vi "transconductance.vi"(6 "Vsg step":dbl=0.002, 8 "B max":dbl=67.0, 9 "B min":dbl=87.0, 10 "load data from file?":bool=TRUE) -> (0 "N Array":T1(array[cluster])=[{"N1"=157.003, "N2"=266.981, "N3"=0.00010058761141376306, "N4"=-1.0315790407323053e-05}, {"N1"=157.003, "N2"=265.999, "N3"=0.00010059098292336149, "N4"=-1.0332480129997402e-05}, {"N1"=157.003, "N2"=265.085, "N3"=0.00010060944077843739, "N4"=-1.0322427910341245e-05}, {"N1"=157.003, "N2"=263.997, "N3"=0.000100657113380779, "N4"=-1.0393866015746848e-05}, {"N1"=157.003, "N2"=263.075, "N3"=0.00010069386977626447, "N4"=-1.0407685152644096e-05}, {"N1"=157.003, "N2"=262.077, "N3"=0.00010056895998220536, "N4"=-1.0343510988281777e-05}, {"N1"=157.003, "N2"=261.132, "N3"=0.00010053448024520868, "N4"=-1.0349016712876126e-05}, {"N1"=157.003, "N2"=260.059, "N3"=0.00010062294424790826, "N4"=-1.0277597394971399e-05}, {"N1"=157.003, "N2"=259.002, "N3"=0.00010065465463674774, "N4"=-1.030766592338683e-05}, {"N1"=157.003, "N2"=257.994, "N3"=0.00010053039567669925, "N4"=-1.0503582041961604e-05}, {"N1"=157.003, "N2"=257.002, "N3"=0.00010061057686438726, "N4"=-1.0271984325309709e-05}, {"N1"=157.003, "N2"=256.047, "N3"=0.00010067349246760751, "N4"=-1.0251899805257316e-05}, {"N1"=157.003, "N2"=255.009, "N3"=0.0001005746979150816, "N4"=-1.0374581059943446e-05}, {"N1"=157.003, "N2"=254.01, "N3"=0.00010064525623886029, "N4"=-1.0267776606434536e-05}, {"N1"=157.003, "N2"=252.961, "N3"=0.0001005733669086136, "N4"=-1.0318808655600757e-05}, {"N1"=157.003, "N2"=252.138, "N3"=0.00010065566340283842, "N4"=-1.0302895488637936e-05}, {"N1"=157.003, "N2"=251.239, "N3"=0.0001006794958238487, "N4"=-1.030436110773387e-05}, {"N1"=157.003, "N2"=250.058, "N3"=0.0001006606457173001, "N4"=-1.033162509347294e-05}, {"N1"=157.003, "N2"=249.134, "N3"=0.00010070695284612299, "N4"=-1.0349127157664972e-05}, {"N1"=157.003, "N2"=248.057, "N3"=0.00010063480571495228, "N4"=-1.0343952424043254e-05}, {"N1"=157.003, "N2"=247.046, "N3"=0.0001005939449441208, "N4"=-1.0301691972698925e-05}, {"N1"=157.003, "N2"=246.001, "N3"=0.00010061079760290319, "N4"=-1.0341399561683132e-05}, {"N1"=157.003, "N2"=245.127, "N3"=0.00010063836300299804, "N4"=-1.038263241630273e-05}, {"N1"=157.003, "N2"=244.19, "N3"=0.00010052888786407929, "N4"=-1.0366000769957849e-05}, {"N1"=157.003, "N2"=243.056, "N3"=0.00010055609422862572, "N4"=-1.032480110310128e-05}, {"N1"=157.003, "N2"=241.985, "N3"=0.00010060349631456675, "N4"=-1.0352572333486109e-05}, {"N1"=157.003, "N2"=240.968, "N3"=0.0001005730466397368, "N4"=-1.0406162088350849e-05}, {"N1"=157.003, "N2"=239.997, "N3"=0.00010055796837859916, "N4"=-1.0447874922582124e-05}, {"N1"=157.003, "N2"=239.348, "N3"=0.00010064935879623944, "N4"=-1.0319947524395836e-05}, {"N1"=157.003, "N2"=238.084, "N3"=0.00010057773089892466, "N4"=-1.0479841722046195e-05}, {"N1"=157.003, "N2"=237.112, "N3"=0.00010064891429557363, "N4"=-1.049047519616346e-05}, {"N1"=157.003, "N2"=236.004, "N3"=0.00010065709472725735, "N4"=-1.0324150119014948e-05}, {"N1"=157.003, "N2"=234.996, "N3"=0.00010057723777641319, "N4"=-1.0336422363141234e-05}, {"N1"=157.003, "N2"=234.019, "N3"=0.00010045398973880146, "N4"=-1.0377301904232947e-05}, {"N1"=157.003, "N2"=233.096, "N3"=0.00010057181495580477, "N4"=-1.0313588970498165e-05}, {"N1"=157.003, "N2"=232.123, "N3"=0.00010054998403538271, "N4"=-1.0403263055311217e-05}, {"N1"=157.003, "N2"=231.112, "N3"=0.00010069630908042105, "N4"=-1.0328850635915879e-05}, {"N1"=157.003, "N2"=230.005, "N3"=0.0001005825699420265, "N4"=-1.013345847934897e-05}, {"N1"=157.003, "N2"=229.052, "N3"=0.00010066775145077032, "N4"=-1.0360530914703863e-05}, {"N1"=157.003, "N2"=228.029, "N3"=0.0001006005911344668, "N4"=-1.0262365451060467e-05}, {"N1"=157.003, "N2"=227.081, "N3"=0.0001006880496209156, "N4"=-1.0331153141935446e-05}, {"N1"=157.003, "N2"=226.184, "N3"=0.00010063762766846488, "N4"=-1.0365370825229791e-05}, {"N1"=157.003, "N2"=225.156, "N3"=0.00010060840425208388, "N4"=-1.0325694682226826e-05}, {"N1"=157.003, "N2"=223.981, "N3"=0.00010060008180158568, "N4"=-1.030788393467471e-05}, {"N1"=157.003, "N2"=223.117, "N3"=0.00010064362809307492, "N4"=-1.0410394990300755e-05}, {"N1"=157.003, "N2"=222.006, "N3"=0.00010052956894532667, "N4"=-1.0312456867656895e-05}, {"N1"=157.003, "N2"=221.15, "N3"=0.00010073993925105531, "N4"=-1.0520923879015318e-05}, {"N1"=157.003, "N2"=220.132, "N3"=0.0001005467107798333, "N4"=-1.0451840001316155e-05}, {"N1"=157.003, "N2"=219.14, "N3"=0.00010056576858730084, "N4"=-1.0520553001153154e-05}, {"N1"=157.003, "N2"=218.151, "N3"=0.00010058549543700654, "N4"=-1.0330365594944888e-05}, {"N1"=157.003, "N2"=217.144, "N3"=0.00010051145692162056, "N4"=-1.03377330611703e-05}, {"N1"=157.003, "N2"=216.153, "N3"=0.00010073501846407267, "N4"=-1.0489693235349407e-05}, {"N1"=157.003, "N2"=214.997, "N3"=0.00010066401252774728, "N4"=-1.0430688948597772e-05}, {"N1"=157.003, "N2"=214.148, "N3"=0.00010062308186580819, "N4"=-1.0280249425931093e-05}, {"N1"=157.003, "N2"=213.226, "N3"=0.00010062562347473316, "N4"=-1.0297033249151475e-05}, {"N1"=157.003, "N2"=212.267, "N3"=0.0001004056393064652, "N4"=-1.0354527978745687e-05}, {"N1"=157.003, "N2"=211.106, "N3"=0.00010053371092077836, "N4"=-1.0258061653605368e-05}, {"N1"=157.003, "N2"=210.034, "N3"=0.0001005206561452233, "N4"=-1.0277392375838352e-05}, {"N1"=157.003, "N2"=209.16, "N3"=0.00010062151524095544, "N4"=-1.0318539021491905e-05}, {"N1"=157.003, "N2"=208.248, "N3"=0.00010059710791627925, "N4"=-1.0633465001550955e-05}, {"N1"=157.003, "N2"=207.003, "N3"=0.00010062673174994523, "N4"=-1.0321171852761056e-05}, {"N1"=157.003, "N2"=206.388, "N3"=0.00010061513331833293, "N4"=-1.0324705100902347e-05}, {"N1"=157.003, "N2"=204.991, "N3"=0.0001005439011236034, "N4"=-1.0309493090621932e-05}, {"N1"=157.003, "N2"=204.132, "N3"=0.00010070060888909204, "N4"=-1.0291219627570718e-05}, {"N1"=157.003, "N2"=203.139, "N3"=0.00010064572292852508, "N4"=-1.0464495626958931e-05}, {"N1"=157.003, "N2"=202.208, "N3"=0.00010064163036004339, "N4"=-1.0527705497905832e-05}, {"N1"=157.003, "N2"=200.997, "N3"=0.00010060444212186648, "N4"=-1.0239666475444635e-05}, {"N1"=157.003, "N2"=199.979, "N3"=0.00010045464357967768, "N4"=-1.0332757739473804e-05}, {"N1"=157.003, "N2"=199.145, "N3"=0.00010052319470245587, "N4"=-1.0408078825076916e-05}, {"N1"=157.003, "N2"=198.151, "N3"=0.00010054670987583925, "N4"=-1.0224118002428333e-05}, {"N1"=157.003, "N2"=197.167, "N3"=0.00010064778537782342, "N4"=-1.0323540832018964e-05}, {"N1"=157.003, "N2"=196.024, "N3"=0.00010059750202844955, "N4"=-1.031116849358743e-05}, {"N1"=157.003, "N2"=195.158, "N3"=0.00010058423886157823, "N4"=-1.0255054779838974e-05}, {"N1"=157.003, "N2"=194.255, "N3"=0.00010071404209700317, "N4"=-1.0181418387683495e-05}, {"N1"=157.003, "N2"=193.167, "N3"=0.00010057340590266535, "N4"=-1.0242330877904251e-05}, {"N1"=157.003, "N2"=192.004, "N3"=0.00010068713388045283, "N4"=-1.0249310430158046e-05}, {"N1"=157.003, "N2"=191.222, "N3"=0.00010060502412989036, "N4"=-1.0132381864656099e-05}, {"N1"=157.003, "N2"=190.0, "N3"=0.00010060744320199426, "N4"=-1.0398792500202499e-05}, {"N1"=157.003, "N2"=189.161, "N3"=0.00010058313711640197, "N4"=-1.0335999046260006e-05}, {"N1"=157.003, "N2"=188.182, "N3"=0.0001005729482088783, "N4"=-1.0175494539414885e-05}, {"N1"=157.003, "N2"=187.187, "N3"=0.00010062532065791654, "N4"=-1.0311661990340356e-05}, {"N1"=157.003, "N2"=186.127, "N3"=0.00010070821910793247, "N4"=-1.027480676439334e-05}, {"N1"=157.003, "N2"=185.003, "N3"=0.00010055156194819312, "N4"=-1.028064538575304e-05}, {"N1"=157.003, "N2"=183.995, "N3"=0.00010067671472910203, "N4"=-1.0455212193898765e-05}, {"N1"=157.003, "N2"=183.205, "N3"=0.00010050604172122397, "N4"=-1.0365017753701822e-05}, {"N1"=157.003, "N2"=182.153, "N3"=0.00010057840866780894, "N4"=-1.0315396628303899e-05}, {"N1"=157.003, "N2"=181.15, "N3"=0.00010058546375450866, "N4"=-1.0361578284644076e-05}, {"N1"=157.003, "N2"=179.996, "N3"=0.0001006240086180247, "N4"=-1.0119129316713388e-05}, {"N1"=157.003, "N2"=179.042, "N3"=0.00010064273438767862, "N4"=-1.0255802631395027e-05}, {"N1"=157.003, "N2"=177.974, "N3"=0.00010063106842247951, "N4"=-1.0299974893794054e-05}, {"N1"=157.003, "N2"=177.161, "N3"=0.00010065009914739528, "N4"=-1.0296372901106247e-05}, {"N1"=157.003, "N2"=175.982, "N3"=0.00010067126680486314, "N4"=-1.0306700692332765e-05}, {"N1"=157.003, "N2"=174.995, "N3"=0.00010053475509784773, "N4"=-1.0433320095914615e-05}, {"N1"=157.003, "N2"=174.139, "N3"=0.00010049406853859304, "N4"=-1.0270604949039266e-05}, {"N1"=157.003, "N2"=173.118, "N3"=0.00010053736854866473, "N4"=-1.016880594814786e-05}, {"N1"=157.003, "N2"=172.219, "N3"=0.00010058931714745791, "N4"=-1.0410165714531099e-05}, {"N1"=157.003, "N2"=171.156, "N3"=0.00010056082364767814, "N4"=-1.0322038747437007e-05}, {"N1"=157.003, "N2"=170.109, "N3"=0.00010056010719994381, "N4"=-1.0287668368179046e-05}, {"N1"=157.003, "N2"=169.204, "N3"=0.00010064886941818687, "N4"=-1.029160673901251e-05}, {"N1"=157.003, "N2"=168.15, "N3"=0.00010060742217090351, "N4"=-1.0262911647489893e-05}, {"N1"=157.003, "N2"=167.112, "N3"=0.00010047282448029428, "N4"=-1.0358833399498402e-05}, {"N1"=157.003, "N2"=166.21, "N3"=0.00010060401190277079, "N4"=-1.0350385128996471e-05}, {"N1"=157.003, "N2"=165.011, "N3"=0.00010060416035284246, "N4"=-1.0377472785141268e-05}, {"N1"=157.003, "N2"=164.167, "N3"=0.0001004397217463161, "N4"=-1.0450134705351127e-05}, {"N1"=157.003, "N2"=163.001, "N3"=0.00010051036584794823, "N4"=-1.0382389231895817e-05}, {"N1"=157.003, "N2"=162.034, "N3"=0.00010047904100883916, "N4"=-1.0341186675967576e-05}, {"N1"=157.003, "N2"=160.997, "N3"=0.00010053000872693343, "N4"=-1.0484345783511955e-05}, {"N1"=157.003, "N2"=160.209, "N3"=0.00010062652830459546, "N4"=-1.0297537290876405e-05}, {"N1"=157.003, "N2"=159.149, "N3"=0.00010056339474194626, "N4"=-1.0346385416074202e-05}, {"N1"=157.003, "N2"=157.992, "N3"=0.00010054027429101758, "N4"=-1.0402084267772915e-05}, {"N1"=157.003, "N2"=157.001, "N3"=0.00010072664661678648, "N4"=-1.0389584614637704e-05}, {"N1"=157.003, "N2"=156.136, "N3"=0.00010057574533189637, "N4"=-1.0286379321831545e-05}, {"N1"=157.003, "N2"=155.184, "N3"=0.00010061297401308573, "N4"=-1.0356101436450663e-05}, {"N1"=157.003, "N2"=154.14, "N3"=0.00010065486717861918, "N4"=-1.027695564379398e-05}, {"N1"=157.003, "N2"=153.001, "N3"=0.00010066710265738706, "N4"=-1.0289877618531446e-05}, {"N1"=157.003, "N2"=152.094, "N3"=0.00010069298668309146, "N4"=-1.0373605458303733e-05}, {"N1"=157.003, "N2"=151.229, "N3"=0.00010075373194915584, "N4"=-1.0343078388110773e-05}, {"N1"=147.01, "N2"=267.017, "N3"=9.799983736018753e-05, "N4"=-1.0019951532324723e-05}, {"N1"=147.01, "N2"=262.383, "N3"=9.763241950106681e-05, "N4"=-9.728183012788925e-06}, {"N1"=147.01, "N2"=257.562, "N3"=9.857415477184657e-05, "N4"=-9.961675445649451e-06}, {"N1"=147.01, "N2"=252.008, "N3"=9.812568640591443e-05, "N4"=-9.853612153506874e-06}, {"N1"=147.01, "N2"=247.006, "N3"=9.984319825339365e-05, "N4"=-1.0146544647968204e-05}, {"N1"=147.01, "N2"=241.997, "N3"=9.947477892699824e-05, "N4"=-1.0131401570354352e-05}, {"N1"=147.01, "N2"=238.533, "N3"=0.00010005415475521616, "N4"=-1.0167893750971189e-05}, {"N1"=147.01, "N2"=232.001, "N3"=9.882236061778423e-05, "N4"=-1.011184445981214e-05}, {"N1"=147.01, "N2"=228.619, "N3"=9.9581272321477e-05, "N4"=-1.0201481180871728e-05}, {"N1"=147.01, "N2"=221.992, "N3"=9.96719889398003e-05, "N4"=-1.0088519208290693e-05}, {"N1"=147.01, "N2"=217.038, "N3"=9.844041955679962e-05, "N4"=-9.941300701952415e-06}, {"N1"=147.01, "N2"=212.037, "N3"=9.969254017177194e-05, "N4"=-1.0181600609931255e-05}, {"N1"=147.01, "N2"=207.001, "N3"=9.949616020991875e-05, "N4"=-1.0131625256668759e-05}, {"N1"=147.01, "N2"=202.009, "N3"=9.972322051345787e-05, "N4"=-1.030119353660157e-05}, {"N1"=147.01, "N2"=197.009, "N3"=9.972222689830247e-05, "N4"=-1.0129755820315606e-05}, {"N1"=147.01, "N2"=192.052, "N3"=9.927072186296552e-05, "N4"=-1.0101700894209476e-05}, {"N1"=147.01, "N2"=187.035, "N3"=9.971985526642769e-05, "N4"=-1.0163071908619776e-05}, {"N1"=147.01, "N2"=182.038, "N3"=9.938768123188747e-05, "N4"=-1.0116333084138861e-05}, {"N1"=147.01, "N2"=177.024, "N3"=9.895565966028784e-05, "N4"=-1.0184916134362883e-05}, {"N1"=147.01, "N2"=172.002, "N3"=9.903423254443763e-05, "N4"=-9.977232855655323e-06}, {"N1"=147.01, "N2"=167.528, "N3"=9.938030934401597e-05, "N4"=-1.013542865258268e-05}, {"N1"=147.01, "N2"=162.609, "N3"=9.898463034406892e-05, "N4"=-1.0045094991441177e-05}, {"N1"=147.01, "N2"=157.833, "N3"=9.946683387231336e-05, "N4"=-1.0208638458775468e-05}, {"N1"=137.106, "N2"=157.019, "N3"=0.00010037737790660152, "N4"=-1.030680610999361e-05}, {"N1"=137.106, "N2"=161.993, "N3"=0.00010051095901282851, "N4"=-1.015609388550053e-05}, {"N1"=137.106, "N2"=166.478, "N3"=0.00010061415096599144, "N4"=-1.0361761811054065e-05}, {"N1"=137.106, "N2"=171.321, "N3"=0.00010066129576563336, "N4"=-1.0484617945251967e-05}, {"N1"=137.106, "N2"=177.002, "N3"=0.00010061617278473286, "N4"=-1.0472267311277374e-05}, {"N1"=137.106, "N2"=181.274, "N3"=0.00010061494851260961, "N4"=-1.0526404210905806e-05}, {"N1"=137.106, "N2"=185.979, "N3"=0.00010059337699446351, "N4"=-1.040515740405918e-05}, {"N1"=137.106, "N2"=190.957, "N3"=0.0001006229368267242, "N4"=-1.0316576837476962e-05}, {"N1"=137.106, "N2"=196.956, "N3"=0.00010052691716632796, "N4"=-1.0426565141411268e-05}, {"N1"=137.106, "N2"=200.797, "N3"=0.00010048017416406656, "N4"=-1.0205543027371177e-05}, {"N1"=137.106, "N2"=206.992, "N3"=0.00010051573531694569, "N4"=-1.0500465961498208e-05}, {"N1"=137.106, "N2"=211.99, "N3"=0.00010047604987372997, "N4"=-1.0186688450911605e-05}, {"N1"=137.106, "N2"=216.974, "N3"=0.00010041066876877247, "N4"=-1.0483017642678282e-05}, {"N1"=137.106, "N2"=221.18, "N3"=0.00010052645014313375, "N4"=-1.0365935977453018e-05}, {"N1"=137.106, "N2"=225.381, "N3"=0.00010058558925443369, "N4"=-1.0254871445882739e-05}, {"N1"=137.106, "N2"=232.004, "N3"=9.913954515490299e-05, "N4"=-1.005309209916423e-05}, {"N1"=137.106, "N2"=236.99, "N3"=0.0001003799328902402, "N4"=-1.0139936029757658e-05}, {"N1"=137.106, "N2"=242.016, "N3"=0.00010005730438840346, "N4"=-1.0090877786993333e-05}, {"N1"=137.106, "N2"=245.974, "N3"=0.00010048425816903801, "N4"=-1.0483823131656468e-05}, {"N1"=137.106, "N2"=250.925, "N3"=0.00010040732666965968, "N4"=-1.0299776631743095e-05}, {"N1"=137.106, "N2"=257.02, "N3"=0.00010045673123155542, "N4"=-1.014502752268486e-05}, {"N1"=137.106, "N2"=261.97, "N3"=0.00010053750806744122, "N4"=-1.0170204737819931e-05}, {"N1"=137.106, "N2"=266.974, "N3"=0.00010046811899562129, "N4"=-1.0258157731175788e-05}, {"N1"=127.009, "N2"=157.022, "N3"=0.00010057347860141696, "N4"=-1.0228102959349011e-05}, {"N1"=127.009, "N2"=161.996, "N3"=0.00010062562883782826, "N4"=-1.0170220838565306e-05}, {"N1"=127.009, "N2"=167.013, "N3"=0.00010066593581146635, "N4"=-1.0124193285242448e-05}, {"N1"=127.009, "N2"=171.248, "N3"=0.00010070721275823473, "N4"=-1.0260385180386528e-05}, {"N1"=127.009, "N2"=176.996, "N3"=0.00010064297358361281, "N4"=-1.0308355187961158e-05}, {"N1"=127.009, "N2"=181.986, "N3"=0.00010061342489787007, "N4"=-1.0129603180411648e-05}, {"N1"=127.009, "N2"=186.989, "N3"=0.00010061225714944682, "N4"=-1.026327093758386e-05}, {"N1"=127.009, "N2"=192.002, "N3"=0.00010060286819188852, "N4"=-1.0222596869690172e-05}, {"N1"=127.009, "N2"=197.03, "N3"=0.00010067499622887365, "N4"=-1.042309998693685e-05}, {"N1"=127.009, "N2"=202.004, "N3"=0.00010059110286327089, "N4"=-1.0321036547786183e-05}, {"N1"=127.009, "N2"=206.995, "N3"=0.00010059948277673225, "N4"=-1.0384420982036602e-05}, {"N1"=127.009, "N2"=211.966, "N3"=0.00010058300170100732, "N4"=-1.0321869852951667e-05}, {"N1"=127.009, "N2"=216.996, "N3"=0.00010057100746133218, "N4"=-1.0479270764700121e-05}, {"N1"=127.009, "N2"=222.012, "N3"=0.00010050186248972992, "N4"=-1.0279112143261431e-05}, {"N1"=127.009, "N2"=227.008, "N3"=0.00010067472374815698, "N4"=-1.024778604350329e-05}, {"N1"=127.009, "N2"=231.971, "N3"=0.00010065735991437597, "N4"=-1.027124744107791e-05}, {"N1"=127.009, "N2"=237.004, "N3"=0.00010057124546163262, "N4"=-1.0340391607088675e-05}, {"N1"=127.009, "N2"=242.0, "N3"=0.00010054458432600382, "N4"=-1.0398708177970036e-05}, {"N1"=127.009, "N2"=246.996, "N3"=0.00010062032362546629, "N4"=-1.029301084170431e-05}, {"N1"=127.009, "N2"=251.943, "N3"=0.0001005705365053531, "N4"=-1.0188324652684972e-05}, {"N1"=127.009, "N2"=256.96, "N3"=0.00010061231844925602, "N4"=-1.0222616593874322e-05}, {"N1"=127.009, "N2"=261.944, "N3"=0.0001005374732511164, "N4"=-1.0238804050129587e-05}, {"N1"=127.009, "N2"=267.002, "N3"=0.00010061482989823944, "N4"=-1.0260599454521908e-05}, {"N1"=117.007, "N2"=32.056, "N3"=0.00010064978817090146, "N4"=-1.025610764423456e-05}, {"N1"=117.007, "N2"=34.532, "N3"=0.00010045388961118922, "N4"=-1.0281623718938048e-05}, {"N1"=117.007, "N2"=36.991, "N3"=0.00010051501976709822, "N4"=-1.0346988455857735e-05}, {"N1"=117.007, "N2"=39.496, "N3"=0.00010051493139529077, "N4"=-1.0087270665342305e-05}, {"N1"=117.007, "N2"=42.014, "N3"=0.00010069551813105615, "N4"=-1.0293552346164798e-05}, {"N1"=117.007, "N2"=44.076, "N3"=0.00010061513649741965, "N4"=-1.0166358665250762e-05}, {"N1"=117.007, "N2"=47.003, "N3"=0.00010062687846722984, "N4"=-1.0327337858815028e-05}, {"N1"=117.007, "N2"=49.497, "N3"=0.00010056452732695654, "N4"=-1.0173349314359884e-05}, {"N1"=117.007, "N2"=52.015, "N3"=0.00010052841627670957, "N4"=-1.0154426622830124e-05}, {"N1"=117.007, "N2"=54.143, "N3"=0.00010067512909890701, "N4"=-1.0297943395729118e-05}, {"N1"=117.007, "N2"=56.469, "N3"=0.00010058850823882672, "N4"=-1.0229671611179695e-05}, {"N1"=117.007, "N2"=59.109, "N3"=0.00010052479798279025, "N4"=-1.0343373479061018e-05}, {"N1"=117.007, "N2"=61.392, "N3"=0.00010058686320873386, "N4"=-1.022378755210072e-05}, {"N1"=117.007, "N2"=64.504, "N3"=0.0001005412527806689, "N4"=-1.0139418557798202e-05}, {"N1"=117.007, "N2"=66.556, "N3"=0.00010059966338797697, "N4"=-1.0310327223639804e-05}, {"N1"=117.007, "N2"=69.51, "N3"=0.00010057652888712345, "N4"=-1.0212157986809609e-05}, {"N1"=117.007, "N2"=71.992, "N3"=0.00010050180247112291, "N4"=-1.028268878318887e-05}, {"N1"=117.007, "N2"=74.522, "N3"=0.00010060272680910092, "N4"=-1.0302907303716237e-05}, {"N1"=117.007, "N2"=76.511, "N3"=0.00010063436117013613, "N4"=-1.0284977160718541e-05}, {"N1"=117.007, "N2"=79.507, "N3"=0.00010053382792202885, "N4"=-1.0146593941792322e-05}, {"N1"=117.007, "N2"=81.621, "N3"=0.0001005751528212949, "N4"=-1.0354807579206691e-05}, {"N1"=117.007, "N2"=84.502, "N3"=0.00010054348640316594, "N4"=-9.990825055029414e-06}, {"N1"=117.007, "N2"=86.673, "N3"=0.00010050030986939123, "N4"=-1.0332786827163976e-05}, {"N1"=117.007, "N2"=89.151, "N3"=0.0001006654029019091, "N4"=-1.0344630164623589e-05}, {"N1"=117.007, "N2"=91.994, "N3"=0.00010054329129975139, "N4"=-1.0416490377942942e-05}, {"N1"=117.007, "N2"=93.872, "N3"=0.00010074985037679878, "N4"=-1.0168075579477274e-05}, {"N1"=117.007, "N2"=97.001, "N3"=0.00010066712568587043, "N4"=-1.0282065430206825e-05}, {"N1"=117.007, "N2"=99.508, "N3"=0.00010058539368521102, "N4"=-1.0226362854395622e-05}, {"N1"=117.007, "N2"=102.003, "N3"=0.00010072773688354306, "N4"=-1.0239518541904778e-05}, {"N1"=117.007, "N2"=104.027, "N3"=0.0001006236337285617, "N4"=-9.92643871278832e-06}, {"N1"=117.007, "N2"=107.002, "N3"=0.00010052762532773571, "N4"=-1.0217345822124191e-05}, {"N1"=117.007, "N2"=109.51, "N3"=0.0001006008322570536, "N4"=-1.0213249312954479e-05}, {"N1"=117.007, "N2"=111.64, "N3"=0.00010065064240265076, "N4"=-1.043949739151913e-05}, {"N1"=117.007, "N2"=114.086, "N3"=0.00010065977101688157, "N4"=-1.0347667960354994e-05}, {"N1"=117.007, "N2"=116.974, "N3"=0.00010064577563892032, "N4"=-1.0261940880614038e-05}, {"N1"=117.007, "N2"=119.164, "N3"=0.00010055241551826978, "N4"=-1.0013106313453286e-05}, {"N1"=117.007, "N2"=121.617, "N3"=0.000100561207477888, "N4"=-1.0369167295744242e-05}, {"N1"=117.007, "N2"=123.953, "N3"=0.00010059801647650067, "N4"=-1.0273027796032252e-05}, {"N1"=117.007, "N2"=126.551, "N3"=0.0001006127598601274, "N4"=-1.0125299677061743e-05}, {"N1"=117.007, "N2"=129.224, "N3"=0.00010055833799216406, "N4"=-1.0282054349485067e-05}, {"N1"=117.007, "N2"=131.348, "N3"=0.0001006318839714987, "N4"=-1.0193376447352927e-05}, {"N1"=117.007, "N2"=134.11, "N3"=0.00010063185541431723, "N4"=-1.0205829882631764e-05}, {"N1"=117.007, "N2"=137.003, "N3"=0.00010060564044060756, "N4"=-1.0244636687470948e-05}, {"N1"=117.007, "N2"=139.499, "N3"=0.00010062058894582516, "N4"=-1.0205560464282248e-05}, {"N1"=117.007, "N2"=141.377, "N3"=0.00010055921223965429, "N4"=-1.0317277689164375e-05}, {"N1"=117.007, "N2"=143.853, "N3"=0.00010063046467230716, "N4"=-1.0424464439912497e-05}, {"N1"=117.007, "N2"=146.475, "N3"=0.00010074839880717587, "N4"=-9.968827456523466e-06}, {"N1"=117.007, "N2"=149.043, "N3"=0.00010060702485041066, "N4"=-1.0324898769603983e-05}, {"N1"=117.007, "N2"=151.32, "N3"=0.00010061979522812291, "N4"=-1.010611168298942e-05}, {"N1"=117.007, "N2"=153.929, "N3"=0.00010073737621468872, "N4"=-1.017623849860103e-05}, {"N1"=117.007, "N2"=156.997, "N3"=0.00010052357273829458, "N4"=-1.030104354858853e-05}, {"N1"=117.007, "N2"=159.155, "N3"=0.00010064384474727063, "N4"=-1.0154250298751187e-05}, {"N1"=117.007, "N2"=161.993, "N3"=0.00010049835467157835, "N4"=-1.0126613367881921e-05}, {"N1"=117.007, "N2"=163.92, "N3"=0.00010061017247784827, "N4"=-1.0129053480100996e-05}, {"N1"=117.007, "N2"=166.542, "N3"=0.00010066112540598374, "N4"=-1.0323598162374622e-05}, {"N1"=117.007, "N2"=169.032, "N3"=0.00010056464247038716, "N4"=-1.015117251415302e-05}, {"N1"=117.007, "N2"=171.999, "N3"=0.00010055273787852328, "N4"=-1.0222883358440501e-05}, {"N1"=117.007, "N2"=174.087, "N3"=0.0001005535662134572, "N4"=-1.0233743737108524e-05}, {"N1"=117.007, "N2"=177.013, "N3"=0.00010065204487612477, "N4"=-1.0278690981467345e-05}, {"N1"=117.007, "N2"=179.486, "N3"=0.00010062663690154288, "N4"=-1.0210955481467252e-05}, {"N1"=117.007, "N2"=181.566, "N3"=0.00010065643695650927, "N4"=-1.0305260660087358e-05}, {"N1"=117.007, "N2"=184.05, "N3"=0.00010053947571011885, "N4"=-1.0281875916189764e-05}, {"N1"=117.007, "N2"=186.314, "N3"=0.00010051599223005814, "N4"=-1.0336881480449907e-05}, {"N1"=117.007, "N2"=188.866, "N3"=0.00010068051349858722, "N4"=-1.026762456597061e-05}, {"N1"=117.007, "N2"=191.473, "N3"=0.00010059622764588772, "N4"=-1.0246628233644514e-05}, {"N1"=117.007, "N2"=194.499, "N3"=0.0001004420622289131, "N4"=-1.0237429165590822e-05}, {"N1"=117.007, "N2"=197.005, "N3"=0.00010060970619697381, "N4"=-1.0205860357975657e-05}, {"N1"=117.007, "N2"=199.518, "N3"=0.00010062216506165582, "N4"=-1.0228015285178902e-05}, {"N1"=117.007, "N2"=201.451, "N3"=0.00010078348793378344, "N4"=-1.0117377988074068e-05}, {"N1"=117.007, "N2"=204.498, "N3"=0.00010059087649278548, "N4"=-1.0238717664490123e-05}, {"N1"=117.007, "N2"=207.002, "N3"=0.00010057185074610495, "N4"=-1.0255278722166194e-05}, {"N1"=117.007, "N2"=209.501, "N3"=0.00010050592898327873, "N4"=-1.0391027260226272e-05}, {"N1"=117.007, "N2"=211.266, "N3"=0.0001005823105087564, "N4"=-1.0250973507029187e-05}, {"N1"=117.007, "N2"=214.506, "N3"=0.00010063260661714465, "N4"=-1.0292247886556636e-05}, {"N1"=117.007, "N2"=216.342, "N3"=0.00010063951530946773, "N4"=-1.0279616841338573e-05}, {"N1"=117.007, "N2"=219.492, "N3"=0.00010048115826019133, "N4"=-1.0267554131539686e-05}, {"N1"=117.007, "N2"=221.307, "N3"=0.0001006316815669094, "N4"=-1.0207880772305242e-05}, {"N1"=117.007, "N2"=224.494, "N3"=0.00010054522858521489, "N4"=-1.0184516241235662e-05}, {"N1"=117.007, "N2"=226.535, "N3"=0.00010070519724589977, "N4"=-1.0178226851388292e-05}, {"N1"=117.007, "N2"=228.773, "N3"=0.00010055385580668074, "N4"=-1.0249496333864772e-05}, {"N1"=117.007, "N2"=231.998, "N3"=0.00010064839405973074, "N4"=-1.0482356762634406e-05}, {"N1"=117.007, "N2"=234.493, "N3"=0.0001005447595299115, "N4"=-1.014946667913593e-05}, {"N1"=117.007, "N2"=236.999, "N3"=0.00010054486355912897, "N4"=-1.0488706413938635e-05}, {"N1"=117.007, "N2"=239.48, "N3"=0.00010053899503907004, "N4"=-1.0335221946167345e-05}, {"N1"=117.007, "N2"=241.988, "N3"=0.0001005781719500306, "N4"=-1.0175093856633557e-05}, {"N1"=117.007, "N2"=244.468, "N3"=0.0001004815279861057, "N4"=-1.022807286858223e-05}, {"N1"=117.007, "N2"=246.5, "N3"=0.00010075441800463656, "N4"=-1.0055129608757884e-05}, {"N1"=117.007, "N2"=248.959, "N3"=0.0001006404674253252, "N4"=-1.032902146641543e-05}, {"N1"=117.007, "N2"=252.031, "N3"=0.0001006261384085402, "N4"=-1.0265942683216317e-05}, {"N1"=117.007, "N2"=253.846, "N3"=0.00010070306362349486, "N4"=-1.0240516717808242e-05}, {"N1"=117.007, "N2"=257.004, "N3"=0.0001006801603898491, "N4"=-1.0325659054015416e-05}, {"N1"=117.007, "N2"=259.503, "N3"=0.00010055575183981358, "N4"=-1.0294112971374265e-05}, {"N1"=117.007, "N2"=262.01, "N3"=0.00010062552009819317, "N4"=-1.0188597483007576e-05}, {"N1"=117.007, "N2"=263.976, "N3"=0.00010063652055599028, "N4"=-1.0204669545558723e-05}, {"N1"=117.007, "N2"=266.952, "N3"=0.000100514825665194, "N4"=-1.040146174902912e-05}, {"N1"=117.007, "N2"=269.469, "N3"=0.0001006420158488929, "N4"=-1.0331409244148652e-05}, {"N1"=117.007, "N2"=271.982, "N3"=0.00010057113432047844, "N4"=-1.0220097216685064e-05}, {"N1"=117.007, "N2"=274.503, "N3"=0.00010058024667950214, "N4"=-1.031877234810934e-05}, {"N1"=117.007, "N2"=276.997, "N3"=0.0001005561952905316, "N4"=-1.0286103088404645e-05}, {"N1"=117.007, "N2"=279.503, "N3"=0.00010051021491299667, "N4"=-1.0437540985715723e-05}, {"N1"=117.007, "N2"=282.002, "N3"=0.00010064439847725866, "N4"=-1.0075036301704775e-05}, {"N1"=117.007, "N2"=284.503, "N3"=0.0001006200552994746, "N4"=-1.0263733076995429e-05}, {"N1"=117.007, "N2"=286.96, "N3"=0.00010058228864646168, "N4"=-1.0217664392238925e-05}, {"N1"=117.007, "N2"=289.5, "N3"=0.00010063080321728486, "N4"=-1.0261720319263618e-05}, {"N1"=117.007, "N2"=291.996, "N3"=0.00010042548197148666, "N4"=-1.0116467509768251e-05}, {"N1"=117.007, "N2"=294.44, "N3"=0.00010058818357799011, "N4"=-1.0369759866378409e-05}, {"N1"=117.007, "N2"=297.002, "N3"=0.00010061449943261898, "N4"=-1.0198178104675134e-05}, {"N1"=117.007, "N2"=299.447, "N3"=0.00010053105057471438, "N4"=-1.0346528082889999e-05}, {"N1"=117.007, "N2"=301.999, "N3"=0.00010069113752078103, "N4"=-1.0211268869372451e-05}, {"N1"=187.027, "N2"=89.503, "N3"=0.0001005538097501194, "N4"=-1.0068716487720403e-05}, {"N1"=187.027, "N2"=87.241, "N3"=0.00010063437472482058, "N4"=-1.0504361485493965e-05}, {"N1"=187.027, "N2"=84.714, "N3"=0.0001005805723632631, "N4"=-1.0371142364249591e-05}, {"N1"=187.027, "N2"=82.378, "N3"=0.00010058564168627688, "N4"=-1.0616441632202452e-05}, {"N1"=187.027, "N2"=79.768, "N3"=0.00010055343585591008, "N4"=-1.0293175645836954e-05}, {"N1"=187.027, "N2"=77.006, "N3"=0.0001006022924498344, "N4"=-1.025812933866109e-05}, {"N1"=187.027, "N2"=74.747, "N3"=0.00010053039429056371, "N4"=-1.0480715790045093e-05}, {"N1"=187.027, "N2"=72.204, "N3"=0.00010073948663635986, "N4"=-1.0397569090337858e-05}, {"N1"=187.027, "N2"=69.687, "N3"=0.00010047861358984462, "N4"=-1.0406363855228905e-05}, {"N1"=187.027, "N2"=67.001, "N3"=0.00010059018869806295, "N4"=-1.0362119487654798e-05}, {"N1"=187.027, "N2"=64.514, "N3"=0.00010067770468751678, "N4"=-1.0264446735673443e-05}, {"N1"=184.504, "N2"=64.511, "N3"=0.00010067979628336618, "N4"=-1.0123006665973067e-05}, {"N1"=184.504, "N2"=66.865, "N3"=0.00010058980563947531, "N4"=-1.034051355402341e-05}, {"N1"=184.504, "N2"=69.309, "N3"=0.00010058242185159121, "N4"=-1.0332746370657409e-05}, {"N1"=184.504, "N2"=72.02, "N3"=0.0001006185988594614, "N4"=-1.0322913240994248e-05}, {"N1"=184.504, "N2"=74.346, "N3"=0.00010053861643353745, "N4"=-1.0189404728299887e-05}, {"N1"=184.504, "N2"=76.763, "N3"=0.00010051830927292453, "N4"=-1.0304975486645362e-05}, {"N1"=184.504, "N2"=79.202, "N3"=0.00010063132765245739, "N4"=-1.0497288171111559e-05}, {"N1"=184.504, "N2"=82.007, "N3"=0.0001006238777087195, "N4"=-1.0342532146106403e-05}, {"N1"=184.504, "N2"=84.288, "N3"=0.00010059607081892192, "N4"=-1.0391061751967603e-05}, {"N1"=184.504, "N2"=86.989, "N3"=0.0001005416740301612, "N4"=-1.0390375441065005e-05}, {"N1"=184.504, "N2"=89.512, "N3"=0.00010048184727127543, "N4"=-1.0500678517682486e-05}, {"N1"=182.02, "N2"=89.482, "N3"=0.00010050855414624652, "N4"=-1.0331298091019059e-05}, {"N1"=182.02, "N2"=87.008, "N3"=0.00010059725246730611, "N4"=-1.0021974070113783e-05}, {"N1"=182.02, "N2"=84.5, "N3"=0.00010064138388942822, "N4"=-1.0330565331350644e-05}, {"N1"=182.02, "N2"=82.251, "N3"=0.00010059626324907907, "N4"=-1.0363153720005846e-05}, {"N1"=182.02, "N2"=79.689, "N3"=0.00010070038682013327, "N4"=-1.0152433515939979e-05}, {"N1"=182.02, "N2"=76.996, "N3"=0.0001006624795222232, "N4"=-1.036483953997913e-05}, {"N1"=182.02, "N2"=74.714, "N3"=0.00010055589215289286, "N4"=-1.0413660572035531e-05}, {"N1"=182.02, "N2"=71.997, "N3"=0.00010060580719745948, "N4"=-1.0382949390742456e-05}, {"N1"=182.02, "N2"=69.897, "N3"=0.0001005916548237922, "N4"=-1.035092915466362e-05}, {"N1"=182.02, "N2"=67.236, "N3"=0.00010059841289240594, "N4"=-1.0442950057046927e-05}, {"N1"=182.02, "N2"=64.532, "N3"=0.00010059224341172395, "N4"=-1.062260387394076e-05}, {"N1"=179.503, "N2"=64.479, "N3"=0.00010057055625034519, "N4"=-1.0517867007309303e-05}, {"N1"=179.503, "N2"=66.781, "N3"=0.000100421153562096, "N4"=-1.0331116778665024e-05}, {"N1"=179.503, "N2"=69.326, "N3"=0.00010054916476736131, "N4"=-1.0331989543478477e-05}, {"N1"=179.503, "N2"=71.763, "N3"=0.00010047434048428019, "N4"=-1.0263828286308527e-05}, {"N1"=179.503, "N2"=74.235, "N3"=0.00010057455741087348, "N4"=-1.0380831519662786e-05}, {"N1"=179.503, "N2"=76.705, "N3"=0.00010066717519552144, "N4"=-1.0380978544815065e-05}, {"N1"=179.503, "N2"=79.32, "N3"=0.00010060522661631534, "N4"=-1.0461271615126765e-05}, {"N1"=179.503, "N2"=81.658, "N3"=0.00010057766342038517, "N4"=-1.0413113813839867e-05}, {"N1"=179.503, "N2"=84.508, "N3"=0.00010069252694269775, "N4"=-1.0398580251867144e-05}, {"N1"=179.503, "N2"=86.68, "N3"=0.00010059231391507116, "N4"=-1.044539416751534e-05}, {"N1"=179.503, "N2"=89.35, "N3"=0.00010048971129646124, "N4"=-1.0268819117500044e-05}, {"N1"=177.025, "N2"=89.498, "N3"=0.00010060618454866035, "N4"=-1.0371231194086334e-05}, {"N1"=177.025, "N2"=87.264, "N3"=0.00010057510843963045, "N4"=-1.0225328126104061e-05}, {"N1"=177.025, "N2"=84.856, "N3"=0.0001005685693757888, "N4"=-1.018497459984881e-05}, {"N1"=177.025, "N2"=81.991, "N3"=0.0001006204574554324, "N4"=-1.031876629735078e-05}, {"N1"=177.025, "N2"=79.714, "N3"=0.0001005650653539355, "N4"=-1.0300677403340528e-05}, {"N1"=177.025, "N2"=77.318, "N3"=0.00010043209269920212, "N4"=-1.029537108597193e-05}, {"N1"=177.025, "N2"=74.497, "N3"=0.00010049008523085714, "N4"=-1.0465378307644795e-05}, {"N1"=177.025, "N2"=71.997, "N3"=0.00010054503295847881, "N4"=-1.0422497997885621e-05}, {"N1"=177.025, "N2"=69.505, "N3"=0.00010049241157570501, "N4"=-1.0506515638655537e-05}, {"N1"=177.025, "N2"=67.036, "N3"=0.00010049802689116723, "N4"=-1.0254992435638624e-05}, {"N1"=177.025, "N2"=64.524, "N3"=0.00010055511045977823, "N4"=-1.0471541695994191e-05}, {"N1"=174.508, "N2"=64.524, "N3"=0.00010058442377447452, "N4"=-1.0265602103734435e-05}, {"N1"=174.508, "N2"=66.824, "N3"=0.00010060549659099618, "N4"=-1.0335393232345529e-05}, {"N1"=174.508, "N2"=69.52, "N3"=0.00010056961567867355, "N4"=-1.03139183475667e-05}, {"N1"=174.508, "N2"=72.009, "N3"=0.00010050525424298924, "N4"=-1.0471776431016364e-05}, {"N1"=174.508, "N2"=74.5, "N3"=0.00010055674082340847, "N4"=-1.0297914935022879e-05}, {"N1"=174.508, "N2"=76.802, "N3"=0.00010057488934929836, "N4"=-1.0349374017560867e-05}, {"N1"=174.508, "N2"=79.236, "N3"=0.00010045680590912412, "N4"=-1.0322793862780694e-05}, {"N1"=174.508, "N2"=81.867, "N3"=0.00010043564909997728, "N4"=-1.0303026661889269e-05}, {"N1"=174.508, "N2"=84.493, "N3"=0.00010053298385350193, "N4"=-1.0386051365001408e-05}, {"N1"=174.508, "N2"=86.994, "N3"=0.00010053200300050581, "N4"=-1.0328246222436942e-05}, {"N1"=174.508, "N2"=89.508, "N3"=0.00010055825595324877, "N4"=-1.0359151928951748e-05}, {"N1"=172.007, "N2"=89.492, "N3"=0.00010063203033637178, "N4"=-1.0327706829098011e-05}, {"N1"=172.007, "N2"=87.298, "N3"=0.00010048876122707189, "N4"=-1.0389142662693645e-05}, {"N1"=172.007, "N2"=84.787, "N3"=0.00010047819419267379, "N4"=-1.0360910545361936e-05}, {"N1"=172.007, "N2"=82.322, "N3"=0.00010054374530748202, "N4"=-1.0332833010349498e-05}, {"N1"=172.007, "N2"=79.933, "N3"=0.00010059860927256583, "N4"=-1.0495770678229992e-05}, {"N1"=172.007, "N2"=77.048, "N3"=0.00010050973067817493, "N4"=-1.0373769938330423e-05}, {"N1"=172.007, "N2"=74.5, "N3"=0.00010052776184992925, "N4"=-1.0329652120112693e-05}, {"N1"=172.007, "N2"=72.003, "N3"=0.00010051195382604792, "N4"=-1.030155450789321e-05}, {"N1"=172.007, "N2"=69.502, "N3"=0.00010057737153872506, "N4"=-1.0406750813701743e-05}, {"N1"=172.007, "N2"=67.281, "N3"=0.00010053398890493448, "N4"=-1.0261150031855245e-05}, {"N1"=172.007, "N2"=64.498, "N3"=0.00010060849661348991, "N4"=-1.031575763252827e-05}, {"N1"=169.502, "N2"=64.525, "N3"=0.00010054683702601303, "N4"=-1.0370137456722481e-05}, {"N1"=169.502, "N2"=66.705, "N3"=0.00010058528937249951, "N4"=-1.0293815086596263e-05}, {"N1"=169.502, "N2"=69.48, "N3"=0.00010057189043098801, "N4"=-1.0309919001522938e-05}, {"N1"=169.502, "N2"=72.019, "N3"=0.00010059753324136094, "N4"=-1.0271135721251809e-05}, {"N1"=169.502, "N2"=74.4, "N3"=0.0001005185725337175, "N4"=-1.0524089497531527e-05}, {"N1"=169.502, "N2"=76.985, "N3"=0.00010050824590943186, "N4"=-1.0323707397510927e-05}, {"N1"=169.502, "N2"=79.494, "N3"=0.00010061569883517271, "N4"=-1.0430429858222473e-05}, {"N1"=169.502, "N2"=81.711, "N3"=0.00010068521739159446, "N4"=-1.0375009521526162e-05}, {"N1"=169.502, "N2"=84.526, "N3"=0.00010057546661980447, "N4"=-1.048782298781082e-05}, {"N1"=169.502, "N2"=87.001, "N3"=0.00010062622101785718, "N4"=-1.0388108016666844e-05}, {"N1"=169.502, "N2"=89.271, "N3"=0.00010055616555887019, "N4"=-1.033895491044533e-05}, {"N1"=167.005, "N2"=89.508, "N3"=0.00010055746015128895, "N4"=-1.0238378697299005e-05}, {"N1"=167.005, "N2"=87.002, "N3"=0.00010070615682900987, "N4"=-1.0358853090244672e-05}, {"N1"=167.005, "N2"=84.501, "N3"=0.00010048217565123469, "N4"=-1.0392975117995525e-05}, {"N1"=167.005, "N2"=82.374, "N3"=0.00010061420096214566, "N4"=-1.051369939236666e-05}, {"N1"=167.005, "N2"=79.7, "N3"=0.00010058672720208782, "N4"=-1.03232323866168e-05}, {"N1"=167.005, "N2"=77.011, "N3"=0.00010050169575191754, "N4"=-1.032033897095732e-05}, {"N1"=167.005, "N2"=74.756, "N3"=0.0001007119468191676, "N4"=-1.0343831292146167e-05}, {"N1"=167.005, "N2"=72.038, "N3"=0.00010040373607560784, "N4"=-1.058028106504143e-05}, {"N1"=167.005, "N2"=69.847, "N3"=0.00010054577185633803, "N4"=-1.037811124380008e-05}, {"N1"=167.005, "N2"=67.414, "N3"=0.00010056868380268909, "N4"=-1.0272744913655757e-05}, {"N1"=167.005, "N2"=64.501, "N3"=0.00010057363754714859, "N4"=-1.0397242170889903e-05}, {"N1"=164.505, "N2"=64.518, "N3"=0.00010044004683687069, "N4"=-1.028603303927345e-05}, {"N1"=164.505, "N2"=66.758, "N3"=0.00010058509910058875, "N4"=-1.0374163484188778e-05}, {"N1"=164.505, "N2"=69.112, "N3"=0.00010050825134333576, "N4"=-1.0333402406292994e-05}, {"N1"=164.505, "N2"=71.993, "N3"=0.00010054040915011839, "N4"=-1.0497567414438182e-05}, {"N1"=164.505, "N2"=74.397, "N3"=0.00010054122780018578, "N4"=-1.0339260857338038e-05}, {"N1"=164.505, "N2"=76.994, "N3"=0.00010060326598119498, "N4"=-1.0527681852640668e-05}, {"N1"=164.505, "N2"=79.503, "N3"=0.00010046474291687741, "N4"=-1.0260425970497155e-05}, {"N1"=164.505, "N2"=81.873, "N3"=0.00010056650989864249, "N4"=-1.0367701953412877e-05}, {"N1"=164.505, "N2"=84.278, "N3"=0.00010069327471749918, "N4"=-1.0299978353635183e-05}, {"N1"=164.505, "N2"=87.002, "N3"=0.00010055633707278133, "N4"=-1.04525051468583e-05}, {"N1"=164.505, "N2"=89.246, "N3"=0.00010059900386763756, "N4"=-1.0222708643708766e-05}, {"N1"=162.021, "N2"=89.501, "N3"=0.00010055905888410154, "N4"=-1.0383167945725405e-05}, {"N1"=162.021, "N2"=86.999, "N3"=0.00010049836016716291, "N4"=-1.0344028905420932e-05}, {"N1"=162.021, "N2"=84.479, "N3"=0.00010065865893854313, "N4"=-1.029031910432269e-05}, {"N1"=162.021, "N2"=82.334, "N3"=0.00010060171073522291, "N4"=-1.031179676129115e-05}, {"N1"=162.021, "N2"=79.722, "N3"=0.00010055161232195931, "N4"=-1.0410237870902512e-05}, {"N1"=162.021, "N2"=77.33, "N3"=0.00010056329704811053, "N4"=-1.0424688690105853e-05}, {"N1"=162.021, "N2"=74.499, "N3"=0.00010064834110723014, "N4"=-1.0253179379907153e-05}, {"N1"=162.021, "N2"=72.164, "N3"=0.00010050968622089045, "N4"=-1.0304515033076581e-05}, {"N1"=162.021, "N2"=69.517, "N3"=0.0001006460174419785, "N4"=-1.0319282055668342e-05}, {"N1"=162.021, "N2"=67.273, "N3"=0.00010059532093116402, "N4"=-1.0359489066628755e-05}, {"N1"=162.021, "N2"=64.491, "N3"=0.00010055335726968501, "N4"=-1.0375397216295825e-05}, {"N1"=159.508, "N2"=64.529, "N3"=0.00010058220947958114, "N4"=-1.0409654073027485e-05}, {"N1"=159.508, "N2"=66.608, "N3"=0.00010051924034481212, "N4"=-1.0559200871671656e-05}, {"N1"=159.508, "N2"=69.256, "N3"=0.000100615955350755, "N4"=-1.0411918977297675e-05}, {"N1"=159.508, "N2"=71.794, "N3"=0.0001005186441244473, "N4"=-1.0305323618103925e-05}, {"N1"=159.508, "N2"=74.288, "N3"=0.00010038751051594126, "N4"=-1.0460520801557472e-05}, {"N1"=159.508, "N2"=76.997, "N3"=0.00010058454495070586, "N4"=-1.0434871716286152e-05}, {"N1"=159.508, "N2"=79.495, "N3"=0.00010058453901491224, "N4"=-1.0393787876144356e-05}, {"N1"=159.508, "N2"=81.774, "N3"=0.00010046879993332481, "N4"=-1.0258755801039191e-05}, {"N1"=159.508, "N2"=84.345, "N3"=0.00010062366311837281, "N4"=-1.0232208681591546e-05}, {"N1"=159.508, "N2"=86.676, "N3"=0.00010063829099980864, "N4"=-1.0368738311184274e-05}, {"N1"=159.508, "N2"=89.366, "N3"=0.00010062332445066576, "N4"=-1.0288054360646662e-05}, {"N1"=157.01, "N2"=89.366, "N3"=0.00010063216609520602, "N4"=-1.0366590924044708e-05}, {"N1"=157.01, "N2"=87.038, "N3"=0.00010062377070477484, "N4"=-1.0259742326928577e-05}, {"N1"=157.01, "N2"=84.503, "N3"=0.00010055391234922045, "N4"=-1.0326654697798581e-05}, {"N1"=157.01, "N2"=82.261, "N3"=0.0001005896288054743, "N4"=-1.0170121633197498e-05}, {"N1"=157.01, "N2"=79.5, "N3"=0.0001005675395538572, "N4"=-1.0355383724985741e-05}, {"N1"=157.01, "N2"=77.011, "N3"=0.00010044278409493319, "N4"=-1.034540281846942e-05}, {"N1"=157.01, "N2"=74.522, "N3"=0.0001006017918027428, "N4"=-1.0410648176801857e-05}, {"N1"=157.01, "N2"=71.989, "N3"=0.0001006871321519983, "N4"=-1.0447830822041254e-05}, {"N1"=157.01, "N2"=69.44, "N3"=0.00010047733555323425, "N4"=-1.0352021411602509e-05}, {"N1"=157.01, "N2"=67.021, "N3"=0.00010063259498380248, "N4"=-1.0369864678277793e-05}, {"N1"=157.01, "N2"=64.47, "N3"=0.00010054128894894425, "N4"=-1.0349513973693469e-05}, {"N1"=154.508, "N2"=64.497, "N3"=0.00010058742278479965, "N4"=-1.043268893895931e-05}, {"N1"=154.508, "N2"=66.632, "N3"=0.00010057605131771914, "N4"=-1.0472163804897722e-05}, {"N1"=154.508, "N2"=69.157, "N3"=0.0001005754932818997, "N4"=-1.052486689613068e-05}, {"N1"=154.508, "N2"=72.002, "N3"=0.00010051158349612883, "N4"=-1.043815035637486e-05}, {"N1"=154.508, "N2"=74.507, "N3"=0.0001006876921083139, "N4"=-1.039748449678052e-05}, {"N1"=154.508, "N2"=76.982, "N3"=0.00010058681115521638, "N4"=-1.0472693776308262e-05}, {"N1"=154.508, "N2"=79.392, "N3"=0.0001005541671659117, "N4"=-1.0504080827325662e-05}, {"N1"=154.508, "N2"=81.991, "N3"=0.00010054442882218008, "N4"=-1.0354346083750894e-05}, {"N1"=154.508, "N2"=84.377, "N3"=0.00010050536334402543, "N4"=-1.040163233595326e-05}, {"N1"=154.508, "N2"=86.78, "N3"=0.00010045068223784615, "N4"=-1.037975022275213e-05}, {"N1"=154.508, "N2"=89.297, "N3"=0.00010059722699638339, "N4"=-1.0364877935260277e-05}, {"N1"=152.008, "N2"=89.496, "N3"=0.00010052916265034106, "N4"=-1.0356259089907488e-05}, {"N1"=152.008, "N2"=87.027, "N3"=0.00010055355037465621, "N4"=-1.0394689698756681e-05}, {"N1"=152.008, "N2"=84.502, "N3"=0.00010051462109257033, "N4"=-1.0391057887481473e-05}, {"N1"=152.008, "N2"=82.342, "N3"=0.00010057255034859199, "N4"=-1.0443052617878978e-05}, {"N1"=152.008, "N2"=79.498, "N3"=0.00010049361733670868, "N4"=-1.0075862343825072e-05}, {"N1"=152.008, "N2"=76.991, "N3"=0.00010048952736481864, "N4"=-1.0429041716639411e-05}, {"N1"=152.008, "N2"=74.53, "N3"=0.00010054597131692924, "N4"=-1.038281981980344e-05}, {"N1"=152.008, "N2"=72.287, "N3"=0.00010051822579456211, "N4"=-1.0300216981003882e-05}, {"N1"=152.008, "N2"=69.513, "N3"=0.00010055985014127507, "N4"=-1.0377012189536592e-05}, {"N1"=152.008, "N2"=67.004, "N3"=0.00010056119554619893, "N4"=-1.04417746693229e-05}, {"N1"=152.008, "N2"=64.534, "N3"=0.00010053739074560734, "N4"=-1.023587720430397e-05}, {"N1"=149.619, "N2"=64.504, "N3"=0.00010061252828025033, "N4"=-1.0559659891738197e-05}, {"N1"=149.619, "N2"=66.605, "N3"=0.00010060023951287196, "N4"=-1.0309522827413073e-05}, {"N1"=149.619, "N2"=69.495, "N3"=0.0001005216016225172, "N4"=-1.0172256394895664e-05}, {"N1"=149.619, "N2"=72.003, "N3"=0.00010038723155643375, "N4"=-1.0335554165351732e-05}, {"N1"=149.619, "N2"=74.404, "N3"=0.00010062409473556875, "N4"=-1.059015536094174e-05}, {"N1"=149.619, "N2"=76.728, "N3"=0.00010059828984453887, "N4"=-1.047656158213085e-05}, {"N1"=149.619, "N2"=79.496, "N3"=0.0001005060711540597, "N4"=-1.0329403959264902e-05}, {"N1"=149.619, "N2"=81.871, "N3"=0.00010053106990657012, "N4"=-1.0441724821028686e-05}, {"N1"=149.619, "N2"=84.308, "N3"=0.00010043043735246, "N4"=-1.0466751074281351e-05}, {"N1"=149.619, "N2"=86.692, "N3"=0.00010056624561014778, "N4"=-1.0605117016603453e-05}, {"N1"=149.619, "N2"=89.261, "N3"=0.0001007245704509603, "N4"=-1.0358427367549496e-05}, {"N1"=147.005, "N2"=89.514, "N3"=0.00010054788293493557, "N4"=-1.0465707937829983e-05}, {"N1"=147.005, "N2"=87.318, "N3"=0.00010067747498786916, "N4"=-1.0449256220258553e-05}, {"N1"=147.005, "N2"=84.97, "N3"=0.0001005471351982552, "N4"=-1.0325399204829004e-05}, {"N1"=147.005, "N2"=82.459, "N3"=0.0001006336050149554, "N4"=-1.0312722372735097e-05}, {"N1"=147.005, "N2"=79.496, "N3"=0.00010057255386028244, "N4"=-1.0344660957195826e-05}, {"N1"=147.005, "N2"=76.982, "N3"=0.00010057759239115202, "N4"=-1.0370210061721761e-05}, {"N1"=147.005, "N2"=74.702, "N3"=0.00010054433615195099, "N4"=-1.031799270277536e-05}, {"N1"=147.005, "N2"=72.278, "N3"=0.00010056781136823783, "N4"=-1.03095900815865e-05}, {"N1"=147.005, "N2"=70.089, "N3"=0.00010070615191175957, "N4"=-1.033377084890516e-05}, {"N1"=147.005, "N2"=67.307, "N3"=0.00010058128746386446, "N4"=-1.0444745911001558e-05}, {"N1"=147.118, "N2"=64.488, "N3"=0.000100576975520853, "N4"=-1.037696059266248e-05}, {"N1"=182.012, "N2"=152.611, "N3"=0.00010055273278373869, "N4"=-1.0408310537738696e-05}, {"N1"=182.012, "N2"=154.521, "N3"=0.00010056655571956805, "N4"=-1.0216076711249071e-05}, {"N1"=182.012, "N2"=157.019, "N3"=0.0001004627190886361, "N4"=-1.0528661328930298e-05}, {"N1"=182.012, "N2"=159.159, "N3"=0.00010054194119197448, "N4"=-1.0482959038998612e-05}, {"N1"=182.012, "N2"=161.982, "N3"=0.00010058221076553393, "N4"=-1.0317470544947592e-05}, {"N1"=182.012, "N2"=164.502, "N3"=0.00010056800492814469, "N4"=-1.0377751714809693e-05}, {"N1"=182.012, "N2"=166.904, "N3"=0.00010059709329404294, "N4"=-1.0364691330812088e-05}, {"N1"=182.012, "N2"=169.371, "N3"=0.0001005974575843628, "N4"=-1.0259290343015878e-05}, {"N1"=182.012, "N2"=171.997, "N3"=0.00010065865520086382, "N4"=-1.0410635835058914e-05}, {"N1"=182.012, "N2"=174.501, "N3"=0.0001005689954811829, "N4"=-1.0524764759634564e-05}, {"N1"=182.012, "N2"=176.701, "N3"=0.00010058564900218558, "N4"=-1.0358045979302124e-05}, {"N1"=182.012, "N2"=179.487, "N3"=0.0001005761639196866, "N4"=-1.0515876781309377e-05}, {"N1"=182.012, "N2"=181.998, "N3"=0.00010049371861045066, "N4"=-1.0261366670332017e-05}, {"N1"=179.504, "N2"=182.007, "N3"=0.00010053614047661596, "N4"=-1.044014033571524e-05}, {"N1"=179.504, "N2"=179.827, "N3"=0.00010051391831655712, "N4"=-1.0424197597054344e-05}, {"N1"=179.504, "N2"=176.956, "N3"=0.00010068079984430216, "N4"=-1.0227667218636083e-05}, {"N1"=179.504, "N2"=174.514, "N3"=0.00010049733005875758, "N4"=-1.035523428389971e-05}, {"N1"=179.504, "N2"=172.174, "N3"=0.00010058032892290357, "N4"=-1.0399169546890665e-05}, {"N1"=179.504, "N2"=169.502, "N3"=0.00010057418913917706, "N4"=-1.013360662580444e-05}, {"N1"=179.504, "N2"=167.252, "N3"=0.00010056731585418782, "N4"=-1.0448611950470434e-05}, {"N1"=179.504, "N2"=164.512, "N3"=0.00010059025588361039, "N4"=-1.0303488174053339e-05}, {"N1"=179.504, "N2"=162.068, "N3"=0.00010058875689560746, "N4"=-9.99043304684887e-06}, {"N1"=179.504, "N2"=159.491, "N3"=0.00010061354137906023, "N4"=-1.043460790607774e-05}, {"N1"=179.504, "N2"=157.22, "N3"=0.0001005621931456755, "N4"=-1.0360835824388902e-05}, {"N1"=179.504, "N2"=154.749, "N3"=0.0001006188684023702, "N4"=-1.0401023715949517e-05}, {"N1"=179.504, "N2"=152.204, "N3"=0.00010062366835214202, "N4"=-1.0421884559596913e-05}, {"N1"=177.006, "N2"=151.995, "N3"=0.00010058465638431029, "N4"=-1.0335842559258598e-05}, {"N1"=177.006, "N2"=154.396, "N3"=0.00010064048986834815, "N4"=-1.0419054431910744e-05}, {"N1"=177.006, "N2"=156.992, "N3"=0.00010070759447510396, "N4"=-1.049131453854165e-05}, {"N1"=177.006, "N2"=159.309, "N3"=0.00010058808962722079, "N4"=-1.039657704163045e-05}, {"N1"=177.006, "N2"=161.993, "N3"=0.00010069386264902427, "N4"=-1.0142245152433344e-05}, {"N1"=177.006, "N2"=164.281, "N3"=0.00010064613814311726, "N4"=-1.0347712971643544e-05}, {"N1"=177.006, "N2"=166.816, "N3"=0.00010053383469759641, "N4"=-1.0379028976706458e-05}, {"N1"=177.006, "N2"=169.292, "N3"=0.00010065689384258168, "N4"=-1.0345278335648412e-05}, {"N1"=177.006, "N2"=172.022, "N3"=0.00010059339792922846, "N4"=-1.0414143332488914e-05}, {"N1"=177.006, "N2"=174.29, "N3"=0.00010061108002761034, "N4"=-1.0514609177634065e-05}, {"N1"=177.006, "N2"=176.983, "N3"=0.00010067030682426444, "N4"=-1.0374197988561465e-05}, {"N1"=177.006, "N2"=178.925, "N3"=0.00010066950640410923, "N4"=-1.0392269856550798e-05}, {"N1"=177.006, "N2"=181.965, "N3"=0.00010051154842300859, "N4"=-1.035363274010177e-05}, {"N1"=174.535, "N2"=181.998, "N3"=0.00010052762174271708, "N4"=-1.0315700662767116e-05}, {"N1"=174.535, "N2"=179.507, "N3"=0.00010049881209647428, "N4"=-1.0464915893973651e-05}, {"N1"=174.535, "N2"=177.004, "N3"=0.00010065558772756656, "N4"=-1.0404842677178236e-05}, {"N1"=174.535, "N2"=174.498, "N3"=0.00010061016798809082, "N4"=-1.033869071584736e-05}, {"N1"=174.535, "N2"=172.23, "N3"=0.00010055953109317131, "N4"=-1.0294735150771711e-05}, {"N1"=174.535, "N2"=169.474, "N3"=0.00010053638717837301, "N4"=-1.0426220828840348e-05}, {"N1"=174.535, "N2"=167.212, "N3"=0.00010054711611366855, "N4"=-1.0288179033399426e-05}, {"N1"=174.535, "N2"=164.881, "N3"=0.0001005637441230306, "N4"=-1.0376406182987105e-05}, {"N1"=174.535, "N2"=162.178, "N3"=0.00010057630041995113, "N4"=-1.0333188832120185e-05}, {"N1"=174.535, "N2"=159.922, "N3"=0.00010051390612366023, "N4"=-1.03732462107962e-05}, {"N1"=174.535, "N2"=157.024, "N3"=0.00010052151661060848, "N4"=-1.0178899892628567e-05}, {"N1"=174.535, "N2"=154.742, "N3"=0.00010052568212633925, "N4"=-1.0336577309168365e-05}, {"N1"=174.535, "N2"=152.001, "N3"=0.00010043833567543106, "N4"=-1.0345716020400479e-05}, {"N1"=172.007, "N2"=151.993, "N3"=0.00010052091622244408, "N4"=-1.037796586495544e-05}, {"N1"=172.007, "N2"=154.261, "N3"=0.00010056042046810158, "N4"=-1.0331026431309562e-05}, {"N1"=172.007, "N2"=156.807, "N3"=0.00010052078834673039, "N4"=-1.0236069899038438e-05}, {"N1"=172.007, "N2"=159.134, "N3"=0.00010055899324905961, "N4"=-1.030433807189516e-05}, {"N1"=172.007, "N2"=161.987, "N3"=0.00010053597918022388, "N4"=-1.02501173014592e-05}, {"N1"=172.007, "N2"=164.278, "N3"=0.000100582114547373, "N4"=-1.0395954634842206e-05}, {"N1"=172.007, "N2"=167.0, "N3"=0.00010048467907552117, "N4"=-1.0313757712231493e-05}, {"N1"=172.007, "N2"=169.414, "N3"=0.00010057912792042218, "N4"=-1.0401981611189082e-05}, {"N1"=172.007, "N2"=171.78, "N3"=0.00010058536722138234, "N4"=-1.022592089962056e-05}, {"N1"=172.007, "N2"=174.418, "N3"=0.00010056524818285286, "N4"=-1.0555883638983451e-05}, {"N1"=172.007, "N2"=176.847, "N3"=0.00010048009637215594, "N4"=-1.0264985239173327e-05}, {"N1"=172.007, "N2"=179.499, "N3"=0.0001006041996268558, "N4"=-1.0386931447997637e-05}, {"N1"=172.007, "N2"=181.743, "N3"=0.00010058483003502757, "N4"=-1.033539560252702e-05}, {"N1"=169.511, "N2"=182.003, "N3"=0.0001006095386880882, "N4"=-1.0397496007975827e-05}, {"N1"=169.511, "N2"=179.724, "N3"=0.00010040829034856045, "N4"=-1.0402310925533099e-05}, {"N1"=169.511, "N2"=177.288, "N3"=0.0001005602775023726, "N4"=-1.0344480264179504e-05}, {"N1"=169.511, "N2"=174.502, "N3"=0.00010048213937989927, "N4"=-1.026176079311075e-05}, {"N1"=169.511, "N2"=172.408, "N3"=0.00010052120688560638, "N4"=-1.0409633619178077e-05}, {"N1"=169.511, "N2"=169.784, "N3"=0.00010056851888490843, "N4"=-1.0377628999671905e-05}, {"N1"=169.511, "N2"=167.224, "N3"=0.00010050211359977716, "N4"=-1.0512748060521344e-05}, {"N1"=169.511, "N2"=164.787, "N3"=0.00010057181541433262, "N4"=-1.042288722994474e-05}, {"N1"=169.511, "N2"=162.208, "N3"=0.00010057285277288677, "N4"=-1.0240506833313383e-05}, {"N1"=169.511, "N2"=159.929, "N3"=0.00010063847822573006, "N4"=-1.0286818897050851e-05}, {"N1"=169.511, "N2"=157.013, "N3"=0.00010043988380991298, "N4"=-1.038852685845044e-05}, {"N1"=169.511, "N2"=154.684, "N3"=0.00010054150477038508, "N4"=-1.0394937302553588e-05}, {"N1"=169.511, "N2"=152.303, "N3"=0.00010050107854436061, "N4"=-1.0356554570408694e-05}, {"N1"=167.008, "N2"=151.975, "N3"=0.00010065804591532068, "N4"=-1.0473499284903614e-05}, {"N1"=167.008, "N2"=154.281, "N3"=0.00010043280079178797, "N4"=-1.0388035735919689e-05}, {"N1"=167.008, "N2"=156.97, "N3"=0.0001005049187407278, "N4"=-1.0151105398959336e-05}, {"N1"=167.008, "N2"=159.168, "N3"=0.00010053391016644253, "N4"=-9.92503840144809e-06}, {"N1"=167.008, "N2"=161.748, "N3"=0.00010054044702236584, "N4"=-1.0377863950430322e-05}, {"N1"=167.008, "N2"=164.403, "N3"=0.00010056653769692994, "N4"=-1.0419094789339587e-05}, {"N1"=167.008, "N2"=166.864, "N3"=0.00010052741000594614, "N4"=-1.0124455762147418e-05}, {"N1"=167.008, "N2"=169.32, "N3"=0.0001005865975931813, "N4"=-1.0305890954236986e-05}, {"N1"=167.008, "N2"=171.787, "N3"=0.00010061330642759622, "N4"=-1.0257225208519041e-05}, {"N1"=167.008, "N2"=174.225, "N3"=0.00010048411635875578, "N4"=-1.0217662381425612e-05}, {"N1"=167.008, "N2"=176.792, "N3"=0.0001005693070561886, "N4"=-1.0213021913462708e-05}, {"N1"=167.008, "N2"=179.243, "N3"=0.00010053451649290888, "N4"=-1.0329012823308996e-05}, {"N1"=167.008, "N2"=181.729, "N3"=0.00010066065081120688, "N4"=-1.0493101769788713e-05}, {"N1"=164.51, "N2"=182.003, "N3"=0.00010058644189508781, "N4"=-1.0534583371748753e-05}, {"N1"=164.51, "N2"=179.494, "N3"=0.00010047532875861697, "N4"=-1.0320441834768146e-05}, {"N1"=164.51, "N2"=177.325, "N3"=0.00010059320676960861, "N4"=-1.0358395076057365e-05}, {"N1"=164.51, "N2"=174.834, "N3"=0.00010054372731298209, "N4"=-1.040873096506112e-05}, {"N1"=164.51, "N2"=172.15, "N3"=0.00010058291433696635, "N4"=-1.0184313976353813e-05}, {"N1"=164.51, "N2"=169.73, "N3"=0.00010064845886809261, "N4"=-1.0218453728016236e-05}, {"N1"=164.51, "N2"=167.039, "N3"=0.00010051874866106351, "N4"=-1.036866155552973e-05}, {"N1"=164.51, "N2"=164.719, "N3"=0.0001005647780331879, "N4"=-1.0228367487269825e-05}, {"N1"=164.51, "N2"=161.997, "N3"=0.00010070305115664577, "N4"=-1.0296255264737138e-05}, {"N1"=164.51, "N2"=159.871, "N3"=0.00010049964669458673, "N4"=-1.0616605005878712e-05}, {"N1"=164.51, "N2"=157.373, "N3"=0.00010050972698554164, "N4"=-1.030774489819331e-05}, {"N1"=164.51, "N2"=154.751, "N3"=0.00010058390297280664, "N4"=-1.0262379242022347e-05}, {"N1"=164.51, "N2"=152.344, "N3"=0.00010054924905839477, "N4"=-1.0563518384471683e-05}, {"N1"=162.009, "N2"=152.344, "N3"=0.0001005838648785531, "N4"=-1.0140418680852941e-05}, {"N1"=162.009, "N2"=154.493, "N3"=0.00010045565144201422, "N4"=-1.0345202237889113e-05}, {"N1"=162.009, "N2"=156.98, "N3"=0.0001005573067128509, "N4"=-1.029998197998634e-05}, {"N1"=162.009, "N2"=159.478, "N3"=0.00010036673714426203, "N4"=-1.0156282973690785e-05}, {"N1"=162.009, "N2"=161.958, "N3"=0.00010048540042336985, "N4"=-1.0399506130201608e-05}, {"N1"=162.009, "N2"=164.262, "N3"=0.00010061991373559685, "N4"=-1.0444457665240834e-05}, {"N1"=162.009, "N2"=166.85, "N3"=0.00010049639860075027, "N4"=-1.045305862910067e-05}, {"N1"=162.009, "N2"=169.347, "N3"=0.00010052351561037964, "N4"=-1.0184274437547899e-05}, {"N1"=162.009, "N2"=172.005, "N3"=0.00010056116542875544, "N4"=-1.0400976153311835e-05}, {"N1"=162.009, "N2"=174.21, "N3"=0.00010068390788027873, "N4"=-1.0255326298505552e-05}, {"N1"=162.009, "N2"=177.009, "N3"=0.0001005654883920819, "N4"=-1.0388144268547188e-05}, {"N1"=162.009, "N2"=179.386, "N3"=0.00010061309434455823, "N4"=-1.0531154999894492e-05}, {"N1"=162.009, "N2"=181.876, "N3"=0.00010059807898114881, "N4"=-1.0333029210150257e-05}, {"N1"=159.505, "N2"=182.002, "N3"=0.00010055723891507587, "N4"=-1.0318546030714028e-05}, {"N1"=159.505, "N2"=179.505, "N3"=0.00010046027729769476, "N4"=-1.0382956727671214e-05}, {"N1"=159.505, "N2"=177.231, "N3"=0.00010058221955045654, "N4"=-1.0434351774140535e-05}, {"N1"=159.505, "N2"=174.768, "N3"=0.00010063209262666011, "N4"=-1.0350089425412385e-05}, {"N1"=159.505, "N2"=172.352, "N3"=0.00010046025084146832, "N4"=-1.0329755908837778e-05}, {"N1"=159.505, "N2"=169.744, "N3"=0.00010059654554971513, "N4"=-1.0241273093192002e-05}, {"N1"=159.505, "N2"=167.018, "N3"=0.000100479958707661, "N4"=-1.0337587297327188e-05}, {"N1"=159.505, "N2"=164.748, "N3"=0.00010064692875075217, "N4"=-1.0245102370866817e-05}, {"N1"=159.505, "N2"=162.011, "N3"=0.00010050869279020892, "N4"=-1.0474623494397008e-05}, {"N1"=159.505, "N2"=159.877, "N3"=0.00010070627481461012, "N4"=-1.032540641702993e-05}, {"N1"=159.505, "N2"=157.405, "N3"=0.00010071054762358575, "N4"=-1.027765798450718e-05}, {"N1"=159.505, "N2"=154.737, "N3"=0.00010053402519125851, "N4"=-1.0509891274614203e-05}, {"N1"=159.505, "N2"=152.281, "N3"=0.00010062812666296488, "N4"=-1.044019968337579e-05}, {"N1"=157.011, "N2"=152.002, "N3"=0.0001005194015027839, "N4"=-1.0430277023516214e-05}, {"N1"=157.011, "N2"=154.502, "N3"=0.00010052981987561536, "N4"=-1.025224719428463e-05}, {"N1"=157.011, "N2"=156.649, "N3"=0.000100664982423806, "N4"=-1.0376498361488301e-05}, {"N1"=157.011, "N2"=159.501, "N3"=0.00010062713095967057, "N4"=-1.0509484487856454e-05}, {"N1"=157.011, "N2"=161.992, "N3"=0.00010052307864800399, "N4"=-1.0395547561060376e-05}, {"N1"=157.011, "N2"=164.318, "N3"=0.00010066038653681619, "N4"=-1.029675659740362e-05}, {"N1"=157.011, "N2"=166.897, "N3"=0.00010053632356016271, "N4"=-1.0374164340022899e-05}, {"N1"=157.011, "N2"=169.419, "N3"=0.00010049859835869724, "N4"=-1.0371437785845049e-05}, {"N1"=157.011, "N2"=171.88, "N3"=0.00010050306876779167, "N4"=-1.022335142529632e-05}, {"N1"=157.011, "N2"=174.293, "N3"=0.00010049440467144726, "N4"=-1.0223900522649466e-05}, {"N1"=157.011, "N2"=176.902, "N3"=0.00010062190913278209, "N4"=-1.045145236080008e-05}, {"N1"=157.011, "N2"=179.179, "N3"=0.00010041970507105444, "N4"=-1.0257525708310082e-05}, {"N1"=157.011, "N2"=182.022, "N3"=0.00010055201620996002, "N4"=-1.025273201986802e-05}, {"N1"=127.007, "N2"=181.98, "N3"=0.00010066967452682336, "N4"=-1.0220175988694377e-05}, {"N1"=127.007, "N2"=179.71, "N3"=0.00010055538270612703, "N4"=-1.025609312780955e-05}, {"N1"=127.007, "N2"=177.003, "N3"=0.00010064307003744251, "N4"=-1.0394766220874339e-05}, {"N1"=127.007, "N2"=174.758, "N3"=0.00010065691572176585, "N4"=-1.0569369307369789e-05}, {"N1"=127.007, "N2"=171.989, "N3"=0.00010054302114903295, "N4"=-1.0278496859463441e-05}, {"N1"=127.007, "N2"=169.507, "N3"=0.00010052219109080995, "N4"=-1.0374154825409664e-05}, {"N1"=127.007, "N2"=167.296, "N3"=0.00010055625572461704, "N4"=-1.0338406912258674e-05}, {"N1"=127.007, "N2"=164.506, "N3"=0.00010061744105887757, "N4"=-1.0400707561427745e-05}, {"N1"=127.007, "N2"=162.004, "N3"=0.00010071314175082436, "N4"=-1.0132054198391493e-05}, {"N1"=127.007, "N2"=159.5, "N3"=0.00010055527946356487, "N4"=-1.0221145777137548e-05}, {"N1"=127.007, "N2"=157.002, "N3"=0.00010053989180110475, "N4"=-1.0238627656812452e-05}, {"N1"=127.007, "N2"=154.494, "N3"=0.00010046380864192742, "N4"=-1.0323179668306778e-05}, {"N1"=127.007, "N2"=152.004, "N3"=0.00010076251037812463, "N4"=-1.0397209083439456e-05}, {"N1"=124.509, "N2"=152.005, "N3"=0.00010055289537303127, "N4"=-1.0318149507704667e-05}, {"N1"=124.509, "N2"=154.278, "N3"=0.00010056906675676558, "N4"=-1.0241755929751154e-05}, {"N1"=124.509, "N2"=156.995, "N3"=0.00010057283915850164, "N4"=-1.0387271353474952e-05}, {"N1"=124.509, "N2"=159.329, "N3"=0.00010067012052758113, "N4"=-1.0098373201757675e-05}, {"N1"=124.509, "N2"=161.909, "N3"=0.00010059404518212576, "N4"=-1.0230107464653003e-05}, {"N1"=124.509, "N2"=164.353, "N3"=0.0001005730917827833, "N4"=-1.0265841012528947e-05}, {"N1"=124.509, "N2"=166.772, "N3"=0.00010060365168644365, "N4"=-1.0305625088300388e-05}, {"N1"=124.509, "N2"=169.285, "N3"=0.00010055978134938268, "N4"=-1.0440092767503536e-05}, {"N1"=124.509, "N2"=172.011, "N3"=0.00010051420045093946, "N4"=-1.0269949430347485e-05}, {"N1"=124.509, "N2"=174.395, "N3"=0.00010049360501534616, "N4"=-1.033682927176177e-05}, {"N1"=124.509, "N2"=177.001, "N3"=0.00010055855735030683, "N4"=-1.026728226442454e-05}, {"N1"=124.509, "N2"=179.217, "N3"=0.00010052691301909924, "N4"=-1.0123229513416078e-05}, {"N1"=124.509, "N2"=181.794, "N3"=0.00010053161204254887, "N4"=-1.0274482366371959e-05}, {"N1"=122.004, "N2"=182.006, "N3"=0.00010057713663278465, "N4"=-1.0377027274661478e-05}, {"N1"=122.004, "N2"=179.506, "N3"=0.00010056565797614752, "N4"=-1.0372199940521955e-05}, {"N1"=122.004, "N2"=177.01, "N3"=0.00010060151746974734, "N4"=-1.0388607239209304e-05}, {"N1"=122.004, "N2"=174.496, "N3"=0.00010054169938917225, "N4"=-1.0311827976359371e-05}, {"N1"=122.004, "N2"=172.001, "N3"=0.0001006434418902588, "N4"=-1.0355170897474064e-05}, {"N1"=122.004, "N2"=169.77, "N3"=0.000100558145454887, "N4"=-1.046164214171523e-05}, {"N1"=122.004, "N2"=167.31, "N3"=0.00010052510545142468, "N4"=-1.0331957985024297e-05}, {"N1"=122.004, "N2"=164.834, "N3"=0.00010061047949711061, "N4"=-1.032545212338667e-05}, {"N1"=122.004, "N2"=162.299, "N3"=0.00010057413186928892, "N4"=-1.0490653301006056e-05}, {"N1"=122.004, "N2"=159.809, "N3"=0.00010057262055880731, "N4"=-1.0360581022065193e-05}, {"N1"=122.004, "N2"=157.452, "N3"=0.00010057479045979356, "N4"=-1.0369045444105874e-05}, {"N1"=122.004, "N2"=154.845, "N3"=0.00010065951323108781, "N4"=-1.0228662645117242e-05}, {"N1"=122.004, "N2"=152.25, "N3"=0.00010067579688774562, "N4"=-1.0296467220094232e-05}, {"N1"=119.507, "N2"=152.001, "N3"=0.00010052817383513941, "N4"=-1.0389724821440452e-05}, {"N1"=119.507, "N2"=154.494, "N3"=0.00010058017163122574, "N4"=-1.0152733108088067e-05}, {"N1"=119.507, "N2"=156.785, "N3"=0.00010056519103290949, "N4"=-1.0288040660934445e-05}, {"N1"=119.507, "N2"=159.23, "N3"=0.00010059444682129899, "N4"=-1.0298177774956188e-05}, {"N1"=119.507, "N2"=161.993, "N3"=0.0001005203463430634, "N4"=-1.0185615245692898e-05}, {"N1"=119.507, "N2"=164.253, "N3"=0.00010066571589598315, "N4"=-1.0207348610608702e-05}, {"N1"=119.507, "N2"=166.823, "N3"=0.00010056864418895355, "N4"=-1.033267345830009e-05}, {"N1"=119.507, "N2"=169.278, "N3"=0.00010057864360744154, "N4"=-1.0277086614245395e-05}, {"N1"=119.507, "N2"=171.993, "N3"=0.00010066265875918596, "N4"=-1.029751357328337e-05}, {"N1"=119.507, "N2"=174.278, "N3"=0.00010060703030850649, "N4"=-1.0103391482026253e-05}, {"N1"=119.507, "N2"=176.998, "N3"=0.00010060025344344439, "N4"=-1.0323915711634079e-05}, {"N1"=119.507, "N2"=179.514, "N3"=0.00010057981625729959, "N4"=-1.0295503743191012e-05}, {"N1"=119.507, "N2"=181.675, "N3"=0.00010059327261484356, "N4"=-1.0428834837094947e-05}, {"N1"=117.007, "N2"=182.002, "N3"=0.00010061818343626208, "N4"=-1.0319901056366384e-05}, {"N1"=117.007, "N2"=179.851, "N3"=0.00010054985650052086, "N4"=-1.0139151259362754e-05}, {"N1"=117.007, "N2"=177.36, "N3"=0.00010062351150607574, "N4"=-1.0334951983724557e-05}, {"N1"=117.007, "N2"=174.534, "N3"=0.00010057227752130818, "N4"=-1.0292515733334306e-05}, {"N1"=117.007, "N2"=172.391, "N3"=0.00010066808612838374, "N4"=-1.0435468135302864e-05}, {"N1"=117.007, "N2"=169.503, "N3"=0.00010056843347508542, "N4"=-1.0489739905106059e-05}, {"N1"=117.007, "N2"=167.294, "N3"=0.00010059541206115747, "N4"=-1.037897687149665e-05}, {"N1"=117.007, "N2"=164.774, "N3"=0.00010050409926807748, "N4"=-1.0341059880821408e-05}, {"N1"=117.007, "N2"=162.008, "N3"=0.00010058359392534071, "N4"=-1.0478415008222957e-05}, {"N1"=117.007, "N2"=159.94, "N3"=0.00010053978570627231, "N4"=-1.0195104142266479e-05}, {"N1"=117.007, "N2"=157.468, "N3"=0.00010051485676268084, "N4"=-1.034759566346305e-05}, {"N1"=117.007, "N2"=154.711, "N3"=0.00010058288379158468, "N4"=-1.0244664241709425e-05}, {"N1"=117.007, "N2"=152.27, "N3"=0.00010065008790879852, "N4"=-1.0369873700764411e-05}, {"N1"=114.503, "N2"=152.018, "N3"=0.00010068431467890425, "N4"=-1.0254021790212383e-05}, {"N1"=114.503, "N2"=154.528, "N3"=0.00010063648586061624, "N4"=-1.0401640504030923e-05}, {"N1"=114.503, "N2"=156.994, "N3"=0.00010057438667298901, "N4"=-1.0286239676061815e-05}, {"N1"=114.503, "N2"=159.257, "N3"=0.00010056396828368788, "N4"=-1.0307452724514088e-05}, {"N1"=114.503, "N2"=161.72, "N3"=0.00010064475418264949, "N4"=-1.0304295957939977e-05}, {"N1"=114.503, "N2"=164.258, "N3"=0.00010056313134032531, "N4"=-1.0265622238591132e-05}, {"N1"=114.503, "N2"=166.668, "N3"=0.00010054206554045979, "N4"=-1.03577829325654e-05}, {"N1"=114.503, "N2"=168.921, "N3"=0.00010055263722193717, "N4"=-1.0240166845763056e-05}, {"N1"=114.503, "N2"=172.006, "N3"=0.00010059201181876049, "N4"=-1.0224358903848528e-05}, {"N1"=114.503, "N2"=174.205, "N3"=0.0001005777722337138, "N4"=-1.0295983590500779e-05}, {"N1"=114.503, "N2"=177.0, "N3"=0.00010063818422803006, "N4"=-1.0268253185394315e-05}, {"N1"=114.503, "N2"=179.336, "N3"=0.00010059059953981527, "N4"=-1.039412205429316e-05}, {"N1"=114.503, "N2"=181.793, "N3"=0.00010050182424797325, "N4"=-1.0293494403914489e-05}, {"N1"=112.001, "N2"=182.001, "N3"=0.00010058772052700467, "N4"=-1.0116996145843834e-05}, {"N1"=112.001, "N2"=179.736, "N3"=0.00010062770027443537, "N4"=-1.0394589470427061e-05}, {"N1"=112.001, "N2"=177.038, "N3"=0.00010049241913289186, "N4"=-1.0154728674995575e-05}, {"N1"=112.001, "N2"=174.505, "N3"=0.00010063028981436415, "N4"=-1.020454856739115e-05}, {"N1"=112.001, "N2"=172.268, "N3"=0.00010061659246320014, "N4"=-1.0266370303128043e-05}, {"N1"=112.001, "N2"=169.794, "N3"=0.00010064160852633623, "N4"=-1.0394536898233264e-05}, {"N1"=112.001, "N2"=167.006, "N3"=0.00010053190296396764, "N4"=-1.0298528321225881e-05}, {"N1"=112.001, "N2"=164.496, "N3"=0.00010056563349771668, "N4"=-1.0207391044562614e-05}, {"N1"=112.001, "N2"=162.414, "N3"=0.00010060633719081935, "N4"=-1.0240845650269418e-05}, {"N1"=112.001, "N2"=159.847, "N3"=0.00010056750058437907, "N4"=-1.022347948799072e-05}, {"N1"=112.001, "N2"=157.042, "N3"=0.00010063169467172565, "N4"=-1.0014326106408688e-05}, {"N1"=112.001, "N2"=154.72, "N3"=0.00010070283509249232, "N4"=-1.0219994933391487e-05}, {"N1"=112.001, "N2"=152.235, "N3"=0.00010051617793078027, "N4"=-9.985715127407607e-06}, {"N1"=109.503, "N2"=151.998, "N3"=0.00010064479545558171, "N4"=-1.019823804320326e-05}, {"N1"=109.503, "N2"=154.553, "N3"=0.00010047279421271291, "N4"=-1.0214967537903954e-05}, {"N1"=109.503, "N2"=157.015, "N3"=0.00010064125710251541, "N4"=-1.033262893440704e-05}, {"N1"=109.503, "N2"=159.501, "N3"=0.00010056605207760532, "N4"=-1.0050326295282882e-05}, {"N1"=109.503, "N2"=161.768, "N3"=0.00010060794445267047, "N4"=-1.0391545930470155e-05}, {"N1"=109.503, "N2"=164.311, "N3"=0.00010059434852723423, "N4"=-1.0154338884270507e-05}, {"N1"=109.503, "N2"=166.728, "N3"=0.00010051166299766488, "N4"=-1.0277169883596048e-05}, {"N1"=109.503, "N2"=169.341, "N3"=0.00010057169316557466, "N4"=-1.0213253273715291e-05}, {"N1"=109.503, "N2"=171.739, "N3"=0.00010058779134890114, "N4"=-1.0385291622614835e-05}, {"N1"=109.503, "N2"=174.183, "N3"=0.00010067913942708822, "N4"=-1.0270797434936313e-05}, {"N1"=109.503, "N2"=176.659, "N3"=0.00010058024764650308, "N4"=-1.0190941665468636e-05}, {"N1"=109.503, "N2"=179.505, "N3"=0.00010056550367754658, "N4"=-1.0351926966026093e-05}, {"N1"=109.503, "N2"=181.848, "N3"=0.00010060054708789, "N4"=-1.0382526391134081e-05}, {"N1"=107.007, "N2"=182.004, "N3"=0.0001006000455667911, "N4"=-1.015378722873713e-05}, {"N1"=107.007, "N2"=179.895, "N3"=0.00010052561134913114, "N4"=-1.0148921681179518e-05}, {"N1"=107.007, "N2"=177.287, "N3"=0.00010065412648543197, "N4"=-1.0258985312638265e-05}, {"N1"=107.007, "N2"=174.779, "N3"=0.00010066791920310797, "N4"=-1.0353637086780785e-05}, {"N1"=107.007, "N2"=172.252, "N3"=0.00010058023682484012, "N4"=-1.0318279193977408e-05}, {"N1"=107.007, "N2"=169.481, "N3"=0.00010063706509352364, "N4"=-1.0197247737394732e-05}, {"N1"=107.007, "N2"=167.481, "N3"=0.00010072604919962668, "N4"=-1.0372199018389237e-05}, {"N1"=107.007, "N2"=164.504, "N3"=0.00010060272558520007, "N4"=-1.0283276967420611e-05}, {"N1"=107.007, "N2"=162.41, "N3"=0.00010066468650682885, "N4"=-1.0281510362058396e-05}, {"N1"=107.007, "N2"=159.862, "N3"=0.00010055360467534195, "N4"=-1.0179858122773344e-05}, {"N1"=107.007, "N2"=156.988, "N3"=0.00010054736426164819, "N4"=-1.0153865620150245e-05}, {"N1"=107.007, "N2"=154.766, "N3"=0.0001006424414233881, "N4"=-1.014273009512474e-05}, {"N1"=107.007, "N2"=152.003, "N3"=0.00010064326729363789, "N4"=-1.034598843938665e-05}, {"N1"=146.999, "N2"=114.503, "N3"=0.00010060499770106316, "N4"=-1.0317076173852246e-05}, {"N1"=146.999, "N2"=111.989, "N3"=0.00010047583572364766, "N4"=-1.03994928026879e-05}, {"N1"=146.999, "N2"=109.53, "N3"=0.00010056748890579797, "N4"=-1.0362628901071797e-05}, {"N1"=146.999, "N2"=106.998, "N3"=0.0001005299083186239, "N4"=-1.0319567343808175e-05}, {"N1"=146.999, "N2"=104.693, "N3"=0.00010053513575496426, "N4"=-1.0312374890310944e-05}, {"N1"=146.999, "N2"=102.002, "N3"=0.00010055637248268927, "N4"=-1.0328987151737936e-05}, {"N1"=146.999, "N2"=99.466, "N3"=0.00010056296547858146, "N4"=-1.036130313154264e-05}, {"N1"=146.999, "N2"=97.303, "N3"=0.00010052119951464826, "N4"=-1.0275481300931123e-05}, {"N1"=146.999, "N2"=94.731, "N3"=0.00010068244026671613, "N4"=-1.06117423064434e-05}, {"N1"=146.999, "N2"=92.018, "N3"=0.0001004552952991342, "N4"=-1.0654054944551996e-05}, {"N1"=146.999, "N2"=89.5, "N3"=0.00010052150063502006, "N4"=-1.031630545163132e-05}, {"N1"=149.496, "N2"=89.5, "N3"=0.00010060504796829301, "N4"=-1.0299318883327083e-05}, {"N1"=149.496, "N2"=92.008, "N3"=0.00010051072029635824, "N4"=-1.0403256147104009e-05}, {"N1"=149.496, "N2"=94.283, "N3"=0.00010055444696055002, "N4"=-1.0518940524357734e-05}, {"N1"=149.496, "N2"=96.644, "N3"=0.00010064332893876944, "N4"=-1.0001216674626905e-05}, {"N1"=149.496, "N2"=99.17, "N3"=0.00010060793657365403, "N4"=-1.0275067239957101e-05}, {"N1"=149.496, "N2"=102.005, "N3"=0.0001005318022941122, "N4"=-1.0382527589088096e-05}, {"N1"=149.496, "N2"=104.497, "N3"=0.00010054079000820997, "N4"=-1.0544537688756178e-05}, {"N1"=149.496, "N2"=106.846, "N3"=0.00010043415997742106, "N4"=-1.0486591910841888e-05}, {"N1"=149.496, "N2"=109.257, "N3"=0.00010047973222052626, "N4"=-1.041296831386093e-05}, {"N1"=149.496, "N2"=111.86, "N3"=0.0001007007111001422, "N4"=-1.0281231289777976e-05}, {"N1"=149.496, "N2"=114.476, "N3"=0.00010050480021978257, "N4"=-1.0329033218604983e-05}, {"N1"=151.908, "N2"=114.506, "N3"=0.00010055656515645495, "N4"=-1.0020266230478073e-05}, {"N1"=151.908, "N2"=111.991, "N3"=0.00010056495506648089, "N4"=-1.0327543095226283e-05}, {"N1"=151.908, "N2"=109.497, "N3"=0.00010058706905136275, "N4"=-1.0365900866113115e-05}, {"N1"=151.908, "N2"=107.024, "N3"=0.00010051509340318225, "N4"=-1.0376536524763746e-05}, {"N1"=151.908, "N2"=104.891, "N3"=0.00010041706046621053, "N4"=-1.0316740908889466e-05}, {"N1"=151.908, "N2"=102.341, "N3"=0.00010050920824774616, "N4"=-1.0065406545552593e-05}, {"N1"=151.908, "N2"=99.956, "N3"=0.00010068041493594367, "N4"=-1.0389397204993474e-05}, {"N1"=151.908, "N2"=97.378, "N3"=0.0001006900423365571, "N4"=-1.0662835478619497e-05}, {"N1"=151.908, "N2"=94.523, "N3"=0.00010060966842381001, "N4"=-1.0410285085022189e-05}, {"N1"=151.908, "N2"=91.984, "N3"=0.00010068792556598615, "N4"=-1.0274635261056571e-05}, {"N1"=151.908, "N2"=89.699, "N3"=0.00010066185923758861, "N4"=-9.907377051691505e-06}, {"N1"=154.495, "N2"=89.503, "N3"=0.00010068253868042378, "N4"=-1.0495030963229954e-05}, {"N1"=154.495, "N2"=91.829, "N3"=0.00010078882479117923, "N4"=-1.0699169460155344e-05}, {"N1"=154.495, "N2"=94.117, "N3"=0.00010059461735619844, "N4"=-1.026890771828903e-05}, {"N1"=154.495, "N2"=97.011, "N3"=0.00010053202746382141, "N4"=-1.0344645710348867e-05}, {"N1"=154.495, "N2"=99.519, "N3"=0.00010053142546206444, "N4"=-1.0369638826065193e-05}, {"N1"=154.495, "N2"=101.998, "N3"=0.00010067871661700116, "N4"=-1.0374874269089218e-05}, {"N1"=154.495, "N2"=104.218, "N3"=0.00010072553753268753, "N4"=-1.0573427401765086e-05}, {"N1"=154.495, "N2"=107.001, "N3"=0.0001005573049878312, "N4"=-1.0221720030120929e-05}, {"N1"=154.495, "N2"=109.477, "N3"=0.0001007143346600422, "N4"=-1.0315424468920982e-05}, {"N1"=154.495, "N2"=111.798, "N3"=0.00010060679547104105, "N4"=-1.0492485481270145e-05}, {"N1"=154.495, "N2"=114.412, "N3"=0.00010046906821566981, "N4"=-1.023083318528866e-05}, {"N1"=156.996, "N2"=114.502, "N3"=0.00010055007321851584, "N4"=-1.052274942483182e-05}, {"N1"=156.996, "N2"=112.25, "N3"=0.00010057418626935975, "N4"=-1.0405543610434793e-05}, {"N1"=156.996, "N2"=109.676, "N3"=0.00010069179485446984, "N4"=-1.0379151706304188e-05}, {"N1"=156.996, "N2"=107.411, "N3"=0.00010058209465276414, "N4"=-1.0256652904447258e-05}, {"N1"=156.996, "N2"=104.812, "N3"=0.00010051735728992372, "N4"=-1.0376534442795295e-05}, {"N1"=156.996, "N2"=102.473, "N3"=0.00010059071085739439, "N4"=-1.02479410442246e-05}, {"N1"=156.996, "N2"=99.888, "N3"=0.00010052469801744513, "N4"=-1.0382065100851749e-05}, {"N1"=156.996, "N2"=96.999, "N3"=0.0001005415183791208, "N4"=-1.013971629911719e-05}, {"N1"=156.996, "N2"=94.456, "N3"=0.00010054257194928158, "N4"=-1.0226317752047225e-05}, {"N1"=156.996, "N2"=91.999, "N3"=0.00010062668881057213, "N4"=-1.0382610226950327e-05}, {"N1"=156.996, "N2"=89.497, "N3"=0.00010068589824330873, "N4"=-1.041429745330267e-05}, {"N1"=159.49, "N2"=89.514, "N3"=0.00010054182451209732, "N4"=-1.0395374993859549e-05}, {"N1"=159.49, "N2"=91.996, "N3"=0.00010054486127716693, "N4"=-1.0307167894579886e-05}, {"N1"=159.49, "N2"=94.25, "N3"=0.00010066637434498448, "N4"=-1.0136340878502978e-05}, {"N1"=159.49, "N2"=96.785, "N3"=0.00010056763970426168, "N4"=-1.0337906859028654e-05}, {"N1"=159.49, "N2"=98.566, "N3"=0.00010048567701356749, "N4"=-1.0346873370842697e-05}, {"N1"=159.49, "N2"=101.997, "N3"=0.00010065826315028559, "N4"=-1.0174631971257145e-05}, {"N1"=159.49, "N2"=104.506, "N3"=0.00010050570275674231, "N4"=-1.0379874853053304e-05}, {"N1"=159.49, "N2"=106.852, "N3"=0.0001005877573224815, "N4"=-1.026776664524608e-05}, {"N1"=159.49, "N2"=109.471, "N3"=0.00010058612875963466, "N4"=-1.0430394597249182e-05}, {"N1"=159.49, "N2"=111.868, "N3"=0.0001006541226677135, "N4"=-1.0230268960334434e-05}, {"N1"=159.49, "N2"=114.342, "N3"=0.0001005775105304762, "N4"=-1.0437108678183315e-05}, {"N1"=161.983, "N2"=114.507, "N3"=0.00010068371665082046, "N4"=-1.0445701995914409e-05}, {"N1"=161.983, "N2"=112.004, "N3"=0.00010052410901230568, "N4"=-1.0481194334898093e-05}, {"N1"=161.983, "N2"=109.489, "N3"=0.00010053260717008978, "N4"=-1.0642110397844789e-05}, {"N1"=161.983, "N2"=107.301, "N3"=0.000100640325155521, "N4"=-1.0374144854144585e-05}, {"N1"=161.983, "N2"=104.505, "N3"=0.00010047611407593544, "N4"=-1.0380815109538789e-05}, {"N1"=161.983, "N2"=102.017, "N3"=0.00010057110679466989, "N4"=-1.0420174110328346e-05}, {"N1"=161.983, "N2"=99.513, "N3"=0.00010055845295575355, "N4"=-1.03154613520224e-05}, {"N1"=161.983, "N2"=97.001, "N3"=0.00010057308979834507, "N4"=-1.0349930881454738e-05}, {"N1"=161.983, "N2"=94.499, "N3"=0.00010059409055654802, "N4"=-1.0029465881604357e-05}, {"N1"=161.983, "N2"=92.01, "N3"=0.00010056956364370521, "N4"=-1.0602775271067255e-05}, {"N1"=161.983, "N2"=89.898, "N3"=0.00010060244056346333, "N4"=-1.0638698777958477e-05}, {"N1"=164.496, "N2"=89.898, "N3"=0.00010048814396409382, "N4"=-1.0260437340010916e-05}, {"N1"=164.496, "N2"=92.007, "N3"=0.00010057011320489959, "N4"=-1.0642901694107624e-05}, {"N1"=164.496, "N2"=94.303, "N3"=0.00010058277958213819, "N4"=-1.0059975250910372e-05}, {"N1"=164.496, "N2"=96.719, "N3"=0.00010063913013417645, "N4"=-1.0637514624567747e-05}, {"N1"=164.496, "N2"=99.229, "N3"=0.00010052994145816619, "N4"=-1.0324964588086446e-05}, {"N1"=164.496, "N2"=101.835, "N3"=0.00010054225919419489, "N4"=-1.022470931712745e-05}, {"N1"=164.496, "N2"=104.366, "N3"=0.00010050480199991469, "N4"=-1.011263863189184e-05}, {"N1"=164.496, "N2"=106.998, "N3"=0.0001005543191480403, "N4"=-1.0414655531885156e-05}, {"N1"=164.496, "N2"=109.173, "N3"=0.00010053051225409979, "N4"=-1.0500326021179052e-05}, {"N1"=164.496, "N2"=111.739, "N3"=0.00010062423849062954, "N4"=-1.0613135323965765e-05}, {"N1"=164.496, "N2"=114.42, "N3"=0.00010063062561204481, "N4"=-1.058885887449276e-05}, {"N1"=166.994, "N2"=114.519, "N3"=0.00010051709293576832, "N4"=-1.0443402691016554e-05}, {"N1"=166.994, "N2"=112.33, "N3"=0.00010049375406009971, "N4"=-1.0740933275983281e-05}, {"N1"=166.994, "N2"=109.852, "N3"=0.00010052042976109586, "N4"=-1.0571157365927451e-05}, {"N1"=166.994, "N2"=107.002, "N3"=0.0001005949653323901, "N4"=-1.0415577576495951e-05}, {"N1"=166.994, "N2"=104.759, "N3"=0.00010055088701353558, "N4"=-1.0421181788351225e-05}, {"N1"=166.994, "N2"=102.327, "N3"=0.00010075376943781988, "N4"=-1.0417052859371254e-05}, {"N1"=166.994, "N2"=99.502, "N3"=0.0001006670723644356, "N4"=-1.0199569011228347e-05}, {"N1"=166.994, "N2"=97.268, "N3"=0.00010070266596724642, "N4"=-1.0393130558592505e-05}, {"N1"=166.994, "N2"=94.497, "N3"=0.00010051464624161111, "N4"=-1.0434830073153744e-05}, {"N1"=166.994, "N2"=92.044, "N3"=0.00010050716248067688, "N4"=-1.0349337942348713e-05}, {"N1"=166.994, "N2"=89.817, "N3"=0.00010066563636718391, "N4"=-1.0045009227877071e-05}, {"N1"=169.495, "N2"=89.486, "N3"=0.00010057320179739244, "N4"=-1.0227325730443702e-05}, {"N1"=169.495, "N2"=91.671, "N3"=0.00010069826294117365, "N4"=-1.063886211215806e-05}, {"N1"=169.495, "N2"=94.283, "N3"=0.00010058349482054724, "N4"=-1.0645406429609959e-05}, {"N1"=169.495, "N2"=96.819, "N3"=0.00010054384086763938, "N4"=-1.055977207209704e-05}, {"N1"=169.495, "N2"=99.226, "N3"=0.00010053929190141979, "N4"=-1.046351796738137e-05}, {"N1"=169.495, "N2"=102.002, "N3"=0.00010050597692589498, "N4"=-1.0037749856519407e-05}, {"N1"=169.495, "N2"=104.246, "N3"=0.00010060301951595907, "N4"=-1.0376405720979674e-05}, {"N1"=169.495, "N2"=106.804, "N3"=0.00010057429264822356, "N4"=-1.0167419264455338e-05}, {"N1"=169.495, "N2"=109.27, "N3"=0.00010050538878497119, "N4"=-1.0088713846005043e-05}, {"N1"=169.495, "N2"=112.026, "N3"=0.00010053910145648137, "N4"=-1.0394493351801651e-05}, {"N1"=169.495, "N2"=114.22, "N3"=0.00010052851417023094, "N4"=-1.0682873460167943e-05}, {"N1"=171.883, "N2"=114.507, "N3"=0.00010053712116719145, "N4"=-1.0266044088642181e-05}, {"N1"=171.883, "N2"=111.996, "N3"=0.0001005017439561145, "N4"=-1.0324547629284264e-05}, {"N1"=171.883, "N2"=109.848, "N3"=0.00010049948944593192, "N4"=-1.0206767308618884e-05}, {"N1"=171.883, "N2"=107.463, "N3"=0.00010052904871629471, "N4"=-1.038533145363368e-05}, {"N1"=171.883, "N2"=104.871, "N3"=0.0001005738260646754, "N4"=-1.0376004348811694e-05}, {"N1"=171.883, "N2"=101.991, "N3"=0.00010055372310088669, "N4"=-1.0250260450221826e-05}, {"N1"=171.883, "N2"=99.94, "N3"=0.00010059384998808005, "N4"=-1.0377346727853323e-05}, {"N1"=171.883, "N2"=97.323, "N3"=0.00010045260127290205, "N4"=-1.0142135108610598e-05}, {"N1"=171.883, "N2"=94.547, "N3"=0.00010056545431402706, "N4"=-1.0329684145398186e-05}, {"N1"=171.883, "N2"=92.259, "N3"=0.00010045935630986664, "N4"=-1.0476569179953833e-05}, {"N1"=171.883, "N2"=89.71, "N3"=0.00010053456463580633, "N4"=-1.0482807818304463e-05}, {"N1"=174.494, "N2"=89.504, "N3"=0.00010059148056849578, "N4"=-1.014857690287672e-05}, {"N1"=174.494, "N2"=91.742, "N3"=0.00010060176173810656, "N4"=-1.0322886507205224e-05}, {"N1"=174.494, "N2"=94.098, "N3"=0.0001005640572937127, "N4"=-1.0406357664570412e-05}, {"N1"=174.494, "N2"=97.009, "N3"=0.00010059732841583133, "N4"=-1.009206877841672e-05}, {"N1"=174.494, "N2"=99.498, "N3"=0.0001004866464273728, "N4"=-1.0385158848437636e-05}, {"N1"=174.494, "N2"=101.844, "N3"=0.0001004846690086862, "N4"=-1.0508972621384048e-05}, {"N1"=174.494, "N2"=104.48, "N3"=0.0001004879994441, "N4"=-1.0551649159602135e-05}, {"N1"=174.494, "N2"=106.817, "N3"=0.00010063513433150371, "N4"=-1.0415313534897814e-05}, {"N1"=174.494, "N2"=109.502, "N3"=0.00010052069776793929, "N4"=-1.0429211626997979e-05}, {"N1"=174.494, "N2"=111.991, "N3"=0.00010067569666507484, "N4"=-1.0419642235438489e-05}, {"N1"=174.494, "N2"=114.536, "N3"=0.00010081180105069445, "N4"=-1.0404705205815954e-05}, {"N1"=176.998, "N2"=114.513, "N3"=0.00010056115436641966, "N4"=-1.0292414962786945e-05}, {"N1"=176.998, "N2"=112.3, "N3"=0.00010055971217769431, "N4"=-1.0269561378937349e-05}, {"N1"=176.998, "N2"=109.691, "N3"=0.00010046435749747637, "N4"=-1.0388972064867833e-05}, {"N1"=176.998, "N2"=107.0, "N3"=0.00010054050728334219, "N4"=-1.0447588731418671e-05}, {"N1"=176.998, "N2"=104.801, "N3"=0.00010062624247864694, "N4"=-1.0425638948989608e-05}, {"N1"=176.998, "N2"=102.327, "N3"=0.00010055222900913126, "N4"=-1.0269352290753455e-05}, {"N1"=176.998, "N2"=99.501, "N3"=0.00010047325837555974, "N4"=-1.0143078887491751e-05}, {"N1"=176.998, "N2"=97.002, "N3"=0.00010062184796938916, "N4"=-1.0280035050657638e-05}, {"N1"=176.998, "N2"=94.439, "N3"=0.00010052864374345616, "N4"=-1.0484935932147626e-05}, {"N1"=176.998, "N2"=92.22, "N3"=0.00010054150201171854, "N4"=-1.0384158887893506e-05}, {"N1"=176.998, "N2"=89.894, "N3"=0.00010055443147564314, "N4"=-1.0381384344484938e-05}, {"N1"=179.496, "N2"=89.502, "N3"=0.00010065394787749831, "N4"=-1.0378615602595834e-05}, {"N1"=179.496, "N2"=91.852, "N3"=0.00010053848144487536, "N4"=-1.0296378167571764e-05}, {"N1"=179.496, "N2"=94.183, "N3"=0.00010049253126070856, "N4"=-1.0312313955952983e-05}, {"N1"=179.496, "N2"=96.792, "N3"=0.00010063655479762752, "N4"=-1.0087788581921771e-05}, {"N1"=179.496, "N2"=99.24, "N3"=0.00010048665002495486, "N4"=-1.0368882352837475e-05}, {"N1"=179.496, "N2"=101.709, "N3"=0.00010054720723223964, "N4"=-1.035151219891597e-05}, {"N1"=179.496, "N2"=104.504, "N3"=0.00010066468144814112, "N4"=-1.036751880342346e-05}, {"N1"=179.496, "N2"=106.617, "N3"=0.00010059194868342962, "N4"=-1.0624696758329911e-05}, {"N1"=179.496, "N2"=109.409, "N3"=0.00010058293048354515, "N4"=-1.013910783805464e-05}, {"N1"=179.496, "N2"=111.842, "N3"=0.00010063206794802302, "N4"=-1.0478987984529087e-05}, {"N1"=179.496, "N2"=114.279, "N3"=0.00010053290884922094, "N4"=-1.0748863794305894e-05}, {"N1"=181.991, "N2"=114.502, "N3"=0.00010060364155975004, "N4"=-1.0539738081964645e-05}, {"N1"=181.991, "N2"=112.198, "N3"=0.00010044157230260417, "N4"=-1.0392808573650057e-05}, {"N1"=181.991, "N2"=109.502, "N3"=0.00010048616274984088, "N4"=-1.022687623825104e-05}, {"N1"=181.991, "N2"=107.002, "N3"=0.00010055591333181053, "N4"=-1.0306410932815041e-05}, {"N1"=181.991, "N2"=104.82, "N3"=0.00010058368991156377, "N4"=-9.91636860521745e-06}, {"N1"=181.991, "N2"=101.992, "N3"=0.00010072475510736278, "N4"=-1.0830380233122652e-05}, {"N1"=181.991, "N2"=99.508, "N3"=0.00010069465835530913, "N4"=-1.044534956683265e-05}, {"N1"=181.991, "N2"=97.389, "N3"=0.00010057978082684279, "N4"=-1.0447508845920227e-05}, {"N1"=181.991, "N2"=94.528, "N3"=0.00010059037235251282, "N4"=-1.0624977651036895e-05}, {"N1"=181.991, "N2"=91.998, "N3"=0.00010057858186474582, "N4"=-1.0278923749840406e-05}, {"N1"=181.991, "N2"=89.84, "N3"=0.00010057553350288104, "N4"=-1.0378586094888816e-05}, {"N1"=184.416, "N2"=89.516, "N3"=0.00010056546088225978, "N4"=-1.0362901620447478e-05}, {"N1"=184.416, "N2"=91.572, "N3"=0.00010048195684120855, "N4"=-1.0260403305451498e-05}, {"N1"=184.416, "N2"=94.219, "N3"=0.00010067708016955082, "N4"=-1.0356189811758044e-05}, {"N1"=184.416, "N2"=96.978, "N3"=0.00010063069950031687, "N4"=-1.034572437768273e-05}, {"N1"=184.416, "N2"=99.511, "N3"=0.00010054426793166629, "N4"=-1.0578225410191917e-05}, {"N1"=184.416, "N2"=102.003, "N3"=0.00010053162118628789, "N4"=-1.031899599693824e-05}, {"N1"=184.416, "N2"=104.499, "N3"=0.0001005533942606881, "N4"=-1.0375560970319743e-05}, {"N1"=184.416, "N2"=106.852, "N3"=0.00010055278397039816, "N4"=-1.0064715694811877e-05}, {"N1"=184.416, "N2"=109.287, "N3"=0.00010065834392520048, "N4"=-1.0316757363626799e-05}, {"N1"=184.416, "N2"=112.001, "N3"=0.00010051492337315109, "N4"=-1.0520721690183389e-05}, {"N1"=184.416, "N2"=114.225, "N3"=0.00010057827621791868, "N4"=-1.0219484032027895e-05}, {"N1"=186.996, "N2"=114.503, "N3"=0.00010063677766509167, "N4"=-1.0181154686397127e-05}, {"N1"=186.996, "N2"=112.186, "N3"=0.00010058314272196287, "N4"=-1.0270785852024913e-05}, {"N1"=186.996, "N2"=109.69, "N3"=0.00010048588062443048, "N4"=-1.029598028684236e-05}, {"N1"=186.996, "N2"=107.408, "N3"=0.00010057368837517393, "N4"=-1.018049608359016e-05}, {"N1"=186.996, "N2"=104.885, "N3"=0.00010060216520685674, "N4"=-1.0312257789517935e-05}, {"N1"=186.996, "N2"=102.042, "N3"=0.00010058432475508994, "N4"=-1.0263384987111241e-05}, {"N1"=186.996, "N2"=99.781, "N3"=0.00010058699630838505, "N4"=-1.0352929066332636e-05}, {"N1"=186.996, "N2"=97.245, "N3"=0.00010046126662878602, "N4"=-1.0626292071846878e-05}, {"N1"=186.996, "N2"=94.498, "N3"=0.00010049120333482968, "N4"=-1.0074309920725545e-05}, {"N1"=186.996, "N2"=92.037, "N3"=0.0001004500649868954, "N4"=-1.0147416916329142e-05}, {"N1"=186.996, "N2"=89.777, "N3"=0.00010069084257118586, "N4"=-1.0339645045259801e-05}, {"N1"=186.996, "N2"=114.498, "N3"=0.00010062692650713552, "N4"=-1.0379146262324162e-05}, {"N1"=186.996, "N2"=116.841, "N3"=0.00010053712096639657, "N4"=-1.0690314902457516e-05}, {"N1"=186.996, "N2"=119.513, "N3"=0.00010065001964136715, "N4"=-1.0242509050843946e-05}, {"N1"=186.996, "N2"=121.875, "N3"=0.00010056583126694079, "N4"=-1.0488769368813804e-05}, {"N1"=186.996, "N2"=124.491, "N3"=0.00010056467831802905, "N4"=-1.0566488413214566e-05}, {"N1"=186.996, "N2"=126.597, "N3"=0.00010049702603825771, "N4"=-1.0686143271586093e-05}, {"N1"=186.996, "N2"=129.501, "N3"=0.00010050459932822164, "N4"=-1.0112848519342277e-05}, {"N1"=186.996, "N2"=131.758, "N3"=0.00010061165238247087, "N4"=-1.0257148823475635e-05}, {"N1"=186.996, "N2"=134.503, "N3"=0.00010059379878020946, "N4"=-1.0292138802663583e-05}, {"N1"=186.996, "N2"=136.697, "N3"=0.0001005177884080994, "N4"=-1.0301529666777696e-05}, {"N1"=186.996, "N2"=139.5, "N3"=0.00010061551648413663, "N4"=-1.0285601009784287e-05}, {"N1"=189.493, "N2"=139.521, "N3"=0.00010065811968121243, "N4"=-1.0474173429681113e-05}, {"N1"=189.493, "N2"=137.255, "N3"=0.00010043239961442407, "N4"=-1.0284677089965968e-05}, {"N1"=189.493, "N2"=134.677, "N3"=0.0001006364092371449, "N4"=-1.0350646107511002e-05}, {"N1"=189.493, "N2"=132.193, "N3"=0.00010047751229100592, "N4"=-1.0246513417188419e-05}, {"N1"=189.493, "N2"=129.515, "N3"=0.00010058039498042905, "N4"=-1.0345678555264667e-05}, {"N1"=189.493, "N2"=126.972, "N3"=0.00010041425246450131, "N4"=-1.0511496380684028e-05}, {"N1"=189.493, "N2"=124.542, "N3"=0.00010045810385222098, "N4"=-1.0313667849160737e-05}, {"N1"=189.493, "N2"=122.316, "N3"=0.00010053537625529291, "N4"=-1.008468362982841e-05}, {"N1"=189.493, "N2"=119.535, "N3"=0.00010052620281201316, "N4"=-1.0293990137032178e-05}, {"N1"=189.493, "N2"=117.021, "N3"=0.00010064299442268789, "N4"=-1.0139610194727024e-05}, {"N1"=189.493, "N2"=114.489, "N3"=0.00010051170749224173, "N4"=-1.0180389026308908e-05}, {"N1"=191.982, "N2"=114.5, "N3"=0.00010059548086192432, "N4"=-1.0344277489752226e-05}, {"N1"=191.982, "N2"=117.013, "N3"=0.00010063536335575964, "N4"=-1.0231229821765076e-05}, {"N1"=191.982, "N2"=119.493, "N3"=0.00010055503695570355, "N4"=-1.0439974054199725e-05}, {"N1"=191.982, "N2"=121.985, "N3"=0.00010055660843981584, "N4"=-1.0345288170957576e-05}, {"N1"=191.982, "N2"=124.318, "N3"=0.0001006575870044503, "N4"=-1.0464226191733627e-05}, {"N1"=191.982, "N2"=126.785, "N3"=0.00010065042167491977, "N4"=-1.0569824372843455e-05}, {"N1"=191.982, "N2"=129.309, "N3"=0.0001005756119552502, "N4"=-1.0615747704357023e-05}, {"N1"=191.982, "N2"=131.72, "N3"=0.00010055452017268634, "N4"=-1.0528711529329893e-05}, {"N1"=191.982, "N2"=134.192, "N3"=0.000100497370641192, "N4"=-1.0270525359081904e-05}, {"N1"=191.982, "N2"=136.758, "N3"=0.00010058151015600906, "N4"=-1.0522709848811357e-05}, {"N1"=191.982, "N2"=139.483, "N3"=0.00010054923431037895, "N4"=-1.0292347101408578e-05}, {"N1"=194.498, "N2"=139.494, "N3"=0.00010055597188211656, "N4"=-1.0243413970924894e-05}, {"N1"=194.498, "N2"=137.198, "N3"=0.00010052169517802965, "N4"=-1.0269947005969802e-05}, {"N1"=194.498, "N2"=134.727, "N3"=0.00010038533466469408, "N4"=-1.0461920879690848e-05}, {"N1"=194.498, "N2"=132.021, "N3"=0.00010047264491826939, "N4"=-1.0402079004565774e-05}, {"N1"=194.498, "N2"=129.847, "N3"=0.00010051765809288875, "N4"=-1.0272964612445752e-05}, {"N1"=194.498, "N2"=127.001, "N3"=0.00010052524486754333, "N4"=-1.0410412930987889e-05}, {"N1"=194.498, "N2"=124.48, "N3"=0.00010055237701232716, "N4"=-1.03785400943151e-05}, {"N1"=194.498, "N2"=122.319, "N3"=0.00010057035390823348, "N4"=-1.0244872409892844e-05}, {"N1"=194.498, "N2"=119.71, "N3"=0.00010052452518299726, "N4"=-1.030883393829317e-05}, {"N1"=194.498, "N2"=117.002, "N3"=0.00010051364548228354, "N4"=-1.0235349706588265e-05}, {"N1"=194.498, "N2"=114.499, "N3"=0.00010062744144064514, "N4"=-1.0497505877162535e-05}, {"N1"=196.972, "N2"=114.499, "N3"=0.00010053100385870424, "N4"=-1.0353452037182097e-05}, {"N1"=196.972, "N2"=116.976, "N3"=0.00010059972183768522, "N4"=-1.0329883461385281e-05}, {"N1"=196.972, "N2"=119.511, "N3"=0.00010062749897995651, "N4"=-1.0250311766008719e-05}, {"N1"=196.972, "N2"=121.995, "N3"=0.00010051258287875067, "N4"=-1.0365730668014968e-05}, {"N1"=196.972, "N2"=124.267, "N3"=0.00010061815081609635, "N4"=-1.055952597950726e-05}, {"N1"=196.972, "N2"=127.008, "N3"=0.00010050307177341909, "N4"=-1.0385253618167535e-05}, {"N1"=196.972, "N2"=129.196, "N3"=0.00010060421668027115, "N4"=-1.0246003522387107e-05}, {"N1"=196.972, "N2"=131.786, "N3"=0.00010056402361198962, "N4"=-1.026584685311642e-05}, {"N1"=196.972, "N2"=134.265, "N3"=0.00010055649605186719, "N4"=-1.0644970161274753e-05}, {"N1"=196.972, "N2"=136.783, "N3"=0.00010067317190733693, "N4"=-1.0308515848458662e-05}, {"N1"=196.972, "N2"=139.497, "N3"=0.00010057618112399889, "N4"=-1.0321839416161683e-05}, {"N1"=199.497, "N2"=139.497, "N3"=0.00010057970726160341, "N4"=-1.0276047033908628e-05}, {"N1"=199.497, "N2"=137.222, "N3"=0.00010052114538489574, "N4"=-1.0074293156140917e-05}, {"N1"=199.497, "N2"=134.505, "N3"=0.00010056195180444358, "N4"=-1.0203826844149927e-05}, {"N1"=199.497, "N2"=131.995, "N3"=0.0001004698654033356, "N4"=-1.0460938590601448e-05}, {"N1"=199.497, "N2"=129.504, "N3"=0.00010068153412573708, "N4"=-1.0386375922436362e-05}, {"N1"=199.497, "N2"=127.001, "N3"=0.000100638010359207, "N4"=-1.0149357679075847e-05}, {"N1"=199.497, "N2"=124.525, "N3"=0.00010048296688320728, "N4"=-1.0485141286157863e-05}, {"N1"=199.497, "N2"=122.009, "N3"=0.00010061013700768544, "N4"=-1.034047782158585e-05}, {"N1"=199.497, "N2"=119.537, "N3"=0.00010062095956746089, "N4"=-1.0325512630045374e-05}, {"N1"=199.497, "N2"=117.278, "N3"=0.00010055229223195379, "N4"=-1.0548318170120856e-05}, {"N1"=199.497, "N2"=114.92, "N3"=0.00010064119661885946, "N4"=-1.0263359827917113e-05}, {"N1"=201.998, "N2"=114.462, "N3"=0.00010058947269887276, "N4"=-1.0470855048853185e-05}, {"N1"=201.998, "N2"=117.003, "N3"=0.00010053842263906008, "N4"=-1.0236722353628386e-05}, {"N1"=201.998, "N2"=119.484, "N3"=0.0001004786998986167, "N4"=-1.0329111902704082e-05}, {"N1"=201.998, "N2"=122.007, "N3"=0.00010059294967026013, "N4"=-1.02258355878065e-05}, {"N1"=201.998, "N2"=124.341, "N3"=0.00010061442402067531, "N4"=-1.0561438191604866e-05}, {"N1"=201.998, "N2"=126.988, "N3"=0.00010050513672655457, "N4"=-1.0114485220686001e-05}, {"N1"=201.998, "N2"=129.507, "N3"=0.00010055592705312273, "N4"=-1.0277288944171451e-05}, {"N1"=201.998, "N2"=131.991, "N3"=0.00010056857022127168, "N4"=-1.0202969391123564e-05}, {"N1"=201.998, "N2"=134.312, "N3"=0.00010053872113150245, "N4"=-1.034326513817242e-05}, {"N1"=201.998, "N2"=136.88, "N3"=0.00010062408148693691, "N4"=-1.0371370902083716e-05}, {"N1"=201.998, "N2"=139.523, "N3"=0.00010044237347185545, "N4"=-1.0382451453732467e-05}, {"N1"=204.491, "N2"=139.485, "N3"=0.00010064217847606471, "N4"=-1.0317244840799119e-05}, {"N1"=204.491, "N2"=137.326, "N3"=0.00010059083950815067, "N4"=-1.0538437754500795e-05}, {"N1"=204.491, "N2"=134.802, "N3"=0.00010077099122968396, "N4"=-1.039643515868239e-05}, {"N1"=204.491, "N2"=131.986, "N3"=0.00010053964731166844, "N4"=-1.0417755879865712e-05}, {"N1"=204.491, "N2"=129.498, "N3"=0.00010064595595277834, "N4"=-1.0059266314419994e-05}, {"N1"=204.491, "N2"=127.246, "N3"=0.0001005963881787339, "N4"=-1.0250428810743107e-05}, {"N1"=204.491, "N2"=124.456, "N3"=0.00010055352125306458, "N4"=-1.0340710812284911e-05}, {"N1"=204.491, "N2"=122.404, "N3"=0.00010060627753549074, "N4"=-1.0201480476549741e-05}, {"N1"=204.491, "N2"=119.502, "N3"=0.00010066574681733725, "N4"=-1.0301008211128834e-05}, {"N1"=204.491, "N2"=117.407, "N3"=0.00010053663381298301, "N4"=-1.0321813295060909e-05}, {"N1"=204.491, "N2"=114.489, "N3"=0.00010064591593863201, "N4"=-1.0272372399629984e-05}, {"N1"=206.86, "N2"=114.496, "N3"=0.00010058435615490992, "N4"=-1.0295169837878176e-05}, {"N1"=206.86, "N2"=116.672, "N3"=0.00010055700024056959, "N4"=-1.0257508350212743e-05}, {"N1"=206.86, "N2"=119.325, "N3"=0.00010053623092425434, "N4"=-1.0535705992731928e-05}, {"N1"=206.86, "N2"=121.643, "N3"=0.00010050002674266096, "N4"=-1.0240308826067224e-05}, {"N1"=206.86, "N2"=124.34, "N3"=0.00010065258252810722, "N4"=-1.0327423105270024e-05}, {"N1"=206.86, "N2"=127.011, "N3"=0.00010064941354573508, "N4"=-1.0396762846880845e-05}, {"N1"=206.86, "N2"=129.275, "N3"=0.0001005796768498394, "N4"=-1.0309694829175047e-05}, {"N1"=206.86, "N2"=131.861, "N3"=0.00010059449510014535, "N4"=-1.0438765224260397e-05}, {"N1"=206.86, "N2"=134.247, "N3"=0.00010059602091789288, "N4"=-1.0359653731078761e-05}, {"N1"=206.86, "N2"=136.823, "N3"=0.0001005199930932152, "N4"=-1.0431533670976243e-05}, {"N1"=206.86, "N2"=139.516, "N3"=0.00010064209274399593, "N4"=-1.052018532491652e-05}, {"N1"=209.497, "N2"=139.473, "N3"=0.0001005538093763474, "N4"=-1.0295763128215634e-05}, {"N1"=209.497, "N2"=137.177, "N3"=0.00010057333324274813, "N4"=-1.0207872963207442e-05}, {"N1"=209.497, "N2"=134.719, "N3"=0.00010066852161287753, "N4"=-1.0274507527038644e-05}, {"N1"=209.497, "N2"=131.993, "N3"=0.00010065610151539386, "N4"=-1.0262678209653979e-05}, {"N1"=209.497, "N2"=129.74, "N3"=0.0001005826845490767, "N4"=-1.0199190442510633e-05}, {"N1"=209.497, "N2"=127.478, "N3"=0.00010054831590596191, "N4"=-1.0283302383927606e-05}, {"N1"=209.497, "N2"=124.548, "N3"=0.00010050160476610038, "N4"=-1.0408404089576085e-05}, {"N1"=209.497, "N2"=122.002, "N3"=0.0001005577994635799, "N4"=-1.0407159510576975e-05}, {"N1"=209.497, "N2"=119.497, "N3"=0.00010049043998568819, "N4"=-1.0311944321728337e-05}, {"N1"=209.497, "N2"=116.996, "N3"=0.0001004551202772475, "N4"=-1.0343993975385424e-05}, {"N1"=209.497, "N2"=114.778, "N3"=0.00010058194584294698, "N4"=-1.053403408371471e-05}, {"N1"=184.553, "N2"=117.007, "N3"=0.00010059146452851106, "N4"=-1.0388544013871929e-05}, {"N1"=184.553, "N2"=119.47, "N3"=0.00010055861458914452, "N4"=-1.029646377974472e-05}, {"N1"=184.553, "N2"=121.688, "N3"=0.00010043189787173947, "N4"=-1.0360464399976454e-05}, {"N1"=184.553, "N2"=124.478, "N3"=0.0001004842791550175, "N4"=-1.0263709190436084e-05}, {"N1"=184.553, "N2"=126.892, "N3"=0.00010053956250465372, "N4"=-1.0370719125443691e-05}, {"N1"=184.553, "N2"=129.337, "N3"=0.00010060897420313449, "N4"=-1.0371594223795042e-05}, {"N1"=184.553, "N2"=131.669, "N3"=0.00010063462681676376, "N4"=-1.0461991302463605e-05}, {"N1"=184.553, "N2"=134.257, "N3"=0.00010048519949538947, "N4"=-1.0342100747403899e-05}, {"N1"=184.553, "N2"=136.878, "N3"=0.0001004410150242101, "N4"=-1.0296165803859934e-05}, {"N1"=184.553, "N2"=139.352, "N3"=0.00010072726757482467, "N4"=-1.0329247248312456e-05}, {"N1"=184.553, "N2"=141.73, "N3"=0.00010044220308956644, "N4"=-1.0490860557901031e-05}, {"N1"=182.005, "N2"=142.009, "N3"=0.00010050500072723025, "N4"=-1.0378923076589328e-05}, {"N1"=182.005, "N2"=139.695, "N3"=0.00010057745486141954, "N4"=-1.0345208963865304e-05}, {"N1"=182.005, "N2"=137.284, "N3"=0.00010063889987340568, "N4"=-1.0452821250099016e-05}, {"N1"=182.005, "N2"=134.521, "N3"=0.00010051918406337945, "N4"=-1.0381885875497187e-05}, {"N1"=182.005, "N2"=132.002, "N3"=0.00010062459358247482, "N4"=-1.0395798732907756e-05}, {"N1"=182.005, "N2"=129.504, "N3"=0.00010066039329513683, "N4"=-1.034003729566559e-05}, {"N1"=182.005, "N2"=127.403, "N3"=0.00010054988421753654, "N4"=-1.0296580649309803e-05}, {"N1"=182.005, "N2"=124.554, "N3"=0.00010056130788994546, "N4"=-1.0479756925140636e-05}, {"N1"=182.005, "N2"=122.333, "N3"=0.00010064438573455727, "N4"=-1.0379667631936802e-05}, {"N1"=182.005, "N2"=119.501, "N3"=0.00010057612504747955, "N4"=-1.0352778076138057e-05}, {"N1"=182.005, "N2"=117.309, "N3"=0.00010061535899683524, "N4"=-1.0487547295164834e-05}, {"N1"=179.507, "N2"=117.309, "N3"=0.0001005761068839688, "N4"=-1.0272221502613761e-05}, {"N1"=179.507, "N2"=119.508, "N3"=0.00010056912493296026, "N4"=-1.042045441849985e-05}, {"N1"=179.507, "N2"=122.003, "N3"=0.00010060642696422925, "N4"=-1.0279204891848489e-05}, {"N1"=179.507, "N2"=124.317, "N3"=0.00010048238786654824, "N4"=-1.0346177423041005e-05}, {"N1"=179.507, "N2"=126.981, "N3"=0.00010054213841186517, "N4"=-1.0389014733202514e-05}, {"N1"=179.507, "N2"=129.298, "N3"=0.00010054557882903328, "N4"=-1.037299416906731e-05}, {"N1"=179.507, "N2"=131.778, "N3"=0.0001006549625792609, "N4"=-1.0435875991270398e-05}, {"N1"=179.507, "N2"=134.504, "N3"=0.00010057585420062247, "N4"=-1.0355421914546735e-05}, {"N1"=179.507, "N2"=136.846, "N3"=0.00010049615915529446, "N4"=-1.0514025118121538e-05}, {"N1"=179.507, "N2"=139.398, "N3"=0.00010056063905756571, "N4"=-1.0319168874166382e-05}, {"N1"=179.507, "N2"=141.755, "N3"=0.00010039573925551357, "N4"=-1.0524674139036438e-05}, {"N1"=177.003, "N2"=142.038, "N3"=0.00010054669038812751, "N4"=-1.0297527520687461e-05}, {"N1"=177.003, "N2"=139.87, "N3"=0.00010056811682685965, "N4"=-1.0295586509111913e-05}, {"N1"=177.003, "N2"=136.998, "N3"=0.00010057392273408035, "N4"=-1.0423048935353686e-05}, {"N1"=177.003, "N2"=134.817, "N3"=0.00010062002221420951, "N4"=-1.0320428410655464e-05}, {"N1"=177.003, "N2"=132.058, "N3"=0.00010059690147045393, "N4"=-1.0462448490692068e-05}, {"N1"=177.003, "N2"=129.5, "N3"=0.00010054937145393229, "N4"=-1.0477489139447477e-05}, {"N1"=177.003, "N2"=127.394, "N3"=0.00010062797985192404, "N4"=-1.0226482257500002e-05}, {"N1"=177.003, "N2"=124.471, "N3"=0.00010055012646937922, "N4"=-1.0274417456608019e-05}, {"N1"=177.003, "N2"=121.948, "N3"=0.00010065343711328856, "N4"=-1.0393282014272288e-05}, {"N1"=177.003, "N2"=119.501, "N3"=0.00010061922156220026, "N4"=-1.0433497176401722e-05}, {"N1"=177.003, "N2"=117.001, "N3"=0.00010059092541057091, "N4"=-1.0341842791110043e-05}, {"N1"=174.504, "N2"=117.036, "N3"=0.00010052648773553534, "N4"=-1.0274308803411861e-05}, {"N1"=174.504, "N2"=119.495, "N3"=0.00010060080739597907, "N4"=-1.004476358369826e-05}, {"N1"=174.504, "N2"=122.003, "N3"=0.00010053621340103111, "N4"=-1.0288554566044123e-05}, {"N1"=174.504, "N2"=124.273, "N3"=0.00010050928980549325, "N4"=-1.042302041259302e-05}, {"N1"=174.504, "N2"=127.001, "N3"=0.00010057425999680214, "N4"=-9.974371701551962e-06}, {"N1"=174.504, "N2"=129.501, "N3"=0.00010061672470143939, "N4"=-1.0328659908826785e-05}, {"N1"=174.504, "N2"=132.001, "N3"=0.00010054119176128216, "N4"=-1.0359274896880002e-05}, {"N1"=174.504, "N2"=134.232, "N3"=0.00010057445359787256, "N4"=-1.0104543978999419e-05}, {"N1"=174.504, "N2"=136.748, "N3"=0.00010059589049026271, "N4"=-1.0251558252398136e-05}, {"N1"=174.504, "N2"=139.528, "N3"=0.00010052773895841159, "N4"=-1.0541482878885507e-05}, {"N1"=174.504, "N2"=141.812, "N3"=0.00010061440418712718, "N4"=-1.0336290301436648e-05}, {"N1"=172.009, "N2"=141.984, "N3"=0.00010065201552302352, "N4"=-1.0558237704119496e-05}, {"N1"=172.009, "N2"=139.493, "N3"=0.00010056159099212083, "N4"=-1.0342304145441498e-05}, {"N1"=172.009, "N2"=137.23, "N3"=0.00010056426046591867, "N4"=-1.036678018499724e-05}, {"N1"=172.009, "N2"=134.498, "N3"=0.00010054660093263579, "N4"=-1.0298519284589796e-05}, {"N1"=172.009, "N2"=132.35, "N3"=0.00010055376462966115, "N4"=-1.0324016195050238e-05}, {"N1"=172.009, "N2"=129.501, "N3"=0.00010052148919223511, "N4"=-1.0367851727278967e-05}, {"N1"=172.009, "N2"=127.304, "N3"=0.00010058874875637376, "N4"=-1.050973793832626e-05}, {"N1"=172.009, "N2"=124.471, "N3"=0.00010062062036049002, "N4"=-1.0457672994235088e-05}, {"N1"=172.009, "N2"=122.002, "N3"=0.00010060071027730201, "N4"=-1.0312777300722334e-05}, {"N1"=172.009, "N2"=119.495, "N3"=0.00010054298827558248, "N4"=-1.035459533675667e-05}, {"N1"=172.009, "N2"=116.97, "N3"=0.00010065863829078428, "N4"=-1.0309129248540426e-05}, {"N1"=169.505, "N2"=117.016, "N3"=0.00010046786274321069, "N4"=-1.0456601365642704e-05}, {"N1"=169.505, "N2"=119.469, "N3"=0.00010059761364771047, "N4"=-1.0561117146104116e-05}, {"N1"=169.505, "N2"=121.795, "N3"=0.00010049341433007379, "N4"=-1.0413905917185706e-05}, {"N1"=169.505, "N2"=124.517, "N3"=0.00010066636235475952, "N4"=-1.0353637411980454e-05}, {"N1"=169.505, "N2"=126.796, "N3"=0.00010063261802844523, "N4"=-1.0334558463862006e-05}, {"N1"=169.505, "N2"=129.357, "N3"=0.00010065423291790545, "N4"=-1.037834212491725e-05}, {"N1"=169.505, "N2"=132.029, "N3"=0.00010067855270641082, "N4"=-1.0426042694351648e-05}, {"N1"=169.505, "N2"=134.331, "N3"=0.00010065724773310943, "N4"=-1.038623372708994e-05}, {"N1"=169.505, "N2"=136.739, "N3"=0.00010051110533248984, "N4"=-1.0284339923302253e-05}, {"N1"=169.505, "N2"=139.397, "N3"=0.00010047939506040595, "N4"=-1.0414307248424401e-05}, {"N1"=169.505, "N2"=141.802, "N3"=0.00010065899947397095, "N4"=-1.0393187540705996e-05}, {"N1"=167.007, "N2"=141.99, "N3"=0.0001005695242329897, "N4"=-1.0177853494214666e-05}, {"N1"=167.007, "N2"=139.501, "N3"=0.00010057099206360553, "N4"=-1.0436733617320278e-05}, {"N1"=167.007, "N2"=137.004, "N3"=0.00010055185673082942, "N4"=-1.0291492047554177e-05}, {"N1"=167.007, "N2"=134.499, "N3"=0.00010058146722498193, "N4"=-1.0378272869030202e-05}, {"N1"=167.007, "N2"=132.364, "N3"=0.00010064054212182182, "N4"=-1.0403412975477178e-05}, {"N1"=167.007, "N2"=129.507, "N3"=0.00010055472748843877, "N4"=-1.0385498149809915e-05}, {"N1"=167.007, "N2"=127.495, "N3"=0.00010062915483101089, "N4"=-1.042384852936843e-05}, {"N1"=167.007, "N2"=124.543, "N3"=0.00010046154332406246, "N4"=-1.0301958710256067e-05}, {"N1"=167.007, "N2"=121.992, "N3"=0.00010056415387770768, "N4"=-1.0261909708538007e-05}, {"N1"=167.007, "N2"=119.805, "N3"=0.00010073189424383664, "N4"=-1.0527798543412124e-05}, {"N1"=167.007, "N2"=117.251, "N3"=0.00010044392362746821, "N4"=-1.0199591460805141e-05}, {"N1"=164.503, "N2"=116.969, "N3"=0.0001005662404775267, "N4"=-1.0522124124447618e-05}, {"N1"=164.503, "N2"=119.497, "N3"=0.00010055112325902262, "N4"=-1.0073237802308957e-05}, {"N1"=164.503, "N2"=121.766, "N3"=0.00010050117544255604, "N4"=-1.0497485658056827e-05}, {"N1"=164.504, "N2"=117.016, "N3"=0.00010049269743051667, "N4"=-1.027483733153481e-05}, {"N1"=164.504, "N2"=119.367, "N3"=0.0001005494031865731, "N4"=-1.0447866343600998e-05}, {"N1"=164.504, "N2"=121.889, "N3"=0.00010064802033732407, "N4"=-1.0308063755329468e-05}, {"N1"=164.504, "N2"=124.267, "N3"=0.00010046883424490334, "N4"=-1.0350521661484808e-05}, {"N1"=164.504, "N2"=126.886, "N3"=0.00010046276650051809, "N4"=-1.0481892568155837e-05}, {"N1"=164.504, "N2"=129.289, "N3"=0.00010055448424209784, "N4"=-1.0442580692069773e-05}, {"N1"=164.504, "N2"=131.731, "N3"=0.0001006115049858572, "N4"=-1.0392922399654882e-05}, {"N1"=164.504, "N2"=134.366, "N3"=0.0001006793384461246, "N4"=-1.033310104194545e-05}, {"N1"=164.504, "N2"=136.998, "N3"=0.00010052813978749797, "N4"=-1.0430491024404317e-05}, {"N1"=164.504, "N2"=139.246, "N3"=0.00010056181587766742, "N4"=-1.0534594612818997e-05}, {"N1"=164.504, "N2"=141.982, "N3"=0.0001006401968849996, "N4"=-1.0373517835298896e-05}, {"N1"=164.504, "N2"=144.215, "N3"=0.00010057635521052555, "N4"=-1.0292313151340409e-05}, {"N1"=164.504, "N2"=146.977, "N3"=0.00010056580743087376, "N4"=-1.04566991718854e-05}, {"N1"=164.504, "N2"=149.356, "N3"=0.00010053373307857589, "N4"=-1.0473120979234718e-05}, {"N1"=162.003, "N2"=149.502, "N3"=0.00010062833487448124, "N4"=-1.0508614851963253e-05}, {"N1"=162.003, "N2"=147.042, "N3"=0.00010058351795946075, "N4"=-1.0348234094961914e-05}, {"N1"=162.003, "N2"=144.709, "N3"=0.00010056895190275648, "N4"=-1.0035774931746906e-05}, {"N1"=162.003, "N2"=142.296, "N3"=0.00010051733628145831, "N4"=-1.0388688555696195e-05}, {"N1"=162.003, "N2"=139.835, "N3"=0.00010056969524132631, "N4"=-1.0370244545291619e-05}, {"N1"=162.003, "N2"=137.008, "N3"=0.00010063945488903496, "N4"=-1.0486306542250182e-05}, {"N1"=162.003, "N2"=134.498, "N3"=0.00010064349784457727, "N4"=-1.037733840445335e-05}, {"N1"=162.003, "N2"=132.004, "N3"=0.00010055458506125796, "N4"=-1.0284724588700372e-05}, {"N1"=162.003, "N2"=129.477, "N3"=0.00010054150805728426, "N4"=-1.017120948535454e-05}, {"N1"=162.003, "N2"=126.995, "N3"=0.00010047982834951657, "N4"=-1.0333472742136943e-05}, {"N1"=162.003, "N2"=124.495, "N3"=0.0001005415230748842, "N4"=-1.0124737897377322e-05}, {"N1"=162.003, "N2"=122.384, "N3"=0.00010054688084870989, "N4"=-1.0322868076468943e-05}, {"N1"=162.003, "N2"=119.935, "N3"=0.00010057868733831236, "N4"=-1.047529098877101e-05}, {"N1"=162.003, "N2"=116.998, "N3"=0.00010065071902185159, "N4"=-1.0441210210756248e-05}, {"N1"=159.505, "N2"=117.023, "N3"=0.00010062140426381693, "N4"=-1.034592009907794e-05}, {"N1"=159.505, "N2"=119.55, "N3"=0.00010060155731901412, "N4"=-1.0267163950348662e-05}, {"N1"=159.505, "N2"=121.786, "N3"=0.00010053619129403293, "N4"=-1.02912944372415e-05}, {"N1"=159.505, "N2"=124.336, "N3"=0.00010059512806725215, "N4"=-1.0325923429429126e-05}, {"N1"=159.505, "N2"=127.001, "N3"=0.00010059490134238402, "N4"=-1.0234806928315857e-05}, {"N1"=159.505, "N2"=129.508, "N3"=0.0001005043131485438, "N4"=-1.0399015546300578e-05}, {"N1"=159.505, "N2"=131.903, "N3"=0.0001005843560390402, "N4"=-1.0272099266852468e-05}, {"N1"=159.505, "N2"=134.24, "N3"=0.00010052350589281774, "N4"=-1.0457459019346997e-05}, {"N1"=159.505, "N2"=137.018, "N3"=0.00010065178511222863, "N4"=-1.0395917854740611e-05}, {"N1"=159.505, "N2"=139.138, "N3"=0.00010049346146368262, "N4"=-1.0388102971892434e-05}, {"N1"=159.505, "N2"=141.995, "N3"=0.00010056839258668768, "N4"=-1.0468358529202424e-05}, {"N1"=159.505, "N2"=144.496, "N3"=0.00010057206895810795, "N4"=-1.0297865401393399e-05}, {"N1"=159.505, "N2"=147.0, "N3"=0.00010059814995048672, "N4"=-1.0449303729327082e-05}, {"N1"=159.505, "N2"=149.477, "N3"=0.00010057296034411018, "N4"=-1.0169088841860752e-05}, {"N1"=157.002, "N2"=149.507, "N3"=0.00010055599748203207, "N4"=-1.0293578939030758e-05}, {"N1"=157.002, "N2"=147.277, "N3"=0.00010061897360933323, "N4"=-1.00413229943577e-05}, {"N1"=157.002, "N2"=144.921, "N3"=0.00010057222441126179, "N4"=-1.045298666327595e-05}, {"N1"=157.002, "N2"=142.012, "N3"=0.00010046539741328427, "N4"=-1.027049515612258e-05}, {"N1"=157.002, "N2"=139.751, "N3"=0.00010050684974882449, "N4"=-1.0192608431104588e-05}, {"N1"=157.002, "N2"=137.33, "N3"=0.00010060248451382324, "N4"=-1.0523615020027692e-05}, {"N1"=157.002, "N2"=134.742, "N3"=0.00010057979882366348, "N4"=-1.0276825120798206e-05}, {"N1"=157.002, "N2"=132.036, "N3"=0.00010055957486331446, "N4"=-1.034696883419761e-05}, {"N1"=157.002, "N2"=129.848, "N3"=0.00010058843258311114, "N4"=-1.0449932810669681e-05}, {"N1"=157.002, "N2"=127.01, "N3"=0.00010072069934267054, "N4"=-1.0283362453969017e-05}, {"N1"=157.002, "N2"=124.485, "N3"=0.00010068285389602451, "N4"=-1.057751169934909e-05}, {"N1"=157.002, "N2"=122.267, "N3"=0.00010055765650813793, "N4"=-1.0330501604414478e-05}, {"N1"=157.002, "N2"=119.559, "N3"=0.00010053075352598335, "N4"=-1.0446149515084873e-05}, {"N1"=157.002, "N2"=117.343, "N3"=0.0001007009117533854, "N4"=-1.0355529489366831e-05}, {"N1"=154.503, "N2"=116.955, "N3"=0.00010062063347388942, "N4"=-1.0230402572366444e-05}, {"N1"=154.503, "N2"=119.496, "N3"=0.00010055701816655911, "N4"=-1.0243881079226215e-05}, {"N1"=154.503, "N2"=121.985, "N3"=0.00010051149630278998, "N4"=-1.0342396714054824e-05}, {"N1"=154.503, "N2"=124.278, "N3"=0.00010059523927698657, "N4"=-1.0230929167116033e-05}, {"N1"=154.503, "N2"=126.827, "N3"=0.0001005979251339054, "N4"=-1.0482774858090947e-05}, {"N1"=154.503, "N2"=129.277, "N3"=0.0001005841640628933, "N4"=-1.042178730802122e-05}, {"N1"=154.503, "N2"=131.988, "N3"=0.00010066558399537575, "N4"=-1.040799094449207e-05}, {"N1"=154.503, "N2"=134.333, "N3"=0.0001006598578427202, "N4"=-1.0277371831773167e-05}, {"N1"=154.503, "N2"=136.791, "N3"=0.00010058251372801229, "N4"=-1.0247128664653888e-05}, {"N1"=154.503, "N2"=139.418, "N3"=0.00010041102609172348, "N4"=-1.0322094232625279e-05}, {"N1"=154.503, "N2"=141.779, "N3"=0.00010049850085466028, "N4"=-1.0336339792011367e-05}, {"N1"=154.503, "N2"=144.193, "N3"=0.00010055072828574676, "N4"=-1.0325562302236852e-05}, {"N1"=154.503, "N2"=146.675, "N3"=0.00010058312031848977, "N4"=-1.0349921683832133e-05}, {"N1"=154.503, "N2"=149.496, "N3"=0.00010051919914208212, "N4"=-1.0377976511425714e-05}, {"N1"=152.004, "N2"=149.504, "N3"=0.00010053872617908566, "N4"=-1.037244996437282e-05}, {"N1"=152.004, "N2"=146.998, "N3"=0.00010069476305827682, "N4"=-1.0348155211665467e-05}, {"N1"=152.004, "N2"=144.502, "N3"=0.00010054030045809894, "N4"=-1.0228116513984353e-05}, {"N1"=152.004, "N2"=141.994, "N3"=0.00010043087783237099, "N4"=-1.0304580722653196e-05}, {"N1"=152.004, "N2"=139.505, "N3"=0.00010062939891080778, "N4"=-1.0297233834860054e-05}, {"N1"=152.004, "N2"=136.993, "N3"=0.00010056510264300851, "N4"=-1.0492336501999903e-05}, {"N1"=152.004, "N2"=134.86, "N3"=0.00010059083649006086, "N4"=-1.0390959996788271e-05}, {"N1"=152.004, "N2"=132.032, "N3"=0.00010060163235038002, "N4"=-1.0313066217501323e-05}, {"N1"=152.004, "N2"=129.917, "N3"=0.00010062365410820106, "N4"=-1.0301136021552274e-05}, {"N1"=152.004, "N2"=126.987, "N3"=0.00010046923588716854, "N4"=-1.0430627670585603e-05}, {"N1"=152.004, "N2"=124.507, "N3"=0.00010061948940027883, "N4"=-1.0443531328239596e-05}, {"N1"=152.004, "N2"=122.0, "N3"=0.0001006315748242027, "N4"=-1.0216262680802176e-05}, {"N1"=152.004, "N2"=119.723, "N3"=0.00010057047397371159, "N4"=-1.030836636326719e-05}, {"N1"=152.004, "N2"=117.269, "N3"=0.0001006412606619715, "N4"=-1.0402070343421836e-05}, {"N1"=149.504, "N2"=117.269, "N3"=0.00010071971682391206, "N4"=-1.032964995042858e-05}, {"N1"=149.504, "N2"=119.5, "N3"=0.00010060647358717563, "N4"=-1.0363472297927608e-05}, {"N1"=149.504, "N2"=122.022, "N3"=0.00010065573416933438, "N4"=-1.0378418406286614e-05}, {"N1"=149.504, "N2"=124.324, "N3"=0.00010050845863892421, "N4"=-1.0239097726091218e-05}, {"N1"=149.504, "N2"=126.829, "N3"=0.000100666022023567, "N4"=-1.0278249193180104e-05}, {"N1"=149.504, "N2"=129.512, "N3"=0.00010057161008923896, "N4"=-1.0195806740961933e-05}, {"N1"=149.504, "N2"=131.713, "N3"=0.00010059135508919501, "N4"=-1.0415387066107528e-05}, {"N1"=149.504, "N2"=134.376, "N3"=0.00010052759374161593, "N4"=-1.0593649276601493e-05}, {"N1"=149.504, "N2"=136.866, "N3"=0.00010068945385428807, "N4"=-1.031282962259783e-05}, {"N1"=149.504, "N2"=139.382, "N3"=0.00010065552702871607, "N4"=-1.0404840070232321e-05}, {"N1"=149.504, "N2"=141.991, "N3"=0.00010052397105623015, "N4"=-1.0348581102478636e-05}, {"N1"=149.504, "N2"=144.488, "N3"=0.00010063895072433827, "N4"=-1.0303289972633314e-05}, {"N1"=149.504, "N2"=147.016, "N3"=0.00010049471126759772, "N4"=-1.0294953776593344e-05}, {"N1"=149.504, "N2"=149.345, "N3"=0.00010056050725249474, "N4"=-1.0292767409900594e-05}, {"N1"=147.008, "N2"=149.495, "N3"=0.00010060819213176628, "N4"=-1.0301275023816109e-05}, {"N1"=147.008, "N2"=147.263, "N3"=0.00010061750449992732, "N4"=-1.0224208561623774e-05}, {"N1"=147.008, "N2"=144.754, "N3"=0.00010059529064690775, "N4"=-1.0423492606312144e-05}, {"N1"=147.008, "N2"=141.979, "N3"=0.00010053056929662445, "N4"=-1.0332587928845142e-05}, {"N1"=147.008, "N2"=139.558, "N3"=0.00010070357522428476, "N4"=-1.0228629523470624e-05}, {"N1"=147.008, "N2"=137.4, "N3"=0.00010045900680224087, "N4"=-1.0232107246527014e-05}, {"N1"=147.008, "N2"=134.508, "N3"=0.00010061414760207699, "N4"=-1.0068050881017596e-05}, {"N1"=147.008, "N2"=132.006, "N3"=0.00010059335460784064, "N4"=-1.026844486475866e-05}, {"N1"=147.008, "N2"=129.802, "N3"=0.00010050994037513152, "N4"=-1.0260426956511741e-05}, {"N1"=147.008, "N2"=126.998, "N3"=0.00010050072050497287, "N4"=-1.0403086083888002e-05}, {"N1"=147.008, "N2"=124.522, "N3"=0.00010059993307454964, "N4"=-1.0232223757630371e-05}, {"N1"=147.008, "N2"=121.93, "N3"=0.00010068030603337025, "N4"=-1.0307410632941375e-05}, {"N1"=147.008, "N2"=119.471, "N3"=0.00010061625922177942, "N4"=-1.0293525457093817e-05}, {"N1"=147.008, "N2"=117.016, "N3"=0.0001005019227000808, "N4"=-1.0401879402249025e-05}, {"N1"=144.504, "N2"=117.003, "N3"=0.00010049787147710703, "N4"=-1.0425079943250253e-05}, {"N1"=144.504, "N2"=119.501, "N3"=0.00010054804787299352, "N4"=-1.0252634002677028e-05}, {"N1"=144.504, "N2"=122.011, "N3"=0.00010053416621200439, "N4"=-1.0322782559442437e-05}, {"N1"=144.504, "N2"=124.118, "N3"=0.00010058345125384192, "N4"=-1.0321329000219688e-05}, {"N1"=144.504, "N2"=126.616, "N3"=0.00010039034644257998, "N4"=-1.0284757628914072e-05}, {"N1"=144.504, "N2"=129.507, "N3"=0.00010058733940772762, "N4"=-1.0420289465942938e-05}, {"N1"=144.504, "N2"=132.003, "N3"=0.00010050170010654708, "N4"=-1.0390696761684604e-05}, {"N1"=144.504, "N2"=134.358, "N3"=0.00010066427544073963, "N4"=-1.0108124806403855e-05}, {"N1"=144.504, "N2"=137.006, "N3"=0.00010053446248024114, "N4"=-1.0266222017370464e-05}, {"N1"=144.504, "N2"=139.39, "N3"=0.00010057716453669314, "N4"=-1.0279331405274479e-05}, {"N1"=144.504, "N2"=141.993, "N3"=0.0001005184963360002, "N4"=-1.0267612729027159e-05}, {"N1"=144.504, "N2"=144.35, "N3"=0.00010056769340112286, "N4"=-1.0322318585012174e-05}, {"N1"=144.504, "N2"=146.899, "N3"=0.0001005777386354461, "N4"=-1.0289315989756152e-05}, {"N1"=144.504, "N2"=149.495, "N3"=0.00010058602866922187, "N4"=-1.0356066131030543e-05}, {"N1"=166.994, "N2"=144.92, "N3"=0.00010063132489488085, "N4"=-1.0393145199522023e-05}, {"N1"=166.994, "N2"=147.006, "N3"=0.00010051194333166727, "N4"=-1.0250463266315734e-05}, {"N1"=166.994, "N2"=149.514, "N3"=0.0001005771438343386, "N4"=-1.0362734110826016e-05}, {"N1"=169.497, "N2"=149.5, "N3"=0.00010049483742907352, "N4"=-1.0311511979643547e-05}, {"N1"=169.497, "N2"=147.434, "N3"=0.00010047759243822706, "N4"=-1.0315267637816948e-05}, {"N1"=169.497, "N2"=144.724, "N3"=0.0001004964544789488, "N4"=-1.028986751682054e-05}, {"N1"=172.011, "N2"=144.489, "N3"=0.00010049460915218653, "N4"=-1.0231060331594025e-05}, {"N1"=172.011, "N2"=146.993, "N3"=0.0001005835280386187, "N4"=-1.044002113577621e-05}, {"N1"=172.011, "N2"=149.482, "N3"=0.00010065528758565956, "N4"=-1.045002103134663e-05}, {"N1"=174.496, "N2"=149.539, "N3"=0.0001004252902922398, "N4"=-1.020324583339702e-05}, {"N1"=174.496, "N2"=147.244, "N3"=0.00010053865660222454, "N4"=-1.0650778643545045e-05}, {"N1"=174.496, "N2"=144.824, "N3"=0.00010070969444101262, "N4"=-1.024451573464899e-05}, {"N1"=176.995, "N2"=144.504, "N3"=0.00010049948356024197, "N4"=-1.034940024297289e-05}, {"N1"=176.995, "N2"=146.978, "N3"=0.00010055264892997143, "N4"=-1.0356491313978087e-05}, {"N1"=176.995, "N2"=149.5, "N3"=0.00010057760683022456, "N4"=-1.0343439488403287e-05}, {"N1"=179.484, "N2"=149.499, "N3"=0.00010053634824722144, "N4"=-1.0272097288995867e-05}, {"N1"=179.484, "N2"=147.222, "N3"=0.00010050028712718304, "N4"=-1.0490296942003244e-05}, {"N1"=179.484, "N2"=144.895, "N3"=0.00010048059150285485, "N4"=-1.047428348899092e-05}, {"N1"=181.998, "N2"=144.49, "N3"=0.00010051575158333539, "N4"=-1.0504628107330734e-05}, {"N1"=181.998, "N2"=147.011, "N3"=0.00010052303872423142, "N4"=-1.011001761152717e-05}, {"N1"=181.998, "N2"=149.479, "N3"=0.00010055176613925775, "N4"=-1.031223064909187e-05}, {"N1"=184.49, "N2"=149.492, "N3"=0.00010051176723114332, "N4"=-1.0350523756774964e-05}, {"N1"=184.49, "N2"=147.234, "N3"=0.0001004816200286196, "N4"=-1.0280022324874274e-05}, {"N1"=184.49, "N2"=144.852, "N3"=0.00010054409790484611, "N4"=-1.0289696224564238e-05}, {"N1"=186.998, "N2"=144.499, "N3"=0.00010053397621725331, "N4"=-1.0262259270116831e-05}, {"N1"=186.998, "N2"=147.012, "N3"=0.00010046894356162366, "N4"=-1.0428316306154973e-05}, {"N1"=186.998, "N2"=149.48, "N3"=0.0001005994588730581, "N4"=-1.033140550864559e-05}, {"N1"=191.996, "N2"=144.795, "N3"=0.00010057503022848991, "N4"=-1.0338940453395174e-05}, {"N1"=191.996, "N2"=147.003, "N3"=0.00010066534958225373, "N4"=-1.0380780420219314e-05}, {"N1"=191.996, "N2"=149.362, "N3"=0.00010045742974572892, "N4"=-1.0407899416737152e-05}, {"N1"=191.996, "N2"=151.724, "N3"=0.0001005426468584359, "N4"=-1.041982763249689e-05}, {"N1"=191.996, "N2"=154.337, "N3"=0.00010054163078601866, "N4"=-1.0324258520933678e-05}, {"N1"=191.996, "N2"=156.886, "N3"=0.00010056662242594223, "N4"=-1.038386753752895e-05}, {"N1"=191.996, "N2"=159.496, "N3"=0.0001006132221954114, "N4"=-1.0237620457409125e-05}, {"N1"=191.996, "N2"=161.991, "N3"=0.00010051966642671815, "N4"=-1.0219524315805733e-05}, {"N1"=191.996, "N2"=164.35, "N3"=0.00010054011068586918, "N4"=-1.0306705331260904e-05}, {"N1"=191.996, "N2"=166.841, "N3"=0.00010064457917184225, "N4"=-1.0165964089479782e-05}, {"N1"=191.996, "N2"=169.349, "N3"=0.00010053072958605225, "N4"=-1.0410678322353806e-05}, {"N1"=191.996, "N2"=172.005, "N3"=0.0001004938480593684, "N4"=-1.0388414744068434e-05}, {"N1"=191.996, "N2"=174.505, "N3"=0.00010066827534930882, "N4"=-1.0395636867591871e-05}, {"N1"=191.996, "N2"=177.006, "N3"=0.0001005048646735938, "N4"=-1.0223947706368497e-05}, {"N1"=191.996, "N2"=179.504, "N3"=0.00010058085140214634, "N4"=-1.0431970547534671e-05}, {"N1"=191.996, "N2"=181.84, "N3"=0.00010052922489490765, "N4"=-1.0355084186355676e-05}, {"N1"=191.996, "N2"=184.374, "N3"=0.00010058119857393249, "N4"=-1.0414147914325042e-05}, {"N1"=191.996, "N2"=187.017, "N3"=0.00010055623762781604, "N4"=-1.0471997511387608e-05}, {"N1"=191.996, "N2"=189.493, "N3"=0.00010061746471290358, "N4"=-1.0469366265831165e-05}, {"N1"=191.996, "N2"=192.044, "N3"=0.00010054215797227613, "N4"=-1.035195576109068e-05}, {"N1"=191.996, "N2"=194.506, "N3"=0.00010070522372706563, "N4"=-1.0337727806851342e-05}, {"N1"=191.996, "N2"=196.968, "N3"=0.00010065305882857154, "N4"=-1.0272321635940252e-05}, {"N1"=191.996, "N2"=199.515, "N3"=0.00010065777271444059, "N4"=-1.0350588285323707e-05}, {"N1"=191.996, "N2"=201.997, "N3"=0.00010058385854993672, "N4"=-1.0306678170450834e-05}, {"N1"=191.996, "N2"=204.265, "N3"=0.00010061221693842934, "N4"=-1.0065603355709244e-05}, {"N1"=191.996, "N2"=206.999, "N3"=0.0001005875811108127, "N4"=-1.0206305681344109e-05}, {"N1"=191.996, "N2"=209.539, "N3"=0.00010058820923197684, "N4"=-1.0493263333126373e-05}, {"N1"=191.996, "N2"=212.028, "N3"=0.00010061805295099033, "N4"=-1.0298862286088797e-05}, {"N1"=191.996, "N2"=214.443, "N3"=0.00010055810354804531, "N4"=-1.0563400445389847e-05}, {"N1"=191.996, "N2"=216.725, "N3"=0.00010053926676591393, "N4"=-1.038753898763444e-05}, {"N1"=191.996, "N2"=219.47, "N3"=0.00010058066546024038, "N4"=-1.03096656971029e-05}, {"N1"=191.996, "N2"=221.797, "N3"=0.000100521698263223, "N4"=-1.033180469731966e-05}, {"N1"=191.996, "N2"=224.497, "N3"=0.0001004795934350268, "N4"=-1.0405173181004657e-05}, {"N1"=191.996, "N2"=226.998, "N3"=0.00010059015791575789, "N4"=-1.033766826105032e-05}, {"N1"=191.996, "N2"=229.436, "N3"=0.00010060923714347418, "N4"=-1.0267885998498252e-05}, {"N1"=191.996, "N2"=231.634, "N3"=0.00010049651116289272, "N4"=-1.0430449385843277e-05}, {"N1"=191.996, "N2"=234.5, "N3"=0.00010055712089386373, "N4"=-1.0358131509413556e-05}, {"N1"=191.996, "N2"=236.999, "N3"=0.00010068379827598355, "N4"=-1.0302561579314388e-05}, {"N1"=191.996, "N2"=239.477, "N3"=0.00010047866336560874, "N4"=-1.0411909259862328e-05}, {"N1"=191.996, "N2"=241.853, "N3"=0.00010055343454259429, "N4"=-1.0243657310468301e-05}, {"N1"=191.996, "N2"=244.405, "N3"=0.00010058417717772568, "N4"=-1.0269493681777803e-05}, {"N1"=191.996, "N2"=246.91, "N3"=0.00010062819456533582, "N4"=-1.0272141148598907e-05}, {"N1"=191.996, "N2"=249.488, "N3"=0.00010056821029236928, "N4"=-1.0340020021854818e-05}, {"N1"=191.996, "N2"=251.704, "N3"=0.00010065759557074449, "N4"=-1.0329641383071122e-05}, {"N1"=191.996, "N2"=254.492, "N3"=0.00010057796952190451, "N4"=-1.0284612827778078e-05}, {"N1"=191.996, "N2"=256.799, "N3"=0.00010063577042569525, "N4"=-1.0329227866710886e-05}, {"N1"=189.506, "N2"=256.99, "N3"=0.00010053195853199196, "N4"=-1.0445442874501309e-05}, {"N1"=189.506, "N2"=254.642, "N3"=0.00010062373739047002, "N4"=-1.038267676413735e-05}, {"N1"=189.506, "N2"=252.252, "N3"=0.00010060901043629462, "N4"=-1.0423317753346132e-05}, {"N1"=189.506, "N2"=249.855, "N3"=0.00010050094587740504, "N4"=-1.0431223967160507e-05}, {"N1"=189.506, "N2"=246.999, "N3"=0.00010058974428219982, "N4"=-1.0340299277280957e-05}, {"N1"=189.506, "N2"=244.524, "N3"=0.00010055656468780623, "N4"=-1.053351676682195e-05}, {"N1"=189.506, "N2"=242.248, "N3"=0.00010055388255591169, "N4"=-1.0216325327280904e-05}, {"N1"=189.506, "N2"=240.113, "N3"=0.00010057451174382039, "N4"=-1.041060384291682e-05}, {"N1"=189.506, "N2"=236.998, "N3"=0.00010054319017101952, "N4"=-1.0348870506195839e-05}, {"N1"=189.506, "N2"=234.866, "N3"=0.00010050860466242158, "N4"=-1.0475965819222953e-05}, {"N1"=189.506, "N2"=231.979, "N3"=0.00010060735713010531, "N4"=-1.0374517256243438e-05}, {"N1"=189.506, "N2"=229.88, "N3"=0.00010049947613491992, "N4"=-1.0491154630192516e-05}, {"N1"=189.506, "N2"=227.267, "N3"=0.00010062560576095063, "N4"=-1.0555557528305423e-05}, {"N1"=189.506, "N2"=224.473, "N3"=0.00010054870210895435, "N4"=-1.0387256544361327e-05}, {"N1"=189.506, "N2"=222.338, "N3"=0.0001005705880949266, "N4"=-1.0359666369953541e-05}, {"N1"=189.506, "N2"=219.943, "N3"=0.00010052399645025834, "N4"=-1.0310144901537403e-05}, {"N1"=189.506, "N2"=217.359, "N3"=0.00010060901318214533, "N4"=-1.0430222257765288e-05}, {"N1"=189.506, "N2"=214.968, "N3"=0.0001005359008706473, "N4"=-1.0310194088582675e-05}, {"N1"=189.506, "N2"=212.385, "N3"=0.00010054874079276358, "N4"=-1.0350840870693861e-05}, {"N1"=189.506, "N2"=209.538, "N3"=0.00010052877064697572, "N4"=-1.0448750460944099e-05}, {"N1"=189.506, "N2"=207.267, "N3"=0.00010053680956204742, "N4"=-1.0355852855433731e-05}, {"N1"=189.506, "N2"=204.668, "N3"=0.00010057308714312922, "N4"=-1.0381850165958104e-05}, {"N1"=189.506, "N2"=201.992, "N3"=0.00010051465119619463, "N4"=-1.0253710037528991e-05}, {"N1"=189.506, "N2"=199.708, "N3"=0.00010054552600488515, "N4"=-1.0111514624342852e-05}, {"N1"=189.506, "N2"=197.028, "N3"=0.00010056463679786198, "N4"=-1.0131100186631911e-05}, {"N1"=189.506, "N2"=194.795, "N3"=0.00010052779216466223, "N4"=-1.0611826314801406e-05}, {"N1"=189.506, "N2"=192.336, "N3"=0.00010061170953168135, "N4"=-1.0313720182691726e-05}, {"N1"=189.506, "N2"=189.856, "N3"=0.00010049183044402859, "N4"=-1.0574827403736794e-05}, {"N1"=189.506, "N2"=187.38, "N3"=0.00010057831497383143, "N4"=-1.0526665896714861e-05}, {"N1"=189.506, "N2"=184.506, "N3"=0.0001005504195817918, "N4"=-1.0419727243247705e-05}, {"N1"=189.506, "N2"=182.041, "N3"=0.00010053309735838938, "N4"=-1.027504174089921e-05}, {"N1"=189.506, "N2"=179.521, "N3"=0.00010063619607854753, "N4"=-1.0259288158518756e-05}, {"N1"=189.506, "N2"=177.348, "N3"=0.00010056552179621183, "N4"=-1.0306944055227605e-05}, {"N1"=189.506, "N2"=174.768, "N3"=0.00010050767014227269, "N4"=-1.0363158516396958e-05}, {"N1"=189.506, "N2"=171.99, "N3"=0.00010049993887402406, "N4"=-1.0288583567424436e-05}, {"N1"=189.506, "N2"=169.508, "N3"=0.00010061187175001803, "N4"=-1.0557478049771404e-05}, {"N1"=189.506, "N2"=167.368, "N3"=0.00010048423542880793, "N4"=-1.0045680054673883e-05}, {"N1"=189.506, "N2"=164.762, "N3"=0.00010065330365149442, "N4"=-1.0141054465717669e-05}, {"N1"=189.506, "N2"=162.018, "N3"=0.00010066083398297246, "N4"=-1.0542179742891947e-05}, {"N1"=189.506, "N2"=159.944, "N3"=0.00010052369352912782, "N4"=-1.032647282448874e-05}, {"N1"=189.506, "N2"=157.276, "N3"=0.00010056916416645032, "N4"=-1.0215027812823863e-05}, {"N1"=189.506, "N2"=154.743, "N3"=0.00010047947141481361, "N4"=-1.0419662663205136e-05}, {"N1"=189.506, "N2"=151.994, "N3"=0.00010057001878316886, "N4"=-9.826004172101797e-06}, {"N1"=189.506, "N2"=149.739, "N3"=0.00010054929559028402, "N4"=-1.0679183701845848e-05}, {"N1"=189.506, "N2"=147.013, "N3"=0.00010075367648667777, "N4"=-1.0348473745328102e-05}, {"N1"=189.506, "N2"=144.553, "N3"=0.00010056636743875816, "N4"=-1.0022593896020288e-05}, {"N1"=187.13, "N2"=144.493, "N3"=0.00010053838933053025, "N4"=-1.06298346600296e-05}, {"N1"=187.13, "N2"=146.75, "N3"=0.0001005970449939864, "N4"=-1.0435689480923566e-05}, {"N1"=187.13, "N2"=149.507, "N3"=0.0001004670463215843, "N4"=-1.0411558691606884e-05}, {"N1"=187.13, "N2"=151.762, "N3"=0.00010049367432338714, "N4"=-1.0307083770674997e-05}, {"N1"=187.13, "N2"=154.498, "N3"=0.00010064459157133176, "N4"=-1.0031696878103363e-05}, {"N1"=187.13, "N2"=156.888, "N3"=0.00010059117290115231, "N4"=-1.0476521312755448e-05}, {"N1"=187.13, "N2"=159.499, "N3"=0.0001005079689039197, "N4"=-1.0521172221912126e-05}, {"N1"=187.13, "N2"=162.01, "N3"=0.00010048336649203051, "N4"=-9.95963564899579e-06}, {"N1"=187.13, "N2"=164.287, "N3"=0.00010058054596888425, "N4"=-1.067950241070496e-05}, {"N1"=187.13, "N2"=166.865, "N3"=0.00010050096505067525, "N4"=-1.045661472837391e-05}, {"N1"=187.13, "N2"=169.51, "N3"=0.00010064722990245543, "N4"=-1.0385550376919822e-05}, {"N1"=187.13, "N2"=171.93, "N3"=0.00010054066693114364, "N4"=-1.0358528804819501e-05}, {"N1"=187.13, "N2"=174.498, "N3"=0.0001006758249585693, "N4"=-1.0626358761555797e-05}, {"N1"=187.13, "N2"=177.007, "N3"=0.00010054981271242698, "N4"=-1.0393582564080786e-05}, {"N1"=187.13, "N2"=179.51, "N3"=0.00010063106678017868, "N4"=-1.0350383828251821e-05}, {"N1"=187.13, "N2"=181.88, "N3"=0.00010052458297340836, "N4"=-1.0536264182501381e-05}, {"N1"=187.13, "N2"=184.399, "N3"=0.00010060053032234755, "N4"=-1.0290728734102487e-05}, {"N1"=187.13, "N2"=187.007, "N3"=0.00010058178533841776, "N4"=-1.053579462825528e-05}, {"N1"=187.13, "N2"=189.503, "N3"=0.00010056000137835346, "N4"=-1.033274667374382e-05}, {"N1"=187.13, "N2"=191.985, "N3"=0.00010053399619088432, "N4"=-1.0663283285985974e-05}, {"N1"=187.13, "N2"=194.498, "N3"=0.00010057416046866958, "N4"=-1.0483080191442944e-05}, {"N1"=187.13, "N2"=196.976, "N3"=0.00010062100307365897, "N4"=-1.0670093567442412e-05}, {"N1"=187.13, "N2"=199.335, "N3"=0.00010063980686717409, "N4"=-1.0280074269162914e-05}, {"N1"=187.13, "N2"=202.036, "N3"=0.00010053629939556323, "N4"=-1.0455161452210727e-05}, {"N1"=187.13, "N2"=204.283, "N3"=0.00010045055700881544, "N4"=-1.0636975882671941e-05}, {"N1"=187.13, "N2"=206.87, "N3"=0.00010055760691081898, "N4"=-1.0567788857664322e-05}, {"N1"=187.13, "N2"=209.492, "N3"=0.00010049319937417005, "N4"=-9.910018236603157e-06}, {"N1"=187.13, "N2"=211.978, "N3"=0.00010053316117246027, "N4"=-1.0556809365678003e-05}, {"N1"=187.13, "N2"=214.492, "N3"=0.00010055957782332536, "N4"=-1.0616242470082422e-05}, {"N1"=187.13, "N2"=216.915, "N3"=0.00010062990865654056, "N4"=-1.0457187594364205e-05}, {"N1"=187.13, "N2"=219.518, "N3"=0.00010066021960718487, "N4"=-1.0272684496675975e-05}, {"N1"=187.13, "N2"=222.0, "N3"=0.00010064441367586943, "N4"=-1.0475701685312074e-05}, {"N1"=187.13, "N2"=224.502, "N3"=0.00010049878162934754, "N4"=-1.0344766905520962e-05}, {"N1"=187.13, "N2"=226.994, "N3"=0.00010051449094228862, "N4"=-1.0401970655682825e-05}, {"N1"=187.13, "N2"=229.413, "N3"=0.00010055933438376278, "N4"=-1.0533913920877074e-05}, {"N1"=187.13, "N2"=231.753, "N3"=0.00010072714981528499, "N4"=-1.0420251189267061e-05}, {"N1"=187.13, "N2"=234.378, "N3"=0.00010053684965334715, "N4"=-1.039539290241415e-05}, {"N1"=187.13, "N2"=237.008, "N3"=0.00010058967589759505, "N4"=-1.0608434997809762e-05}, {"N1"=187.13, "N2"=239.637, "N3"=0.00010048395874628148, "N4"=-1.055213645387239e-05}, {"N1"=187.13, "N2"=241.759, "N3"=0.00010056319796045057, "N4"=-1.0623324474982988e-05}, {"N1"=187.13, "N2"=244.503, "N3"=0.00010061295369376409, "N4"=-1.0529273654315344e-05}, {"N1"=187.13, "N2"=246.729, "N3"=0.00010050408284990959, "N4"=-9.912348997140046e-06}, {"N1"=187.13, "N2"=249.445, "N3"=0.00010049962265092163, "N4"=-1.0437248961338241e-05}, {"N1"=187.13, "N2"=251.744, "N3"=0.00010058042213900567, "N4"=-1.026354125131022e-05}, {"N1"=187.13, "N2"=254.339, "N3"=0.00010055287538140131, "N4"=-1.0345509885470194e-05}, {"N1"=187.13, "N2"=256.915, "N3"=0.00010066126264276298, "N4"=-1.0276367626954048e-05}, {"N1"=184.504, "N2"=257.002, "N3"=0.00010058865292160406, "N4"=-1.0413560771788407e-05}, {"N1"=184.504, "N2"=254.662, "N3"=0.00010059037275160661, "N4"=-1.0167167002920129e-05}, {"N1"=184.504, "N2"=252.015, "N3"=0.00010054666334783864, "N4"=-1.0509023833849896e-05}, {"N1"=184.504, "N2"=249.66, "N3"=0.00010049472511201633, "N4"=-1.0301718262494856e-05}, {"N1"=184.504, "N2"=247.351, "N3"=0.00010054614750886326, "N4"=-1.0347062752666793e-05}, {"N1"=184.504, "N2"=244.504, "N3"=0.00010064938286882759, "N4"=-1.0238012787382043e-05}, {"N1"=184.504, "N2"=242.002, "N3"=0.00010059504820740615, "N4"=-1.0449901619130157e-05}, {"N1"=184.504, "N2"=239.727, "N3"=0.00010062185568411652, "N4"=-1.0393539408979357e-05}, {"N1"=184.504, "N2"=237.299, "N3"=0.00010045063384983075, "N4"=-1.0268859103872335e-05}, {"N1"=184.504, "N2"=234.664, "N3"=0.00010053501606030399, "N4"=-1.0205976976529773e-05}, {"N1"=184.504, "N2"=231.991, "N3"=0.0001006286827361225, "N4"=-1.0257915445336476e-05}, {"N1"=184.504, "N2"=229.502, "N3"=0.00010050282065797416, "N4"=-1.008298843883937e-05}, {"N1"=184.504, "N2"=227.346, "N3"=0.000100611779365592, "N4"=-1.02938184637026e-05}, {"N1"=184.504, "N2"=224.866, "N3"=0.00010054791499493552, "N4"=-1.0141562516733599e-05}, {"N1"=184.504, "N2"=222.014, "N3"=0.00010062181181911447, "N4"=-1.0306009627423539e-05}, {"N1"=184.504, "N2"=219.867, "N3"=0.00010063023197977295, "N4"=-1.0374782923846605e-05}, {"N1"=184.676, "N2"=216.999, "N3"=0.0001005277051479229, "N4"=-1.0266818753325784e-05}, {"N1"=184.662, "N2"=214.498, "N3"=0.00010053693001922061, "N4"=-1.0330329797231284e-05}, {"N1"=184.677, "N2"=212.007, "N3"=0.00010058282265285195, "N4"=-1.035627437734821e-05}, {"N1"=184.676, "N2"=209.503, "N3"=0.00010060823300190782, "N4"=-1.0337046188399921e-05}, {"N1"=184.675, "N2"=206.998, "N3"=0.0001006829091124832, "N4"=-1.0373077841842383e-05}, {"N1"=184.668, "N2"=204.502, "N3"=0.00010061749675097556, "N4"=-1.0337837948793004e-05}, {"N1"=184.682, "N2"=202.007, "N3"=0.00010063459815530022, "N4"=-1.036227538375986e-05}, {"N1"=184.677, "N2"=199.504, "N3"=0.00010057544314753224, "N4"=-1.0399934309518636e-05}, {"N1"=184.673, "N2"=197.005, "N3"=0.00010070265673481819, "N4"=-1.0396287285154003e-05}, {"N1"=184.652, "N2"=194.496, "N3"=0.00010053547922922743, "N4"=-1.0418086156486104e-05}, {"N1"=184.67, "N2"=192.006, "N3"=0.00010059579658227902, "N4"=-1.0402015105569576e-05}, {"N1"=184.672, "N2"=189.5, "N3"=0.00010061569682931151, "N4"=-1.0134319438222533e-05}, {"N1"=184.67, "N2"=187.0, "N3"=0.00010057380903570334, "N4"=-1.0405290683878323e-05}, {"N1"=184.669, "N2"=184.5, "N3"=0.00010047722217336012, "N4"=-1.0367230872522774e-05}, {"N1"=184.665, "N2"=181.999, "N3"=0.00010060880092000912, "N4"=-1.0361291416871499e-05}, {"N1"=184.676, "N2"=179.499, "N3"=0.00010061482456302944, "N4"=-1.0522538377029939e-05}, {"N1"=184.678, "N2"=176.999, "N3"=0.00010062195859281164, "N4"=-1.035164978013157e-05}, {"N1"=184.67, "N2"=174.501, "N3"=0.00010062438396040221, "N4"=-1.0298221450096029e-05}, {"N1"=184.636, "N2"=171.999, "N3"=0.00010055345546514398, "N4"=-1.0358131838181341e-05}, {"N1"=184.674, "N2"=169.501, "N3"=0.00010050390446363961, "N4"=-1.042263095618173e-05}, {"N1"=184.662, "N2"=166.996, "N3"=0.0001006825990264115, "N4"=-1.0504232168865763e-05}, {"N1"=184.682, "N2"=164.52, "N3"=0.00010055466511977611, "N4"=-1.0403147541392191e-05}, {"N1"=184.674, "N2"=161.996, "N3"=0.00010058478715753651, "N4"=-1.0334858738086899e-05}, {"N1"=184.677, "N2"=159.505, "N3"=0.00010056067939185176, "N4"=-1.0309319124362399e-05}, {"N1"=184.672, "N2"=156.999, "N3"=0.00010059857095461566, "N4"=-1.0282080851684711e-05}, {"N1"=184.674, "N2"=154.5, "N3"=0.00010061526532846634, "N4"=-1.0418456017324834e-05}, {"N1"=184.682, "N2"=152.003, "N3"=0.00010051693196295312, "N4"=-1.0337491205647466e-05}, {"N1"=184.682, "N2"=149.509, "N3"=0.00010053890079761343, "N4"=-1.0403517270499351e-05}, {"N1"=184.666, "N2"=146.998, "N3"=0.00010075643050487386, "N4"=-1.0581079529169731e-05}, {"N1"=184.664, "N2"=144.496, "N3"=0.00010057788325799562, "N4"=-1.0248508032282926e-05}, {"N1"=182.154, "N2"=254.484, "N3"=0.0001005228266862595, "N4"=-1.0320640276482976e-05}, {"N1"=182.154, "N2"=251.999, "N3"=0.00010041612643578808, "N4"=-1.029034591187582e-05}, {"N1"=182.19, "N2"=249.503, "N3"=0.0001005418702379083, "N4"=-1.0107274266541032e-05}, {"N1"=182.192, "N2"=246.998, "N3"=0.00010069596661045965, "N4"=-1.044467352502349e-05}, {"N1"=182.196, "N2"=244.502, "N3"=0.00010062223338736789, "N4"=-1.0404214155486233e-05}, {"N1"=182.192, "N2"=242.0, "N3"=0.00010054296809495869, "N4"=-1.0357706743338664e-05}, {"N1"=182.194, "N2"=239.501, "N3"=0.00010059629840531535, "N4"=-1.0313954303766615e-05}, {"N1"=182.191, "N2"=236.994, "N3"=0.00010059864566966612, "N4"=-1.0447773037011574e-05}, {"N1"=182.199, "N2"=234.505, "N3"=0.00010050530681521679, "N4"=-1.0427765970498422e-05}, {"N1"=182.187, "N2"=231.994, "N3"=0.00010067607062458273, "N4"=-1.0548774757051225e-05}, {"N1"=182.197, "N2"=229.503, "N3"=0.00010063282891798748, "N4"=-1.0437269325049078e-05}, {"N1"=182.187, "N2"=227.0, "N3"=0.00010063996932031998, "N4"=-1.0370417567571988e-05}, {"N1"=182.19, "N2"=224.498, "N3"=0.00010056726878312552, "N4"=-1.03599009828373e-05}, {"N1"=182.2, "N2"=222.001, "N3"=0.00010064804362076197, "N4"=-1.0311621371166104e-05}, {"N1"=182.202, "N2"=219.504, "N3"=0.00010063665671695525, "N4"=-1.0513499784442607e-05}, {"N1"=182.189, "N2"=217.008, "N3"=0.00010054850449051165, "N4"=-1.0399421359489461e-05}, {"N1"=182.191, "N2"=214.502, "N3"=0.00010054825225798077, "N4"=-1.0389796810447088e-05}, {"N1"=182.195, "N2"=211.998, "N3"=0.0001006371102507405, "N4"=-1.035884378338865e-05}, {"N1"=182.177, "N2"=209.494, "N3"=0.0001005418293118631, "N4"=-1.0606910342392814e-05}, {"N1"=182.193, "N2"=207.0, "N3"=0.00010048796834559383, "N4"=-1.046365618180543e-05}, {"N1"=182.205, "N2"=204.506, "N3"=0.00010053784773541875, "N4"=-1.0356783177716566e-05}, {"N1"=182.21, "N2"=202.0, "N3"=0.00010058145737585234, "N4"=-1.0313437763917822e-05}, {"N1"=182.209, "N2"=199.502, "N3"=0.00010060472034277179, "N4"=-1.0397894862159398e-05}, {"N1"=182.208, "N2"=197.002, "N3"=0.00010058214212044629, "N4"=-1.0397273362676702e-05}, {"N1"=182.193, "N2"=194.497, "N3"=0.00010057097663167662, "N4"=-1.0342855635282052e-05}, {"N1"=182.191, "N2"=191.999, "N3"=0.000100542400573095, "N4"=-1.031201011769828e-05}, {"N1"=182.197, "N2"=189.501, "N3"=0.00010059086249518053, "N4"=-1.0386476734764882e-05}, {"N1"=182.197, "N2"=187.0, "N3"=0.00010058561495084324, "N4"=-1.0316108211477523e-05}, {"N1"=182.201, "N2"=184.503, "N3"=0.00010060505409270737, "N4"=-1.0406098887001503e-05}, {"N1"=179.588, "N2"=184.501, "N3"=0.00010063616940509914, "N4"=-1.0346617565174347e-05}, {"N1"=179.656, "N2"=187.006, "N3"=0.00010065555893805825, "N4"=-1.0480888221949916e-05}, {"N1"=179.673, "N2"=189.499, "N3"=0.00010054564226578889, "N4"=-1.043977356501652e-05}, {"N1"=179.665, "N2"=192.02, "N3"=0.00010052428072671487, "N4"=-1.0320044432249768e-05}, {"N1"=179.642, "N2"=194.499, "N3"=0.00010055027974563369, "N4"=-1.0284036331376105e-05}, {"N1"=179.69, "N2"=197.0, "N3"=0.00010067895646756075, "N4"=-1.037442130107441e-05}, {"N1"=179.684, "N2"=199.497, "N3"=0.00010054489452526912, "N4"=-1.038634563507568e-05}, {"N1"=179.695, "N2"=202.007, "N3"=0.00010052154530700064, "N4"=-1.0328663797121323e-05}, {"N1"=179.69, "N2"=204.509, "N3"=0.0001005926642830983, "N4"=-1.041093978537501e-05}, {"N1"=179.689, "N2"=206.998, "N3"=0.0001006624751248665, "N4"=-1.0310725218335403e-05}, {"N1"=179.653, "N2"=209.492, "N3"=0.00010060292275900545, "N4"=-1.0302538350643192e-05}, {"N1"=179.69, "N2"=212.006, "N3"=0.00010050545946527583, "N4"=-1.0482385922550538e-05}, {"N1"=179.689, "N2"=214.502, "N3"=0.0001005631085927493, "N4"=-1.0165697947928522e-05}, {"N1"=179.696, "N2"=217.002, "N3"=0.0001005842810374032, "N4"=-1.0176336430683493e-05}, {"N1"=179.615, "N2"=219.494, "N3"=0.00010060545610708717, "N4"=-1.0323182651774049e-05}, {"N1"=179.69, "N2"=221.998, "N3"=0.00010062674013239683, "N4"=-1.0234555101538814e-05}, {"N1"=179.697, "N2"=224.501, "N3"=0.00010060019569530594, "N4"=-1.0472314513525755e-05}, {"N1"=179.688, "N2"=226.999, "N3"=0.00010066126588863499, "N4"=-1.0319298576540959e-05}, {"N1"=179.687, "N2"=229.498, "N3"=0.00010066164580328467, "N4"=-1.025975396082442e-05}, {"N1"=179.7, "N2"=232.002, "N3"=0.00010059939512870188, "N4"=-1.0557285793716774e-05}, {"N1"=179.701, "N2"=234.509, "N3"=0.00010053158585883804, "N4"=-1.0228406572700483e-05}, {"N1"=179.708, "N2"=236.999, "N3"=0.00010061959633397193, "N4"=-1.0297830329735278e-05}, {"N1"=179.549, "N2"=239.506, "N3"=0.00010064967011407564, "N4"=-1.05889259617004e-05}, {"N1"=179.684, "N2"=242.0, "N3"=0.00010037627995397305, "N4"=-1.040295003289471e-05}, {"N1"=179.627, "N2"=244.499, "N3"=0.00010061424989600551, "N4"=-1.0299384469636194e-05}, {"N1"=179.698, "N2"=247.002, "N3"=0.00010058365592809027, "N4"=-1.0496451474700274e-05}, {"N1"=179.697, "N2"=249.502, "N3"=0.00010061583530648307, "N4"=-1.0431406585168696e-05}, {"N1"=179.698, "N2"=252.0, "N3"=0.00010066307370658188, "N4"=-1.0395753885085858e-05}, {"N1"=179.7, "N2"=254.503, "N3"=0.00010052555325657566, "N4"=-1.0581098634928242e-05}, {"N1"=177.102, "N2"=254.497, "N3"=0.00010048555745751602, "N4"=-1.0386816651810863e-05}, {"N1"=177.137, "N2"=251.998, "N3"=0.00010059759389104031, "N4"=-1.0153478822088376e-05}, {"N1"=177.183, "N2"=249.501, "N3"=0.000100537857748161, "N4"=-1.0329557925633957e-05}, {"N1"=177.185, "N2"=246.999, "N3"=0.00010055447323204678, "N4"=-1.0368566550224198e-05}, {"N1"=177.189, "N2"=244.5, "N3"=0.00010056221783611028, "N4"=-1.0382946243989625e-05}, {"N1"=177.192, "N2"=242.001, "N3"=0.00010069481721494526, "N4"=-1.0383898894730616e-05}, {"N1"=177.187, "N2"=239.506, "N3"=0.00010058983231924863, "N4"=-1.0366846787549775e-05}, {"N1"=177.177, "N2"=236.999, "N3"=0.00010050101429309329, "N4"=-1.0363531734940847e-05}, {"N1"=177.192, "N2"=234.497, "N3"=0.00010062033004765729, "N4"=-1.0323968376937155e-05}, {"N1"=177.186, "N2"=231.995, "N3"=0.00010058413040989756, "N4"=-1.0383102834931026e-05}, {"N1"=177.2, "N2"=229.506, "N3"=0.00010045518994180424, "N4"=-1.042239591152223e-05}, {"N1"=177.179, "N2"=226.999, "N3"=0.00010048041293317921, "N4"=-1.0263383880804631e-05}, {"N1"=177.183, "N2"=224.499, "N3"=0.00010071286959190333, "N4"=-1.0339318502571861e-05}, {"N1"=177.186, "N2"=221.995, "N3"=0.00010059400792826088, "N4"=-1.0449054784554912e-05}, {"N1"=177.158, "N2"=219.495, "N3"=0.00010053505722966405, "N4"=-1.0472546356348127e-05}, {"N1"=177.197, "N2"=217.0, "N3"=0.0001005921550973305, "N4"=-1.0373497084032953e-05}, {"N1"=177.203, "N2"=214.503, "N3"=0.00010054778122167157, "N4"=-1.0269459682578653e-05}, {"N1"=177.194, "N2"=211.993, "N3"=0.00010055533647499167, "N4"=-1.0280953807681494e-05}, {"N1"=177.168, "N2"=209.498, "N3"=0.00010057971757330195, "N4"=-1.0502428665994152e-05}, {"N1"=177.207, "N2"=207.002, "N3"=0.00010063009929595163, "N4"=-1.0451516427657889e-05}, {"N1"=177.203, "N2"=204.504, "N3"=0.00010060522268642766, "N4"=-1.0381643154015022e-05}, {"N1"=177.202, "N2"=202.001, "N3"=0.0001004996141450169, "N4"=-1.0429244923116366e-05}, {"N1"=177.198, "N2"=199.511, "N3"=0.00010062412150139144, "N4"=-1.0304515823025727e-05}, {"N1"=177.202, "N2"=197.003, "N3"=0.00010057485897462646, "N4"=-1.041353011796818e-05}, {"N1"=177.194, "N2"=194.503, "N3"=0.00010044384844484558, "N4"=-1.0106364077812626e-05}, {"N1"=177.201, "N2"=192.001, "N3"=0.00010060196900009477, "N4"=-1.041383927467444e-05}, {"N1"=177.207, "N2"=189.497, "N3"=0.00010054079156093745, "N4"=-1.0350166348202287e-05}, {"N1"=177.206, "N2"=187.002, "N3"=0.00010056306483115067, "N4"=-1.0374352214990319e-05}, {"N1"=177.218, "N2"=184.509, "N3"=0.0001005764672463416, "N4"=-1.0345034109409499e-05}, {"N1"=174.571, "N2"=184.493, "N3"=0.00010072866807588699, "N4"=-1.029687447840569e-05}, {"N1"=174.65, "N2"=187.003, "N3"=0.000100485986306007, "N4"=-1.0459243065894773e-05}, {"N1"=174.658, "N2"=189.505, "N3"=0.00010063758223053145, "N4"=-1.0364681770711236e-05}, {"N1"=174.653, "N2"=191.998, "N3"=0.00010052738678345106, "N4"=-1.0432268863797004e-05}, {"N1"=174.646, "N2"=194.5, "N3"=0.0001005670859205579, "N4"=-1.0340561490660886e-05}, {"N1"=174.684, "N2"=197.015, "N3"=0.00010047454940461702, "N4"=-1.0411449152606119e-05}, {"N1"=174.673, "N2"=199.499, "N3"=0.00010063638529204644, "N4"=-1.0419233542543256e-05}, {"N1"=174.682, "N2"=202.011, "N3"=0.00010061527337342576, "N4"=-1.0392112452181738e-05}, {"N1"=174.676, "N2"=204.493, "N3"=0.00010063932969324114, "N4"=-1.0205101205046129e-05}, {"N1"=174.687, "N2"=207.01, "N3"=0.00010050634990863304, "N4"=-1.037532209054735e-05}, {"N1"=174.674, "N2"=209.5, "N3"=0.00010063847531389078, "N4"=-1.0300039421451099e-05}, {"N1"=174.671, "N2"=212.001, "N3"=0.00010060084805033301, "N4"=-1.0497005381869963e-05}, {"N1"=174.67, "N2"=214.503, "N3"=0.00010061356385345521, "N4"=-1.0196774324362367e-05}, {"N1"=174.668, "N2"=216.997, "N3"=0.00010061524473087806, "N4"=-1.0334329796891949e-05}, {"N1"=174.662, "N2"=219.501, "N3"=0.00010057410210229362, "N4"=-1.0331382769647341e-05}, {"N1"=174.669, "N2"=222.004, "N3"=0.00010051124469771391, "N4"=-1.0297241823616087e-05}, {"N1"=174.672, "N2"=224.497, "N3"=0.00010072919871038887, "N4"=-1.0422662026231325e-05}, {"N1"=174.672, "N2"=226.997, "N3"=0.00010063774158155976, "N4"=-1.0255244115338244e-05}, {"N1"=174.62, "N2"=229.501, "N3"=0.00010064995527971172, "N4"=-1.0224462296017921e-05}, {"N1"=174.674, "N2"=232.011, "N3"=0.00010062112250728264, "N4"=-1.0397636295264744e-05}, {"N1"=174.677, "N2"=234.499, "N3"=0.00010055436207432691, "N4"=-1.0281127842375146e-05}, {"N1"=174.67, "N2"=237.001, "N3"=0.00010050617276623229, "N4"=-1.027258178442683e-05}, {"N1"=174.549, "N2"=239.504, "N3"=0.00010050484095148279, "N4"=-1.031200458815883e-05}, {"N1"=174.675, "N2"=242.002, "N3"=0.00010061105085279847, "N4"=-1.054470283941695e-05}, {"N1"=174.66, "N2"=244.499, "N3"=0.0001006543242287764, "N4"=-1.0573445930777054e-05}, {"N1"=174.675, "N2"=246.999, "N3"=0.00010061747366050946, "N4"=-1.0339165989216521e-05}, {"N1"=174.687, "N2"=249.5, "N3"=0.00010062444313943346, "N4"=-1.039956754348585e-05}, {"N1"=174.667, "N2"=251.997, "N3"=0.00010051804426435225, "N4"=-1.0342258611695435e-05}, {"N1"=174.662, "N2"=254.498, "N3"=0.00010055232259890577, "N4"=-1.045142564050838e-05}, {"N1"=172.115, "N2"=254.491, "N3"=0.00010051686117666405, "N4"=-1.0388854735803942e-05}, {"N1"=172.164, "N2"=251.996, "N3"=0.0001006414820498013, "N4"=-1.0054974529688774e-05}, {"N1"=172.19, "N2"=249.505, "N3"=0.00010056147694537137, "N4"=-1.0284964750875155e-05}, {"N1"=172.191, "N2"=246.997, "N3"=0.00010060688637063793, "N4"=-1.0270710291712582e-05}, {"N1"=172.186, "N2"=244.501, "N3"=0.00010056424994078149, "N4"=-1.0298647667606897e-05}, {"N1"=172.177, "N2"=241.999, "N3"=0.00010051479907519292, "N4"=-1.0142310174587072e-05}, {"N1"=172.172, "N2"=239.499, "N3"=0.00010056352317475037, "N4"=-1.0253836497988945e-05}, {"N1"=172.189, "N2"=237.006, "N3"=0.00010064045328109252, "N4"=-1.0410486615616051e-05}, {"N1"=172.174, "N2"=234.489, "N3"=0.00010064704779005822, "N4"=-1.0423936208343195e-05}, {"N1"=172.184, "N2"=231.999, "N3"=0.0001005800423486196, "N4"=-1.0586593352628624e-05}, {"N1"=172.188, "N2"=229.502, "N3"=0.00010059027590518583, "N4"=-1.0331123081686343e-05}, {"N1"=172.189, "N2"=227.005, "N3"=0.00010068451897971222, "N4"=-1.0168074987990413e-05}, {"N1"=172.184, "N2"=224.497, "N3"=0.00010053358872492644, "N4"=-1.0289763013672919e-05}, {"N1"=172.184, "N2"=221.997, "N3"=0.0001006372130003581, "N4"=-1.0481774014161902e-05}, {"N1"=172.195, "N2"=219.501, "N3"=0.0001005904343064764, "N4"=-1.0389478667070903e-05}, {"N1"=172.201, "N2"=217.003, "N3"=0.00010053807792962248, "N4"=-1.0329489634346316e-05}, {"N1"=172.191, "N2"=214.494, "N3"=0.00010045730072107484, "N4"=-1.0417370122834706e-05}, {"N1"=172.192, "N2"=211.999, "N3"=0.00010048814039782801, "N4"=-1.0409257057633277e-05}, {"N1"=172.19, "N2"=209.498, "N3"=0.00010057360657568786, "N4"=-1.0254523689738158e-05}, {"N1"=172.189, "N2"=206.998, "N3"=0.00010045587934314887, "N4"=-1.0288711787228305e-05}, {"N1"=172.198, "N2"=204.505, "N3"=0.00010056220129472909, "N4"=-1.0070555701615801e-05}, {"N1"=172.176, "N2"=202.002, "N3"=0.00010064757794587837, "N4"=-1.0294114382088938e-05}, {"N1"=172.195, "N2"=199.498, "N3"=0.00010062406927801754, "N4"=-1.0492634029975401e-05}, {"N1"=172.192, "N2"=197.007, "N3"=0.00010061760060688045, "N4"=-1.0319016762631358e-05}, {"N1"=172.19, "N2"=194.498, "N3"=0.0001006768879635731, "N4"=-1.0495769795981891e-05}, {"N1"=172.184, "N2"=191.993, "N3"=0.00010064513924344042, "N4"=-1.0260890454632586e-05}, {"N1"=172.187, "N2"=189.502, "N3"=0.00010062987674075304, "N4"=-1.0247210788922372e-05}, {"N1"=172.194, "N2"=187.016, "N3"=0.00010055542473272687, "N4"=-1.0399342866811968e-05}, {"N1"=172.185, "N2"=184.501, "N3"=0.00010051081253480909, "N4"=-1.038332393606816e-05}, {"N1"=169.563, "N2"=184.497, "N3"=0.00010057564127638256, "N4"=-1.0485856185273882e-05}, {"N1"=169.651, "N2"=187.004, "N3"=0.00010066079330302313, "N4"=-1.0464470154247918e-05}, {"N1"=169.652, "N2"=189.5, "N3"=0.00010049759588790874, "N4"=-1.0147858256438632e-05}, {"N1"=169.665, "N2"=192.012, "N3"=0.00010057660017072396, "N4"=-1.0362647190816887e-05}, {"N1"=169.623, "N2"=194.496, "N3"=0.0001005112713275198, "N4"=-1.0234816069322997e-05}, {"N1"=169.669, "N2"=197.0, "N3"=0.0001004700649591163, "N4"=-1.0301567365730803e-05}, {"N1"=169.681, "N2"=199.501, "N3"=0.00010054694945842724, "N4"=-1.0288530492477278e-05}, {"N1"=169.657, "N2"=202.0, "N3"=0.00010061466789349555, "N4"=-1.0370879859008016e-05}, {"N1"=169.679, "N2"=204.506, "N3"=0.00010057761059978556, "N4"=-1.0411547644922838e-05}, {"N1"=169.68, "N2"=207.011, "N3"=0.00010052892107143731, "N4"=-1.0345931532869249e-05}, {"N1"=169.659, "N2"=209.5, "N3"=0.00010057331488656413, "N4"=-1.0305138964679457e-05}, {"N1"=169.683, "N2"=212.005, "N3"=0.00010049854978679058, "N4"=-1.0444554288430891e-05}, {"N1"=169.643, "N2"=214.488, "N3"=0.00010064361521584659, "N4"=-1.0231382961806053e-05}, {"N1"=169.696, "N2"=217.01, "N3"=0.00010057201619316158, "N4"=-1.0273976312836689e-05}, {"N1"=169.689, "N2"=219.499, "N3"=0.00010056240201869727, "N4"=-1.0397294429770199e-05}, {"N1"=169.695, "N2"=222.007, "N3"=0.00010058393849249667, "N4"=-1.0563435601418958e-05}, {"N1"=169.694, "N2"=224.504, "N3"=0.00010062342773689217, "N4"=-1.027479502943902e-05}, {"N1"=169.693, "N2"=227.004, "N3"=0.00010060142019270304, "N4"=-1.0440565255336727e-05}, {"N1"=169.646, "N2"=229.498, "N3"=0.00010045983366748363, "N4"=-1.0549573493660818e-05}, {"N1"=169.693, "N2"=232.0, "N3"=0.00010060860524726317, "N4"=-1.0490586065317864e-05}, {"N1"=169.698, "N2"=234.499, "N3"=0.0001004620166549092, "N4"=-1.0355874221948874e-05}, {"N1"=169.698, "N2"=237.001, "N3"=0.00010045953472266104, "N4"=-1.0287812797728431e-05}, {"N1"=169.669, "N2"=239.504, "N3"=0.00010060445077700746, "N4"=-1.0446724440658474e-05}, {"N1"=169.7, "N2"=242.003, "N3"=0.00010062231607050165, "N4"=-9.966647343258625e-06}, {"N1"=169.634, "N2"=244.497, "N3"=0.00010053943024300296, "N4"=-1.0366991371883932e-05}, {"N1"=169.694, "N2"=247.002, "N3"=0.00010060203540456271, "N4"=-1.0589080912723271e-05}, {"N1"=169.698, "N2"=249.499, "N3"=0.0001005270987376022, "N4"=-1.018610807636997e-05}, {"N1"=169.709, "N2"=252.001, "N3"=0.00010060138099867682, "N4"=-1.0297077075708232e-05}, {"N1"=169.706, "N2"=254.503, "N3"=0.00010055233210342543, "N4"=-1.0308382448634867e-05}, {"N1"=167.097, "N2"=254.496, "N3"=0.00010055323748903371, "N4"=-1.0295554297436698e-05}, {"N1"=167.183, "N2"=252.006, "N3"=0.0001005731980104857, "N4"=-1.0508893095794842e-05}, {"N1"=167.169, "N2"=249.497, "N3"=0.0001006541466741243, "N4"=-1.0462661197045484e-05}, {"N1"=167.173, "N2"=247.004, "N3"=0.00010050252083091611, "N4"=-1.0391793226125795e-05}, {"N1"=167.176, "N2"=244.499, "N3"=0.00010061911516447071, "N4"=-1.042743786596333e-05}, {"N1"=167.184, "N2"=241.999, "N3"=0.0001005972017832446, "N4"=-1.0381523237597055e-05}, {"N1"=167.176, "N2"=239.5, "N3"=0.00010061270376565658, "N4"=-1.0391382418108855e-05}, {"N1"=167.175, "N2"=236.994, "N3"=0.00010052984442463315, "N4"=-1.0378537328507458e-05}, {"N1"=167.178, "N2"=234.492, "N3"=0.00010056685022607013, "N4"=-1.0443249324212588e-05}, {"N1"=167.175, "N2"=231.992, "N3"=0.00010058796799152978, "N4"=-1.041822884297264e-05}, {"N1"=167.172, "N2"=229.499, "N3"=0.00010067165956468124, "N4"=-1.0401015599978216e-05}, {"N1"=167.164, "N2"=226.998, "N3"=0.00010045940880956217, "N4"=-1.0310865849866963e-05}, {"N1"=167.174, "N2"=224.495, "N3"=0.00010063601659370512, "N4"=-1.0476373134599244e-05}, {"N1"=167.184, "N2"=221.999, "N3"=0.00010061578555971528, "N4"=-1.0292484737972615e-05}, {"N1"=167.177, "N2"=219.498, "N3"=0.00010056856621518597, "N4"=-1.0260227548745439e-05}, {"N1"=167.19, "N2"=217.002, "N3"=0.00010061301942774867, "N4"=-1.0239518843107783e-05}, {"N1"=167.193, "N2"=214.501, "N3"=0.00010047026271902722, "N4"=-1.0398967465937847e-05}, {"N1"=167.182, "N2"=212.003, "N3"=0.00010053355907538146, "N4"=-1.0500875061622776e-05}, {"N1"=167.179, "N2"=209.497, "N3"=0.00010052410468545998, "N4"=-1.0130521793911515e-05}, {"N1"=167.182, "N2"=207.005, "N3"=0.00010062906017382527, "N4"=-1.0305147422099646e-05}, {"N1"=167.185, "N2"=204.501, "N3"=0.00010049102215116068, "N4"=-1.0619072161567706e-05}, {"N1"=167.184, "N2"=202.008, "N3"=0.00010056727455622281, "N4"=-1.0400836774709033e-05}, {"N1"=167.176, "N2"=199.503, "N3"=0.00010053051641833995, "N4"=-1.0355051827182074e-05}, {"N1"=167.186, "N2"=197.001, "N3"=0.00010057924178788546, "N4"=-1.0442360512442227e-05}, {"N1"=167.175, "N2"=194.502, "N3"=0.00010062024431056108, "N4"=-1.0424079782696805e-05}, {"N1"=167.17, "N2"=191.999, "N3"=0.00010057885569335226, "N4"=-1.0181100769330292e-05}, {"N1"=167.183, "N2"=189.501, "N3"=0.00010058643083420424, "N4"=-1.0458272218985298e-05}, {"N1"=167.186, "N2"=186.999, "N3"=0.0001005120077863805, "N4"=-1.0224871308968336e-05}, {"N1"=167.184, "N2"=184.5, "N3"=0.00010051024336397331, "N4"=-1.0359181292938607e-05}, {"N1"=164.612, "N2"=184.487, "N3"=0.00010068444454775948, "N4"=-1.0277184356841555e-05}, {"N1"=164.685, "N2"=186.993, "N3"=0.00010056219876634349, "N4"=-1.056935949569249e-05}, {"N1"=164.697, "N2"=189.501, "N3"=0.0001005383853038811, "N4"=-1.0356786255029424e-05}, {"N1"=164.69, "N2"=191.996, "N3"=0.00010050455846528987, "N4"=-1.0315227556939213e-05}, {"N1"=164.641, "N2"=194.491, "N3"=0.00010047586454124057, "N4"=-1.0479495773678329e-05}, {"N1"=164.701, "N2"=197.001, "N3"=0.00010050476369027672, "N4"=-1.0258960773707157e-05}, {"N1"=164.689, "N2"=199.499, "N3"=0.00010063690443383835, "N4"=-1.0284191731486123e-05}, {"N1"=164.7, "N2"=202.0, "N3"=0.00010058932238884035, "N4"=-1.0378866116192078e-05}, {"N1"=164.71, "N2"=204.511, "N3"=0.00010056518527380809, "N4"=-1.0381587219565184e-05}, {"N1"=164.702, "N2"=207.001, "N3"=0.00010048329748186218, "N4"=-1.0413294299592136e-05}, {"N1"=164.67, "N2"=209.502, "N3"=0.0001005170168710166, "N4"=-1.0214495985341898e-05}, {"N1"=164.712, "N2"=211.998, "N3"=0.00010058171905587996, "N4"=-1.0325150526639756e-05}, {"N1"=164.714, "N2"=214.511, "N3"=0.00010054708777904731, "N4"=-1.0387927617555442e-05}, {"N1"=164.708, "N2"=217.001, "N3"=0.00010062209381520189, "N4"=-1.0336454913694004e-05}, {"N1"=164.652, "N2"=219.505, "N3"=0.0001005896209920459, "N4"=-1.0341047770826337e-05}, {"N1"=164.687, "N2"=221.99, "N3"=0.00010056464456567054, "N4"=-1.0284176107136435e-05}, {"N1"=164.708, "N2"=224.497, "N3"=0.00010061144394982626, "N4"=-1.03625311683962e-05}, {"N1"=164.71, "N2"=226.996, "N3"=0.00010050567449272583, "N4"=-1.0341416738097949e-05}, {"N1"=164.719, "N2"=229.509, "N3"=0.00010074836704543797, "N4"=-1.0235496402675522e-05}, {"N1"=164.715, "N2"=232.0, "N3"=0.00010054298852051879, "N4"=-1.0353246737409088e-05}, {"N1"=164.69, "N2"=234.507, "N3"=0.00010055319918718821, "N4"=-1.024795931649671e-05}, {"N1"=164.717, "N2"=237.0, "N3"=0.0001006107078652486, "N4"=-1.0371489595238984e-05}, {"N1"=164.612, "N2"=239.499, "N3"=0.00010059639064008739, "N4"=-1.0365996760995914e-05}, {"N1"=164.707, "N2"=242.0, "N3"=0.0001006776099516418, "N4"=-1.0437891859427039e-05}, {"N1"=164.721, "N2"=244.497, "N3"=0.00010057249844747878, "N4"=-1.0374347206260776e-05}, {"N1"=164.708, "N2"=246.996, "N3"=0.00010061517834854645, "N4"=-1.0433753441773959e-05}, {"N1"=164.714, "N2"=249.504, "N3"=0.00010060224841593455, "N4"=-1.0511257037897375e-05}, {"N1"=164.698, "N2"=251.999, "N3"=0.00010050236472987877, "N4"=-1.0345082307200191e-05}, {"N1"=164.728, "N2"=254.495, "N3"=0.00010057186517266543, "N4"=-1.0367279025278467e-05}, {"N1"=162.06, "N2"=254.495, "N3"=0.00010063729839163527, "N4"=-1.0362379770043512e-05}, {"N1"=162.141, "N2"=252.0, "N3"=0.00010056237791561374, "N4"=-1.034224319013826e-05}, {"N1"=162.153, "N2"=249.504, "N3"=0.0001004655893511692, "N4"=-1.059366525247979e-05}, {"N1"=162.157, "N2"=247.001, "N3"=0.00010058027596434067, "N4"=-1.0337699146953011e-05}, {"N1"=162.159, "N2"=244.5, "N3"=0.00010060685361868647, "N4"=-1.0387037123043438e-05}, {"N1"=162.16, "N2"=242.005, "N3"=0.00010059671372319361, "N4"=-1.012455465864298e-05}, {"N1"=162.163, "N2"=239.498, "N3"=0.00010061014758433187, "N4"=-1.0381558382614488e-05}, {"N1"=162.164, "N2"=236.998, "N3"=0.00010053110616205387, "N4"=-1.0411523057746539e-05}, {"N1"=162.158, "N2"=234.504, "N3"=0.00010045925574865349, "N4"=-1.032577219901195e-05}, {"N1"=162.151, "N2"=232.002, "N3"=0.00010053469123793202, "N4"=-1.0324978675779233e-05}, {"N1"=162.147, "N2"=229.507, "N3"=0.00010047711290579158, "N4"=-1.0577794785973643e-05}, {"N1"=162.151, "N2"=227.0, "N3"=0.000100583750598305, "N4"=-1.0252292798054244e-05}, {"N1"=162.156, "N2"=224.502, "N3"=0.00010051040052604691, "N4"=-1.0497424972670217e-05}, {"N1"=162.151, "N2"=221.999, "N3"=0.00010057981312098673, "N4"=-1.0490640200134917e-05}, {"N1"=162.154, "N2"=219.494, "N3"=0.00010055861065495857, "N4"=-1.0308532882452357e-05}, {"N1"=162.161, "N2"=217.008, "N3"=0.00010053317572877121, "N4"=-1.017373575937342e-05}, {"N1"=162.062, "N2"=214.484, "N3"=0.00010065132494397626, "N4"=-1.0386328413876784e-05}, {"N1"=162.081, "N2"=212.004, "N3"=0.00010051304618895223, "N4"=-1.0119640698762242e-05}, {"N1"=162.06, "N2"=209.5, "N3"=0.00010060637483988311, "N4"=-1.0356664369281701e-05}, {"N1"=162.072, "N2"=207.001, "N3"=0.00010061797220147472, "N4"=-1.0331096772687592e-05}, {"N1"=162.071, "N2"=204.5, "N3"=0.00010040878414042545, "N4"=-1.0317256898137698e-05}, {"N1"=162.033, "N2"=201.988, "N3"=0.00010049317424853139, "N4"=-1.0269185405696788e-05}, {"N1"=162.076, "N2"=199.5, "N3"=0.00010064470280000817, "N4"=-1.0410930238069582e-05}, {"N1"=162.07, "N2"=196.996, "N3"=0.00010061036931313751, "N4"=-1.0162747163073602e-05}, {"N1"=162.072, "N2"=194.502, "N3"=0.0001005799650069087, "N4"=-1.0332754147332612e-05}, {"N1"=162.083, "N2"=192.003, "N3"=0.0001004779610552684, "N4"=-1.038635033735244e-05}, {"N1"=162.084, "N2"=189.495, "N3"=0.00010060239037467525, "N4"=-1.039564976459955e-05}, {"N1"=162.088, "N2"=186.999, "N3"=0.00010063447588914267, "N4"=-1.056924071922337e-05}, {"N1"=162.093, "N2"=184.508, "N3"=0.0001005430259799713, "N4"=-1.0249951654566563e-05}, {"N1"=159.586, "N2"=184.492, "N3"=0.00010049120916944316, "N4"=-1.0347214881357189e-05}, {"N1"=159.665, "N2"=187.014, "N3"=0.00010059715176997785, "N4"=-1.0654984865295603e-05}, {"N1"=159.648, "N2"=189.501, "N3"=0.00010048358317273929, "N4"=-1.0491392340729304e-05}, {"N1"=159.669, "N2"=192.009, "N3"=0.00010057098338442595, "N4"=-1.0580473637981688e-05}, {"N1"=159.628, "N2"=194.493, "N3"=0.00010056465004307806, "N4"=-1.0359133354054748e-05}, {"N1"=159.683, "N2"=196.998, "N3"=0.00010064769270639601, "N4"=-1.0547121397763753e-05}, {"N1"=159.681, "N2"=199.503, "N3"=0.00010054911844227734, "N4"=-1.0427850892176607e-05}, {"N1"=159.673, "N2"=202.016, "N3"=0.00010059216167829333, "N4"=-1.0394476581802831e-05}, {"N1"=159.679, "N2"=204.504, "N3"=0.00010055603092307458, "N4"=-1.03225494068049e-05}, {"N1"=159.678, "N2"=207.008, "N3"=0.00010047424445919067, "N4"=-1.0349693237252857e-05}, {"N1"=159.661, "N2"=209.491, "N3"=0.0001005625953371467, "N4"=-1.0303306306932754e-05}, {"N1"=159.682, "N2"=211.999, "N3"=0.00010067045101782425, "N4"=-1.0338707016838153e-05}, {"N1"=159.678, "N2"=214.511, "N3"=0.00010052455123519654, "N4"=-1.040957230881374e-05}, {"N1"=159.681, "N2"=217.0, "N3"=0.00010062375059846504, "N4"=-1.0387502534429516e-05}, {"N1"=159.631, "N2"=219.499, "N3"=0.00010064392550265344, "N4"=-1.0256915317709298e-05}, {"N1"=159.673, "N2"=221.999, "N3"=0.00010063480028147744, "N4"=-1.0443971192238724e-05}, {"N1"=159.678, "N2"=224.504, "N3"=0.00010047216015381788, "N4"=-1.0372311059328435e-05}, {"N1"=159.671, "N2"=226.996, "N3"=0.00010060990644050815, "N4"=-1.0499123345119184e-05}, {"N1"=159.643, "N2"=229.507, "N3"=0.0001004050069800666, "N4"=-1.0309576444389373e-05}, {"N1"=159.672, "N2"=232.013, "N3"=0.00010065108981697429, "N4"=-1.0240383097282447e-05}, {"N1"=159.667, "N2"=234.502, "N3"=0.00010057880902161669, "N4"=-1.0414677749914856e-05}, {"N1"=159.675, "N2"=237.003, "N3"=0.00010060586695214941, "N4"=-1.0419020569264407e-05}, {"N1"=159.636, "N2"=239.498, "N3"=0.00010057025519349663, "N4"=-1.047650850179947e-05}, {"N1"=159.681, "N2"=242.009, "N3"=0.00010060686310376392, "N4"=-1.025625267415124e-05}, {"N1"=159.672, "N2"=244.502, "N3"=0.00010051375830790238, "N4"=-1.0239087992064942e-05}, {"N1"=159.674, "N2"=247.006, "N3"=0.00010053004362397551, "N4"=-1.0378076737151689e-05}, {"N1"=159.673, "N2"=249.501, "N3"=0.00010059546073768384, "N4"=-1.0420651184153005e-05}, {"N1"=159.682, "N2"=252.004, "N3"=0.0001005603285545853, "N4"=-1.0294325889061525e-05}, {"N1"=159.682, "N2"=254.507, "N3"=0.00010058808018336061, "N4"=-1.0510559651184475e-05}, {"N1"=117.123, "N2"=267.003, "N3"=0.00010067129746453202, "N4"=-1.024290124981069e-05}, {"N1"=117.203, "N2"=264.5, "N3"=0.00010062292682362226, "N4"=-1.0283976676837624e-05}, {"N1"=117.181, "N2"=262.0, "N3"=0.0001004688199897459, "N4"=-1.0264752668153745e-05}, {"N1"=117.176, "N2"=259.501, "N3"=0.00010054797724566015, "N4"=-1.0228895847046031e-05}, {"N1"=117.188, "N2"=257.0, "N3"=0.00010052232010495917, "N4"=-1.0353439920672607e-05}, {"N1"=117.185, "N2"=254.5, "N3"=0.00010057461980159789, "N4"=-1.0462273969466404e-05}, {"N1"=117.186, "N2"=252.002, "N3"=0.00010053770936291817, "N4"=-1.0315879053515138e-05}, {"N1"=117.189, "N2"=249.505, "N3"=0.00010073252285522125, "N4"=-1.0333633299456483e-05}, {"N1"=117.19, "N2"=247.004, "N3"=0.00010068100516319383, "N4"=-1.0196642212430384e-05}, {"N1"=114.548, "N2"=247.002, "N3"=0.00010042786687336703, "N4"=-1.02667717379889e-05}, {"N1"=114.62, "N2"=249.495, "N3"=0.00010064530971303591, "N4"=-1.0272076491187834e-05}, {"N1"=114.626, "N2"=252.002, "N3"=0.00010054024472804827, "N4"=-1.0327149439822778e-05}, {"N1"=114.618, "N2"=254.499, "N3"=0.0001005979314468822, "N4"=-1.0421395302032924e-05}, {"N1"=114.629, "N2"=257.001, "N3"=0.00010059653364665182, "N4"=-1.0310110926418404e-05}, {"N1"=114.635, "N2"=259.5, "N3"=0.00010059434287913416, "N4"=-1.0266011237306022e-05}, {"N1"=114.631, "N2"=262.0, "N3"=0.0001004621620673141, "N4"=-1.0109218949034534e-05}, {"N1"=114.626, "N2"=264.498, "N3"=0.00010058412458445037, "N4"=-1.0337842680561553e-05}, {"N1"=114.641, "N2"=267.001, "N3"=0.00010060778885442503, "N4"=-1.0210290825223535e-05}, {"N1"=112.077, "N2"=267.001, "N3"=0.00010069711916332094, "N4"=-1.0236793600919145e-05}, {"N1"=112.148, "N2"=264.495, "N3"=0.00010062070092815818, "N4"=-1.0337806825137646e-05}, {"N1"=112.146, "N2"=262.0, "N3"=0.00010057628581603331, "N4"=-1.029581630119796e-05}, {"N1"=112.139, "N2"=259.5, "N3"=0.00010055074491980576, "N4"=-1.035400569852696e-05}, {"N1"=112.152, "N2"=256.999, "N3"=0.00010055624574738871, "N4"=-1.0254949339491484e-05}, {"N1"=112.14, "N2"=254.5, "N3"=0.00010056138271577749, "N4"=-1.028657839867459e-05}, {"N1"=112.132, "N2"=252.0, "N3"=0.00010059484921779787, "N4"=-1.0109842524207384e-05}, {"N1"=112.137, "N2"=249.5, "N3"=0.00010060239856359985, "N4"=-1.0304957532695906e-05}, {"N1"=112.126, "N2"=246.992, "N3"=0.00010047623437422644, "N4"=-1.0264771884878599e-05}, {"N1"=109.545, "N2"=246.991, "N3"=0.00010047251428951773, "N4"=-1.026374433289153e-05}, {"N1"=109.63, "N2"=249.493, "N3"=0.00010057916016005694, "N4"=-1.0156188205085047e-05}, {"N1"=109.639, "N2"=252.001, "N3"=0.00010051822406411564, "N4"=-1.0315636233188464e-05}, {"N1"=109.649, "N2"=254.498, "N3"=0.00010063395504480406, "N4"=-1.0210070790905946e-05}, {"N1"=109.665, "N2"=256.993, "N3"=0.0001005801884423354, "N4"=-1.0288150521002311e-05}, {"N1"=109.66, "N2"=259.493, "N3"=0.0001006153336217253, "N4"=-1.0091488432145692e-05}, {"N1"=109.656, "N2"=262.0, "N3"=0.00010068278959794761, "N4"=-1.0263983577893284e-05}, {"N1"=109.664, "N2"=264.498, "N3"=0.00010056056441971814, "N4"=-1.0237961530378919e-05}, {"N1"=109.677, "N2"=266.996, "N3"=0.00010058805648154425, "N4"=-1.0316467513949557e-05}, {"N1"=107.041, "N2"=266.995, "N3"=0.00010060447818857248, "N4"=-1.0266236420666362e-05}, {"N1"=107.165, "N2"=264.499, "N3"=0.00010059229515192147, "N4"=-1.0265641440307016e-05}, {"N1"=107.165, "N2"=261.997, "N3"=0.00010061999595869576, "N4"=-1.0202499061939264e-05}, {"N1"=107.142, "N2"=259.499, "N3"=0.00010066710792231959, "N4"=-1.0337546288340794e-05}, {"N1"=107.156, "N2"=257.002, "N3"=0.00010051977751008614, "N4"=-1.0201599973621467e-05}, {"N1"=107.149, "N2"=254.5, "N3"=0.0001005717282943262, "N4"=-1.0271241370175966e-05}, {"N1"=107.16, "N2"=251.997, "N3"=0.00010057147717808183, "N4"=-1.0354647022534269e-05}, {"N1"=107.159, "N2"=249.493, "N3"=0.00010054004773226875, "N4"=-1.0192142333102007e-05}, {"N1"=107.163, "N2"=246.989, "N3"=0.00010062997971821412, "N4"=-1.0291434430959109e-05}, {"N1"=104.521, "N2"=247.003, "N3"=0.00010055107869386881, "N4"=-1.0343356173776305e-05}, {"N1"=104.579, "N2"=249.502, "N3"=0.00010061132922813323, "N4"=-1.0309294448999744e-05}, {"N1"=104.587, "N2"=251.999, "N3"=0.0001005967230643678, "N4"=-1.0259943217820464e-05}, {"N1"=104.584, "N2"=254.502, "N3"=0.00010059618763392928, "N4"=-1.0203557813365438e-05}, {"N1"=104.575, "N2"=257.003, "N3"=0.00010069534109524803, "N4"=-1.00650799542488e-05}, {"N1"=104.582, "N2"=259.502, "N3"=0.00010062216749369335, "N4"=-1.0286206154315433e-05}, {"N1"=104.578, "N2"=261.997, "N3"=0.00010055427467048132, "N4"=-1.01682315349658e-05}, {"N1"=104.585, "N2"=264.5, "N3"=0.00010060499764449955, "N4"=-1.0212376994969955e-05}, {"N1"=104.581, "N2"=266.999, "N3"=0.00010056776964300815, "N4"=-1.0169744940117539e-05}, {"N1"=102.032, "N2"=266.981, "N3"=0.00010056653876004774, "N4"=-1.0005656853446916e-05}, {"N1"=102.123, "N2"=264.501, "N3"=0.0001005479772534712, "N4"=-1.0210045478967782e-05}, {"N1"=102.138, "N2"=261.996, "N3"=0.00010054316524457154, "N4"=-1.022279666309473e-05}, {"N1"=102.148, "N2"=259.503, "N3"=0.00010060939278726304, "N4"=-1.0275829031642107e-05}, {"N1"=102.131, "N2"=257.001, "N3"=0.00010062272790967308, "N4"=-1.0200579802152772e-05}, {"N1"=102.122, "N2"=254.497, "N3"=0.00010064319617871176, "N4"=-1.0068382095610039e-05}, {"N1"=102.138, "N2"=251.999, "N3"=0.00010061217506869047, "N4"=-1.0307002723702313e-05}, {"N1"=102.141, "N2"=249.5, "N3"=0.00010071195010380847, "N4"=-1.0276849876389942e-05}, {"N1"=102.135, "N2"=246.995, "N3"=0.00010061630714937413, "N4"=-1.0301244591834584e-05}, {"N1"=99.535, "N2"=246.998, "N3"=0.00010074207867602223, "N4"=-1.0164058289737604e-05}, {"N1"=99.64, "N2"=249.496, "N3"=0.00010067858165107633, "N4"=-1.0232213823950155e-05}, {"N1"=99.625, "N2"=252.001, "N3"=0.0001005861420662187, "N4"=-1.0241930059294844e-05}, {"N1"=99.634, "N2"=254.495, "N3"=0.00010067450993103872, "N4"=-1.0348907065918236e-05}, {"N1"=99.634, "N2"=256.996, "N3"=0.00010059000932241389, "N4"=-1.0155161020250288e-05}, {"N1"=99.633, "N2"=259.501, "N3"=0.00010058871610421926, "N4"=-1.0261632218517937e-05}, {"N1"=99.632, "N2"=261.999, "N3"=0.00010046835107141718, "N4"=-1.0375422589986828e-05}, {"N1"=99.648, "N2"=264.498, "N3"=0.00010062894967864391, "N4"=-1.0150927386504143e-05}, {"N1"=99.633, "N2"=267.002, "N3"=0.00010068109872893713, "N4"=-1.0340250589051905e-05}, {"N1"=97.061, "N2"=266.991, "N3"=0.00010053563756110692, "N4"=-1.0330141283540816e-05}, {"N1"=97.182, "N2"=264.506, "N3"=0.0001005654497696182, "N4"=-1.02432923174658e-05}, {"N1"=97.193, "N2"=262.0, "N3"=0.00010061820852984836, "N4"=-1.0172325459328257e-05}, {"N1"=97.181, "N2"=259.503, "N3"=0.00010051677987168872, "N4"=-1.0185037403834221e-05}, {"N1"=97.179, "N2"=257.001, "N3"=0.000100566108073429, "N4"=-1.0339154384265917e-05}, {"N1"=97.182, "N2"=254.498, "N3"=0.00010057451609120394, "N4"=-1.030097164732469e-05}, {"N1"=97.188, "N2"=251.999, "N3"=0.00010072031825096892, "N4"=-1.0145267615871417e-05}, {"N1"=97.19, "N2"=249.503, "N3"=0.00010055512900159086, "N4"=-1.0241241903490255e-05}, {"N1"=97.185, "N2"=246.997, "N3"=0.00010055815013535092, "N4"=-1.011674255794795e-05}, {"N1"=106.899, "N2"=87.002, "N3"=0.00010051232014797229, "N4"=-1.0377055516705508e-05}, {"N1"=106.985, "N2"=84.503, "N3"=0.00010062051772684422, "N4"=-1.026678020041305e-05}, {"N1"=106.991, "N2"=82.005, "N3"=0.00010058190119618773, "N4"=-1.0069256654844627e-05}, {"N1"=106.996, "N2"=79.499, "N3"=0.00010050909244172333, "N4"=-1.0327608953553874e-05}, {"N1"=106.925, "N2"=77.002, "N3"=0.00010060136515168984, "N4"=-1.0304273050686467e-05}, {"N1"=106.927, "N2"=74.494, "N3"=0.0001005933878775541, "N4"=-1.028816506900307e-05}, {"N1"=106.985, "N2"=72.001, "N3"=0.00010055753685108611, "N4"=-1.0104142741629941e-05}, {"N1"=106.988, "N2"=69.5, "N3"=0.00010050731873294315, "N4"=-1.0023490127959328e-05}, {"N1"=106.985, "N2"=67.006, "N3"=0.00010054148034486088, "N4"=-1.0314522300361196e-05}, {"N1"=109.453, "N2"=66.999, "N3"=0.00010063702864250401, "N4"=-1.0408915803091011e-05}, {"N1"=109.461, "N2"=69.503, "N3"=0.0001005508380909665, "N4"=-1.0393626795548991e-05}, {"N1"=109.467, "N2"=72.001, "N3"=0.00010061070020238811, "N4"=-1.0264411477729059e-05}, {"N1"=109.464, "N2"=74.504, "N3"=0.00010052885046383734, "N4"=-1.030771051768036e-05}, {"N1"=109.462, "N2"=77.01, "N3"=0.00010070603852665719, "N4"=-1.0258230058229614e-05}, {"N1"=109.46, "N2"=79.51, "N3"=0.00010063409306854831, "N4"=-1.0092027407681177e-05}, {"N1"=109.452, "N2"=82.013, "N3"=0.00010064518398708693, "N4"=-1.0425961732971865e-05}, {"N1"=109.462, "N2"=84.507, "N3"=0.00010051938811239046, "N4"=-1.0254691772929124e-05}, {"N1"=109.465, "N2"=87.006, "N3"=0.00010055979371262698, "N4"=-1.016026741237997e-05}, {"N1"=111.914, "N2"=86.999, "N3"=0.00010059059158318699, "N4"=-1.024985578146052e-05}, {"N1"=111.897, "N2"=84.503, "N3"=0.00010054098206863079, "N4"=-1.0204970717140697e-05}, {"N1"=111.913, "N2"=82.005, "N3"=0.0001006644102824774, "N4"=-1.0334522690613895e-05}, {"N1"=111.9, "N2"=79.505, "N3"=0.00010058183446719118, "N4"=-1.0661460994799807e-05}, {"N1"=111.908, "N2"=77.006, "N3"=0.00010056065961343714, "N4"=-1.0312807617792926e-05}, {"N1"=111.865, "N2"=74.5, "N3"=0.00010057486137636771, "N4"=-1.0332106730336527e-05}, {"N1"=111.918, "N2"=72.006, "N3"=0.00010063413282944223, "N4"=-1.023802550092837e-05}, {"N1"=111.847, "N2"=69.494, "N3"=0.00010066338055338708, "N4"=-1.026494925312687e-05}, {"N1"=111.889, "N2"=67.01, "N3"=0.00010057062414110136, "N4"=-1.0347584831444238e-05}, {"N1"=114.481, "N2"=67.0, "N3"=0.00010060432582215632, "N4"=-1.038328481737206e-05}, {"N1"=114.484, "N2"=69.5, "N3"=0.00010058418037491044, "N4"=-1.0576970946821335e-05}, {"N1"=114.498, "N2"=72.002, "N3"=0.00010051338853911865, "N4"=-1.0251183496556309e-05}, {"N1"=114.483, "N2"=74.512, "N3"=0.00010061529714991107, "N4"=-1.0268732698940605e-05}, {"N1"=114.481, "N2"=77.01, "N3"=0.00010060882964825721, "N4"=-1.0084270217947536e-05}, {"N1"=114.476, "N2"=79.512, "N3"=0.00010065574312637255, "N4"=-1.0276102608187517e-05}, {"N1"=114.476, "N2"=82.008, "N3"=0.00010067761312384966, "N4"=-1.0344182989985636e-05}, {"N1"=114.48, "N2"=84.501, "N3"=0.00010061739446333418, "N4"=-1.0507945334196473e-05}, {"N1"=114.481, "N2"=87.005, "N3"=0.00010053877928055211, "N4"=-1.0282391722648257e-05}, {"N1"=116.908, "N2"=86.999, "N3"=0.00010057827449808248, "N4"=-1.0224370075910872e-05}, {"N1"=116.976, "N2"=84.499, "N3"=0.00010052400156992185, "N4"=-1.0303307322099827e-05}, {"N1"=116.982, "N2"=82.001, "N3"=0.00010057612637140915, "N4"=-1.0232536840616968e-05}, {"N1"=116.999, "N2"=79.502, "N3"=0.0001005477998578979, "N4"=-1.0337074271430648e-05}, {"N1"=117.002, "N2"=77.001, "N3"=0.00010050179814002798, "N4"=-1.0298560990077212e-05}, {"N1"=116.987, "N2"=74.502, "N3"=0.00010044657750298294, "N4"=-1.0254808215152012e-05}, {"N1"=117.016, "N2"=71.999, "N3"=0.00010055564145096281, "N4"=-1.0132995956915474e-05}, {"N1"=116.966, "N2"=69.499, "N3"=0.00010054121747852851, "N4"=-1.026754805651437e-05}, {"N1"=116.998, "N2"=67.004, "N3"=0.00010055230443864371, "N4"=-1.0209838713278836e-05}, {"N1"=119.416, "N2"=67.005, "N3"=0.00010058210501163632, "N4"=-1.0208565903701327e-05}, {"N1"=119.476, "N2"=69.503, "N3"=0.00010070745238256607, "N4"=-1.0317544410738476e-05}, {"N1"=119.466, "N2"=71.999, "N3"=0.00010065318150793048, "N4"=-1.0397731307394825e-05}, {"N1"=119.462, "N2"=74.51, "N3"=0.00010058380082689938, "N4"=-1.0409883911069292e-05}, {"N1"=119.475, "N2"=77.013, "N3"=0.0001005356520618528, "N4"=-1.0258468376416225e-05}, {"N1"=119.464, "N2"=79.501, "N3"=0.0001006544033857569, "N4"=-1.0394811305075629e-05}, {"N1"=119.457, "N2"=82.015, "N3"=0.00010061058105771496, "N4"=-1.0449084730244491e-05}, {"N1"=119.457, "N2"=84.516, "N3"=0.00010053443223313884, "N4"=-1.0360712606127218e-05}, {"N1"=119.472, "N2"=87.003, "N3"=0.0001006349196342368, "N4"=-1.0344881732530916e-05}, {"N1"=121.925, "N2"=86.999, "N3"=0.00010057046905970515, "N4"=-9.887845932593585e-06}, {"N1"=121.957, "N2"=84.5, "N3"=0.00010051424233160402, "N4"=-1.0298187826706225e-05}, {"N1"=121.962, "N2"=82.004, "N3"=0.00010060815884218694, "N4"=-1.0376569578744985e-05}, {"N1"=121.976, "N2"=79.5, "N3"=0.00010052981794654998, "N4"=-1.0126217080803282e-05}, {"N1"=121.965, "N2"=77.002, "N3"=0.00010050239395843576, "N4"=-1.061327102342567e-05}, {"N1"=121.965, "N2"=74.508, "N3"=0.00010050552790741951, "N4"=-1.0290291997400478e-05}, {"N1"=121.978, "N2"=72.002, "N3"=0.00010060676343976665, "N4"=-1.013120032621056e-05}, {"N1"=121.957, "N2"=69.505, "N3"=0.00010066234071299886, "N4"=-1.0341389130890764e-05}, {"N1"=121.977, "N2"=67.0, "N3"=0.00010070649974879173, "N4"=-1.029419398376751e-05}, {"N1"=124.433, "N2"=66.999, "N3"=0.00010055646175807004, "N4"=-1.0289359062139445e-05}, {"N1"=124.477, "N2"=69.5, "N3"=0.00010049574564853454, "N4"=-1.0392616517396088e-05}, {"N1"=124.486, "N2"=72.017, "N3"=0.00010060734926154591, "N4"=-1.0164743595990427e-05}, {"N1"=124.484, "N2"=74.502, "N3"=0.00010056712319464603, "N4"=-1.0275376365589162e-05}, {"N1"=124.492, "N2"=77.0, "N3"=0.00010063784535170024, "N4"=-1.053049790350161e-05}, {"N1"=124.493, "N2"=79.505, "N3"=0.00010056614822412224, "N4"=-1.0448633075951891e-05}, {"N1"=124.493, "N2"=82.001, "N3"=0.00010049376748875212, "N4"=-1.0537109210555458e-05}, {"N1"=124.494, "N2"=84.517, "N3"=0.00010058817386355465, "N4"=-1.0423900802209011e-05}, {"N1"=124.505, "N2"=87.001, "N3"=0.00010069118738934375, "N4"=-1.0294401246304264e-05}, {"N1"=126.923, "N2"=86.999, "N3"=0.00010059819545767648, "N4"=-1.0297660889143589e-05}, {"N1"=126.968, "N2"=84.502, "N3"=0.00010055359654846057, "N4"=-9.92923698509667e-06}, {"N1"=126.962, "N2"=82.015, "N3"=0.00010064646293383291, "N4"=-1.0477153580188214e-05}, {"N1"=126.965, "N2"=79.508, "N3"=0.0001005633145791528, "N4"=-1.0419793504128884e-05}, {"N1"=126.968, "N2"=77.004, "N3"=0.00010063989447547184, "N4"=-1.039755702821742e-05}, {"N1"=126.974, "N2"=74.5, "N3"=0.00010058338746739966, "N4"=-1.0291713776693597e-05}, {"N1"=126.972, "N2"=71.999, "N3"=0.00010062210140792953, "N4"=-1.0212388409676702e-05}, {"N1"=126.937, "N2"=69.499, "N3"=0.00010063565718873436, "N4"=-1.0198729717050587e-05}, {"N1"=126.951, "N2"=67.003, "N3"=0.00010062827514799282, "N4"=-1.0496410146082091e-05}, {"N1"=207.042, "N2"=67.002, "N3"=0.00010055134084037263, "N4"=-1.0336606421981276e-05}, {"N1"=207.1, "N2"=69.522, "N3"=0.00010064567104762942, "N4"=-1.0321482612276694e-05}, {"N1"=207.1, "N2"=72.002, "N3"=0.00010052408250711327, "N4"=-1.0288909953065614e-05}, {"N1"=207.069, "N2"=74.501, "N3"=0.00010049323784101942, "N4"=-1.0287565433305119e-05}, {"N1"=207.101, "N2"=77.001, "N3"=0.00010062739930357217, "N4"=-1.0281779277293586e-05}, {"N1"=207.108, "N2"=79.532, "N3"=0.00010062378558442375, "N4"=-1.025636291772424e-05}, {"N1"=207.106, "N2"=82.0, "N3"=0.00010055475074769214, "N4"=-1.0307797209499544e-05}, {"N1"=207.104, "N2"=84.506, "N3"=0.0001005312191416613, "N4"=-1.0307770153731927e-05}, {"N1"=207.09, "N2"=87.007, "N3"=0.00010060104993681344, "N4"=-1.0324308090709687e-05}, {"N1"=209.462, "N2"=87.003, "N3"=0.00010069775464636404, "N4"=-1.0086419844648227e-05}, {"N1"=209.518, "N2"=84.506, "N3"=0.00010055215018121781, "N4"=-1.0329264656842698e-05}, {"N1"=209.522, "N2"=82.002, "N3"=0.00010068030959579917, "N4"=-9.944307224290469e-06}, {"N1"=209.51, "N2"=79.5, "N3"=0.00010067619093958527, "N4"=-1.0165977122320352e-05}, {"N1"=209.533, "N2"=76.997, "N3"=0.0001005973603616755, "N4"=-1.0336309131755114e-05}, {"N1"=209.507, "N2"=74.5, "N3"=0.00010051616108954655, "N4"=-1.0374566254615045e-05}, {"N1"=209.533, "N2"=72.005, "N3"=0.00010059130383165952, "N4"=-1.0560698842937328e-05}, {"N1"=209.448, "N2"=69.497, "N3"=0.00010056711114762238, "N4"=-1.0335861372614563e-05}, {"N1"=209.526, "N2"=67.0, "N3"=0.00010067872941124583, "N4"=-1.0294738162322259e-05}, {"N1"=211.919, "N2"=67.0, "N3"=0.00010063254320753911, "N4"=-1.0178060217653594e-05}, {"N1"=212.008, "N2"=69.502, "N3"=0.00010060512642423166, "N4"=-1.0405640474738863e-05}, {"N1"=212.023, "N2"=72.007, "N3"=0.0001005704649155309, "N4"=-1.0239978758249574e-05}, {"N1"=212.013, "N2"=74.498, "N3"=0.00010050423573558398, "N4"=-1.0459207245018824e-05}, {"N1"=212.032, "N2"=77.009, "N3"=0.00010057018335624141, "N4"=-1.0264420590141643e-05}, {"N1"=212.015, "N2"=79.501, "N3"=0.00010056393444607281, "N4"=-1.037975011332122e-05}, {"N1"=212.026, "N2"=82.007, "N3"=0.00010057506011984283, "N4"=-1.0099858841456314e-05}, {"N1"=212.037, "N2"=84.51, "N3"=0.00010045298913882377, "N4"=-1.0351015735173768e-05}, {"N1"=212.045, "N2"=87.012, "N3"=0.00010066040848817733, "N4"=-1.0353248320359791e-05}, {"N1"=214.434, "N2"=86.999, "N3"=0.0001005749656276479, "N4"=-1.0328820332756019e-05}, {"N1"=214.5, "N2"=84.508, "N3"=0.00010056077507496633, "N4"=-1.0223957632679518e-05}, {"N1"=214.501, "N2"=82.008, "N3"=0.00010047583098045784, "N4"=-1.0200884174155184e-05}, {"N1"=214.504, "N2"=79.503, "N3"=0.00010049711460021243, "N4"=-1.0337430862803363e-05}, {"N1"=214.495, "N2"=77.003, "N3"=0.00010057243444076018, "N4"=-1.0329958505929577e-05}, {"N1"=214.511, "N2"=74.501, "N3"=0.00010063891794493008, "N4"=-1.0202041074101114e-05}, {"N1"=214.502, "N2"=72.003, "N3"=0.0001005530455498703, "N4"=-1.0341748240194267e-05}, {"N1"=214.503, "N2"=69.508, "N3"=0.00010066517350864406, "N4"=-1.0273029489592905e-05}, {"N1"=214.504, "N2"=67.002, "N3"=0.00010057443898676322, "N4"=-1.0643357917712385e-05}, {"N1"=216.967, "N2"=66.999, "N3"=0.00010063503590142273, "N4"=-1.0350148420913918e-05}, {"N1"=217.011, "N2"=69.507, "N3"=0.00010060395650817198, "N4"=-1.0192467632278532e-05}, {"N1"=217.012, "N2"=72.003, "N3"=0.00010063921896594177, "N4"=-1.0459009638346552e-05}, {"N1"=217.018, "N2"=74.501, "N3"=0.00010062647418294577, "N4"=-1.0396801214236604e-05}, {"N1"=217.009, "N2"=77.008, "N3"=0.00010061292593577963, "N4"=-1.0273306205176266e-05}, {"N1"=217.017, "N2"=79.504, "N3"=0.00010057053112326033, "N4"=-1.023907513471943e-05}, {"N1"=217.018, "N2"=82.013, "N3"=0.00010060922621905568, "N4"=-1.0355649919727279e-05}, {"N1"=217.016, "N2"=84.508, "N3"=0.00010063763175127578, "N4"=-1.0320110795820426e-05}, {"N1"=217.017, "N2"=87.005, "N3"=0.00010064376690502326, "N4"=-1.0371145084833707e-05}, {"N1"=219.437, "N2"=86.998, "N3"=0.00010053356811331625, "N4"=-1.0101335913634599e-05}, {"N1"=219.474, "N2"=84.502, "N3"=0.00010056783687108572, "N4"=-9.85461928442005e-06}, {"N1"=219.496, "N2"=82.007, "N3"=0.00010076054684920304, "N4"=-1.041533236610626e-05}, {"N1"=219.495, "N2"=79.5, "N3"=0.00010064067871542483, "N4"=-1.0283468873670739e-05}, {"N1"=219.499, "N2"=77.007, "N3"=0.00010055518756997739, "N4"=-1.0487565314261106e-05}, {"N1"=219.44, "N2"=74.498, "N3"=0.00010060825206396356, "N4"=-9.798345280146752e-06}, {"N1"=219.492, "N2"=72.006, "N3"=0.00010061686304847366, "N4"=-1.0199562920874177e-05}, {"N1"=219.411, "N2"=69.503, "N3"=0.00010052705861113211, "N4"=-1.0320712522216568e-05}, {"N1"=219.452, "N2"=67.001, "N3"=0.00010059063299615535, "N4"=-1.0528870102917256e-05}, {"N1"=221.944, "N2"=67.002, "N3"=0.00010058232096693351, "N4"=-1.0337516928155011e-05}, {"N1"=222.004, "N2"=69.507, "N3"=0.0001005029545057057, "N4"=-1.0281677057906925e-05}, {"N1"=221.982, "N2"=72.001, "N3"=0.00010056880005246238, "N4"=-1.022349276107091e-05}, {"N1"=221.982, "N2"=74.5, "N3"=0.00010065576349024778, "N4"=-1.024657827373725e-05}, {"N1"=221.994, "N2"=77.01, "N3"=0.0001005382392973918, "N4"=-1.0118001210578003e-05}, {"N1"=221.991, "N2"=79.503, "N3"=0.00010060175559570843, "N4"=-1.0338449905549244e-05}, {"N1"=221.992, "N2"=82.01, "N3"=0.00010061425069748994, "N4"=-1.0209582913130938e-05}, {"N1"=221.992, "N2"=84.512, "N3"=0.0001004958723581159, "N4"=-1.0385854378216263e-05}, {"N1"=221.981, "N2"=87.012, "N3"=0.00010056445414379728, "N4"=-1.0293850841150737e-05}, {"N1"=224.433, "N2"=86.995, "N3"=0.0001005816076169972, "N4"=-1.028840795065175e-05}, {"N1"=224.485, "N2"=84.504, "N3"=0.00010060297611600566, "N4"=-1.0314747785514537e-05}, {"N1"=224.494, "N2"=82.005, "N3"=0.00010057948908679308, "N4"=-1.0236719489084794e-05}, {"N1"=224.492, "N2"=79.505, "N3"=0.00010059795766299457, "N4"=-1.0320018966860413e-05}, {"N1"=224.482, "N2"=77.003, "N3"=0.00010058471434349656, "N4"=-1.011573201835033e-05}, {"N1"=224.397, "N2"=74.496, "N3"=0.00010053043572196017, "N4"=-1.0286351967551368e-05}, {"N1"=224.476, "N2"=71.995, "N3"=0.0001005809230669314, "N4"=-1.0205360875853817e-05}, {"N1"=224.399, "N2"=69.501, "N3"=0.00010061366290280907, "N4"=-1.0211959723604356e-05}, {"N1"=224.489, "N2"=67.0, "N3"=0.00010060064416751453, "N4"=-1.032502564169628e-05}, {"N1"=226.952, "N2"=67.002, "N3"=0.0001006369430978361, "N4"=-1.0434700733044642e-05}, {"N1"=227.0, "N2"=69.509, "N3"=0.00010055519196641069, "N4"=-1.0253245845202816e-05}, {"N1"=227.005, "N2"=72.006, "N3"=0.00010058188539322229, "N4"=-1.0270007374481483e-05}, {"N1"=226.988, "N2"=74.503, "N3"=0.0001005948368945051, "N4"=-1.022371784229762e-05}, {"N1"=226.996, "N2"=77.002, "N3"=0.00010060978507668937, "N4"=-1.0195183358056406e-05}, {"N1"=226.987, "N2"=79.512, "N3"=0.00010061598903874942, "N4"=-1.0264905128426394e-05}, {"N1"=226.963, "N2"=82.004, "N3"=0.00010055580534048747, "N4"=-1.029195030620679e-05}, {"N1"=226.988, "N2"=84.523, "N3"=0.000100596142124528, "N4"=-1.0174363225797958e-05}, {"N1"=226.988, "N2"=87.013, "N3"=0.00010043980805613111, "N4"=-1.0213544268527403e-05}, {"N1"=226.946, "N2"=246.984, "N3"=0.00010065028979043666, "N4"=-1.0524218965807193e-05}, {"N1"=226.954, "N2"=249.501, "N3"=0.00010054707759626902, "N4"=-1.0279495344808947e-05}, {"N1"=226.968, "N2"=252.004, "N3"=0.00010057676999776135, "N4"=-1.0068376867805955e-05}, {"N1"=226.954, "N2"=254.492, "N3"=0.00010062391197440939, "N4"=-1.0450439112825726e-05}, {"N1"=226.974, "N2"=256.996, "N3"=0.00010066220270651209, "N4"=-1.001070728074639e-05}, {"N1"=226.962, "N2"=259.496, "N3"=0.00010056508387492809, "N4"=-1.0304069840120842e-05}, {"N1"=226.977, "N2"=262.0, "N3"=0.00010069697954400125, "N4"=-1.0231554804281007e-05}, {"N1"=226.961, "N2"=264.499, "N3"=0.00010050983234318854, "N4"=-1.0307029124288474e-05}, {"N1"=226.978, "N2"=266.998, "N3"=0.00010071095322854614, "N4"=-1.0266647273029206e-05}, {"N1"=224.646, "N2"=267.0, "N3"=0.00010050457785449692, "N4"=-1.0340684570211349e-05}, {"N1"=224.603, "N2"=264.5, "N3"=0.0001005474726825836, "N4"=-1.0438531318564597e-05}, {"N1"=224.655, "N2"=261.997, "N3"=0.00010063087053718227, "N4"=-1.022375466434457e-05}, {"N1"=224.648, "N2"=259.503, "N3"=0.00010062577194548791, "N4"=-1.0305877796317359e-05}, {"N1"=224.65, "N2"=256.999, "N3"=0.00010053527058305886, "N4"=-1.0216369466455645e-05}, {"N1"=224.647, "N2"=254.489, "N3"=0.00010054499763095839, "N4"=-1.0216092318993868e-05}, {"N1"=224.658, "N2"=252.006, "N3"=0.00010065122637341251, "N4"=-1.002469019169797e-05}, {"N1"=224.65, "N2"=249.5, "N3"=0.00010050236044512719, "N4"=-1.0369252068034365e-05}, {"N1"=224.657, "N2"=246.999, "N3"=0.00010050517258815378, "N4"=-1.028968885628919e-05}, {"N1"=222.076, "N2"=247.002, "N3"=0.00010055528984982321, "N4"=-1.0293566813158102e-05}, {"N1"=222.145, "N2"=249.501, "N3"=0.00010065751494962773, "N4"=-1.039591007406633e-05}, {"N1"=222.143, "N2"=252.001, "N3"=0.00010087404967555311, "N4"=-1.0479169728932771e-05}, {"N1"=222.141, "N2"=254.504, "N3"=0.00010054379319839901, "N4"=-1.0122418572329379e-05}, {"N1"=222.154, "N2"=257.0, "N3"=0.00010068304744474788, "N4"=-1.0248764126123949e-05}, {"N1"=222.129, "N2"=259.502, "N3"=0.00010062094981913318, "N4"=-1.0324562528066859e-05}, {"N1"=222.155, "N2"=262.001, "N3"=0.00010070026392851403, "N4"=-1.0388724728921369e-05}, {"N1"=222.128, "N2"=264.496, "N3"=0.00010055382574124339, "N4"=-1.0302629634203676e-05}, {"N1"=222.143, "N2"=266.997, "N3"=0.00010058672751501809, "N4"=-1.0193593568924285e-05}, {"N1"=219.562, "N2"=266.997, "N3"=0.00010055065591194332, "N4"=-1.0384805416417194e-05}, {"N1"=219.642, "N2"=264.498, "N3"=0.00010065416304775239, "N4"=-1.0303176440523526e-05}, {"N1"=219.671, "N2"=261.997, "N3"=0.00010064148542206741, "N4"=-1.0243353890842768e-05}, {"N1"=219.67, "N2"=259.483, "N3"=0.00010064921190908889, "N4"=-1.0298357086791502e-05}, {"N1"=219.658, "N2"=256.996, "N3"=0.00010064584538987735, "N4"=-1.0248405227535391e-05}, {"N1"=219.646, "N2"=254.489, "N3"=0.00010058177372200028, "N4"=-1.0367288358884665e-05}, {"N1"=219.675, "N2"=252.0, "N3"=0.0001005162952669433, "N4"=-1.0392927171577334e-05}, {"N1"=219.678, "N2"=249.502, "N3"=0.00010056596040855672, "N4"=-1.0214793342487479e-05}, {"N1"=219.657, "N2"=246.999, "N3"=0.00010063573902690341, "N4"=-1.0307535309443987e-05}, {"N1"=217.08, "N2"=246.994, "N3"=0.0001006519423977907, "N4"=-1.0244494004664458e-05}, {"N1"=217.118, "N2"=249.498, "N3"=0.00010052429261857621, "N4"=-1.044948868925336e-05}, {"N1"=217.09, "N2"=251.991, "N3"=0.00010054472889102999, "N4"=-1.0293214524590472e-05}, {"N1"=217.127, "N2"=254.491, "N3"=0.00010046907336576803, "N4"=-1.0262527406719686e-05}, {"N1"=217.135, "N2"=257.001, "N3"=0.00010055567032088702, "N4"=-1.0299213691257778e-05}, {"N1"=217.135, "N2"=259.5, "N3"=0.0001006412801632793, "N4"=-1.0320962008452717e-05}, {"N1"=217.131, "N2"=261.993, "N3"=0.00010058850557553264, "N4"=-1.0263127112156919e-05}, {"N1"=217.137, "N2"=264.502, "N3"=0.00010062564012700985, "N4"=-1.0341147236524869e-05}, {"N1"=217.134, "N2"=266.999, "N3"=0.00010049686827522053, "N4"=-1.0355472898834788e-05}, {"N1"=214.604, "N2"=266.992, "N3"=0.00010050777009712029, "N4"=-1.0232952771274728e-05}, {"N1"=214.648, "N2"=264.494, "N3"=0.00010056247902914494, "N4"=-1.027321321664182e-05}, {"N1"=214.639, "N2"=262.0, "N3"=0.00010057710668784902, "N4"=-1.0344371694022798e-05}, {"N1"=214.649, "N2"=259.509, "N3"=0.00010070346805508621, "N4"=-1.030882971542685e-05}, {"N1"=214.642, "N2"=256.998, "N3"=0.00010057950008854065, "N4"=-1.0364018664301022e-05}, {"N1"=214.642, "N2"=254.501, "N3"=0.00010055905573912868, "N4"=-1.038834090407824e-05}, {"N1"=214.632, "N2"=251.995, "N3"=0.00010057225961402201, "N4"=-1.0288331190990525e-05}, {"N1"=214.628, "N2"=249.496, "N3"=0.00010049942947412219, "N4"=-1.0427345000905543e-05}, {"N1"=214.659, "N2"=247.001, "N3"=0.00010065106316976622, "N4"=-1.0318865915162873e-05}, {"N1"=212.086, "N2"=247.0, "N3"=0.00010054049961126128, "N4"=-1.0286076889062284e-05}, {"N1"=212.15, "N2"=249.502, "N3"=0.00010055664807715495, "N4"=-1.0329449828192031e-05}, {"N1"=212.132, "N2"=252.006, "N3"=0.00010068188324601617, "N4"=-1.0380262405387706e-05}, {"N1"=212.145, "N2"=254.5, "N3"=0.00010067511509381524, "N4"=-1.0239109244426103e-05}, {"N1"=212.147, "N2"=257.001, "N3"=0.00010050925701224387, "N4"=-1.0350640304870126e-05}, {"N1"=212.13, "N2"=259.5, "N3"=0.00010062024783254645, "N4"=-1.0460309212821724e-05}, {"N1"=212.136, "N2"=261.996, "N3"=0.00010053214611414518, "N4"=-1.0300092739042196e-05}, {"N1"=212.157, "N2"=264.499, "N3"=0.00010065593202383329, "N4"=-1.0283110963462803e-05}, {"N1"=212.097, "N2"=266.992, "N3"=0.00010062898407260945, "N4"=-1.0178713352019605e-05}, {"N1"=209.573, "N2"=266.992, "N3"=0.00010064654557543395, "N4"=-1.0294731763197119e-05}, {"N1"=209.619, "N2"=264.497, "N3"=0.00010055003234705244, "N4"=-1.0322604883162464e-05}, {"N1"=209.652, "N2"=262.001, "N3"=0.00010056986370545585, "N4"=-1.0240927369688976e-05}, {"N1"=209.651, "N2"=259.501, "N3"=0.0001005504437778276, "N4"=-1.0402929454698797e-05}, {"N1"=209.652, "N2"=257.0, "N3"=0.0001006138653332042, "N4"=-1.028624945684621e-05}, {"N1"=209.655, "N2"=254.499, "N3"=0.00010046996744364618, "N4"=-1.0313156230400227e-05}, {"N1"=209.649, "N2"=251.997, "N3"=0.00010054668336265244, "N4"=-1.0312496809101996e-05}, {"N1"=209.586, "N2"=249.499, "N3"=0.00010054299511352194, "N4"=-1.0324341755023403e-05}, {"N1"=209.552, "N2"=246.997, "N3"=0.00010065642656394289, "N4"=-1.0344524564077034e-05}, {"N1"=207.065, "N2"=246.995, "N3"=0.00010061474200014649, "N4"=-1.026526560635324e-05}, {"N1"=207.122, "N2"=249.498, "N3"=0.0001006320834273451, "N4"=-1.0253729084075166e-05}, {"N1"=207.087, "N2"=251.993, "N3"=0.00010063813434864981, "N4"=-1.0357138412593596e-05}, {"N1"=207.132, "N2"=254.497, "N3"=0.00010058197699204032, "N4"=-1.0304586208417301e-05}, {"N1"=207.16, "N2"=257.0, "N3"=0.00010053317938152688, "N4"=-1.0375609656199857e-05}, {"N1"=207.145, "N2"=259.494, "N3"=0.00010055177823206895, "N4"=-1.0332606535258964e-05}, {"N1"=207.148, "N2"=261.992, "N3"=0.00010046975179085102, "N4"=-1.0589160707666948e-05}, {"N1"=207.143, "N2"=264.498, "N3"=0.00010066896914636279, "N4"=-1.0126388520934882e-05}, {"N1"=207.142, "N2"=266.994, "N3"=0.0001005366357673231, "N4"=-1.0343369053099564e-05}, {"N1"=204.567, "N2"=266.991, "N3"=0.00010056819361984244, "N4"=-1.034038074059891e-05}, {"N1"=204.651, "N2"=264.497, "N3"=0.00010058791833409883, "N4"=-1.03958683504339e-05}, {"N1"=204.647, "N2"=261.99, "N3"=0.00010063069567520518, "N4"=-1.045100292345777e-05}, {"N1"=204.658, "N2"=259.5, "N3"=0.00010050062024984678, "N4"=-1.028468952638022e-05}, {"N1"=204.657, "N2"=257.001, "N3"=0.0001004569222815056, "N4"=-1.043841276237354e-05}, {"N1"=204.641, "N2"=254.493, "N3"=0.00010059801536685324, "N4"=-1.043692988036486e-05}, {"N1"=204.655, "N2"=251.998, "N3"=0.00010061788153362552, "N4"=-1.028116894085906e-05}, {"N1"=204.655, "N2"=249.497, "N3"=0.0001006018366530668, "N4"=-1.0328988335053345e-05}, {"N1"=204.647, "N2"=247.001, "N3"=0.00010055567358477742, "N4"=-1.0089372323895255e-05}, {"N1"=204.633, "N2"=244.493, "N3"=0.00010060475292725768, "N4"=-1.0413726220071594e-05}, {"N1"=204.643, "N2"=241.998, "N3"=0.00010055966477656639, "N4"=-1.0294039236046854e-05}, {"N1"=204.658, "N2"=239.504, "N3"=0.00010057380197396022, "N4"=-1.0368794865746204e-05}, {"N1"=204.652, "N2"=237.006, "N3"=0.00010059943683444395, "N4"=-1.0348488891308487e-05}, {"N1"=204.634, "N2"=234.499, "N3"=0.00010051962445727131, "N4"=-1.0255613989018652e-05}, {"N1"=204.654, "N2"=232.005, "N3"=0.00010064654139410443, "N4"=-1.0407856603434554e-05}, {"N1"=204.634, "N2"=229.495, "N3"=0.00010061877160741786, "N4"=-1.0414503843173611e-05}, {"N1"=204.648, "N2"=226.999, "N3"=0.00010063940826907325, "N4"=-1.0502576509856837e-05}, {"N1"=202.12, "N2"=226.998, "N3"=0.00010065084158035409, "N4"=-1.0384142727275308e-05}, {"N1"=202.143, "N2"=229.496, "N3"=0.00010052468354935875, "N4"=-1.037555489721163e-05}, {"N1"=202.178, "N2"=232.003, "N3"=0.00010062651337841424, "N4"=-1.0337467874748784e-05}, {"N1"=202.089, "N2"=234.494, "N3"=0.00010055146531321666, "N4"=-1.0333255492364494e-05}, {"N1"=202.174, "N2"=237.007, "N3"=0.00010048229927035179, "N4"=-1.0367260868813217e-05}, {"N1"=202.147, "N2"=239.5, "N3"=0.00010052144920660789, "N4"=-1.0371982627652875e-05}, {"N1"=202.172, "N2"=242.003, "N3"=0.00010044908148018206, "N4"=-1.0369463830642187e-05}, {"N1"=202.175, "N2"=244.507, "N3"=0.00010057324780294678, "N4"=-1.0356085541384798e-05}, {"N1"=202.177, "N2"=247.006, "N3"=0.00010056235551274627, "N4"=-1.041490512632681e-05}, {"N1"=202.181, "N2"=249.499, "N3"=0.0001005986749408007, "N4"=-1.0375101466652622e-05}, {"N1"=202.183, "N2"=252.004, "N3"=0.00010054535675531857, "N4"=-1.0426135162518159e-05}, {"N1"=202.189, "N2"=254.502, "N3"=0.00010056395335992274, "N4"=-1.022053001570241e-05}, {"N1"=202.184, "N2"=256.998, "N3"=0.00010051135627041871, "N4"=-1.0534495531103145e-05}, {"N1"=202.161, "N2"=259.501, "N3"=0.00010052094057371137, "N4"=-1.0220741655860598e-05}, {"N1"=202.183, "N2"=262.0, "N3"=0.00010056983877949575, "N4"=-1.0323469057834248e-05}, {"N1"=202.171, "N2"=264.5, "N3"=0.00010061920277874033, "N4"=-1.0160517711631817e-05}, {"N1"=202.166, "N2"=267.004, "N3"=0.00010055394716068769, "N4"=-1.034826452864095e-05}, {"N1"=199.599, "N2"=267.001, "N3"=0.0001004984068318151, "N4"=-1.0355207679255114e-05}, {"N1"=199.688, "N2"=264.499, "N3"=0.00010058822441022313, "N4"=-1.0393990904503394e-05}, {"N1"=199.664, "N2"=261.999, "N3"=0.00010054495214425437, "N4"=-1.0430965621690782e-05}, {"N1"=199.683, "N2"=259.497, "N3"=0.00010056869228687324, "N4"=-1.042115906440467e-05}, {"N1"=199.698, "N2"=256.997, "N3"=0.00010068554207419468, "N4"=-1.0276364880276094e-05}, {"N1"=199.701, "N2"=254.5, "N3"=0.0001006656545955483, "N4"=-1.0244843535228412e-05}, {"N1"=199.703, "N2"=251.995, "N3"=0.00010058137307239781, "N4"=-1.0215198185166196e-05}, {"N1"=199.7, "N2"=249.499, "N3"=0.00010058277454350435, "N4"=-1.0388555097153994e-05}, {"N1"=199.71, "N2"=247.005, "N3"=0.00010059300174373218, "N4"=-1.0428194206591165e-05}, {"N1"=199.692, "N2"=244.501, "N3"=0.00010048968108562608, "N4"=-1.0179454690517312e-05}, {"N1"=199.71, "N2"=242.0, "N3"=0.00010062190585988557, "N4"=-1.029922406447521e-05}, {"N1"=199.689, "N2"=239.49, "N3"=0.00010067880509803468, "N4"=-1.0452287054338239e-05}, {"N1"=199.713, "N2"=237.002, "N3"=0.00010059565313729888, "N4"=-1.0443432417400948e-05}, {"N1"=199.684, "N2"=234.497, "N3"=0.0001004951835917124, "N4"=-1.0455457996890791e-05}, {"N1"=199.714, "N2"=231.997, "N3"=0.00010058751764206648, "N4"=-1.0335579348895757e-05}, {"N1"=199.691, "N2"=229.494, "N3"=0.00010055073671458257, "N4"=-1.030190877503535e-05}, {"N1"=199.706, "N2"=227.005, "N3"=0.0001005269979903724, "N4"=-1.0199386225306044e-05}, {"N1"=197.088, "N2"=227.003, "N3"=0.00010058039264333282, "N4"=-1.036145620744824e-05}, {"N1"=197.15, "N2"=229.494, "N3"=0.00010060734953341666, "N4"=-1.0389305159456381e-05}, {"N1"=197.167, "N2"=231.997, "N3"=0.00010053258915126612, "N4"=-1.0403603809352756e-05}, {"N1"=197.19, "N2"=234.499, "N3"=0.0001005373448805349, "N4"=-1.0422960437339374e-05}, {"N1"=197.188, "N2"=237.002, "N3"=0.00010062544743953492, "N4"=-1.0346218352914987e-05}, {"N1"=197.191, "N2"=239.506, "N3"=0.00010054722920408948, "N4"=-1.0391865405273892e-05}, {"N1"=197.187, "N2"=242.001, "N3"=0.00010053461534679626, "N4"=-1.0366294798750603e-05}, {"N1"=197.175, "N2"=244.499, "N3"=0.00010064128544243675, "N4"=-1.0360826079586181e-05}, {"N1"=197.192, "N2"=247.001, "N3"=0.00010050386189416498, "N4"=-1.0317480094327238e-05}, {"N1"=197.192, "N2"=249.501, "N3"=0.0001006390558747505, "N4"=-1.0522939326788905e-05}, {"N1"=197.192, "N2"=252.006, "N3"=0.00010059339186007532, "N4"=-1.0539960118926326e-05}, {"N1"=197.195, "N2"=254.5, "N3"=0.00010054381036945614, "N4"=-1.0399212255939307e-05}, {"N1"=197.185, "N2"=256.993, "N3"=0.00010070258473786659, "N4"=-1.0465100146734042e-05}, {"N1"=197.2, "N2"=259.499, "N3"=0.00010061875350504074, "N4"=-1.0403891131413874e-05}, {"N1"=197.199, "N2"=261.999, "N3"=0.00010062055171801072, "N4"=-1.0523232852988175e-05}, {"N1"=197.135, "N2"=264.498, "N3"=0.00010064429973864377, "N4"=-1.0338894843905645e-05}, {"N1"=197.134, "N2"=267.001, "N3"=0.00010054916701282032, "N4"=-1.0311588908985012e-05}, {"N1"=194.618, "N2"=267.0, "N3"=0.00010063286694134301, "N4"=-1.0360505167120463e-05}, {"N1"=194.669, "N2"=264.5, "N3"=0.00010049887277404996, "N4"=-1.0321612883766946e-05}, {"N1"=194.684, "N2"=261.992, "N3"=0.00010054609342202796, "N4"=-1.0295398524572918e-05}, {"N1"=194.694, "N2"=259.5, "N3"=0.00010069525021473443, "N4"=-1.0410170955307722e-05}, {"N1"=194.696, "N2"=257.0, "N3"=0.00010065921861748322, "N4"=-1.0321319475309524e-05}, {"N1"=194.672, "N2"=254.494, "N3"=0.00010054052875458746, "N4"=-1.0346417963539715e-05}, {"N1"=194.676, "N2"=251.993, "N3"=0.0001005496400511357, "N4"=-1.0306725786402999e-05}, {"N1"=194.684, "N2"=249.499, "N3"=0.00010058916411243086, "N4"=-1.0529058408906472e-05}, {"N1"=194.673, "N2"=246.999, "N3"=0.00010055043609310792, "N4"=-1.035168382107408e-05}, {"N1"=194.667, "N2"=244.498, "N3"=0.00010059283401479894, "N4"=-1.041185424721329e-05}, {"N1"=194.685, "N2"=242.0, "N3"=0.00010052507110401954, "N4"=-1.0286734617607643e-05}, {"N1"=194.686, "N2"=239.498, "N3"=0.00010058771274752203, "N4"=-1.0314282892817485e-05}, {"N1"=194.67, "N2"=236.996, "N3"=0.00010050751942618397, "N4"=-1.0458209910152601e-05}, {"N1"=194.694, "N2"=234.499, "N3"=0.00010061709929022871, "N4"=-1.0682819439424653e-05}, {"N1"=194.7, "N2"=232.002, "N3"=0.00010061027731715424, "N4"=-1.0262620665692884e-05}, {"N1"=194.703, "N2"=229.499, "N3"=0.00010055155033956318, "N4"=-1.0340758705362404e-05}, {"N1"=194.688, "N2"=227.003, "N3"=0.00010057294219296372, "N4"=-1.0459044745138397e-05}], 1 "peak diff":T3(graph), 3 "Intensity Graph 12":dbl[][](graph))   [LabVIEW 2016]
uses:
  <vilib>/Analysis/3filter.llb/Filter Passband Type.ctl
  <userlib>/_MGI/File/Spreadsheet/MGI Write Spreadsheet Behavior Enum.ctl
  <vilib>/Analysis/3filter.llb/Chebyshev Filter (DBL).vi
  <vilib>/Analysis/NI_AAL_SigProc.lvlib
  <vilib>/Analysis/NI_AALPro.lvlib
  <vilib>/Analysis/NI_AALBase.lvlib
panel:
  in  "Folder Path":path
  in  "Enum":enum16{"X channel", "R"}(ring)
  out "appended array":dbl[][](array[numeric]) format="%#_4f"
  in  "Existing SS file":string="P:\\expt\\Leiden MNK\\SA02836H.20170110\\processed\\9_rounded.txt\nP:\\expt\\Leiden MNK\\SA02836H.20170110\\processed\\29 -rounded -20-50-40 -cropped.txt"
  in  "display graphs?":bool
  in  "Path":path=path "P:/expt/Leiden MNK/SA02836H.20170110/processed/9-11-14-17-19A-25-38-40-41-42-43-44-45-46-47-48 _rounded _20-50-40.txt"
  in  "write SS file?":bool
  in  "Tab Control":T2(tab)=enum."offset trans"
  in  "X axis":enum16{"B field", "theta", "phi"}(ring)
  out "Conductance":T3(graph)
  out "Intensity Graph 14":dbl[][](graph)
  out "angle theta":dbl[](array[numeric])=[2.1586725667033604e-05, 2.166714453280228e-05, 2.1745841280251943e-05, 2.1845808000424864e-05, 2.1930376360427983e-05, 2.1986580115768095e-05, 2.2058581152794458e-05, 2.2169084813773176e-05, 2.226657284126091e-05, 2.232597418953461e-05, 2.2430025558967086e-05, 2.2527763368583487e-05, 2.25972640821974e-05, 2.2702052716424986e-05, 2.2779912537047018e-05, 2.287296915606435e-05, 2.2960249778940445e-05, 2.3064369716876124e-05, 2.316056164837207e-05, 2.3244454458392494e-05, 2.3330102450026187e-05, 2.343313269495234e-05, 2.3523126612641586e-05, 2.3587702173534296e-05, 2.3704166132988858e-05, 2.3820301849636444e-05, 2.3913594772870135e-05, 2.4006746686431012e-05, 2.4093719060623474e-05, 2.4204396320250717e-05, 2.4320818860749184e-05, 2.4436987110049107e-05, 2.4522337570307038e-05, 2.4594539961641787e-05, 2.4720889826243038e-05, 2.481912484042889e-05, 2.4963972112450366e-05, 2.5055789005704938e-05, 2.518134437246013e-05, 2.52774396612965e-05, 2.540503296480945e-05, 2.5493011555245535e-05, 2.5601969066736257e-05, 2.5734147565647586e-05, 2.5844983235778035e-05, 2.5944884448331357e-05, 2.6099811654937253e-05, 2.6170216831749064e-05, 2.6293666621982503e-05, 2.6418051573325204e-05, 2.652102878421431e-05, 2.6701879720213767e-05, 2.6826528122213533e-05, 2.6921932086733258e-05, 2.7039026835256134e-05, 2.710180749514938e-05, 2.7285616394363204e-05, 2.742131917216564e-05, 2.7563531036133056e-05, 2.767752734635836e-05, 2.7852190719296286e-05, 2.793196549356615e-05, 2.810241030173358e-05, 2.8264651714293143e-05, 2.838733650282356e-05, 2.8516876992728783e-05, 2.8678089393625934e-05, 2.8781157569574797e-05, 2.892141303885143e-05, 2.90732931946417e-05, 2.924776113389817e-05, 2.9403605149310246e-05, 2.9530187705877717e-05, 2.9705745282544423e-05, 2.9831346397046727e-05, 3.004597728494249e-05, 3.0144247421604172e-05, 3.033885201618883e-05, 3.0466054033098528e-05, 3.062144873343885e-05, 3.080024887331192e-05, 3.100117617090868e-05, 3.114100918946798e-05, 3.135058479425823e-05, 3.1432395437850074e-05, 3.163669182943396e-05, 3.181409082803682e-05, 3.2030328515635e-05, 3.2206990086513415e-05, 3.2396504593365734e-05, 3.255132838897057e-05, 3.277629931557485e-05, 3.291646710755952e-05, 3.306488491009579e-05, 3.327422279132814e-05, 3.3465200335918826e-05, 3.366350451851328e-05, 3.387045794131546e-05, 3.4081673189905494e-05, 3.428118155267909e-05, 3.444796782085588e-05, 3.468013527532616e-05, 3.4932179004275626e-05, 3.505437847759629e-05, 3.532996583090013e-05, 3.5529734372586415e-05, 3.5776723879736085e-05, 3.598721282141628e-05, 3.620417402698634e-05, 3.646091819815044e-05, 3.675907628388842e-05, 3.6907348266251576e-05, 3.7147507315241474e-05, 3.741468195655853e-05, 3.769779359662773e-05, 3.793235212110471e-05, 3.817233209819662e-05, 2.102853778488628e-05, 2.131969518246847e-05, 2.1928246548387945e-05, 2.2309560382538844e-05, 2.3159736496308177e-05, 2.3551882876703337e-05, 2.4033072112547726e-05, 2.4405516290526906e-05, 2.495674735067161e-05, 2.5725180645810636e-05, 2.5987249118132868e-05, 2.6938514508225103e-05, 2.7539529073701962e-05, 2.8284480666074812e-05, 2.9002039119625082e-05, 2.9615902942768034e-05, 3.05479019457384e-05, 3.128190086783072e-05, 3.202809595007952e-05, 3.298940449595233e-05, 3.398877973900474e-05, 3.487753786922636e-05, 3.610797350624838e-05, 3.662741523406211e-05, 3.555001602690695e-05, 3.462779592284099e-05, 3.366468446768483e-05, 3.256958707429084e-05, 3.180164781324414e-05, 3.0990466390025687e-05, 3.0191454633149184e-05, 2.924393306673225e-05, 2.8671194810380576e-05, 2.782294682072065e-05, 2.715625076612229e-05, 2.651519324221482e-05, 2.6040968092202995e-05, 2.5570610406889277e-05, 2.4483532698670046e-05, 2.426830879959854e-05, 2.3687943156283066e-05, 2.3406229522585815e-05, 2.2926834912274757e-05, 2.2394158910776894e-05, 2.1988681509434532e-05, 2.1561647179376878e-05, 3.669827065512923e-05, 3.558991483281516e-05, 3.453463660152908e-05, 3.3694397934996166e-05, 3.2579366900873616e-05, 3.167674771138353e-05, 3.082885999683237e-05, 3.0021144333421526e-05, 2.927601069080565e-05, 2.8531344184428417e-05, 2.784572470013923e-05, 2.7188235321817965e-05, 2.655484095979941e-05, 2.5937032925541372e-05, 2.5409839188110095e-05, 2.486190903183025e-05, 2.431312511740493e-05, 2.3804877416433456e-05, 2.3340944294560985e-05, 2.2871313293573554e-05, 2.243408006759147e-05, 2.1990856443354662e-05, 2.1590868643663856e-05, 0.00017989793084163531, 0.00016667392303886173, 0.00015568885432441939, 0.00014581429377619868, 0.00013732156435429925, 0.00013079278238553463, 0.0001226622862740532, 0.00011640953966007466, 0.0001107344799342985, 0.00010653750252655795, 0.00010206125466354256, 9.744111151962543e-05, 9.387546807914762e-05, 8.930592600901674e-05, 8.660280264083538e-05, 8.290333222994904e-05, 7.998568056241067e-05, 7.73477852669762e-05, 7.536072158304934e-05, 7.244851444808198e-05, 7.060109261759297e-05, 6.817255719899728e-05, 6.643641728416589e-05, 6.469588371707474e-05, 6.262045622353491e-05, 6.14937490749412e-05, 5.946125748715278e-05, 5.791613276141085e-05, 5.65794555388506e-05, 5.542128035908973e-05, 5.382898128773295e-05, 5.26344909490558e-05, 5.165583137720181e-05, 5.055291662446842e-05, 4.929794800493535e-05, 4.834705975832681e-05, 4.737604751984577e-05, 4.650022001476156e-05, 4.55522793588936e-05, 4.4585900156316776e-05, 4.3896992995827445e-05, 4.299292073529205e-05, 4.207410489154584e-05, 4.132742943473062e-05, 4.075357697851496e-05, 4.008050521131009e-05, 3.940916910292627e-05, 3.867580438729392e-05, 3.809866245070826e-05, 3.749668026377359e-05, 3.668590138333746e-05, 3.6231771153829526e-05, 3.554555796046472e-05, 3.516677805675485e-05, 3.4630649606701444e-05, 3.408780338512576e-05, 3.349581973688204e-05, 3.30943433973802e-05, 3.257917424574856e-05, 3.2122180008764976e-05, 3.176359570862406e-05, 3.1298492978252056e-05, 3.0910946726233935e-05, 3.0543181423222896e-05, 3.0102099403289698e-05, 2.9588359072831163e-05, 2.9260737256096563e-05, 2.8895765712873618e-05, 2.8664382421596155e-05, 2.818332052420008e-05, 2.7837134837204466e-05, 2.7487055177698466e-05, 2.7278132240046454e-05, 2.6879544817218383e-05, 2.665325955882038e-05, 2.6229412866503798e-05, 2.605326826122967e-05, 2.5661341720092964e-05, 2.547060179319822e-05, 2.5183529312853706e-05, 2.485680132756229e-05, 2.4567003591669426e-05, 2.4307260088255454e-05, 2.405403412487513e-05, 2.3814010462822546e-05, 2.3549779409285465e-05, 2.341907877875159e-05, 2.316154078259738e-05, 2.287596779566132e-05, 2.2729767377320737e-05, 2.244536377269717e-05, 2.2201747903438084e-05, 2.2004570867276158e-05, 2.1843076237004567e-05, 2.157344874400114e-05, 2.1398983741469467e-05, 2.118633415963724e-05, 2.0993663592455922e-05, 2.0799667844924282e-05, 2.0603754208245806e-05, 2.044843392734649e-05, 2.0263774030616927e-05, 2.0082731506860316e-05, 1.9916132343218294e-05, 1.970559964017691e-05, 1.9573693750528955e-05, 1.940992375576684e-05, 1.923547374976923e-05, 1.9103299064936993e-05, 6.437000896775354e-05, 6.609191716816253e-05, 6.802703564254357e-05, 6.995960994726697e-05, 7.222554771437215e-05, 7.48524370401405e-05, 7.705951149386457e-05, 7.993944123004589e-05, 8.261225895819801e-05, 8.601951124340279e-05, 8.941326796748757e-05, 8.941928367672352e-05, 8.619414230432713e-05, 8.31486281045255e-05, 8.004750146019474e-05, 7.748148386897486e-05, 7.502670407782409e-05, 7.279803996465797e-05, 7.030282184383354e-05, 6.838138636010617e-05, 6.622232221436901e-05, 6.431747437572383e-05, 6.435613819024624e-05, 6.624446024487495e-05, 6.824055078363819e-05, 7.007503032128907e-05, 7.240280540758932e-05, 7.490694623022208e-05, 7.711310096541419e-05, 8.006289354997511e-05, 8.245671882392809e-05, 8.572586835095792e-05, 8.931244962560864e-05, 8.936659092763767e-05, 8.615786335842376e-05, 8.31007525997646e-05, 8.021899389805215e-05, 7.762507800950659e-05, 7.519463234735826e-05, 7.267088857878207e-05, 7.057086418075975e-05, 6.826876535146e-05, 6.649186708336516e-05, 6.443913085364202e-05, 6.440713499240302e-05, 6.60355844066151e-05, 6.790509306234823e-05, 7.031415088081669e-05, 7.228283377116624e-05, 7.442426135347129e-05, 7.728710910015905e-05, 8.001452893205068e-05, 8.283995477124673e-05, 8.589582896133155e-05, 8.929054983901227e-05, 8.931657936625224e-05, 8.626048052312817e-05, 8.288570951721357e-05, 7.996954390435716e-05, 7.733525974186145e-05, 7.503081540463473e-05, 7.264060530509614e-05, 7.029131159176123e-05, 6.817269687027084e-05, 6.621214656094613e-05, 6.436925929877793e-05, 6.442800051517609e-05, 6.595319373647212e-05, 6.78992824410984e-05, 6.997804065200227e-05, 7.210883785421049e-05, 7.474280147249415e-05, 7.731297285763354e-05, 7.998153889202689e-05, 8.291356944669405e-05, 8.561366896840866e-05, 8.937396879135062e-05, 8.928181952693686e-05, 8.639701015129222e-05, 8.293530309936296e-05, 8.003185387402264e-05, 7.740981140938368e-05, 7.480286155576013e-05, 7.25193712231322e-05, 7.060050685822764e-05, 6.817487826078329e-05, 6.626886785980925e-05, 6.45388075695309e-05, 6.436874989075155e-05, 6.632074845730285e-05, 6.813179229956141e-05, 6.99828717096315e-05, 7.231110343425752e-05, 7.477273377166224e-05, 7.718938278239618e-05, 7.985660796349165e-05, 8.247810750997814e-05, 8.547425064638639e-05, 8.933884686633405e-05, 8.919667035314726e-05, 8.632825519584929e-05, 8.332414932586479e-05, 8.001529474833002e-05, 7.743038052623788e-05, 7.48648277262026e-05, 7.240237172183244e-05, 7.037773841864758e-05, 6.845558350531947e-05, 6.622208360224708e-05, 6.458438859818297e-05, 6.437480772130053e-05, 6.618618473271577e-05, 6.826923056170872e-05, 7.000817932957648e-05, 7.226591165902583e-05, 7.450992492918524e-05, 7.740674586818413e-05, 7.980129733159892e-05, 8.295225663106017e-05, 8.56760859202865e-05, 8.933468216370342e-05, 8.930769262310082e-05, 8.64660135661559e-05, 8.3240002213107e-05, 8.02197129384706e-05, 7.742543436874197e-05, 7.484797992020575e-05, 7.249600062671064e-05, 7.039448001713089e-05, 6.835391802509012e-05, 6.652532802270366e-05, 6.451325796831295e-05, 6.451892666687963e-05, 6.623908384927461e-05, 6.817881958197959e-05, 7.006189072997383e-05, 7.24791895905398e-05, 7.472890380828922e-05, 7.734706639311159e-05, 8.013651701762373e-05, 8.29050585241371e-05, 8.603009465715116e-05, 8.935305605049078e-05, 8.935663360563129e-05, 8.648372044351231e-05, 8.332564002913884e-05, 7.998235502487738e-05, 7.742869538050867e-05, 7.486425078420991e-05, 7.256813521584818e-05, 7.026102163727167e-05, 6.824766391361133e-05, 6.632173474804975e-05, 6.454636256100246e-05, 6.435926452407158e-05, 6.620122549922845e-05, 6.81529853489646e-05, 6.998108704960326e-05, 7.242773580961861e-05, 7.478310196341431e-05, 7.729585138199359e-05, 7.967227996967287e-05, 8.288600695638336e-05, 8.599086752406786e-05, 8.92609813892872e-05, 8.936923658368949e-05, 8.653958624860597e-05, 8.28759410441273e-05, 7.98822921986923e-05, 7.748690857573706e-05, 7.512065262124056e-05, 7.243853392077715e-05, 7.035465568489712e-05, 6.825259993056713e-05, 6.646543435305364e-05, 6.465413540186307e-05, 6.435830519410215e-05, 6.606191631549344e-05, 6.779953500045452e-05, 6.992421499824927e-05, 7.248645052635686e-05, 7.485738948841073e-05, 7.711662492902382e-05, 7.972150787603545e-05, 8.232443715195223e-05, 8.562086067819452e-05, 8.935982219220319e-05, 3.7751192292915604e-05, 3.728968362162855e-05, 3.665855598485811e-05, 3.6194176228500386e-05, 3.5577633138000925e-05, 3.502767283335665e-05, 3.453355747634424e-05, 3.403067673527123e-05, 3.353149249388891e-05, 3.302089381116091e-05, 3.261517007492257e-05, 3.2105889073935084e-05, 3.163697372473068e-05, 3.1648763717021176e-05, 3.202535382262299e-05, 3.259897889350623e-05, 3.2994905077526146e-05, 3.3470955831422424e-05, 3.3996510752820914e-05, 3.445150285439551e-05, 3.503329314743699e-05, 3.5561068419336474e-05, 3.6144555384844625e-05, 3.6647940757065486e-05, 3.725411148916786e-05, 3.7878843628951994e-05, 3.791622286650054e-05, 3.734731027736894e-05, 3.6754230332358805e-05, 3.6176694379618475e-05, 3.5614707750695074e-05, 3.510204430147461e-05, 3.453004763594291e-05, 3.406667294423608e-05, 3.350488395800635e-05, 3.307470456041311e-05, 3.2590608721271426e-05, 3.223662340433177e-05, 3.1648325320597974e-05, 3.164764695405814e-05, 3.20776224838345e-05, 3.258197758919429e-05, 3.303498035403951e-05, 3.3453154046639004e-05, 3.3989347468126445e-05, 3.445282273715012e-05, 3.4945676641228973e-05, 3.553254777529819e-05, 3.60114468507093e-05, 3.667884305610148e-05, 3.722129298129871e-05, 3.785957155228985e-05, 3.789269408678911e-05, 3.735025495026211e-05, 3.672933558830085e-05, 3.620600189308939e-05, 3.556018258404195e-05, 3.508035560492065e-05, 3.447513782486948e-05, 3.4015840113248817e-05, 3.354940634857423e-05, 3.303537643226331e-05, 3.255404641973961e-05, 3.2112691657947096e-05, 3.1710086463012124e-05, 3.1672565537848496e-05, 3.201003352415968e-05, 3.2498981812360084e-05, 3.299218635266575e-05, 3.340587969297239e-05, 3.39381312961545e-05, 3.443493123840413e-05, 3.496841717616863e-05, 3.552475831941872e-05, 3.605449955263151e-05, 3.665162398713225e-05, 3.7241110193922365e-05, 3.7808103826607605e-05, 3.79488810987405e-05, 3.72980186156869e-05, 3.668540271483855e-05, 3.618923873192948e-05, 3.561430920159424e-05, 3.5048254413098675e-05, 3.4517908708416546e-05, 3.403725205332728e-05, 3.355735778118881e-05, 3.304529071865428e-05, 3.259308590249692e-05, 3.2136281419254537e-05, 3.173643422085462e-05, 3.166529451067197e-05, 3.207244968109005e-05, 3.2502840522119145e-05, 3.294971934261905e-05, 3.3476482617678856e-05, 3.397591414385845e-05, 3.447877477843221e-05, 3.498040510791641e-05, 3.561707818888672e-05, 3.60178243593582e-05, 3.659320948500004e-05, 3.7240684243038066e-05, 3.781604529390689e-05, 3.782906412234421e-05, 3.725531160547006e-05, 3.67021867361964e-05, 3.6058832201710375e-05, 3.554865673162455e-05, 3.509695725133871e-05, 3.451015580513471e-05, 3.401048253757979e-05, 3.3497458573785134e-05, 3.3113845281116464e-05, 3.255189312146583e-05, 3.2135761261715825e-05, 3.169107167929224e-05, 3.165627514709697e-05, 3.206568005276303e-05, 3.2516527437630983e-05, 3.299113219283025e-05, 3.339646991065413e-05, 3.395558896687686e-05, 3.446980301283135e-05, 3.5002817869541875e-05, 3.55452648354445e-05, 3.609052282292646e-05, 3.6658869357910856e-05, 3.722558496623433e-05, 3.786136785347428e-05, 3.7889879510070014e-05, 3.728064616692551e-05, 3.681912197104291e-05, 3.6147170917414815e-05, 3.555452213807799e-05, 3.509910851345768e-05, 3.451414362006681e-05, 3.398760193917481e-05, 3.350245327267213e-05, 3.303578028006331e-05, 3.258985607769649e-05, 3.211104694478308e-05, 3.1651152884602756e-05, 3.1695502117496664e-05, 3.205942371811955e-05, 3.257810969522769e-05, 3.300115845718404e-05, 3.349453029748128e-05, 3.397793186659135e-05, 3.443865398251056e-05, 3.504403923309355e-05, 3.561910794686733e-05, 3.6121586965642786e-05, 3.6690688481066885e-05, 3.725809564767277e-05, 3.798101745880933e-05, 3.790175667046739e-05, 3.734935035929479e-05, 3.6704348657150954e-05, 3.620165211168678e-05, 3.559786196618704e-05, 3.506120175314491e-05, 3.456314396443473e-05, 3.4035213161693715e-05, 3.348064639453368e-05, 3.3016195621625734e-05, 3.2551120785171856e-05, 3.213851277207246e-05, 3.168441795485013e-05, 3.166184326103864e-05, 3.2099137443811316e-05, 3.256337135544615e-05, 3.3012877315651816e-05, 3.352564494381616e-05, 3.393742905240615e-05, 3.442510476046552e-05, 3.497188595781952e-05, 3.550529137149154e-05, 3.605796101965192e-05, 3.6598525383977356e-05, 3.724605428642699e-05, 3.788701649118747e-05, 3.789343545707015e-05, 3.730125012731804e-05, 3.6750716025843007e-05, 3.6196930511290996e-05, 3.555333625928338e-05, 3.511485733899603e-05, 3.4540554140491494e-05, 3.404300492595718e-05, 3.3533606027374983e-05, 3.3075650546951064e-05, 3.2565169890366956e-05, 3.210222587510704e-05, 3.172461796195882e-05, 3.1675461001364575e-05, 3.2032529194307015e-05, 3.250621633448127e-05, 3.301572781228163e-05, 3.3457990653892606e-05, 3.39943646446606e-05, 3.4452476176569666e-05, 3.494762955213803e-05, 3.5572412598013593e-05, 3.601666496260075e-05, 3.657299940853273e-05, 3.7249935250317074e-05, 3.7872366485808314e-05, 3.7948047561916695e-05, 3.7313923074397396e-05, 3.6705147225233295e-05, 3.6179828539668704e-05, 3.5657430403145627e-05, 3.507800533562869e-05, 3.45635396056553e-05, 3.410613086428796e-05, 3.350753886460016e-05, 3.307988784374294e-05, 3.257708030579405e-05, 3.213753408306983e-05, 3.1675204011011634e-05, 3.166604500545721e-05, 3.2077839318956585e-05, 3.252291309986449e-05, 3.3040261869520896e-05, 3.346475315861635e-05, 3.39607960938916e-05, 3.449010063263224e-05, 3.5028124474017015e-05, 3.549151251310394e-05, 3.604755384626299e-05, 3.671483673118163e-05, 3.7292188700884916e-05, 3.783067473458075e-05, 3.7938143985851374e-05, 3.724720364065454e-05, 3.672463953675995e-05, 3.612523022638644e-05, 3.563381263676313e-05, 3.5077576142058964e-05, 3.454065352914174e-05, 3.402798824189923e-05, 3.3558224485026176e-05, 3.311740970232846e-05, 3.262117238592223e-05, 3.2099267013900315e-05, 3.1696728943087704e-05, 3.166940303400096e-05, 3.2016972474371294e-05, 3.2529495327861545e-05, 3.300080045486828e-05, 3.3455768713797157e-05, 3.402197941032663e-05, 3.445869982962244e-05, 3.503933997680318e-05, 3.551297138629444e-05, 3.603919106931777e-05, 3.669668772999325e-05, 3.725874632317133e-05, 3.793632002218143e-05, 5.034140386009787e-05, 5.1405417764363034e-05, 5.2607437875735724e-05, 5.383221613013851e-05, 5.502028761743824e-05, 5.648375273427655e-05, 5.792766872338838e-05, 5.919078017923184e-05, 6.089536580801086e-05, 6.254933219998784e-05, 6.43514830916855e-05, 6.440496811499396e-05, 6.259064503955025e-05, 6.110693785846252e-05, 5.966679756980533e-05, 5.812655189259126e-05, 5.6468290557270446e-05, 5.512658675732061e-05, 5.385745358409542e-05, 5.269286711917042e-05, 5.157988324694074e-05, 5.030312793421826e-05, 5.031585057373114e-05, 5.145009413462307e-05, 5.2633538181251045e-05, 5.381120710647997e-05, 5.485192967768537e-05, 5.627024784588277e-05, 5.771102140395292e-05, 5.924453639298655e-05, 6.0985256275115705e-05, 6.2717355005828e-05, 6.42983722477551e-05, 6.445241541678502e-05, 6.28861719349636e-05, 6.12391705668629e-05, 5.9375337637671876e-05, 5.7878660229788826e-05, 5.6554692728739017e-05, 5.537573346070511e-05, 5.3845376912466736e-05, 5.270975924154786e-05, 5.1560356811615425e-05, 5.031337255155373e-05, 5.031435979415981e-05, 5.1336092660983214e-05, 5.2602345789020385e-05, 5.3653066428830064e-05, 5.494810079494163e-05, 5.6243334247534805e-05, 5.766098964064527e-05, 5.938828924997739e-05, 6.098781479294144e-05, 6.266899178490844e-05, 6.445888717859621e-05, 6.435442734193223e-05, 6.262007264345963e-05, 6.119637547850869e-05, 5.953506546101573e-05, 5.8411675368688715e-05, 5.654375767548761e-05, 5.5102602577420655e-05, 5.3936790750408315e-05, 5.2645546815913934e-05, 5.1552333280746036e-05, 5.039851382105782e-05, 5.037903385628458e-05, 5.14232276143403e-05, 5.260888394533848e-05, 5.3739162544933895e-05, 5.508690759699852e-05, 5.648372291179113e-05, 5.7897711341508705e-05, 5.940571311670336e-05, 6.099129972639748e-05, 6.262592701069818e-05, 6.411817007052168e-05, 6.404532403661034e-05, 6.262831123492084e-05, 6.111119223936633e-05, 5.96180420657171e-05, 5.8046955630392255e-05, 5.656844026646922e-05, 5.5176024523229084e-05, 5.384528775297232e-05, 5.276006031204139e-05, 5.1596525673483406e-05, 5.0390754565021574e-05, 5.029039018977031e-05, 5.125850596517278e-05, 5.242868932882805e-05, 5.3865039474113424e-05, 5.4994238701883545e-05, 5.64148832548535e-05, 5.796665777992641e-05, 5.931897176498817e-05, 6.094442161013203e-05, 6.256395007796395e-05, 6.421630766821287e-05, 6.439465385765042e-05, 6.29379571601221e-05, 6.112459024311006e-05, 5.950007475545741e-05, 5.8054109821853146e-05, 5.6455444929424474e-05, 5.529352132969053e-05, 5.39538078747531e-05, 5.2700051209835296e-05, 5.1420796864053197e-05, 5.042776731460197e-05, 5.030568198690004e-05, 5.1415459144864505e-05, 5.241967617498591e-05, 5.3598822012293104e-05, 5.4948038666427966e-05, 5.648835630600807e-05, 5.767063287259522e-05, 5.913823139489869e-05, 6.094298176575962e-05, 6.238846214628405e-05, 6.420918792569917e-05, 6.439340466956352e-05, 6.282898082853965e-05, 6.123292794362629e-05, 5.941513002418885e-05, 5.786509012954889e-05, 5.653104198543727e-05, 5.5106606621919205e-05, 5.397987649836218e-05, 5.259640678536846e-05, 5.1506750707168715e-05, 5.043035137699779e-05, 5.031507102388318e-05, 5.1305851262962184e-05, 5.2476353357133e-05, 5.3836885396618e-05, 5.5013396840533406e-05, 5.6302035072407974e-05, 5.7855636213154304e-05, 5.943390049123672e-05, 6.0990343043362295e-05, 6.246588300992482e-05, 6.409042355317809e-05, 6.44348327937699e-05, 6.271426496367413e-05, 6.1134152807013e-05, 5.957155399866741e-05, 5.8015527446958017e-05, 5.664130623870771e-05, 5.519081942323335e-05, 5.4057928027944565e-05, 5.267370515920322e-05, 5.155301923332817e-05, 5.0403935799510675e-05, 5.0341164914316955e-05, 5.1292163680241964e-05, 5.2578336697311223e-05, 5.3844128511563677e-05, 5.4980165233575966e-05, 5.658388265882416e-05, 5.797904634068593e-05, 5.917297585689226e-05, 6.097033466746626e-05, 6.263971227916564e-05, 6.414240418509895e-05, 6.436811825080474e-05, 6.287065963629307e-05, 6.122302070084911e-05, 5.94538387140932e-05, 5.789070762744889e-05, 5.6469296016591675e-05, 5.513244248127394e-05, 5.391803747045287e-05, 5.277204314958472e-05, 5.141990595941896e-05, 5.045052079655304e-05, 5.035730613175807e-05, 5.136995318603863e-05, 5.248807421308843e-05, 5.3650080757110576e-05, 5.495618511921608e-05, 5.647730634089918e-05, 5.7758594946598075e-05, 5.919077158070698e-05, 6.092956284021412e-05, 6.253316357075593e-05, 6.426100576921405e-05, 5.035457557538552e-05, 4.930078239461595e-05, 4.825266986317651e-05, 4.727792980364449e-05, 4.6283921212879556e-05, 4.548334830688956e-05, 4.446675595678267e-05, 4.375159801569403e-05, 4.285108968047684e-05, 4.213146624850646e-05, 4.132504980694618e-05, 4.133632522312197e-05, 4.192453917363149e-05, 4.2813854738661405e-05, 4.3549487417997815e-05, 4.4495480323794444e-05, 4.531166610887322e-05, 4.621593814631153e-05, 4.709320735788235e-05, 4.818444097212653e-05, 4.92767863714827e-05, 5.0300872843307454e-05, 5.0337960624243016e-05, 4.9276418774402044e-05, 4.8215202784618976e-05, 4.723096500184233e-05, 4.639114940173286e-05, 4.548522591934184e-05, 4.456424600747187e-05, 4.373936848509646e-05, 4.290922849276538e-05, 4.213937048648347e-05, 4.130285955461042e-05, 4.130236994910505e-05, 4.1979248117324056e-05, 4.269119034265016e-05, 4.3604112302832606e-05, 4.435402878203115e-05, 4.535139302389879e-05, 4.628234915499173e-05, 4.7108436326960684e-05, 4.811319881831885e-05, 4.9221446382178286e-05, 5.0354393468478535e-05, 5.030613569826519e-05, 4.927454761222819e-05, 4.824268054411011e-05, 4.7206416549120936e-05, 4.6392005795358875e-05, 4.5338890784171915e-05, 4.461590929284196e-05, 4.3721595039077314e-05, 4.291112967932699e-05, 4.217006397347894e-05, 4.130978227451109e-05, 4.1311230569476006e-05, 4.197167642487683e-05, 4.2836886494862924e-05, 4.3611494797965546e-05, 4.454400621066487e-05, 4.5402266534714e-05, 4.623368733474681e-05, 4.7246811520232464e-05, 4.822905304441845e-05, 4.912449023052604e-05, 5.017678220854041e-05, 5.035166473668417e-05, 4.9233158945661674e-05, 4.818222887709612e-05, 4.723951465798279e-05, 4.636267887923636e-05, 4.534696312892289e-05, 4.4487403964018563e-05, 4.36556630781099e-05, 4.2888531169789434e-05, 4.2119631696237055e-05, 4.1247135484566024e-05, 4.1340445694374894e-05, 4.196896845094025e-05, 4.283135632119441e-05, 4.3644761298102085e-05, 4.453032866262508e-05, 4.5296107358187906e-05, 4.6291800981699324e-05, 4.7092538604164465e-05, 4.82646519235206e-05, 4.906287362708155e-05, 5.036803717833671e-05, 5.0334152221174375e-05, 4.938195723291976e-05, 4.827405589868881e-05, 4.733710425840426e-05, 4.638063516126342e-05, 4.540383594047974e-05, 4.457776823271557e-05, 4.370996740117738e-05, 4.29337522209355e-05, 4.209359070422648e-05, 4.1331224774177686e-05, 4.130770035223098e-05, 4.2007242660002904e-05, 4.28141644329183e-05, 4.3692997348884565e-05, 4.441932570338104e-05, 4.519206560001371e-05, 4.623372344307561e-05, 4.722494308605365e-05, 4.8182616237991456e-05, 4.919530943249277e-05, 5.020928219704823e-05, 4.9257449319461154e-05, 4.822620080052973e-05, 4.728752117331438e-05, 4.625174812413154e-05, 4.539681465819116e-05, 4.4569377695315487e-05, 4.379116868415113e-05, 4.288325997612677e-05, 4.2043617315392526e-05, 4.141488686148312e-05, 4.060477190451614e-05, 4.05503338635481e-05, 4.125175330345315e-05, 4.2001866332455264e-05, 4.281357562707128e-05, 4.3676342233404634e-05, 4.45346529832063e-05, 4.521937471011462e-05, 4.6258960165135195e-05, 4.7137718639087575e-05, 4.822208588212002e-05, 4.9142311542259185e-05, 4.912314011974074e-05, 4.8215905278150096e-05, 4.72473927439505e-05, 4.631077600125899e-05, 4.536615867113055e-05, 4.45547287320946e-05, 4.376378866607297e-05, 4.284312709374968e-05, 4.2076536960322894e-05, 4.133273219942854e-05, 4.057883066160522e-05, 4.055887159244248e-05, 4.1196315491218e-05, 4.206237537582016e-05, 4.276243060879357e-05, 4.364580628473308e-05, 4.4486908239400464e-05, 4.5257693034534834e-05, 4.628465968941232e-05, 4.7290789025449946e-05, 4.8242748875778795e-05, 4.925971131306194e-05, 4.9213434127263324e-05, 4.823634193394465e-05, 4.7214418629905554e-05, 4.633957583474108e-05, 4.537350592095328e-05, 4.451636415024606e-05, 4.364047208078603e-05, 4.292934410566301e-05, 4.214847720954769e-05, 4.128071187366586e-05, 4.065086676829054e-05, 4.061679970245612e-05, 4.1304974048649914e-05, 4.198723088647108e-05, 4.2832576527718665e-05, 4.353083738141544e-05, 4.447422862436455e-05, 4.527203206687006e-05, 4.631710903457787e-05, 4.724509528455652e-05, 4.820861866875464e-05, 4.930593438996716e-05, 4.91931403558847e-05, 4.824530791335073e-05, 4.727491695037915e-05, 4.632104613716276e-05, 4.5473234915776674e-05, 4.458253311627186e-05, 4.3690826693844785e-05, 4.2933019723733636e-05, 4.2115725065603036e-05, 4.1299635322050806e-05, 4.067175244261111e-05, 4.058179650812032e-05, 4.130646652488008e-05, 4.205130516539379e-05, 4.28471109021168e-05, 4.356379613405356e-05, 4.448687325916366e-05, 4.522236846765932e-05, 4.621714938485665e-05, 4.723179870397662e-05, 4.817421979490531e-05, 4.908284706814348e-05, 4.9261096024233474e-05, 4.8211712327843917e-05, 4.7289827940155603e-05, 4.9205300426030306e-05, 4.8263393024441824e-05, 4.731113375016807e-05, 4.632316041130101e-05, 4.5364283834991685e-05, 4.456177678059068e-05, 4.3760501371339595e-05, 4.293125624883577e-05, 4.2043227872843164e-05, 4.13783349608679e-05, 4.0612602519158525e-05, 3.995840011351652e-05, 3.9203387802945624e-05, 3.856663678791803e-05, 3.8565229145670416e-05, 3.919295893455285e-05, 3.981906097119867e-05, 4.047351392044631e-05, 4.120727345974844e-05, 4.2086710393830326e-05, 4.2873854346735265e-05, 4.364529358730192e-05, 4.449133110561559e-05, 4.533304532166667e-05, 4.6271777485094105e-05, 4.7072427080619567e-05, 4.804881221870045e-05, 4.9290256285644085e-05, 4.926537341373025e-05, 4.8214509801937145e-05, 4.729853554157841e-05, 4.63556514431082e-05, 4.5382818146725606e-05, 4.446422588775666e-05, 4.369164527021448e-05, 4.2905040446333725e-05, 4.208879481080848e-05, 4.138230541281744e-05, 4.057991089567235e-05, 3.9878993800501975e-05, 3.920985999310327e-05, 3.855045365409554e-05, 3.853621743762969e-05, 3.914421482480027e-05, 3.9762104836476194e-05, 4.0533498992231405e-05, 4.120627618236827e-05, 4.197260446494767e-05, 4.27691289788613e-05, 4.3636881072560864e-05, 4.438491663211854e-05, 4.543635132619398e-05, 4.6340543821129005e-05, 4.712252133152232e-05, 4.8176949358119496e-05, 4.9169845977918695e-05, 4.9293639690352837e-05, 4.82149422688862e-05, 4.7209776043721284e-05, 4.6377336694175334e-05, 4.544644703371204e-05, 4.457906732561918e-05, 4.3698768866515134e-05, 4.293349378614062e-05, 4.212962497116571e-05, 4.126531733085218e-05, 4.0613489630784294e-05, 3.9954313716609416e-05, 3.929086950404034e-05, 3.852494963661558e-05, 3.853037168023719e-05, 3.924805060142447e-05, 3.986474157607062e-05, 4.0524708315758945e-05, 4.132927029516253e-05, 4.2060221673686054e-05, 4.2736396178036285e-05, 4.3656454085391626e-05, 4.437687677196206e-05, 4.533112198286333e-05, 4.6303196441935344e-05, 4.7260364944102104e-05, 4.8129964186686e-05, 4.917172893778875e-05, 4.9210061378211925e-05, 4.823704040366688e-05, 4.726318820944011e-05, 4.632018343501095e-05, 4.5476493564722366e-05, 4.449262459808792e-05, 4.375771641456476e-05, 4.28633598708048e-05, 4.215130673305953e-05, 4.137648249709009e-05, 4.056312922238923e-05, 3.990772334815839e-05, 3.9165280098888916e-05, 3.857974924678954e-05, 3.855931498438499e-05, 3.914736459927821e-05, 3.9817107596050764e-05, 4.056922032654882e-05, 4.1344027875354466e-05, 4.1891390857666697e-05, 4.285816469581176e-05, 4.366145982827315e-05, 4.436599884905807e-05, 4.534140004533643e-05, 4.628862036000851e-05, 4.731039625847882e-05, 4.825344228976778e-05, 4.920981749216566e-05, 4.921330124599363e-05, 4.8208624039970574e-05, 4.721036153144611e-05, 4.643167989899716e-05, 4.5428248839126225e-05, 4.4501301246354094e-05, 4.362266956049129e-05, 4.2927388994296786e-05, 4.2043417045480565e-05, 4.134189714717249e-05, 4.056034877108787e-05, 3.9917591875643004e-05, 3.922885749242704e-05, 3.8550820567426624e-05, 3.978574526142367e-05, 3.9174660514276535e-05, 3.854251680235271e-05, 3.851458225778182e-05, 3.9047587275290065e-05, 3.9786232398713685e-05, 3.9850209830756225e-05, 3.9206027805050116e-05, 3.858071984809523e-05, 3.847789065140595e-05, 3.912173467999824e-05, 3.984312301497833e-05, 3.9848005946169916e-05, 3.919799155347819e-05, 3.854630357790742e-05, 3.8530748983086115e-05, 3.911264819279489e-05, 3.973300539073634e-05, 3.98583178096035e-05, 3.917765243912157e-05, 3.854181404990039e-05, 3.852313203211526e-05, 3.910219613863789e-05, 3.9769920090139594e-05, 3.986306157770142e-05, 3.915630314680574e-05, 3.855983686597044e-05, 3.979781592245742e-05, 3.923525148650886e-05, 3.8535817310704016e-05, 3.7968082347300365e-05, 3.7324887158624575e-05, 3.6727579420033637e-05, 3.614330763786105e-05, 3.5553534729170675e-05, 3.505034386417848e-05, 3.456290490596515e-05, 3.401252157763598e-05, 3.347503480032623e-05, 3.3052733780554244e-05, 3.253282129605657e-05, 3.210434466738831e-05, 3.1675650595023693e-05, 3.1256457942296714e-05, 3.080708181495749e-05, 3.04230555923191e-05, 2.9996465991900285e-05, 2.9664813910527506e-05, 2.9278844614143605e-05, 2.8906425841285385e-05, 2.85302780835941e-05, 2.8221454473483897e-05, 2.7841892323532745e-05, 2.7504568876298417e-05, 2.7189756904348253e-05, 2.6867535564891757e-05, 2.657965468232256e-05, 2.6258019918388047e-05, 2.596729919687742e-05, 2.5644247500042603e-05, 2.5389613605084715e-05, 2.512458667494002e-05, 2.4858293451836762e-05, 2.4569290521129328e-05, 2.4340848301301122e-05, 2.403990087551123e-05, 2.3821442838564363e-05, 2.3579913823692036e-05, 2.3350900524947192e-05, 2.3095836284456867e-05, 2.2912847639044594e-05, 2.2643906942458915e-05, 2.2453377596639828e-05, 2.2413545002011955e-05, 2.264086628013591e-05, 2.2852035579448446e-05, 2.3046487105912263e-05, 2.33335673815276e-05, 2.3561968391426693e-05, 2.378270649956887e-05, 2.3999096465037315e-05, 2.430695809914132e-05, 2.4519167746311992e-05, 2.4848701613163618e-05, 2.5048702913721435e-05, 2.5368498378776492e-05, 2.5664629003759286e-05, 2.5916713476722578e-05, 2.6186788105952318e-05, 2.652051139503117e-05, 2.67960013091869e-05, 2.7125354816864744e-05, 2.7488447335136823e-05, 2.7791857235427556e-05, 2.8154931039059754e-05, 2.8511353384149216e-05, 2.8846287024066625e-05, 2.9244215323624077e-05, 2.9568614260134713e-05, 2.997164506780307e-05, 3.032697286357333e-05, 3.0754151769332044e-05, 3.1224538336453484e-05, 3.164189484793498e-05, 3.211896826305098e-05, 3.248968109847988e-05, 3.2950341640601424e-05, 3.3479983364170464e-05, 3.4008044577169643e-05, 3.4399183820497e-05, 3.500206050714747e-05, 3.5597532061194634e-05, 3.600999962664939e-05, 3.6637431368391435e-05, 3.720394227702325e-05, 3.791095452337691e-05, 3.847394646909481e-05, 3.9267006544402277e-05, 3.986100887011532e-05, 3.9866466802416444e-05, 3.927622561936738e-05, 3.850212855833677e-05, 3.794008649392767e-05, 3.73241746032598e-05, 3.673607709643806e-05, 3.610481837269171e-05, 3.553652744434842e-05, 3.507788677824729e-05, 3.45086215467281e-05, 3.4019594673428793e-05, 3.350523983356247e-05, 3.305653857994485e-05, 3.2547186830194956e-05, 3.211929928362084e-05, 3.1667222023797934e-05, 3.1258227019928556e-05, 3.081655657692816e-05, 3.040407627746713e-05, 3.000324858359476e-05, 2.9627425078539313e-05, 2.9268331200212423e-05, 2.8927364409161984e-05, 2.851128335162519e-05, 2.8173626617696685e-05, 2.7850952162831896e-05, 2.7484754520011398e-05, 2.7173224751106342e-05, 2.6861791576811585e-05, 2.6580315140983096e-05, 2.6273042522031476e-05, 2.5975225834214716e-05, 2.5648573436174822e-05, 2.537096183554941e-05, 2.5114642373509874e-05, 2.4902549554039933e-05, 2.4577124007704362e-05, 2.4317170270710994e-05, 2.4025116091956863e-05, 2.3833018905075276e-05, 2.357720605063146e-05, 2.3339209298998737e-05, 2.3084063503196565e-05, 2.2891642661628105e-05, 2.2651875556870604e-05, 2.2448924780133204e-05, 2.24251378561797e-05, 2.2631581540687327e-05, 2.2859351443182244e-05, 2.3063060210869157e-05, 2.329026322334401e-05, 2.3585646242923736e-05, 2.3816628384059214e-05, 2.4049054372156625e-05, 2.4253778435682087e-05, 2.454672260566178e-05, 2.48526831590037e-05, 2.5090794210341412e-05, 2.5356198600148973e-05, 2.5619574182177763e-05, 2.5967754935249348e-05, 2.622352414806676e-05, 2.654304042466154e-05, 2.6854990607385756e-05, 2.718292900480095e-05, 2.75147713172493e-05, 2.7868413034155355e-05, 2.8190227523455554e-05, 2.8543257150956376e-05, 2.8884375325863467e-05, 2.9287770445720947e-05, 2.9616334789195504e-05, 3.00184087003563e-05, 3.0421397261671908e-05, 3.081526624224572e-05, 3.120282258932931e-05, 3.167302938251226e-05, 3.211608311973989e-05, 3.257201200971539e-05, 3.30390801028894e-05, 3.349605877713694e-05, 3.397295325898909e-05, 3.454386928202263e-05, 3.501919475877586e-05, 3.557546968658353e-05, 3.612239437083813e-05, 3.671280416274013e-05, 3.731281590879786e-05, 3.788869937488089e-05, 3.852915003502697e-05, 3.927208687690683e-05, 3.9881299295770953e-05, 2.263220365071051e-05, 2.2831123297403587e-05, 2.3088399053253136e-05, 2.3358302094629415e-05, 2.3579477052442172e-05, 2.3804494758509472e-05, 2.40656336852992e-05, 2.432077530065545e-05, 2.455610711575019e-05, 2.486406521181252e-05, 2.512314164722194e-05, 2.5401962521498e-05, 2.5666509538750732e-05, 2.59760456741991e-05, 2.626856774449677e-05, 2.6547431171468844e-05, 2.6857514110817734e-05, 2.7198755081461864e-05, 2.7497792223615107e-05, 2.781418588428158e-05, 2.8167361136435755e-05, 2.852917329163786e-05, 2.889307312575448e-05, 2.925316615001929e-05, 2.9626639498313005e-05, 3.0003568846460276e-05, 3.0413728046575496e-05, 3.0818883510217944e-05, 3.12420123098102e-05, 3.1252013665374115e-05, 3.083932446916404e-05, 3.040037652051647e-05, 2.999488086776648e-05, 2.9620237935845744e-05, 2.928162076838615e-05, 2.887661522672245e-05, 2.851119167268336e-05, 2.8182305489721463e-05, 2.786275703144489e-05, 2.7514763717808725e-05, 2.7162149398521954e-05, 2.6861482396807e-05, 2.6557611398975806e-05, 2.6261620048494924e-05, 2.5970898457398923e-05, 2.567456996419079e-05, 2.540744979432776e-05, 2.513088333392281e-05, 2.4844271870256245e-05, 2.4562108820847542e-05, 2.4325327137440477e-05, 2.4077899121191993e-05, 2.3765029771016263e-05, 2.357789552478895e-05, 2.3331871696080505e-05, 2.3105476971104618e-05, 2.2887179667464933e-05, 2.263112786418657e-05, 2.262265702281246e-05, 2.287247342886585e-05, 2.3087662695764567e-05, 2.3325385638634864e-05, 2.356560597334971e-05, 2.384034795417084e-05, 2.4063584435551735e-05, 2.429665929298378e-05, 2.4585049040899413e-05, 2.484125157214702e-05, 2.507846598280678e-05, 2.5361801526890097e-05, 2.570355489453013e-05, 2.5962801408115027e-05, 2.6243123863256755e-05, 2.6559935203695925e-05, 2.6857263084460877e-05, 2.717729541793595e-05, 2.7507629292726218e-05, 2.7853257367754762e-05, 2.818651301150903e-05, 2.8505817957348046e-05, 2.889734139591722e-05, 2.9250899450105057e-05, 2.9588276756352433e-05, 3.002103236134627e-05, 3.039923072843211e-05, 3.0811644740296125e-05, 3.123211925461936e-05, 3.1282095021068016e-05, 3.078786391417802e-05, 3.042721153642215e-05, 2.9999244722186856e-05, 2.9625036407079576e-05, 2.921994583845258e-05, 2.8902601730766592e-05, 2.853721093827479e-05, 2.8197585464773258e-05, 2.781792987792516e-05, 2.7523436239222057e-05, 2.7188569906370937e-05, 2.6874834247411817e-05, 2.6566398972127694e-05, 2.625259829695009e-05, 2.5940388978510693e-05, 2.5707951375027325e-05, 2.5401735936383417e-05, 2.512763624431958e-05, 2.4848673767777173e-05, 2.456872122477678e-05, 2.4297701336776887e-05, 2.40434531663489e-05, 2.382041712978042e-05, 2.358728652489354e-05, 2.3339999700466802e-05, 2.3107638908791007e-05, 2.2854477240825368e-05, 2.2637599136947754e-05, 2.2630238064705422e-05, 2.2882633714007128e-05, 2.3092716420799572e-05, 2.3337732761893786e-05, 2.3565985789445413e-05, 2.3797923816270697e-05, 2.4057993773998653e-05, 2.432965081597003e-05, 2.4592416099780717e-05, 2.48398136622254e-05, 2.5112627643433506e-05, 2.541264729782148e-05, 2.565802809499414e-05, 2.597371841456968e-05, 2.6256861450055628e-05, 2.6545289907164075e-05, 2.68342207828363e-05, 2.7158365539050577e-05, 2.7505957990986335e-05, 2.78055725834907e-05, 2.817432196148033e-05, 2.854764524367252e-05, 2.8899209451031716e-05, 2.926273614392737e-05, 2.9657686839060867e-05, 3.003516642354202e-05, 3.042536347989095e-05, 3.080699749930545e-05, 3.121308477284461e-05, 3.123389413897194e-05, 3.0841258041012005e-05, 3.0385689158775343e-05, 3.0011742534616125e-05, 2.9609203482645685e-05, 2.92208664444776e-05, 2.8876626417324183e-05, 2.8538593204986373e-05, 2.8178501368553984e-05, 2.782404266631568e-05, 2.7505615630739548e-05, 2.7160410131685802e-05, 2.688474127599782e-05, 2.655339415229307e-05, 2.624978343121755e-05, 2.59587993280533e-05, 2.5680155941378146e-05, 2.5391785123009657e-05, 2.5080499523885608e-05, 2.4846760617955026e-05, 2.4546158216874825e-05, 2.428642643472424e-05, 2.406728250782377e-05, 2.3822985812865174e-05, 2.3560555048011606e-05, 2.3336135088407415e-05, 2.3085377033010956e-05, 2.287306218789398e-05, 2.263715653537991e-05, 2.2637983011512868e-05, 2.2866200717975177e-05, 2.311473803259262e-05, 2.331286243962371e-05, 2.357903564948988e-05, 2.3817433514210812e-05, 2.4069658835790343e-05, 2.4304141879701194e-05, 2.457250599968329e-05, 2.48425205856724e-05, 2.5133273825305083e-05, 2.535661167572797e-05, 2.5684398395632138e-05, 2.596795420233706e-05, 2.6251512067589282e-05, 2.656519929437214e-05, 2.6836807382578253e-05, 2.7170127943699196e-05, 2.749255090911888e-05, 2.785256609418967e-05, 2.8154930529516778e-05, 2.852402077741713e-05, 2.8871617484654475e-05, 2.9252471109645033e-05, 2.9640391011762703e-05, 3.0014447676727006e-05, 3.041238813032084e-05, 3.079649536385284e-05, 3.1213077195598323e-05, 3.126937797896339e-05, 3.0812862341727345e-05, 3.0397861525648663e-05, 2.999274475450745e-05, 2.959953407170889e-05, 2.9230809896457566e-05, 2.890275082742194e-05, 2.853140414337067e-05, 2.817433136672315e-05, 2.7812758669126153e-05, 2.7489956353419543e-05, 2.7183784743592188e-05, 2.6856076248166328e-05, 2.656771766664706e-05, 2.6256170682510078e-05, 2.59558074771195e-05, 2.5677898185907606e-05, 2.5368512949780902e-05, 2.515132837726683e-05, 2.483055561145539e-05, 2.456759896277651e-05, 2.4323075673004535e-05, 2.406585671725563e-05, 2.383637248633487e-05, 2.3568304298728548e-05, 2.3339750742228425e-05, 2.3102171683658013e-05, 2.2850730876337644e-05, 2.264226571112274e-05, 2.2656997031136594e-05, 2.2864285049063326e-05, 2.307078947077462e-05, 2.333118212079108e-05, 2.357606585865392e-05, 2.3816727461103827e-05, 2.4069248314266555e-05, 2.4304036712828652e-05, 2.454496028819486e-05, 2.4828292439651386e-05, 2.5083829718313363e-05, 2.538777267347563e-05, 2.5651538727100838e-05, 2.595867006629168e-05, 2.624939171106269e-05, 2.654338397803409e-05, 2.6887302184261963e-05, 2.7164456013235764e-05, 2.7514657138119396e-05, 2.7850035267021355e-05, 2.813202717499282e-05, 2.850582586249253e-05, 2.8904845617987355e-05, 2.9262266933820024e-05, 2.96285256628151e-05, 2.9983714330225082e-05, 3.041817661360926e-05, 3.083401912287425e-05, 3.122190391812806e-05, 3.120851941317175e-05, 3.0820110940657776e-05, 3.0381292057293622e-05, 3.001053538848392e-05, 2.9625385055904183e-05, 2.9272825154598665e-05, 2.88769598477368e-05, 2.852994968845709e-05, 2.8172730980707985e-05, 2.7809312477183828e-05, 2.7503865510690364e-05, 2.7207637606778233e-05, 2.685005674871194e-05, 2.656827754870334e-05, 2.6271063489723007e-05, 2.5972861716810485e-05, 2.5641550864910474e-05, 2.5394822006761437e-05, 2.506582867598383e-05, 2.4855860016052732e-05, 2.457438002827529e-05, 2.432159749291149e-05, 2.4059704745512142e-05, 2.3818736682915853e-05, 2.3554057365749553e-05, 2.331905789300475e-05, 2.310089073167222e-05, 2.2863456185720585e-05, 2.2644848526090736e-05, 2.160290507156653e-05, 2.1796858333637045e-05, 2.1971142588060144e-05, 2.220020244528335e-05, 2.2410524081233184e-05, 2.26424410246135e-05, 2.285849488657949e-05, 2.313199502739011e-05, 2.335426419404357e-05, 2.329573411286267e-05, 2.3112893943139844e-05, 2.2859071333280234e-05, 2.264777818243857e-05, 2.242698204130971e-05, 2.22105252017957e-05, 2.1969686592427822e-05, 2.1788617776719648e-05, 2.1589438569524477e-05, 2.1608607972194636e-05, 2.1796788199517078e-05, 2.1994643879236302e-05, 2.2200899078231543e-05, 2.241817472054526e-05, 2.2639460949365714e-05, 2.2871667860850802e-05, 2.310257653942659e-05, 2.3307897304407205e-05, 2.330712870451516e-05, 2.309788805353779e-05, 2.2854155352652842e-05, 2.2655977256309407e-05, 2.242403606470225e-05, 2.2215759079533174e-05, 2.201793478460222e-05, 2.178351415399362e-05, 2.1585608420409886e-05, 2.158921328234939e-05, 2.1790305308296493e-05, 2.2004454642825616e-05, 2.2226676864791755e-05, 2.2409782837961158e-05, 2.264179005737146e-05, 2.2866626117374657e-05, 2.3088905929635423e-05, 2.334384580017905e-05, 2.3324220493865173e-05, 2.310444219273971e-05, 2.287218466912295e-05, 2.264711863376308e-05, 2.2448835466464026e-05, 2.2216497456076656e-05, 2.199008214070212e-05, 2.1792974529123385e-05, 2.158101249663098e-05, 2.158220334476712e-05, 2.1780540471306447e-05, 2.1987736558573757e-05, 2.2213591311406146e-05, 2.2432821787919928e-05, 2.265814676694444e-05, 2.2875697915733876e-05, 2.3127734218356896e-05, 2.3340107086583897e-05, 2.3368998645781108e-05, 2.3120442075101856e-05, 2.2869597413888576e-05, 2.266537465803301e-05, 2.2425963810159022e-05, 2.220919726479317e-05, 2.1971123901353e-05, 2.1798327826374337e-05, 2.1605089227450658e-05, 2.1574763654610332e-05, 2.178391354689014e-05, 2.200381179743224e-05, 2.219314326575423e-05, 2.2420198966788858e-05, 2.2642595614096266e-05, 2.290028590190711e-05, 2.3091443790994052e-05, 2.3326427440002016e-05, 6.619309594657594e-05, 6.822398019202553e-05, 7.027520802317559e-05, 7.243797783114154e-05, 7.48556353918473e-05, 7.736967503829575e-05, 8.002003388556734e-05, 8.285820393625589e-05, 8.597144270294788e-05, 8.606213531468118e-05, 8.289050327484622e-05, 8.006233934874659e-05, 7.730965922468797e-05, 7.492573664531924e-05, 7.251803305183587e-05, 7.031256350547889e-05, 6.815218500331044e-05, 6.622131540855979e-05, 6.624692647545636e-05, 6.817005243163337e-05, 7.033285600093146e-05, 7.248493315703989e-05, 7.482146041734854e-05, 7.734919573121721e-05, 8.00754254656863e-05, 8.299402620692911e-05, 8.599122976089077e-05, 8.603288463230196e-05, 8.292156865123665e-05, 7.998379139254989e-05, 7.736783177395668e-05, 7.485341281122613e-05, 7.253180985123016e-05, 7.033950740713827e-05, 6.82234772174211e-05, 6.620823780438365e-05, 6.623881469264977e-05, 6.816176557971415e-05, 7.027460105185636e-05, 7.246314018742393e-05, 7.478252057630524e-05, 7.724846255739656e-05, 8.002074836271588e-05, 8.288734267575951e-05, 8.59832646505363e-05, 8.600746379679245e-05, 8.301961047770176e-05, 8.009836935186438e-05, 7.734568883052358e-05, 7.479605461073592e-05, 7.25408800317995e-05, 7.02866752296902e-05, 6.81551263985532e-05, 6.627307295929359e-05, 6.62336741890087e-05, 6.815434161601649e-05, 7.029441108038893e-05, 7.245200356670144e-05, 7.478199273754193e-05, 7.728757404340417e-05, 8.005809471356281e-05, 8.298003422428201e-05, 8.612025977815978e-05, 8.599323663788638e-05, 8.284866308888091e-05, 8.0041885953059e-05, 7.734116824812659e-05, 7.488472464856378e-05, 7.247362876707365e-05, 7.02170552123952e-05, 6.819075252679456e-05, 6.631165241281962e-05, 6.625193423320294e-05, 6.817941228710933e-05, 7.031174235232102e-05, 7.246885218127489e-05, 7.488235941098155e-05, 7.73557528994303e-05, 8.007363625061441e-05, 8.296519986526182e-05, 8.604951219582471e-05, 8.598500723158196e-05, 8.294600525426712e-05, 7.999230114550591e-05, 7.728538406049982e-05, 7.487597931804889e-05, 7.249054761119725e-05, 7.02605222906077e-05, 6.816101301823857e-05, 6.624772232075211e-05, 6.631445292320907e-05, 6.817520443929044e-05, 7.034653813208065e-05, 7.255749482123736e-05, 7.485751625228733e-05, 7.730405105080039e-05, 8.004245768027899e-05, 8.291107568064512e-05, 8.609651167163694e-05, 8.605701503665009e-05, 8.293644990769365e-05, 8.002365302435447e-05, 7.729695469453374e-05, 7.482563143484778e-05, 7.247567973971621e-05, 7.026871448947802e-05, 6.810474875311074e-05, 6.628300200469861e-05, 6.623663553759216e-05, 6.817943858992303e-05, 7.01985301220266e-05, 7.24257011663921e-05, 7.48331367454313e-05, 7.739742088031556e-05, 8.00142372844263e-05, 8.297878785166332e-05, 8.600475927335316e-05, 8.606043117501313e-05, 8.292951947619548e-05, 8.00828090529236e-05, 7.738785087396713e-05, 7.485840458886391e-05, 7.247769894280582e-05, 7.02874427520752e-05, 6.823154683032546e-05, 6.627737575948156e-05, 6.621013301778715e-05, 6.818906780278146e-05, 7.039830838692591e-05, 7.253190110343217e-05, 7.481641741533608e-05, 7.737695276987249e-05, 8.006168375579251e-05, 8.287090032485091e-05, 8.601989118408337e-05, 8.601149943331799e-05, 8.284626184079652e-05, 8.002899673195371e-05, 7.741141518999584e-05, 7.480089327897152e-05, 7.250111325657686e-05, 7.029352425112159e-05, 6.813221015480357e-05, 6.62198178581566e-05, 6.624405555597751e-05, 6.821127920453261e-05, 7.027352271510854e-05, 7.249655243974909e-05, 7.484227387774593e-05, 7.731918062011421e-05, 8.004531413655737e-05, 8.294468058990392e-05, 8.602973622524823e-05, 8.605820874899099e-05, 8.288693705562035e-05, 8.003385174147199e-05, 7.736144309435245e-05, 7.486190050400398e-05, 7.250316333951877e-05, 7.025783195388162e-05, 6.819131335886006e-05, 6.613698064332733e-05, 2.334902994428943e-05, 2.3089779955352072e-05, 2.2867194322032274e-05, 2.2654250327040787e-05, 2.24420589097621e-05, 2.2204407283396363e-05, 2.202103792971822e-05, 2.1772442212756655e-05, 2.1611819454583376e-05, 2.15673712839191e-05, 2.178051351765104e-05, 2.200683279009929e-05, 2.2217207672828798e-05, 2.2413498482930745e-05, 2.263675056841937e-05, 2.28839411522427e-05, 2.3079603545523137e-05, 2.331394948374215e-05, 2.332529176326199e-05, 2.311514095289536e-05, 2.293505703867007e-05, 2.263514524920676e-05, 2.2446356759140803e-05, 2.2216228604148275e-05, 2.2021672127041704e-05, 2.178221912190319e-05, 2.158524238715302e-05, 2.157750166116563e-05, 2.1803789567624635e-05, 2.200915414532067e-05, 2.222409581247468e-05, 2.243841214013405e-05, 2.2645030355772415e-05, 2.2853807504310942e-05, 2.309402367151253e-05, 2.3344236674728368e-05, 2.3348467975687502e-05, 2.3084825151232472e-05, 2.2861088760085822e-05, 2.261947917784298e-05, 2.24178719751886e-05, 2.2220888624852824e-05, 2.199790390203512e-05, 2.1797281268495692e-05, 2.1565797648875242e-05, 2.1568702563507148e-05, 2.1784258341370977e-05, 2.1994823392559054e-05, 2.223384815897198e-05, 2.242344633269043e-05, 2.263884812111769e-05, 2.286698550359004e-05, 2.3079300479124154e-05, 2.334760233007934e-05, 2.3322049788913553e-05, 2.3091885182495414e-05, 2.289091126173715e-05, 2.2665065606558442e-05, 2.24075245963905e-05, 2.221624483377646e-05, 2.198532679022869e-05, 2.180409032896561e-05, 2.1594714763174294e-05, 2.1598483415395152e-05, 2.1781315037182783e-05, 2.1993155509056286e-05, 2.2200747036183687e-05, 2.243093324548611e-05, 2.2618969435390364e-05, 2.2860988824144458e-05, 2.308902752960515e-05, 2.3349224577554042e-05, 2.3339744016703727e-05, 2.310957868998933e-05, 2.2882144965327962e-05, 2.264436428219414e-05, 2.2412945056781416e-05, 2.220164055905988e-05, 2.1972017261376016e-05, 2.180699687717492e-05, 2.157473544690644e-05, 2.1581750125177223e-05, 2.1789521962631636e-05, 2.200738253999908e-05, 2.21898319027474e-05, 2.2395857096290285e-05, 2.264833102644313e-05, 2.2877086149190623e-05, 2.3102725289221622e-05, 2.3325475210637064e-05, 2.357624857025745e-05, 2.3808644620812102e-05, 2.4059950492234325e-05, 2.431973516284907e-05, 2.4560233688166266e-05, 2.4855593821126953e-05, 2.5120507866818153e-05, 2.540193281253009e-05, 2.54049305588321e-05, 2.509690846143751e-05, 2.4850861944455414e-05, 2.4568537302886444e-05, 2.429131487239315e-05, 2.404782793351554e-05, 2.3781971400271163e-05, 2.3567515985357902e-05, 2.332655299374991e-05, 2.3101814030180663e-05, 2.2860052188523317e-05, 2.2639861764047933e-05, 2.2408254178750347e-05, 2.2194232960792944e-05, 2.1993234001434895e-05, 2.179605163399829e-05, 2.1577642228912748e-05, 2.1565966266985714e-05, 2.178942350413541e-05, 2.1987875561396526e-05, 2.2205118437544262e-05, 2.244717494304578e-05, 2.2662935757352994e-05, 2.2869057618916543e-05, 2.309816261010418e-05, 2.3333756193063565e-05, 2.354851150229106e-05, 2.3823184017908254e-05, 2.4086478009675742e-05, 2.4319230901548673e-05, 2.4554471405592092e-05, 2.4841873957800133e-05, 2.5103631644732964e-05, 2.537288919613255e-05, 2.5386589605561464e-05, 2.5117765676932197e-05, 2.4828308391444177e-05, 2.456456336745782e-05, 2.432643374275534e-05, 2.4053392713036517e-05, 2.380241880960099e-05, 2.3584231021896664e-05, 2.331345667143467e-05, 2.311090198357587e-05, 2.287079196720578e-05, 2.2635504873607936e-05, 2.2451323933095444e-05, 2.2216000507538387e-05, 2.200440820659451e-05, 2.1801652969298914e-05, 2.157685890086693e-05, 2.1594900958952314e-05, 2.1769985844139895e-05, 2.198871263095823e-05, 2.2232804833594565e-05, 2.244104434189173e-05, 2.263529972278819e-05, 2.2862023970861716e-05, 2.309962993194674e-05, 2.3324449152970935e-05, 2.357297335073368e-05, 2.380025747732436e-05, 2.4063881165216175e-05, 2.4298539521549436e-05, 2.4584049979652372e-05, 2.484695936204591e-05, 2.510328784854767e-05, 2.5384709104591776e-05]
  out "angle phi":dbl[](array[numeric])=[90.00000221383264, 90.0000022256005, 90.00000223110156, 90.00000225580085, 90.00000226671646, 90.00000226131833, 90.00000227070977, 90.00000226434369, 90.00000228023627, 90.00000233265473, 90.00000229002634, 90.00000229407333, 90.0000023309754, 90.0000023160516, 90.00000233721477, 90.00000234122754, 90.00000234993932, 90.00000236728485, 90.00000238008987, 90.00000238922836, 90.00000238920474, 90.0000024086022, 90.0000024268278, 90.0000024322376, 90.00000243387338, 90.00000245122095, 90.00000247430849, 90.0000024942776, 90.00000247041729, 90.00000252201198, 90.00000253492003, 90.00000250644153, 90.00000252018492, 90.00000254071509, 90.0000025351148, 90.00000256787594, 90.00000256066127, 90.0000025243121, 90.00000259161541, 90.00000257857656, 90.00000260669749, 90.00000262570298, 90.00000262759478, 90.00000263682297, 90.00000267335835, 90.00000266146074, 90.00000272577225, 90.0000027203965, 90.00000275067669, 90.00000271319568, 90.00000272772205, 90.00000278050801, 90.00000277973393, 90.00000275050388, 90.00000276690716, 90.00000279492691, 90.00000278411622, 90.00000280359946, 90.00000282658604, 90.00000292561111, 90.00000285676819, 90.00000286626174, 90.00000288154331, 90.00000288854002, 90.00000295153288, 90.00000298303279, 90.00000291889766, 90.0000029604279, 90.00000299449641, 90.00000295632529, 90.00000299997119, 90.00000301384748, 90.00000301074698, 90.00000300302337, 90.0000030380051, 90.00000305848958, 90.00000303596195, 90.0000031358259, 90.0000031307147, 90.00000309813315, 90.00000315628068, 90.00000316291062, 90.00000318393535, 90.00000325573812, 90.00000324156967, 90.00000324468272, 90.00000327725478, 90.0000032210905, 90.00000328199086, 90.00000331590621, 90.00000332995815, 90.00000335562984, 90.00000341601309, 90.00000337926781, 90.00000336550599, 90.00000346337256, 90.00000345538139, 90.00000346507228, 90.00000348493907, 90.00000349700579, 90.00000355161468, 90.00000356797656, 90.00000360330763, 90.00000364719227, 90.00000364946894, 90.00000365667916, 90.00000373117987, 90.00000368272337, 90.00000372483784, 90.00000377231459, 90.00000379156408, 90.0000037746972, 90.0000038235959, 90.00000382007386, 90.00000385335103, 90.00000390787153, 90.00000391865805, 90.00000215005386, 90.00000212431381, 90.00000221601773, 90.00000224028757, 90.0000023536035, 90.00000239873448, 90.0000024423346, 90.00000249725653, 90.00000255666336, 90.00000260383064, 90.00000262440022, 90.0000027512309, 90.00000280433122, 90.00000292172584, 90.000002946019, 90.0000030136881, 90.00000311332707, 90.000003184078, 90.00000329646099, 90.00000332352725, 90.00000346638942, 90.00000353942, 90.00000370589102, 90.00000376092379, 90.00000359213864, 90.00000356614821, 90.0000035064257, 90.00000338988667, 90.00000332711, 90.0000032055856, 90.00000309544198, 90.00000303315551, 90.00000291206813, 90.00000290654897, 90.00000275321598, 90.00000276822416, 90.00000268525356, 90.00000260696712, 90.00000248271473, 90.00000245147702, 90.00000238895242, 90.00000244204192, 90.00000235183315, 90.00000226156432, 90.00000222433795, 90.00000220152205, 90.00000373213392, 90.00000359706863, 90.00000347322393, 90.00000343289713, 90.0000033369412, 90.00000318916571, 90.00000314479519, 90.00000305054978, 90.00000303100869, 90.00000292742637, 90.00000287438584, 90.00000279006812, 90.00000276695417, 90.00000265278337, 90.00000258649426, 90.0000025369513, 90.00000249979239, 90.00000246199211, 90.00000238767463, 90.0000023169844, 90.00000227939286, 90.00000223956364, 90.00000220181514, 90.0000183314101, 90.00001705935497, 90.00001602656779, 90.00001463333088, 90.00001403763284, 90.00001321556957, 90.00001258883205, 90.00001177626885, 90.00001118534632, 90.00001089759886, 90.00001037944729, 90.00001002608141, 90.0000095416321, 90.0000090063545, 90.00000887580737, 90.00000841768886, 90.00000818361302, 90.00000792132666, 90.00000770197465, 90.00000731202297, 90.00000726880059, 90.00000677418416, 90.00000683055941, 90.00000664831184, 90.00000648760721, 90.00000620619372, 90.00000607332866, 90.00000588824447, 90.00000575160728, 90.00000546726373, 90.00000547102667, 90.0000053435858, 90.00000535774939, 90.00000519676124, 90.0000050264666, 90.00000481444675, 90.00000488508616, 90.00000474858321, 90.00000458421457, 90.00000455889246, 90.0000044464891, 90.00000436023399, 90.00000428439118, 90.00000419168268, 90.0000041812775, 90.00000415200113, 90.00000389944866, 90.00000396914396, 90.00000382657643, 90.00000378782114, 90.00000375934776, 90.0000036555288, 90.00000358171161, 90.00000354045886, 90.00000355164826, 90.00000344088305, 90.00000340541555, 90.00000336814539, 90.000003327019, 90.00000325955591, 90.00000325197418, 90.00000320080466, 90.00000317882544, 90.00000311486215, 90.00000306616887, 90.0000030157558, 90.00000296821261, 90.00000293718918, 90.00000287753875, 90.00000286866037, 90.00000283854354, 90.00000284180986, 90.00000278008538, 90.00000274911828, 90.00000272244252, 90.00000268022305, 90.00000264279252, 90.00000259931133, 90.00000257430172, 90.00000256696762, 90.00000258879302, 90.00000247991031, 90.00000253570103, 90.00000247271002, 90.00000240916877, 90.00000239714569, 90.00000233718657, 90.00000237713574, 90.0000023338208, 90.00000231139505, 90.00000230197462, 90.00000227284166, 90.00000222802043, 90.00000221491536, 90.00000223246074, 90.00000219671334, 90.00000215296762, 90.00000215379106, 90.00000212764144, 90.00000213960868, 90.00000204699634, 90.00000206700312, 90.0000020401068, 90.00000203092665, 90.0000019850645, 90.00000201787623, 90.00000196736912, 90.00000197969054, 90.00000193729983, 90.0000064455377, 90.00000689876984, 90.00000701445671, 90.0000073839775, 90.00000739338485, 90.00000763248991, 90.0000080337777, 90.00000825074547, 90.00000855598216, 90.00000886114705, 90.00000911599773, 90.00000899080092, 90.00000886065634, 90.00000854178762, 90.00000821243212, 90.00000785260654, 90.0000076916171, 90.00000759387778, 90.00000722601048, 90.00000706344892, 90.00000684367748, 90.00000672138441, 90.00000661518268, 90.00000659958643, 90.00000700470761, 90.00000721893923, 90.00000729952178, 90.00000771288848, 90.00000798590358, 90.00000826283289, 90.00000848483562, 90.00000889905652, 90.0000094314506, 90.00000934613422, 90.00000886373952, 90.00000853906752, 90.00000819466915, 90.00000801209448, 90.00000775420452, 90.00000755656471, 90.0000073064179, 90.00000705015812, 90.00000690444165, 90.00000658489084, 90.00000663956486, 90.00000671374389, 90.00000687701588, 90.00000721081288, 90.0000074037853, 90.0000076292883, 90.00000804894168, 90.00000829430599, 90.00000866094531, 90.00000876495892, 90.00000929848032, 90.00000911561087, 90.00000886170255, 90.00000850034512, 90.00000833213339, 90.00000791982636, 90.00000772083347, 90.00000746444195, 90.00000721071913, 90.00000704291374, 90.00000680236475, 90.00000663109091, 90.00000661214426, 90.0000068186445, 90.00000700150312, 90.00000719161005, 90.00000752334283, 90.000007714324, 90.00000794423451, 90.00000819737505, 90.00000857907544, 90.00000873828554, 90.00000916384036, 90.00000920829306, 90.00000884179838, 90.00000850194078, 90.00000817135377, 90.00000810464935, 90.0000076833781, 90.00000751779517, 90.00000727496003, 90.00000710914978, 90.0000068412403, 90.00000663573256, 90.00000655378165, 90.00000682189561, 90.0000070469416, 90.00000731287302, 90.00000742130047, 90.000007678278, 90.00000792789713, 90.00000841507887, 90.00000851320706, 90.00000873090052, 90.00000923579627, 90.00000913460246, 90.00000890373865, 90.0000085666794, 90.00000835451097, 90.00000796263305, 90.00000783426941, 90.00000739442669, 90.00000725545131, 90.00000700236467, 90.00000688357085, 90.00000656296147, 90.00000664698385, 90.00000681236796, 90.00000697915286, 90.00000717592287, 90.00000748178286, 90.0000077239191, 90.00000788552738, 90.00000818143702, 90.0000085051327, 90.00000882307911, 90.00000921782065, 90.00000924280937, 90.00000908295767, 90.00000861382428, 90.00000822424644, 90.00000806783994, 90.00000776490135, 90.000007491291, 90.00000718790092, 90.00000695076616, 90.00000685408814, 90.00000659604429, 90.00000664639694, 90.0000067538309, 90.00000700180739, 90.00000708361247, 90.00000746314193, 90.00000769692537, 90.00000800416257, 90.00000831539, 90.00000854157742, 90.00000886512407, 90.00000919782025, 90.00000926785812, 90.00000900484436, 90.00000871973124, 90.0000083061854, 90.00000799565115, 90.00000779456437, 90.00000758060635, 90.00000723567624, 90.00000706317637, 90.0000068531445, 90.0000066504335, 90.00000663012803, 90.00000684352959, 90.00000704555823, 90.00000726655705, 90.00000726187311, 90.00000776116788, 90.00000798191004, 90.0000081641092, 90.00000855320592, 90.00000892886423, 90.00000908780743, 90.00000937963452, 90.00000886858564, 90.00000838660853, 90.00000822442999, 90.00000815508854, 90.00000782325569, 90.00000744479283, 90.00000730743197, 90.00000711321182, 90.00000700904867, 90.00000664897514, 90.0000066988504, 90.00000685652765, 90.00000696247848, 90.000007165688, 90.00000745578913, 90.00000771828829, 90.00000791381, 90.00000817255598, 90.00000844756605, 90.00000889119792, 90.00000921963849, 90.0000039076624, 90.00000378808109, 90.00000384187811, 90.00000377376905, 90.00000364946425, 90.00000361455407, 90.00000355805176, 90.00000347057075, 90.00000346799942, 90.00000345570858, 90.00000335862457, 90.00000335687464, 90.00000323043662, 90.00000328655479, 90.00000332131731, 90.00000331156991, 90.00000339979154, 90.00000346061849, 90.00000342540436, 90.00000357939737, 90.00000358847007, 90.00000353191037, 90.00000374854378, 90.00000377580567, 90.0000038509765, 90.00000392322146, 90.00000389618184, 90.00000386647223, 90.00000382890877, 90.00000373914835, 90.00000358724046, 90.00000360894006, 90.00000356485323, 90.00000350129237, 90.00000346866366, 90.00000345655361, 90.00000335850201, 90.00000332783682, 90.00000326007452, 90.0000032475418, 90.00000334023473, 90.00000336802316, 90.00000339467125, 90.00000342475106, 90.00000352489732, 90.0000035252807, 90.00000360577799, 90.0000036506068, 90.00000371645694, 90.0000037141329, 90.00000382728835, 90.00000389974977, 90.00000391211204, 90.00000383716048, 90.00000374016213, 90.00000371004991, 90.00000362552835, 90.00000362583137, 90.00000353853167, 90.00000351794803, 90.00000341077022, 90.0000034675755, 90.0000033257015, 90.00000331549109, 90.00000325830733, 90.00000327320231, 90.00000331624331, 90.00000334312003, 90.00000336933435, 90.00000345939907, 90.00000350206346, 90.00000360197158, 90.00000362399612, 90.00000361719411, 90.00000368533104, 90.00000379088831, 90.00000385034029, 90.00000389609441, 90.00000394859224, 90.00000385783477, 90.00000370526533, 90.00000357272073, 90.00000367613698, 90.00000363113908, 90.00000347641544, 90.00000348738517, 90.0000034210721, 90.00000336018901, 90.00000330989553, 90.00000330171244, 90.00000330828016, 90.00000331635833, 90.00000329435949, 90.00000334691849, 90.00000341110055, 90.00000338959168, 90.00000344944485, 90.00000355653798, 90.00000355783054, 90.00000364162281, 90.00000380485929, 90.00000375280563, 90.00000379959431, 90.00000397288387, 90.0000038137583, 90.00000383665555, 90.00000375936743, 90.00000364885534, 90.00000367902673, 90.00000364310274, 90.00000358954834, 90.0000034456822, 90.00000346462042, 90.00000337286559, 90.00000336252295, 90.00000336364451, 90.00000325517917, 90.00000324836617, 90.00000331411157, 90.00000337324914, 90.00000339316375, 90.00000343396896, 90.00000345686284, 90.00000354632508, 90.00000356302431, 90.00000370438872, 90.00000370035846, 90.00000374109098, 90.00000389158646, 90.00000392812878, 90.00000393159861, 90.00000380196046, 90.00000379529754, 90.00000377520584, 90.00000367685442, 90.00000359035953, 90.00000356145307, 90.00000350751459, 90.00000340792931, 90.00000336092874, 90.00000338506129, 90.00000328003243, 90.00000322729271, 90.0000032177874, 90.00000326988398, 90.00000336478044, 90.00000346525056, 90.00000342414043, 90.00000350661203, 90.00000354071277, 90.00000362246148, 90.00000358339267, 90.00000367165214, 90.00000373645018, 90.0000038284634, 90.00000391908239, 90.0000038892564, 90.00000380358438, 90.00000379086474, 90.00000363144291, 90.00000362019394, 90.00000357881733, 90.00000354057529, 90.0000035335278, 90.0000034208554, 90.00000339606463, 90.00000332355151, 90.00000323640239, 90.0000032381953, 90.00000326670477, 90.00000331065971, 90.0000033626538, 90.00000338588978, 90.00000344944267, 90.0000035307059, 90.00000353820805, 90.00000358909466, 90.00000370347419, 90.00000371454404, 90.00000377322958, 90.0000037848119, 90.0000038748382, 90.00000391633858, 90.00000376525146, 90.00000375967923, 90.00000370559646, 90.00000360258015, 90.00000356059248, 90.00000354878273, 90.00000347850099, 90.00000343039581, 90.00000332159934, 90.00000334194057, 90.00000328603291, 90.0000032889953, 90.00000324879275, 90.00000323006586, 90.00000333868478, 90.0000033788128, 90.00000346832655, 90.00000354576511, 90.00000355464972, 90.00000359582874, 90.0000037057982, 90.00000365222232, 90.00000376504154, 90.0000037940161, 90.00000390195045, 90.00000386475399, 90.00000385671271, 90.00000375401684, 90.00000370830507, 90.00000365070906, 90.00000358081085, 90.00000356071499, 90.00000347332978, 90.00000340576848, 90.00000338633453, 90.00000332388458, 90.00000332080187, 90.00000324420515, 90.00000318493406, 90.00000331356047, 90.00000328643057, 90.00000335049177, 90.00000341456155, 90.00000350756267, 90.00000353317971, 90.0000035553474, 90.00000361272572, 90.0000036645181, 90.0000036536635, 90.0000037846599, 90.00000375826409, 90.00000384423478, 90.0000037868856, 90.0000037704425, 90.00000361026751, 90.00000368052844, 90.00000354085095, 90.0000035317311, 90.00000345560913, 90.00000346475395, 90.00000337847749, 90.00000330522614, 90.00000330420727, 90.0000032712757, 90.00000319646357, 90.00000323238767, 90.00000331550852, 90.0000033941132, 90.00000343214505, 90.00000344734372, 90.00000354836209, 90.00000358160514, 90.0000036271606, 90.00000364854003, 90.00000370584787, 90.00000375493086, 90.00000389980114, 90.00000516252781, 90.00000532058547, 90.0000054207514, 90.00000552596923, 90.00000564369688, 90.00000580191929, 90.00000596846097, 90.00000605060184, 90.00000641825852, 90.00000663383668, 90.00000660425432, 90.00000659337994, 90.00000647837874, 90.0000063923602, 90.00000592926106, 90.00000593645242, 90.0000058318221, 90.00000578157753, 90.00000562339685, 90.00000546069484, 90.00000526614663, 90.00000516972999, 90.00000501387669, 90.00000528368022, 90.00000542409721, 90.00000555512548, 90.00000563542832, 90.00000563513464, 90.00000595530643, 90.0000062738552, 90.00000631026734, 90.00000639995257, 90.0000063283971, 90.00000671844496, 90.00000667563901, 90.00000625142188, 90.00000610966323, 90.00000597008149, 90.00000582792319, 90.00000581293793, 90.00000547342005, 90.00000539867082, 90.00000537733354, 90.00000512344475, 90.00000526548996, 90.00000531130274, 90.00000542216699, 90.00000547116146, 90.00000567236224, 90.00000572993638, 90.0000059551549, 90.00000598937051, 90.00000620315116, 90.00000646615447, 90.00000666720997, 90.00000665383196, 90.0000064193793, 90.00000616201118, 90.00000611994041, 90.00000601457072, 90.00000571549624, 90.00000569080264, 90.0000055057434, 90.0000054591407, 90.00000523966848, 90.00000522994418, 90.00000522670787, 90.00000536166745, 90.00000556903444, 90.00000553950771, 90.00000569137262, 90.00000585227951, 90.00000593924814, 90.0000061134149, 90.0000060809751, 90.00000660248097, 90.00000678049055, 90.00000653940862, 90.00000662768429, 90.00000611215046, 90.00000630160251, 90.0000059617339, 90.00000575276371, 90.00000555172674, 90.00000557688749, 90.00000551074316, 90.00000544203779, 90.0000053023678, 90.00000522500982, 90.00000547859116, 90.00000551362471, 90.00000557717273, 90.00000569965096, 90.00000583280234, 90.00000587317096, 90.00000612208042, 90.00000632688575, 90.00000644228177, 90.00000640788085, 90.00000654831594, 90.00000664945183, 90.00000646921355, 90.00000624908718, 90.00000604191864, 90.00000563832772, 90.00000570308936, 90.00000545438573, 90.0000052900222, 90.00000531627121, 90.00000535881249, 90.00000513681258, 90.0000052819119, 90.00000532376275, 90.00000553712127, 90.00000566888136, 90.00000575831851, 90.0000059493513, 90.00000597085517, 90.0000062598211, 90.00000650628337, 90.00000669513594, 90.00000649658814, 90.000006446969, 90.0000063363767, 90.00000596061138, 90.00000598027871, 90.00000591217724, 90.00000578641811, 90.0000055866904, 90.00000545697624, 90.00000533079913, 90.00000520487616, 90.00000514973792, 90.00000523955944, 90.00000542655508, 90.00000559441814, 90.00000569980354, 90.0000057501006, 90.00000584070122, 90.00000607206678, 90.00000636117046, 90.00000645162089, 90.00000661678764, 90.00000664399535, 90.00000642271277, 90.0000062734471, 90.00000597144094, 90.00000598642885, 90.00000583132231, 90.0000056841372, 90.00000570969249, 90.00000530969196, 90.00000536830336, 90.00000538913126, 90.00000527399094, 90.00000530726098, 90.00000535110632, 90.00000551871787, 90.00000542039753, 90.00000608415444, 90.00000601433499, 90.00000614646586, 90.00000644006407, 90.0000064016495, 90.00000661898021, 90.00000663289833, 90.00000641984238, 90.00000629773153, 90.00000611237954, 90.00000609066005, 90.0000057962503, 90.00000568881859, 90.0000053968642, 90.00000540875544, 90.00000538203186, 90.00000512613967, 90.0000050945145, 90.00000524550909, 90.00000537803096, 90.00000543068914, 90.00000563330171, 90.00000576280985, 90.00000594481055, 90.0000062609048, 90.00000610822917, 90.0000063170699, 90.00000659877277, 90.00000519381366, 90.00000524225167, 90.00000491036573, 90.00000493097205, 90.00000486312416, 90.00000483637771, 90.0000044742785, 90.00000446038449, 90.00000438425995, 90.00000431782827, 90.0000042245271, 90.0000043013305, 90.00000429323953, 90.0000044034864, 90.00000444109729, 90.00000457679586, 90.00000474328498, 90.00000474482214, 90.00000472391028, 90.00000493413803, 90.00000496455226, 90.0000050947543, 90.00000517627461, 90.00000500975352, 90.00000500587024, 90.0000048591331, 90.00000482276097, 90.0000047766402, 90.00000470375257, 90.00000457979604, 90.00000438519255, 90.00000440856743, 90.00000422781308, 90.00000420738088, 90.00000428887171, 90.00000444917434, 90.00000451439715, 90.0000045330082, 90.00000469659865, 90.00000477704486, 90.00000479882888, 90.00000493402955, 90.00000501224201, 90.00000525299595, 90.00000518091079, 90.00000505965947, 90.00000491418868, 90.00000486833574, 90.00000486868012, 90.00000468498993, 90.00000454389269, 90.00000446321839, 90.00000454259758, 90.0000043180399, 90.00000423950218, 90.00000422069381, 90.00000420642813, 90.00000434657606, 90.00000454083587, 90.00000459519015, 90.00000457882506, 90.00000482436735, 90.00000485591832, 90.00000494916466, 90.000005153346, 90.0000051170136, 90.00000524135349, 90.00000501287134, 90.00000495308592, 90.00000480216072, 90.00000486666373, 90.00000456355967, 90.00000454682204, 90.00000442899201, 90.00000441230448, 90.00000434129004, 90.00000426360276, 90.00000423797962, 90.00000439689502, 90.00000441886513, 90.00000452239968, 90.00000445067496, 90.00000461551883, 90.00000476055061, 90.00000477518525, 90.00000493886543, 90.00000503714718, 90.00000514078718, 90.00000515188111, 90.00000503730061, 90.0000050588853, 90.00000482334764, 90.0000047588689, 90.0000046900712, 90.00000456934445, 90.00000453581569, 90.00000442143539, 90.00000436829227, 90.0000043203806, 90.0000042295195, 90.00000426360133, 90.00000436973195, 90.00000445484343, 90.00000450416654, 90.00000462189418, 90.00000478817506, 90.00000488751265, 90.00000494431566, 90.0000050657048, 90.00000525846151, 90.00000508704375, 90.00000493800886, 90.00000487813823, 90.00000472426629, 90.00000468270999, 90.00000459457522, 90.00000455253665, 90.0000044136151, 90.00000430987338, 90.0000042469593, 90.00000424103601, 90.00000418754084, 90.00000424307822, 90.00000436250797, 90.00000442189878, 90.00000451232097, 90.00000457468879, 90.00000463058652, 90.00000482076724, 90.00000486141228, 90.00000496372826, 90.00000512230262, 90.00000501713373, 90.00000499588361, 90.00000482738177, 90.0000047683929, 90.00000468768317, 90.00000459658145, 90.00000453741634, 90.00000441118458, 90.00000440209627, 90.00000424141541, 90.00000425395513, 90.00000415385226, 90.0000042174423, 90.00000435916375, 90.00000438607144, 90.00000453932472, 90.00000463564407, 90.00000459938673, 90.00000472946114, 90.00000488315672, 90.00000500242973, 90.00000506443487, 90.0000050298586, 90.00000481628987, 90.00000483177261, 90.00000480550949, 90.00000449988111, 90.00000456976102, 90.00000449650177, 90.00000431303806, 90.00000429528053, 90.00000432875466, 90.00000417613327, 90.00000426063824, 90.00000424802948, 90.00000432830105, 90.000004387141, 90.00000446938085, 90.00000458710085, 90.00000473012338, 90.00000481381628, 90.00000484318794, 90.00000496484884, 90.00000504975291, 90.00000511997614, 90.00000506497452, 90.00000489899304, 90.00000476416656, 90.00000466991533, 90.00000459685369, 90.00000452452298, 90.00000443000765, 90.00000430929927, 90.00000428055017, 90.00000419941738, 90.00000410696563, 90.0000042865699, 90.00000430395507, 90.00000442108293, 90.00000450327624, 90.00000459469535, 90.00000468443882, 90.00000473939728, 90.00000481969404, 90.00000503483516, 90.00000498412417, 90.00000515412891, 90.00000482986194, 90.00000493948741, 90.00000503097708, 90.00000501494254, 90.00000484546226, 90.00000477231453, 90.00000473313216, 90.00000462773941, 90.00000452035276, 90.0000044061971, 90.0000043622762, 90.00000433468688, 90.00000418615592, 90.00000408907607, 90.00000407631622, 90.0000040176868, 90.00000402736606, 90.00000403225023, 90.0000039735438, 90.000004183027, 90.00000424908818, 90.00000438529946, 90.00000442071774, 90.00000446404134, 90.00000450093357, 90.00000466210777, 90.00000465966306, 90.00000483279493, 90.0000050042937, 90.00000511322652, 90.00000506547906, 90.00000492066218, 90.00000484167093, 90.00000475833092, 90.00000461737498, 90.00000460064014, 90.00000446197535, 90.0000044634108, 90.00000434718226, 90.00000427772757, 90.00000422404142, 90.00000408332568, 90.00000407279595, 90.00000389789649, 90.00000394482284, 90.00000390641736, 90.00000413267932, 90.00000414370635, 90.00000417881407, 90.00000439058273, 90.00000436997155, 90.00000448996974, 90.00000461106099, 90.0000046389518, 90.00000486843216, 90.00000484099668, 90.0000050060663, 90.0000050563573, 90.00000501183267, 90.00000491172217, 90.000004857775, 90.00000471675648, 90.0000047357326, 90.00000461895333, 90.00000451809221, 90.00000438350986, 90.00000429207495, 90.00000424200918, 90.00000417712528, 90.00000410291166, 90.0000040429987, 90.0000039774593, 90.00000397512848, 90.00000403342645, 90.00000405550034, 90.00000415798544, 90.00000422915336, 90.00000438830159, 90.00000441463854, 90.0000044753936, 90.0000045429899, 90.0000047062372, 90.00000480591669, 90.00000479794045, 90.00000493327002, 90.00000508228712, 90.00000504690367, 90.00000496889729, 90.00000487321608, 90.00000471877583, 90.00000464326219, 90.00000451059898, 90.00000453074276, 90.0000045169628, 90.00000431722715, 90.00000427711916, 90.00000417582821, 90.00000408570284, 90.0000040121987, 90.0000039487906, 90.00000394808912, 90.00000397794422, 90.00000412577293, 90.00000416972708, 90.00000419938164, 90.00000426678719, 90.00000428864323, 90.00000445690766, 90.00000452904547, 90.00000469340404, 90.0000047081097, 90.00000484352601, 90.00000493655837, 90.00000509318204, 90.00000510510912, 90.00000491571333, 90.00000484752911, 90.0000047645675, 90.00000465401848, 90.00000461008756, 90.00000451007227, 90.00000431052034, 90.00000429332434, 90.00000422528377, 90.00000414309773, 90.00000409716168, 90.00000401319534, 90.00000396908848, 90.00000410904883, 90.00000399513138, 90.00000397113936, 90.00000395188039, 90.00000400871781, 90.0000040737264, 90.00000405703257, 90.00000406937167, 90.00000400544616, 90.00000390936762, 90.00000414444503, 90.0000040529713, 90.00000410353314, 90.00000403722491, 90.00000396411657, 90.00000393680105, 90.00000408260819, 90.0000041418423, 90.00000416548451, 90.0000039402585, 90.00000395271104, 90.0000039670439, 90.00000400044753, 90.00000407005886, 90.00000406912258, 90.00000406428396, 90.00000396003433, 90.00000409114715, 90.00000404600523, 90.0000039925062, 90.00000393485637, 90.00000383275845, 90.00000379225543, 90.00000367766242, 90.00000361461817, 90.00000359312878, 90.00000349114927, 90.00000352224065, 90.00000346043615, 90.00000341323239, 90.00000330943048, 90.00000332977474, 90.00000326277288, 90.00000323628453, 90.00000320827124, 90.00000316555494, 90.00000308847648, 90.0000030451923, 90.00000298810302, 90.00000297243328, 90.0000029234551, 90.00000282337449, 90.0000028250293, 90.00000286924964, 90.00000278303499, 90.0000028223736, 90.00000274616285, 90.00000269148555, 90.00000266896669, 90.00000265559233, 90.00000260929507, 90.00000256414222, 90.00000258002162, 90.0000025308197, 90.00000249069954, 90.00000249108874, 90.00000242675647, 90.00000240747384, 90.00000238366341, 90.00000237462126, 90.00000235135259, 90.00000231545553, 90.00000230460853, 90.00000232880578, 90.00000233615648, 90.00000236752183, 90.00000239204782, 90.00000239861501, 90.00000246816694, 90.00000241633502, 90.00000248417896, 90.00000250190551, 90.00000255562162, 90.0000025623701, 90.00000261483767, 90.00000266113821, 90.0000026513031, 90.00000266965233, 90.00000268582218, 90.00000274940405, 90.00000274799322, 90.00000279237939, 90.0000028570918, 90.0000028627165, 90.00000290634686, 90.00000290850286, 90.00000290097098, 90.00000294612585, 90.00000312129605, 90.00000307239746, 90.00000319132911, 90.00000321877216, 90.0000032357018, 90.00000323397765, 90.00000327434626, 90.00000332986215, 90.00000339744831, 90.00000342748076, 90.00000356855685, 90.0000034389792, 90.00000352653902, 90.00000372811914, 90.00000369919042, 90.00000372134326, 90.00000385802716, 90.00000370401837, 90.0000040862578, 90.00000403313904, 90.00000397260747, 90.00000421504615, 90.00000407441883, 90.00000399003639, 90.00000389130612, 90.00000372026754, 90.0000038260444, 90.00000377945169, 90.00000352228311, 90.0000037245212, 90.00000359044672, 90.00000351040177, 90.00000345198617, 90.000003489126, 90.00000336432127, 90.00000330362269, 90.00000331913058, 90.0000031974974, 90.00000322798914, 90.00000312408129, 90.00000318233784, 90.00000308813587, 90.00000310368435, 90.00000295484924, 90.00000296499944, 90.00000298338004, 90.00000292690918, 90.00000271037663, 90.00000285341227, 90.00000283584417, 90.00000276215437, 90.00000268124468, 90.00000270366439, 90.00000264011673, 90.00000262557168, 90.00000263083962, 90.00000257617558, 90.00000254124593, 90.00000256454868, 90.00000252295297, 90.00000251767942, 90.00000246738462, 90.00000230186059, 90.0000023973634, 90.00000233593492, 90.0000023305669, 90.00000229177935, 90.00000232158926, 90.000002287486, 90.00000238923364, 90.00000236419523, 90.00000239676827, 90.000002399122, 90.0000024740922, 90.00000248410043, 90.00000247941327, 90.00000249190079, 90.00000253343994, 90.00000251724467, 90.00000259424998, 90.00000258406665, 90.000002659701, 90.0000027035948, 90.00000271082071, 90.00000275939308, 90.00000279882651, 90.00000282701977, 90.00000287120446, 90.00000289637501, 90.00000293907956, 90.0000029867689, 90.00000302359527, 90.0000030690213, 90.00000310402572, 90.0000030641358, 90.00000318812428, 90.00000321950446, 90.00000326187653, 90.0000033587766, 90.0000033508994, 90.00000338132519, 90.00000345046911, 90.00000352312237, 90.00000360396758, 90.00000362300297, 90.00000365529884, 90.00000370320977, 90.00000375237956, 90.00000386364763, 90.00000389659822, 90.00000398690133, 90.00000412421393, 90.0000040637544, 90.00000232363972, 90.0000023396656, 90.00000232103083, 90.00000242283627, 90.0000024380887, 90.00000245228463, 90.00000246740537, 90.00000252585846, 90.00000254777929, 90.00000260524097, 90.00000260568046, 90.00000261753814, 90.00000264402625, 90.00000266130507, 90.0000027442742, 90.00000274571885, 90.00000277522591, 90.00000279963976, 90.00000290094799, 90.000002896248, 90.0000029016262, 90.000002925329, 90.00000298621313, 90.0000030239281, 90.0000030468438, 90.00000307727987, 90.00000314035958, 90.00000316079927, 90.00000323152224, 90.00000321308568, 90.00000321118392, 90.00000315650723, 90.00000307934064, 90.0000030294854, 90.00000301731248, 90.00000298297101, 90.00000292954621, 90.00000291675629, 90.00000285394563, 90.00000281773035, 90.00000283292206, 90.00000271536669, 90.00000268689288, 90.00000269471965, 90.00000264145088, 90.0000026726804, 90.00000260464697, 90.00000256141928, 90.00000260725305, 90.00000249902787, 90.00000248955573, 90.0000025331339, 90.00000246299642, 90.00000241355286, 90.00000243480771, 90.00000239547407, 90.00000236362231, 90.00000238210275, 90.00000233841955, 90.00000230855596, 90.00000237209498, 90.00000240517211, 90.00000243312475, 90.0000024584757, 90.00000248000705, 90.0000025054394, 90.00000252250484, 90.00000256431377, 90.00000260193329, 90.0000025905338, 90.00000263876149, 90.00000269684787, 90.00000273369646, 90.00000273897511, 90.00000274306979, 90.0000027786543, 90.00000287231781, 90.00000289285988, 90.00000290861958, 90.00000295816217, 90.00000295926174, 90.00000302864082, 90.00000297708524, 90.00000310763507, 90.00000312944717, 90.00000317861092, 90.00000321245463, 90.00000319777689, 90.0000032046036, 90.00000313370371, 90.00000311318335, 90.00000304612098, 90.00000302785116, 90.00000299238648, 90.00000294748396, 90.00000285931172, 90.00000287165918, 90.00000281693931, 90.00000283693994, 90.00000272365484, 90.00000272867128, 90.00000269677419, 90.00000265755797, 90.0000026600558, 90.00000258850208, 90.0000025525751, 90.00000256772601, 90.00000251201598, 90.0000024834308, 90.00000246690803, 90.00000249653709, 90.0000024777763, 90.00000239835211, 90.00000238818168, 90.0000023514874, 90.00000235295595, 90.00000233893354, 90.00000228617758, 90.00000236181668, 90.00000238249191, 90.00000241336046, 90.00000240129741, 90.00000245304388, 90.00000251671665, 90.00000254701735, 90.0000026145247, 90.00000257919211, 90.00000256640948, 90.00000262613752, 90.00000270526816, 90.0000027119388, 90.00000272731788, 90.00000278269482, 90.00000281325147, 90.00000280451809, 90.00000284785244, 90.00000282144856, 90.00000291981915, 90.00000301348209, 90.00000300109188, 90.00000309187402, 90.00000306212057, 90.00000309823606, 90.00000318602932, 90.00000322448464, 90.00000325639606, 90.00000320618797, 90.00000306822929, 90.00000309218147, 90.00000301503252, 90.00000299612353, 90.00000295481914, 90.00000294162201, 90.00000291696938, 90.0000028635107, 90.00000281833398, 90.00000282271115, 90.00000273309027, 90.00000271257306, 90.00000271400366, 90.0000027262216, 90.00000262223564, 90.00000263519729, 90.00000263377476, 90.00000259080305, 90.00000253027896, 90.00000248711292, 90.00000249913664, 90.00000235966839, 90.00000242941572, 90.00000245629447, 90.0000023391717, 90.00000234117744, 90.00000232070667, 90.00000231788245, 90.00000238928924, 90.00000240269955, 90.00000241051114, 90.00000244356085, 90.00000245793358, 90.00000248593885, 90.00000250912001, 90.00000255170373, 90.00000257302209, 90.00000259667492, 90.00000260252996, 90.00000267378769, 90.00000265639007, 90.00000267823732, 90.00000270357515, 90.00000277768844, 90.000002837959, 90.00000277061791, 90.00000285230529, 90.00000297518358, 90.00000295000224, 90.00000297389396, 90.0000030370566, 90.00000307069222, 90.00000303821429, 90.00000316206702, 90.00000313286152, 90.0000032170047, 90.00000319176576, 90.0000032385153, 90.00000313138264, 90.00000307828812, 90.00000308719106, 90.00000298371661, 90.0000029536027, 90.00000294388725, 90.00000290850436, 90.00000288229437, 90.00000279351754, 90.00000279053363, 90.00000277461021, 90.00000272918209, 90.00000269924783, 90.0000026543533, 90.00000264470928, 90.0000026102642, 90.00000255524073, 90.0000025568851, 90.00000250382641, 90.00000250735266, 90.00000247987617, 90.00000247126921, 90.00000243113949, 90.00000242032274, 90.00000241379163, 90.00000235211074, 90.00000233403932, 90.00000233293632, 90.00000235145589, 90.00000243271575, 90.00000239799245, 90.0000024340834, 90.00000239703415, 90.00000248360939, 90.00000251705218, 90.00000252287026, 90.0000025498819, 90.00000264071683, 90.00000258772295, 90.000002679077, 90.00000270753205, 90.00000269089556, 90.00000268613195, 90.00000277453228, 90.00000273491398, 90.00000283242558, 90.00000285954292, 90.00000289063705, 90.00000291295018, 90.00000298998678, 90.00000295580885, 90.0000030437898, 90.00000309939969, 90.00000314323258, 90.000003238375, 90.00000318294583, 90.00000321342792, 90.00000326438483, 90.00000317208091, 90.00000315722954, 90.00000305170173, 90.00000306757197, 90.00000299480129, 90.00000294808153, 90.0000028920633, 90.00000286459336, 90.00000281795384, 90.00000279418431, 90.0000027803915, 90.00000274267306, 90.00000267736053, 90.00000269548725, 90.00000264712277, 90.00000265007074, 90.00000257375687, 90.00000252887007, 90.00000254461403, 90.0000025188116, 90.00000250632456, 90.00000242817413, 90.0000023993936, 90.00000240730992, 90.00000239301379, 90.00000234052408, 90.00000236618524, 90.00000219800906, 90.00000222770684, 90.00000224475957, 90.00000225845974, 90.00000230820393, 90.00000235537973, 90.00000234544302, 90.00000237299282, 90.00000236524333, 90.00000238153007, 90.0000023589516, 90.0000023480055, 90.00000234618592, 90.0000022985352, 90.00000226666326, 90.0000022107465, 90.00000223939219, 90.00000219102765, 90.00000219671489, 90.00000223940982, 90.00000225155276, 90.00000228609183, 90.00000228625527, 90.00000231582527, 90.00000229861631, 90.00000236645522, 90.00000238116259, 90.00000238093384, 90.0000023323569, 90.00000234539712, 90.00000229861911, 90.00000229371074, 90.00000222818996, 90.00000224459139, 90.00000221775586, 90.00000221385356, 90.00000220308252, 90.0000022237435, 90.00000223117111, 90.0000022824665, 90.00000227433492, 90.00000231237242, 90.00000235430412, 90.00000234061373, 90.0000023873766, 90.00000239928525, 90.00000236743217, 90.00000233275308, 90.00000229711672, 90.00000224389056, 90.00000227110466, 90.00000222367719, 90.00000221219699, 90.00000218234325, 90.00000214727606, 90.00000221168358, 90.0000022356185, 90.00000226880474, 90.00000227411633, 90.00000226672927, 90.00000234345278, 90.0000023600005, 90.00000238959429, 90.00000235774236, 90.00000234978783, 90.00000232863904, 90.00000232990313, 90.00000226403472, 90.00000226568768, 90.0000022689702, 90.00000219890244, 90.00000221890743, 90.0000022168294, 90.0000022188435, 90.00000222454702, 90.00000224875882, 90.00000230501013, 90.00000231908385, 90.00000230667985, 90.00000235179512, 90.00000234677607, 90.00000683388298, 90.00000696121053, 90.00000703525285, 90.00000744321822, 90.00000766722107, 90.0000079129653, 90.00000804050966, 90.0000082633623, 90.00000881978622, 90.00000890143055, 90.00000856813301, 90.00000816804568, 90.00000792693426, 90.00000763216839, 90.00000727242582, 90.00000728376727, 90.00000695268508, 90.00000669080801, 90.00000675034744, 90.00000691930171, 90.00000722059062, 90.0000076832491, 90.00000767317289, 90.00000794612227, 90.00000814648297, 90.00000846315177, 90.00000884752932, 90.00000887937908, 90.00000871965173, 90.00000815740604, 90.00000789611128, 90.0000075027415, 90.00000740488619, 90.00000722707576, 90.00000712489697, 90.00000677130797, 90.00000673356308, 90.00000698630782, 90.00000714968324, 90.00000744975887, 90.00000766307035, 90.00000788646253, 90.00000806369397, 90.0000084646854, 90.00000873053352, 90.00000872931484, 90.00000850541345, 90.0000082743666, 90.00000800486396, 90.00000763204838, 90.00000749146322, 90.0000072997434, 90.00000702381924, 90.00000681261638, 90.00000651193508, 90.00000698275385, 90.00000725005663, 90.00000729798116, 90.00000789714082, 90.00000791311403, 90.00000806192912, 90.00000852482486, 90.00000880319207, 90.00000879918878, 90.00000856767, 90.00000808693652, 90.00000790228047, 90.00000783575437, 90.0000075298733, 90.00000736249419, 90.00000706657268, 90.00000677952833, 90.00000678183092, 90.00000673242496, 90.00000731935235, 90.00000750880655, 90.00000773643103, 90.00000791505722, 90.00000812687337, 90.00000840795074, 90.00000897571753, 90.00000883919768, 90.00000850633458, 90.00000818742697, 90.00000791176066, 90.00000765058323, 90.00000738880337, 90.00000720235704, 90.00000698875496, 90.00000679875505, 90.00000664240646, 90.00000700332842, 90.00000694820656, 90.00000732663628, 90.00000769155797, 90.00000797877667, 90.00000840335356, 90.0000085212489, 90.00000880365744, 90.00000870387902, 90.00000857816009, 90.00000814792404, 90.00000804408752, 90.00000763687333, 90.00000748060872, 90.00000705646208, 90.00000701774364, 90.00000681742098, 90.0000068023519, 90.0000069317653, 90.00000712695847, 90.00000744992214, 90.00000768623332, 90.00000784598726, 90.00000822935887, 90.00000846810772, 90.00000910151172, 90.00000885117423, 90.0000084018211, 90.00000832266865, 90.00000799576958, 90.00000764358363, 90.00000737894688, 90.00000723464615, 90.00000699695642, 90.00000682975511, 90.00000665261173, 90.00000668183112, 90.00000727687377, 90.00000741131277, 90.00000780309881, 90.0000075358242, 90.00000811587795, 90.0000085080251, 90.00000900374353, 90.00000883997629, 90.0000084753579, 90.00000813548405, 90.00000788034482, 90.00000752783752, 90.00000745065654, 90.00000713286198, 90.0000070411968, 90.00000677830884, 90.00000677604865, 90.00000699365137, 90.00000715225686, 90.00000743718674, 90.00000752683339, 90.0000079113584, 90.00000812173215, 90.00000841861547, 90.0000088295581, 90.0000089230816, 90.0000084516784, 90.0000081719312, 90.00000786244694, 90.00000758604942, 90.00000739681735, 90.00000719093356, 90.00000689691649, 90.00000672535116, 90.0000024414267, 90.00000236059856, 90.00000228915216, 90.00000235278931, 90.0000022318296, 90.00000227510141, 90.00000223749964, 90.00000223270888, 90.00000220314594, 90.00000221901716, 90.00000226118635, 90.00000223581947, 90.00000227543921, 90.00000227765419, 90.0000023000561, 90.00000227920145, 90.00000238121997, 90.00000238687504, 90.00000238774558, 90.00000238733222, 90.00000238257864, 90.00000227883201, 90.00000228486743, 90.00000227957341, 90.00000227186187, 90.00000223178118, 90.00000218747735, 90.00000222851014, 90.00000223188276, 90.0000022401056, 90.00000227395397, 90.00000228482298, 90.00000233409644, 90.00000236297963, 90.00000234573088, 90.00000239101483, 90.00000237643938, 90.00000239966492, 90.00000234039211, 90.00000231049235, 90.00000229610576, 90.000002278796, 90.00000224446404, 90.00000224007415, 90.00000222219893, 90.0000021959647, 90.00000222542576, 90.00000226217115, 90.00000227603834, 90.00000231058036, 90.00000233872595, 90.00000233924465, 90.00000239459897, 90.00000239362377, 90.0000023860275, 90.00000237206066, 90.00000236004391, 90.0000023051385, 90.00000230757081, 90.0000023095629, 90.00000225252235, 90.00000222752774, 90.00000218432507, 90.0000022092223, 90.00000223609982, 90.00000223954076, 90.000002296885, 90.00000229322444, 90.00000232181786, 90.00000234472056, 90.00000237091616, 90.00000239961457, 90.00000238124818, 90.00000235470986, 90.00000235490796, 90.00000231990673, 90.00000231314647, 90.00000228141978, 90.00000231577384, 90.00000219358681, 90.00000221964311, 90.00000221902677, 90.00000225197029, 90.00000228557717, 90.00000227078729, 90.00000232713879, 90.00000234973864, 90.00000233758836, 90.00000237200223, 90.00000234038912, 90.00000244040754, 90.0000024372309, 90.00000248049379, 90.00000250172882, 90.00000250578209, 90.00000257031641, 90.00000260008764, 90.0000026509073, 90.00000262102553, 90.00000259035237, 90.00000255295527, 90.0000025248063, 90.00000250625632, 90.00000248129783, 90.00000245503782, 90.00000242676077, 90.00000241585269, 90.00000238257277, 90.00000237049231, 90.00000230093765, 90.0000023485869, 90.00000225665936, 90.00000225760003, 90.00000220096328, 90.00000222061048, 90.00000222212537, 90.00000225154655, 90.00000228111675, 90.00000230094541, 90.00000229104751, 90.00000230642945, 90.0000023226165, 90.00000238566233, 90.00000241894503, 90.00000238542907, 90.00000243843832, 90.00000250061355, 90.00000252472385, 90.00000255463233, 90.00000255255489, 90.00000257198835, 90.00000257431239, 90.00000261524168, 90.00000259380785, 90.00000256935475, 90.00000254667032, 90.00000250122213, 90.00000248599213, 90.0000024543078, 90.00000242795107, 90.00000239330231, 90.00000241650338, 90.0000023963526, 90.00000234118262, 90.0000023331611, 90.00000229711505, 90.0000023012944, 90.00000223962012, 90.00000221276521, 90.0000022232705, 90.00000223585958, 90.00000225153013, 90.00000229849272, 90.00000230104297, 90.0000023293519, 90.00000234344562, 90.00000241792797, 90.00000240125584, 90.00000243991896, 90.00000243548132, 90.00000246751488, 90.00000252836035, 90.00000261016237, 90.00000253448184, 90.00000258163142, 90.00000263987316]
  in  "dy/dx vs x":bool=TRUE
  in  "Numeric":dbl=20.0
  out "Transconductance":T3(graph)
  out "peak locations":T3(graph)
  out "adjusted transconductance 2":dbl[][](graph)
  out "Intensity Graph 13":dbl[][](graph)
  out "adjusted transconductance":T3(graph)
  out "flattened and interpolated transconductance":T3(graph)
  in  "threshold":dbl=50.0 format="%0.2f"
  in  "X Step":dbl=0.002 format="%#_13g"
  in  "X High":dbl=0.1 format="%#_13g"
  in  "X Low":dbl=-0.06 format="%#_13g"
  in  "Array":dbl[](array[numeric])=array[10001 elements] format="%0.5f"
  out "size(s)":i32=2166
  in  "width":i32=40 min=3
  out "Waveform Graph":dbl[](graph)=[nan, nan, nan, nan, nan, nan, nan, nan, nan, nan, nan, nan, nan, nan, nan, nan, nan, nan, nan, nan, nan, nan, nan, nan, nan, nan, nan, nan, nan, nan, nan, nan, nan, nan, nan, nan, nan, nan, nan, nan, nan, nan, nan, nan, nan, nan, nan, nan, nan, nan, nan, nan, nan, nan, nan, nan, nan, nan, nan, nan, nan, nan, nan, nan, nan, nan, nan, nan, nan, nan, nan, nan, nan, nan, nan, nan, nan, nan, nan, nan, nan, nan, nan, nan, nan, nan, nan, nan, nan, nan, nan, nan, nan, nan, nan, nan, nan, nan, nan, nan, nan, nan, nan, nan, nan, nan, nan, nan, nan, nan, nan, nan, nan, nan, nan, nan, nan, nan, nan, nan, nan, nan, nan, nan, nan, nan, nan, nan, nan, nan, nan, nan, nan, nan, nan, nan, nan, nan, nan, nan, nan, nan, nan, nan, nan, nan, nan, nan, nan, nan, nan, nan, nan, nan, nan, nan, nan, nan, nan, nan, nan, nan, nan, nan, nan, nan, nan, nan, nan, nan, nan, nan, nan, nan, nan, nan, nan, nan, nan, nan, nan, nan, nan, nan, nan, nan, nan, nan, nan, nan, nan, nan, nan, nan, nan, nan, nan, nan, nan, nan, nan, nan, nan, nan, nan, nan, nan, nan, nan, nan, nan, nan, nan, nan, nan, nan, nan, nan, nan, nan, nan, nan, nan, nan, nan, nan, nan, nan, nan, nan, nan, nan, nan, nan, nan, nan, nan, nan, nan, nan, nan, nan, nan, nan, nan, nan, nan, nan, nan, nan, nan, nan, nan, nan, nan, nan, nan, nan, nan, nan, nan, nan, nan, nan, nan, nan, nan, nan, nan, nan, nan, nan, nan, nan, nan, nan, nan, nan, nan, nan, nan, nan, nan, nan, nan, nan, nan, nan, nan, nan, nan, nan, nan, nan, nan, nan, nan, nan, nan, nan, nan, nan, nan, nan, nan, nan, nan, nan, nan, nan, nan, nan, nan, nan, nan, nan, nan, nan, nan, nan, nan, nan, nan, nan, nan, nan, nan, nan, nan, nan, nan, nan, nan, nan, nan, nan, nan, nan, nan, nan, nan, nan, nan, nan, nan, nan, nan, nan, nan, nan, nan, nan, nan, nan, nan, nan, nan, nan, nan, nan, nan, nan, nan, nan, nan, nan, nan, nan, nan, nan, nan, nan, nan, nan, nan, nan, nan, nan, nan, nan, nan, nan, nan, nan, nan, nan, nan, nan, nan, nan, nan, nan, nan, nan, nan, nan, nan, nan, nan, nan, nan, nan, nan, nan, nan, nan, nan, nan, nan, nan, nan, nan, nan, nan, nan, nan, nan, nan, nan, nan, nan, nan, nan, nan, nan, nan, nan, nan, nan, nan, nan, nan, nan, nan, nan, nan, nan, nan, nan, nan, nan, nan, nan, nan, nan, nan, nan, nan, nan, nan, nan, nan, nan, nan, nan, nan, nan, nan, nan, nan, nan, nan, nan, nan, nan, nan, nan, nan, nan, nan, nan, nan, nan, nan, nan, nan, nan, nan, nan, nan, nan, nan, nan, nan, nan, nan, nan, nan, nan, nan, nan, nan, nan, nan, nan, nan, nan, nan, nan, nan, nan, nan, nan, nan, nan, nan, nan, nan, nan, nan, nan, nan, nan, nan, nan, nan, nan, nan, nan, nan, nan, nan, nan, nan, nan, nan, nan, nan, nan, nan, nan, nan, nan, nan, nan, nan, nan, nan, nan, nan, nan, nan, nan, nan, nan, nan, nan, nan, nan, nan, nan, nan, nan, nan, nan, nan, nan, nan, nan, nan, nan, nan, nan, nan, nan, nan, nan, nan, nan, nan, nan, nan, nan, nan, nan, nan, nan, nan, nan, nan, nan, nan, nan, nan, nan, nan, nan, nan, nan, nan, nan, nan, nan, nan, nan, nan, nan, nan, nan, nan, nan, nan, nan, nan, nan, nan, nan, nan, nan, nan, nan, nan, nan, nan, nan, nan, nan, nan, nan, nan, nan, nan, nan, nan, nan, nan, nan, nan, nan, nan, nan, nan, nan, nan, nan, nan, nan, nan, nan, nan, nan, nan, nan, nan, nan, nan, nan, nan, nan, nan, nan, nan, nan, nan, nan, nan, nan, nan, nan, nan, nan, nan, nan, nan, nan, nan, nan, nan, nan, nan, nan, nan, nan, nan, nan, nan, nan, nan, nan, nan, nan, nan, nan, nan, nan, nan, nan, nan, nan, nan, nan, nan, nan, nan, nan, nan, nan, nan, nan, nan, nan, nan, nan, nan, nan, nan, nan, nan, nan, nan, nan, nan, nan, nan, nan, nan, nan, nan, nan, nan, nan, nan, nan, nan, nan, nan, nan, nan, nan, nan, nan, nan, nan, nan, nan, nan, nan, nan, nan, nan, nan, nan, nan, nan, nan, nan, nan, nan, nan, nan, nan, nan, nan, nan, nan, nan, nan, nan, nan, nan, nan, nan, nan, nan, nan, nan, nan, nan, nan, nan, nan, nan, nan, nan, nan, nan, nan, nan, nan, nan, nan, nan, nan, nan, nan, nan, nan, nan, nan, nan, nan, nan, nan, nan, nan, nan, nan, nan, nan, nan, nan, nan, nan, nan, nan, nan, nan, nan, nan, nan, nan, nan, nan, nan, nan, nan, nan, nan, nan, nan, nan, nan, nan, nan, nan, nan, nan, nan, nan, nan, nan, nan, nan, nan, nan, nan, nan, nan, nan, nan, nan, nan, nan, nan, nan, nan, nan, nan, nan, nan, nan, nan, nan, nan, nan, nan, nan, nan, nan, nan, nan, nan, nan, nan, nan, nan, nan, nan, nan, nan, nan, nan, nan, nan, nan, nan, nan, nan, nan, nan, nan, nan, nan, nan, nan, nan, nan, nan, nan, nan, nan, nan, nan, nan, nan, nan, nan, nan, nan, nan, nan, nan, nan, nan, nan, nan, nan, nan, nan, nan, nan, nan, nan, nan, nan, nan, nan, nan, nan, nan, nan, nan, nan, nan, nan, nan, nan, nan, nan, nan, nan, nan, nan, nan, nan, nan, nan, nan, nan, nan, nan, nan, nan, nan, nan, nan, nan, nan, nan, nan, nan, nan, nan, nan, nan, nan, nan, nan, nan, nan, nan, nan, nan, nan, nan, nan, nan, nan, nan, nan, nan, nan, nan, nan, nan, nan, nan, nan, nan, nan, nan, nan, nan, nan, nan, nan, nan, nan, nan, nan, nan, nan, nan, nan, nan, nan, nan, nan, nan, nan, nan, nan, nan, nan, nan, nan, nan, nan, nan, nan, nan, nan, nan, nan, nan, nan, nan, nan, nan, nan, nan, nan, nan, nan, nan, nan, nan, nan, nan, nan, nan, nan, nan, nan, nan, nan, nan, nan, nan, nan, nan, nan, nan, nan, nan, nan, nan, nan, nan, nan, nan, nan, nan, nan, nan, nan, nan, nan, nan, nan, nan, nan, nan, nan, nan, nan, nan, nan, nan, nan, nan, nan, nan, nan, nan, nan, nan, nan, nan, nan, nan, nan, nan, nan, nan, nan, nan, nan, nan, nan, nan, nan, nan, nan, nan, nan, nan, nan, nan, nan, nan, nan, nan, nan, nan, nan, nan, nan, nan, nan, nan, nan, nan, nan, nan, nan, nan, nan, nan, nan, nan, nan, nan, nan, nan, nan, nan, nan, nan, nan, nan, nan, nan, nan, nan, nan, nan, nan, nan, nan, nan, nan, nan, nan, nan, nan, nan, nan, nan, nan, nan, nan, nan, nan, nan, nan, nan, nan, nan, nan, nan, nan, nan, nan, nan, nan, nan, nan, nan, nan, nan, nan, nan, nan, nan, nan, nan, nan, nan, nan, nan, nan, nan, nan, nan, nan, nan, nan, nan, nan, nan, nan, nan, nan, nan, nan, nan, nan, nan, nan, nan, nan, nan, nan, nan, nan, nan, nan, nan, nan, nan, nan, nan, nan, nan, nan, nan, nan, nan, nan, nan, nan, nan, nan, nan, nan, nan, nan, nan, nan, nan, nan, nan, nan, nan, nan, nan, nan, nan, nan, nan, nan, nan, nan, nan, nan, nan, nan, nan, nan, nan, nan, nan, nan, nan, nan, nan, nan, nan, nan, nan, nan, nan, nan, nan, nan, nan, nan, nan, nan, nan, nan, nan, nan, nan, nan, nan, nan, nan, nan, nan, nan, nan, nan, nan, nan, nan, nan, nan, nan, nan, nan, nan, nan, nan, nan, nan, nan, nan, nan, nan, nan, nan, nan, nan, nan, nan, nan, nan, nan, nan, nan, nan, nan, nan, nan, nan, nan, nan, nan, nan, nan, nan, nan, nan, nan, nan, nan, nan, nan, nan, nan, nan, nan, nan, nan, nan, nan, nan, nan, nan, nan, nan, nan, nan, nan, nan, nan, nan, nan, nan, nan, nan, nan, nan, nan, nan, nan, nan, nan, nan, nan, nan, nan, nan, nan, nan, nan, nan, nan, nan, nan, nan, nan, nan, nan, nan, nan, nan, nan, nan, nan, nan, nan, nan, nan, nan, nan, nan, nan, nan, nan, nan, nan, nan, nan, nan, nan, nan, nan, nan, nan, nan, nan, nan, nan, nan, nan, nan, nan, nan, nan, nan, nan, nan, nan, nan, nan, nan, nan, nan, nan, nan, nan, nan, nan, nan, nan, nan, nan, nan, nan, nan, nan, nan, nan, nan, nan, nan, nan, nan, nan, nan, nan, nan, nan, nan, nan, nan, nan, nan, nan, nan, nan, nan, nan, nan, nan, nan, nan, nan, nan, nan, nan, nan, nan, nan, nan, nan, nan, nan, nan, nan, nan, nan, nan, nan, nan, nan, nan, nan, nan, nan, nan, nan, nan, nan, nan, nan, nan, nan, nan, nan, nan, nan, nan, nan, nan, nan, nan, nan, nan, nan, nan, nan, nan, nan, nan, nan, nan, nan, nan, nan, nan, nan, nan, nan, nan, nan, nan, nan, nan, nan, nan, nan, nan, nan, nan, nan, nan, nan, nan, nan, nan, nan, nan, nan, nan, nan, nan, nan, nan, nan, nan, nan, nan, nan, nan, nan, nan, nan, nan, nan, nan, nan, nan, nan, nan, nan, nan, nan, nan, nan, nan, nan, nan, nan, nan, nan, nan, nan, nan, nan, nan, nan, nan, nan, nan, nan, nan, nan, nan, nan, nan, nan, nan, nan, nan, nan, nan, nan, nan, nan, nan, nan, nan, nan, nan, nan, nan, nan, nan, nan, nan, nan, nan, nan, nan, nan, nan, nan, nan, nan, nan, nan, nan, nan, nan, nan, nan, nan, nan, nan, nan, nan, nan, nan, nan, nan, nan, nan, nan, nan, nan, nan, nan, nan, nan, nan, nan, nan, nan, nan, nan, nan, nan, nan, nan, nan, nan, nan, nan, nan, nan, nan, nan, nan, nan, nan, nan, nan, nan, nan, nan, nan, nan, nan, nan, nan, nan, nan, nan, nan, nan, nan, nan, nan, nan, nan, nan, nan, nan, nan, nan, nan, nan, nan, nan, nan, nan, nan, nan, nan, nan, nan, nan, nan, nan, nan, nan, nan, nan, nan, nan, nan, nan, nan, nan, nan, nan, nan, nan, nan, nan, nan, nan, nan, nan, nan, nan, nan, nan, nan, nan, nan, nan, nan, nan, nan, nan, nan, nan, nan, nan, nan, nan, nan, nan, nan, nan, nan, nan, nan, nan, nan, nan, nan, nan, nan, nan, nan, nan, nan, nan, nan, nan, nan, nan, nan, nan, nan, nan, nan, nan, nan, nan, nan, nan, nan, nan, nan, nan, nan, nan, nan, nan, nan, nan, nan, nan, nan, nan, nan, nan, nan, nan, nan, nan, nan, nan, nan, nan, nan, nan, nan, nan, nan, nan, nan, nan, nan, nan, nan, nan, nan, nan, nan, nan, nan, nan, nan, nan, nan, nan, nan, nan, nan, nan, nan, nan, nan, nan, nan, nan, nan, nan, nan, nan, nan, nan, nan, nan, nan, nan, nan, nan, nan, nan, nan, nan, nan, nan, nan, nan, nan, nan, nan, nan, nan, nan, nan, nan, nan, nan, nan, nan, nan, nan, nan, nan, nan, nan, nan, nan, nan, nan, nan, nan, nan, nan, nan, nan, nan, nan, nan, nan, nan, nan, nan, nan, nan, nan, nan, nan, nan, nan, nan, nan, nan, nan, nan, nan, nan, nan, nan, nan, nan, nan, nan, nan, nan, nan, nan, nan, nan, nan, nan, nan, nan, nan, nan, nan, nan, nan, nan, nan, nan, nan, nan, nan, nan, nan, nan, nan, nan, nan, nan, nan, nan, nan, nan, nan, nan, nan, nan, nan, nan, nan, nan, nan, nan, nan, nan, nan, nan, nan, nan, nan, nan, nan, nan, nan, nan, nan, nan, nan, nan, nan, nan, nan, nan, nan, nan, nan, nan, nan, nan, nan, nan, nan, nan, nan, nan, nan, nan, nan, nan, nan, nan, nan, nan, nan, nan, nan, nan, nan, nan, nan, nan, nan, nan, nan, nan, nan, nan, nan, nan, nan, nan, nan, nan, nan, nan, nan, nan, nan, nan, nan, nan, nan, nan, nan, nan, nan, nan, nan, nan, nan, nan, nan, nan, nan, nan, nan, nan, nan, nan, nan, nan, nan, nan, nan, nan, nan, nan, nan, nan, nan, nan, nan, nan, nan, nan, nan, nan, nan, nan, nan, nan, nan, nan, nan, nan, nan, nan, nan, nan, nan, nan, nan, nan, nan, nan, nan, nan, nan, nan, nan, nan, nan, nan, nan, nan, nan, nan, nan, nan, nan, nan, nan, nan]
  in  "threshold 2":dbl=25.0 format="%0.2f"
  in  "width 2":i32=25 min=3
  out "first peak":cluster{dbl[], "Best Linear Fit":dbl[]}[](graph)
  in  "index":i32
  in  "length":i32
  out "Intensity Graph 15":dbl[][](graph)
  in  "X Low 3":dbl=-0.06 format="%#_13g"
  in  "X High 3":dbl=0.6 format="%#_13g"
  in  "X Step 3":dbl=0.002 format="%#_13g"
  in  "low cutoff freq: fl":dbl=0.04 format="%#_13g"
  in  "filter type":T4
  in  "high cutoff freq: fh":dbl=0.45000000000000007 format="%0.2f"
  in  "filter?":bool
  in  "offset trans":dbl
  out "Y line cut 5":T3(graph)
  out "Y line cut 7":T3(graph)
  in  "offset cond":dbl=0.01
  in  "offset 2":dbl
  out "Y line cut 6":T3(graph)
  in  "offset 3":dbl=10.0
  out "flattened and interpolated transconductance 2":T3(graph)
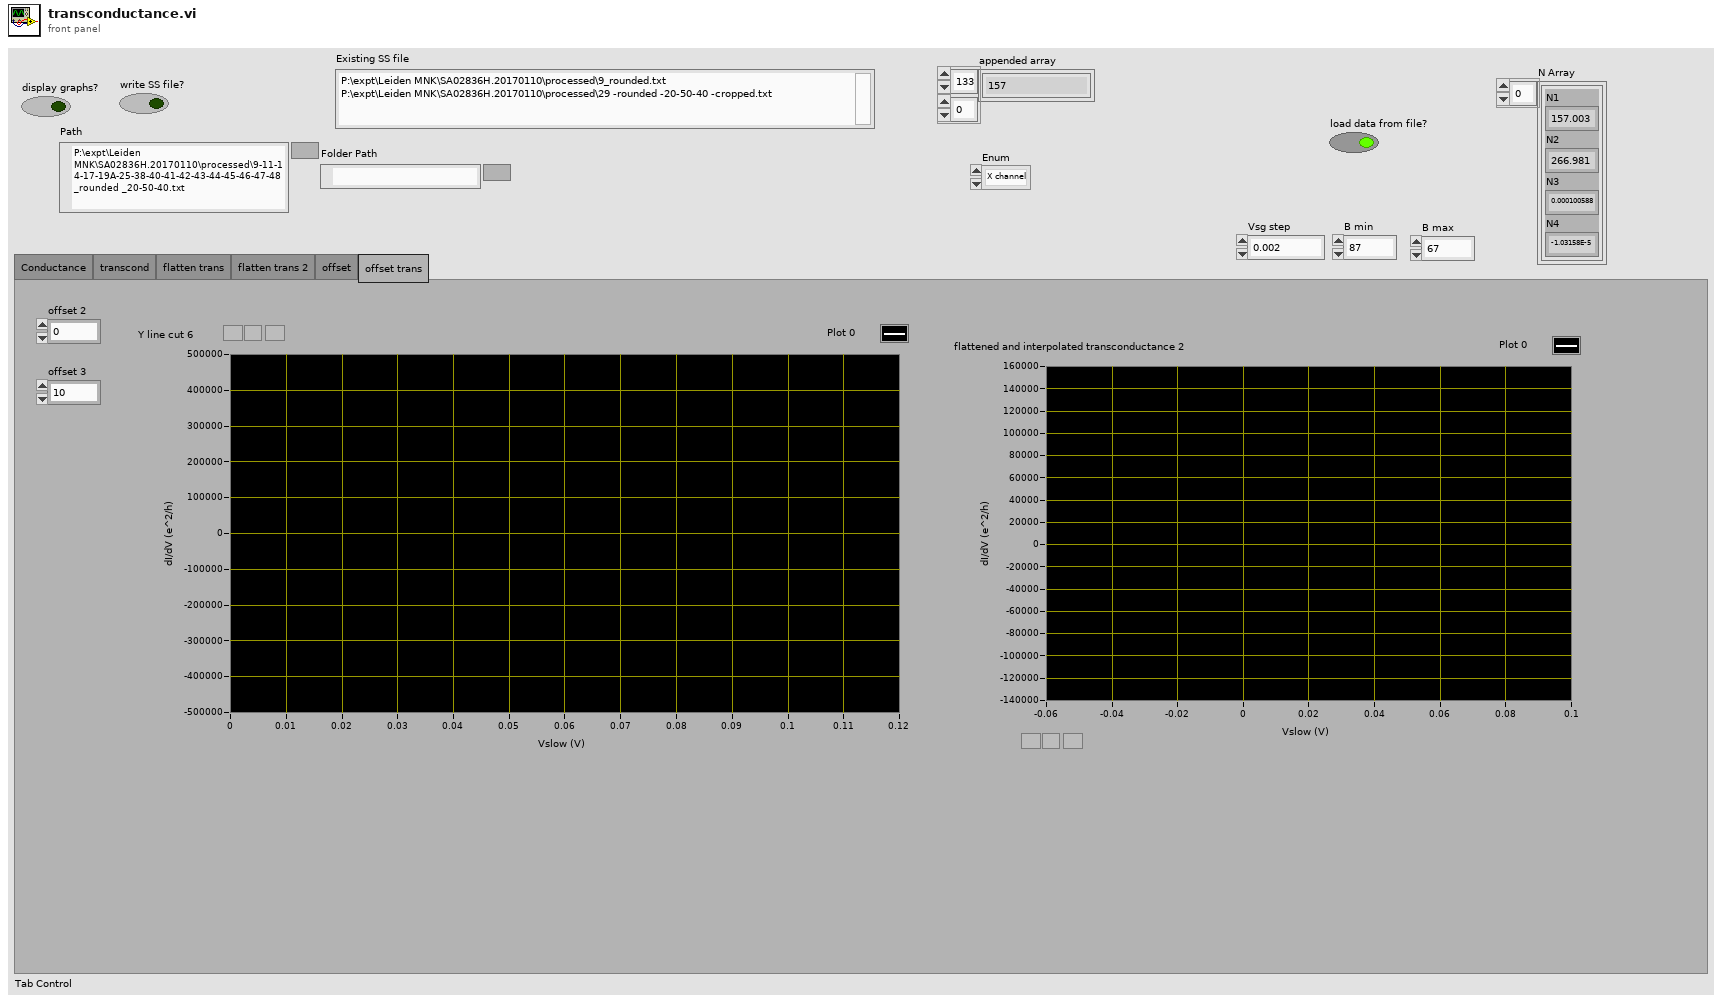
[diagram p1: front panel]
types:
  T1 = cluster{"N1":dbl, "N2":dbl, "N3":dbl, "N4":dbl}[]
  T2 = enum32{"Conductance", "transcond", "flatten trans", "flatten trans 2", "offset", "offset trans"}
  T3 = cluster{"Vfast":dbl[], "Decimated Array":dbl[]}[]
  T4 = typedef "NI_AALBase.lvlib/Filter Passband Type.ctl" = enum32{"Lowpass", "Highpass", "Bandpass", "Bandstop"}
  T5 = cluster{"Decimated Array":dbl[], "Decimated Array":dbl[]}
  T6 = typedef "MGI Write Spreadsheet Behavior Enum.ctl" = enum16{"Append data", "Append headers and data", "Overwrite"}
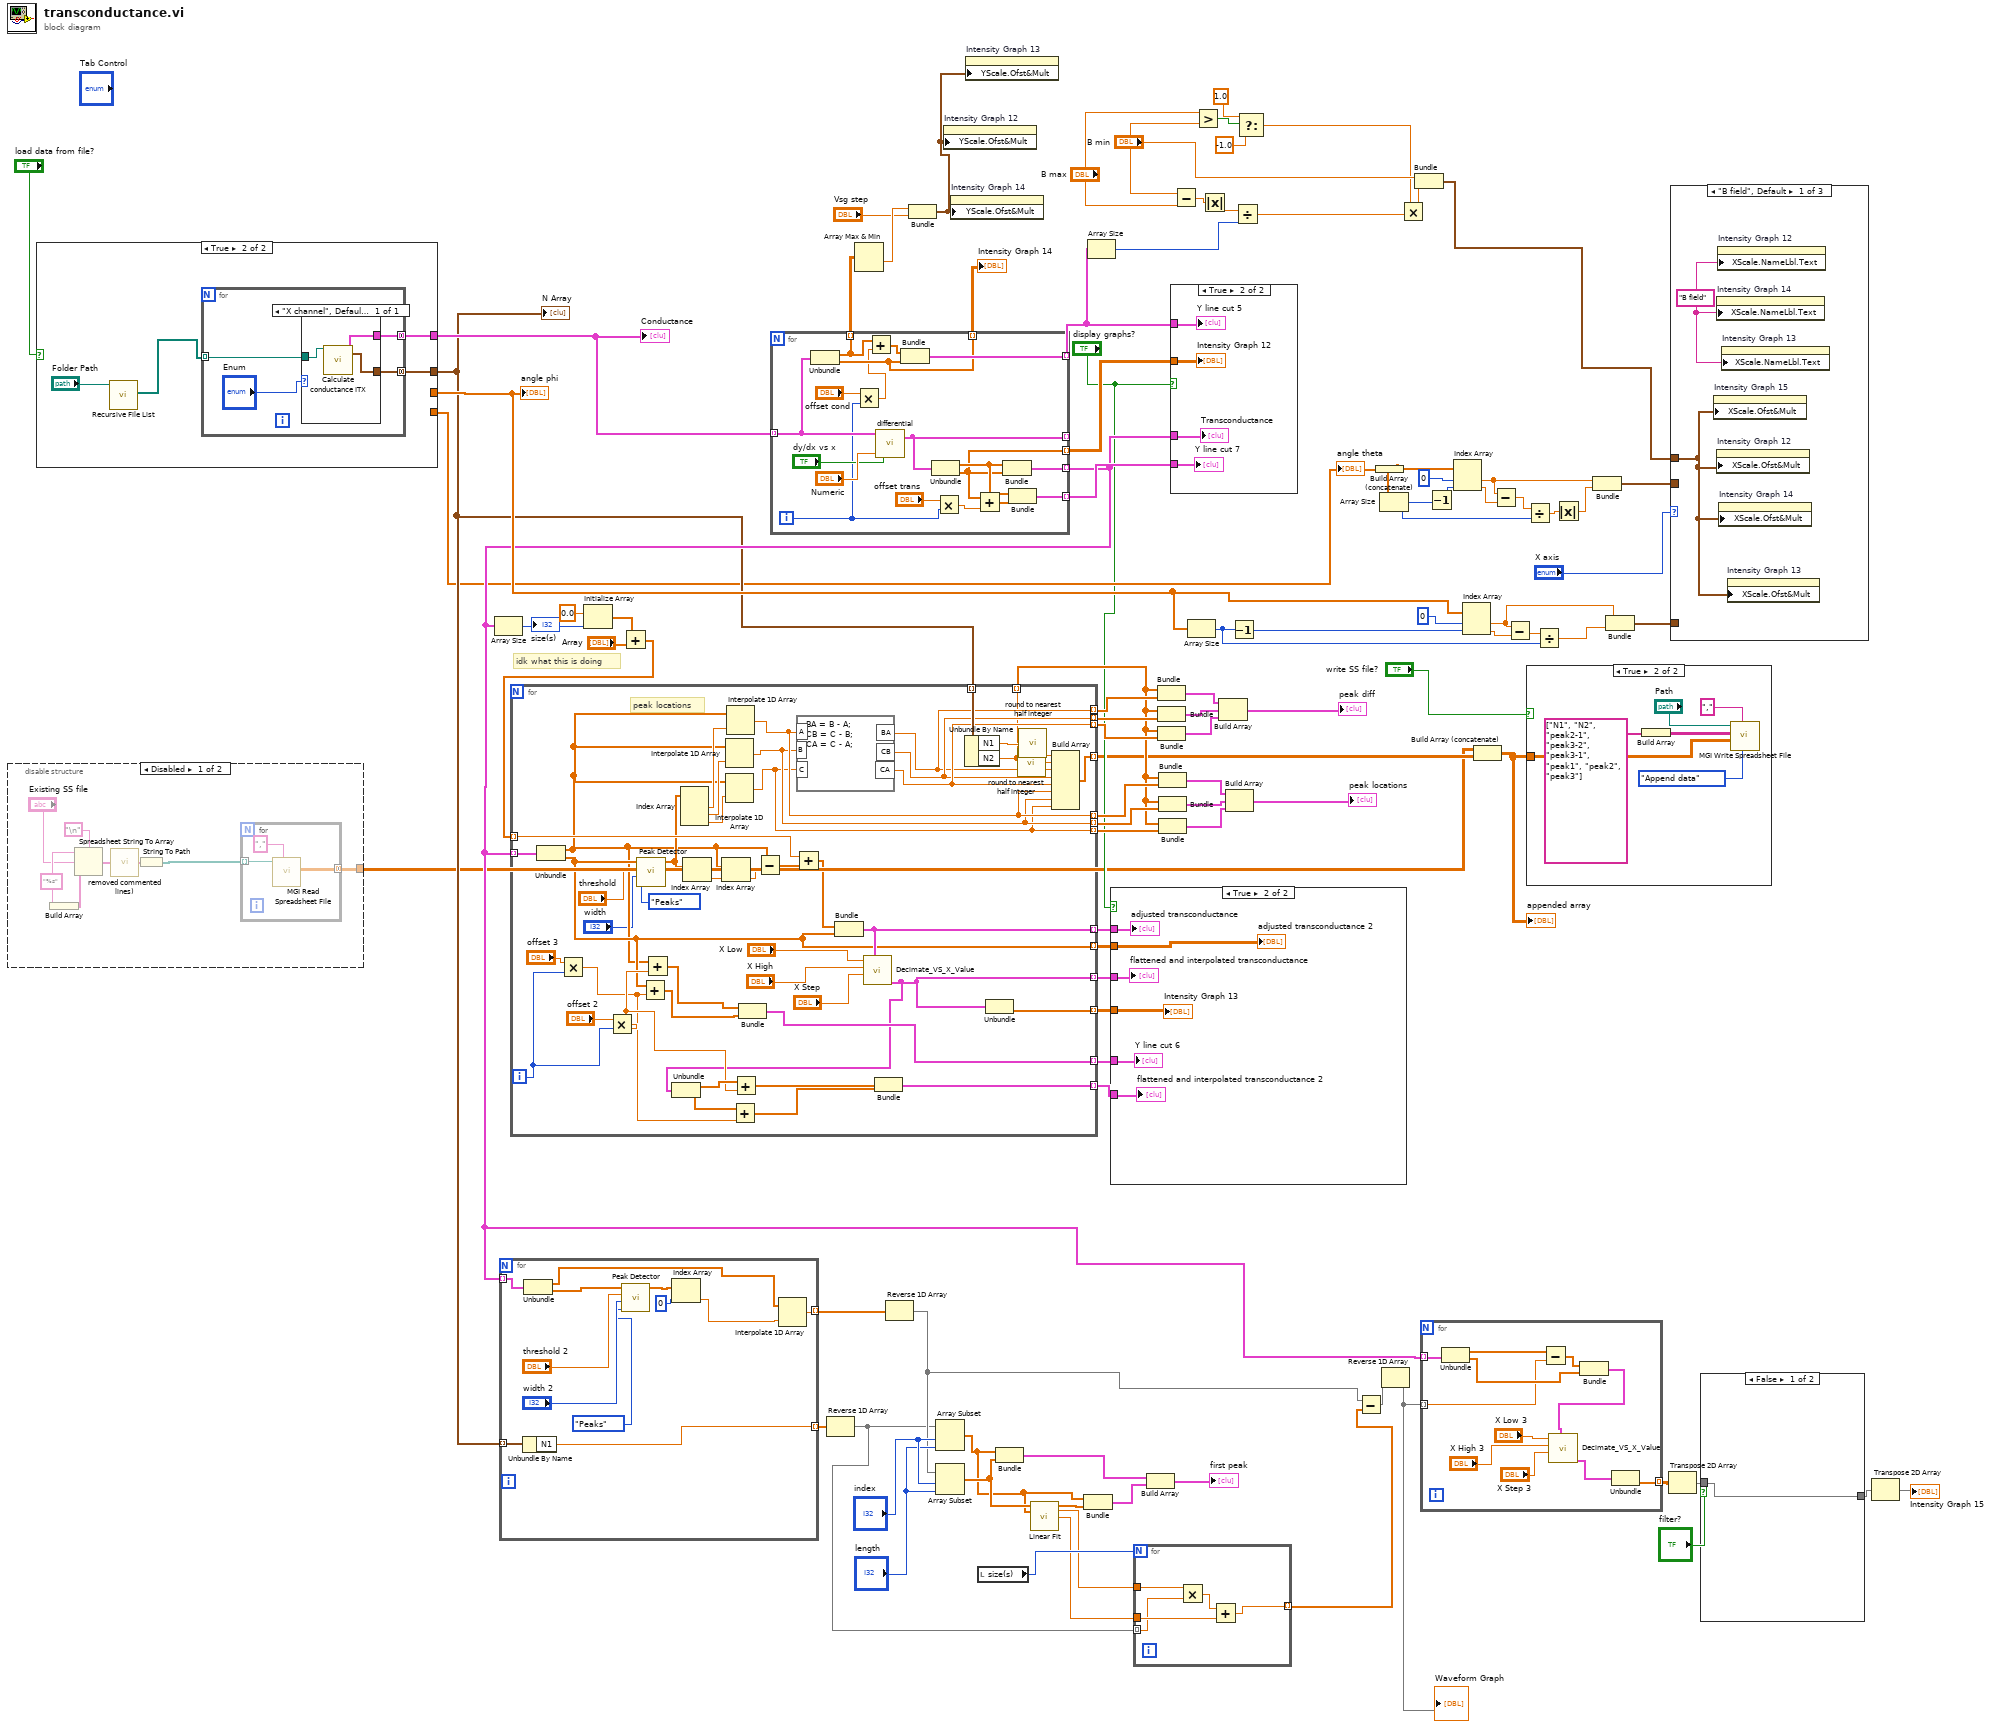
[diagram p0: block diagram]
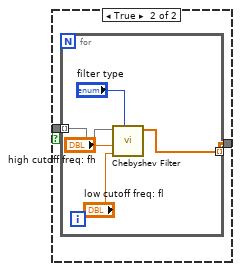
[diagram p4: hidden frame]
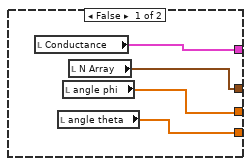
[diagram p7: hidden frame]
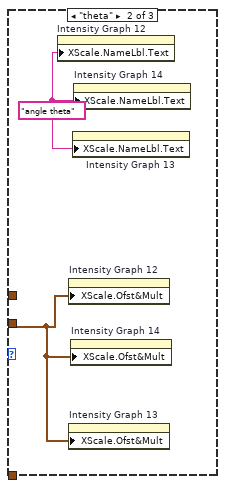
[diagram p8: hidden frame]
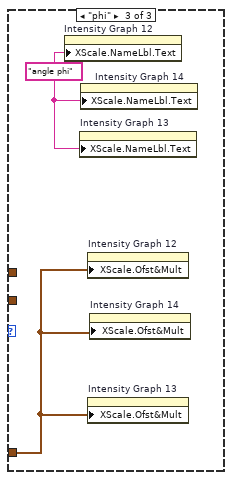
[diagram p9: hidden frame]
diagram:
  # "idk what this is doing"
  n1 = disable-structure shown="Disabled" {
    disable-tunnel: [w102 _] -> w2
    frame Disabled {
      w107 = "%s" ("format string")
      n2 = Build Array(w107) -> (w106:string[])
      n3 = Spreadsheet String To Array(delimiter (Tab)="\n", format string=w107, spreadsheet string="Existing SS file", array type (2D Dbl)=w106) -> (array=w101:string[])
      n4 = call "removed commented lines).vi"("Array in"=w101) -> ("Array out"=w100:string[])
      n5 = String To Path(string=w100) -> (path=w105:path[])
      n6 = for {
        tunnel: w105 -> [w110] mode=indexing
        tunnel: [w108] -> w102 mode=concatenating
        n7 = call <userlib>:"MGI Read Spreadsheet File.vi"("Delimiter (Tab)"=",", "Path"=w110) -> ("Values"=w108:dbl[][])  [unwired: 5 in, 4 out]
      }
    }
    frame Enabled {
    }
  }
  n8 = case shown="True" "load data from file?" {
    tunnel: [w114 _] -> w6
    tunnel: [w111 w118] -> w66
    tunnel: [w113 _] -> w60
    tunnel: [w112 w117] -> w22
    frame False {
      n9 = local read "Conductance"() -> (w111:T3)
      n10 = local read "angle theta"() -> (w114:dbl[])
      n11 = local read "angle phi"() -> (w113:dbl[])
      n12 = local read "N Array"() -> (w112:T1)
    }
    frame True {
      n13 = call <vilib>:"Recursive File List.vi"("Folder Path"="Folder Path") -> ("All Files in Dir"=w116:path[])  [unwired: 6 in, 4 out]
      n14 = for {
        tunnel: [w122] -> w118 mode=concatenating
        tunnel: w116 -> [w121] mode=indexing
        tunnel: [w120] -> w117 mode=concatenating
        n15 = case shown="\"X channel\", Default" "Enum" {
          tunnel: [w125] -> w122
          tunnel: w121 -> [w124]
          tunnel: [w123] -> w120
          frame "X channel", Default {
            n16 = call "Calculate conductance ITX.vi"("File or Folder Path"=w124) -> ("N Array"=w123:T1, "A vs D"=w125:cluster{dbl[], dbl[]}[])  [unwired: 11 in, 2 out]
          }
        }
      }
    }
  }
  "Conductance" <- w66
  "angle theta" <- w6
  "angle phi" <- w60
  "N Array" <- w22
  n17 = for {
    tunnel: w66 -> [w138] mode=indexing
    tunnel: [w141] -> _ mode=indexing
    tunnel: [w139] -> w35 mode=indexing
    tunnel: [w126] -> w94 mode=indexing
    tunnel: [w137] -> w88 mode=indexing
    tunnel: [w135] -> w99 mode=indexing
    tunnel: [w134] -> w93 mode=indexing
    tunnel: [w130] -> w78 mode=indexing
    i -> [w129]
    n18 = Unbundle(w138) -> ("Vfast"=w134:dbl[], "Decimated Array"=w135:dbl[])
    n19 = Multiply(x="offset cond", y=w129) -> (x*y=w127:dbl)
    n20 = Add(x=w134, y=w127) -> (x+y=w136:dbl[])
    n21 = call <userlib>:"differential.vi"("Numeric"="Numeric", "dy/dx vs x"="dy/dx vs x", "A vs B 2"=w138) -> ("A vs B 3"=w141:T5)  [unwired: 1 in]
    n22 = Bundle(w136, "Decimated Array"=w135) -> (w137:cluster{dbl[], "Decimated Array":dbl[]})  [unwired: 1 in]
    n23 = Unbundle(w141) -> ("Decimated Array"=w131:dbl[], "Decimated Array"=w126:dbl[])
    n24 = Multiply(x="offset trans", y=w129) -> (x*y=w133:dbl)
    n25 = Add(x=w126, y=w133) -> (x+y=w132:dbl[])
    n26 = Bundle("Decimated Array"=w131, "Decimated Array"=w126) -> (w139:T5)  [unwired: 1 in]
    n27 = Bundle("Decimated Array"=w131, w132) -> (w130:cluster{"Decimated Array":dbl[], dbl[]})  [unwired: 1 in]
  }
  "Intensity Graph 14" <- w99
  n28 = Array Size(array=w35) -> (size(s)=w20:i32)
  "size(s)" <- w20
  n29 = for {
    tunnel: w35 -> [w155] mode=indexing
    tunnel: [w146] -> w44 mode=indexing
    tunnel: w22 -> [w150] mode=indexing
    tunnel: [w149] -> w53 mode=indexing
    n30 = Unbundle By Name(w150) -> ("N1"=w149:dbl)
    n31 = Unbundle(w155) -> ("Decimated Array"=w148:dbl[], "Decimated Array"=w144:dbl[])
    n32 = call <vilib>:"Peak Detector.vi"("peaks/valleys"=enum32{"Peaks", "Valleys"}."Peaks", "width"="width 2", "threshold"="threshold 2", "X"=w144) -> ("Locations"=w154:dbl[])  [unwired: 3 in, 4 out]
    n33 = Index Array(array=w154, index=0) -> (element=w147:dbl)
    n34 = Interpolate 1D Array(1:w147, 2:w148) -> (0:w146:dbl)
  }
  n35 = Initialize Array(0.0 ("element"), w20) -> (w13:dbl[])
  n36 = Add(x=w13, y="Array") -> (x+y=w11:dbl[])
  n37 = for {
    tunnel: [w177] -> w98 mode=indexing
    tunnel: [w176] -> w97 mode=indexing
    tunnel: [w195] -> w96 mode=indexing
    tunnel: w35 -> [w198] mode=indexing
    tunnel: w11 -> [w175] mode=indexing
    tunnel: [w192] -> w95 mode=indexing
    tunnel: [w188] -> w71 mode=indexing
    tunnel: [w165] -> w18 mode=indexing
    tunnel: [w164] -> w28 mode=indexing
    tunnel: [w163] -> w19 mode=indexing
    tunnel: w22 -> [w174] mode=indexing
    tunnel: [w181] -> w3 mode=indexing
    tunnel: [w166] -> w21 mode=indexing
    tunnel: [w171] -> w17 mode=indexing
    tunnel: [w172] -> w16 mode=indexing
    tunnel: [w173] -> w15 mode=indexing
    tunnel: [w157] -> w10 mode=indexing
    i -> [w191]
    # "peak locations"
    n38 = Unbundle(w198) -> ("Decimated Array"=w162:dbl[], "Decimated Array"=w166:dbl[])
    n39 = Multiply(x="offset 3", y=w191) -> (x*y=w184:dbl)
    n40 = Multiply(x="offset 2", y=w191) -> (x*y=w186:dbl)
    n41 = call <vilib>:"Peak Detector.vi"("peaks/valleys"=enum32{"Peaks", "Valleys"}."Peaks", "width"="width", "threshold"="threshold", "X"=w166) -> ("Locations"=w170:dbl[])  [unwired: 3 in, 4 out]
    n42 = Add(x=w166, y=w184) -> (x+y=w189:dbl[])
    n43 = Add(x=w162, y=w186) -> (x+y=w193:dbl[])
    n44 = Index Array(array=w170) -> (element #1=w169:dbl, element #2=w168:dbl, element #3=w167:dbl)  [unwired: 3 in]
    n45 = Index Array(array=w170) -> (element=w180:dbl)  [unwired: 1 in]
    n46 = Index Array(array=w162, index=w180) -> (element=w196:dbl)
    n47 = Interpolate 1D Array(1:w168, 2:w162) -> (0:w164:dbl)
    n48 = Interpolate 1D Array(1:w167, 2:w162) -> (0:w163:dbl)
    n49 = Interpolate 1D Array(1:w169, 2:w162) -> (0:w165:dbl)
    n50 = Bundle(w193, w189) -> (w192:cluster{dbl[], dbl[]})  [unwired: 1 in]
    n51 = Subtract(x=w162, y=w196) -> (x-y=w179:dbl[])
    n52 = Add(x=w175, y=w179) -> (x+y=w178:dbl[])
    n53 = formula code="BA = B - A;\nCB = C - B;\nCA = C - A;"("A"=w165, "B"=w164, "C"=w163) -> ("BA"=w171:dbl, "CB"=w172:dbl, "CA"=w173:dbl)
    n54 = Bundle(w178, "Decimated Array"=w166) -> (w177:cluster{dbl[], "Decimated Array":dbl[]})  [unwired: 1 in]
    n55 = call <userlib>:"Decimate_VS_X_Value.vi"("XY Graph kind 1"=w177, "X Step"="X Step", "X High"="X High", "X Low"="X Low") -> ("Interpreted"=w176:cluster{dbl[], dbl[]})  [unwired: 6 in, 1 out]
    n56 = Unbundle(w176) -> (w187:dbl[], w185:dbl[])
    n57 = Add(x=w185, y=w184) -> (x+y=w182:dbl[])
    n58 = Add(x=w187, y=w186) -> (x+y=w183:dbl[])
    n59 = Bundle(w183, w182) -> (w188:cluster{dbl[], dbl[]})  [unwired: 1 in]
    n60 = Unbundle By Name(w174) -> ("N1"=w159:dbl, "N2"=w157:dbl)
    n61 = Unbundle(w176) -> (w195:dbl[])  [unwired: 1 out]
    n62 = call "round to nearest half integer.vi"("Numeric"=w157) -> ("rounded to nearest 0.5"=w158:dbl)
    n63 = call "round to nearest half integer.vi"("Numeric"=w159) -> ("rounded to nearest 0.5"=w156:dbl)
    n64 = Build Array(w156, w158, w171, w172, w173, w165, w164, w163) -> (w181:dbl[])
  }
  n65 = Reverse 1D Array(array=w53) -> (reversed array=w38:dbl[])
  n66 = Array Max & Min(array=w93) -> (min value=w92:dbl)  [unwired: 3 out]
  n67 = Reverse 1D Array(array=w44) -> (reversed array=w43:dbl[])
  n68 = Bundle(w92, "Vsg step"="Vsg step") -> (w70:cluster{dbl, "Vsg step":dbl})  [unwired: 1 in]
  n69 = Array Subset(array=w38, index="index", length="length") -> (w40:dbl[])
  n70 = Array Subset(array=w43, index="index", length="length") -> (w41:dbl[])
  n71 = property on="Intensity Graph 12" class="IntGraph (strict)"("YScale.Ofst&Mult"=w70) -> ()  [unwired: 2 in, 2 out]
  n72 = property on="Intensity Graph 14" class="IntGraph (strict)"("YScale.Ofst&Mult"=w70) -> ()  [unwired: 2 in, 2 out]
  n73 = property on="Intensity Graph 13" class="IntGraph (strict)"("YScale.Ofst&Mult"=w70) -> ()  [unwired: 2 in, 2 out]
  n74 = local read "size(s)"() -> (w46:i32)
  n75 = Bundle(w40, w41) -> (w50:cluster{dbl[], dbl[]})  [unwired: 1 in]
  n76 = call <vilib>:"Linear Fit.vi"("Y"=w41, "X"=w40) -> ("Best Linear Fit"=w47:dbl[], "slope"=w42:dbl, "intercept"=w39:dbl)  [unwired: 9 in, 2 out]
  n77 = Bundle(w40, "Best Linear Fit"=w47) -> (w48:cluster{dbl[], "Best Linear Fit":dbl[]})  [unwired: 1 in]
  n78 = Array Size(array=w88) -> (size(s)=w87:i32)
  n79 = case shown="True" "display graphs?" {
    tunnel: w98 -> [_ w207]
    tunnel: w97 -> [_ w206]
    tunnel: w96 -> [_ w205]
    tunnel: w95 -> [_ w204]
    tunnel: w71 -> [_ w203]
    tunnel: w21 -> [_ w202]
    frame False {
    }
    frame True {
      "Intensity Graph 13" <- w205
      "adjusted transconductance" <- w207
      "flattened and interpolated transconductance" <- w206
      "Y line cut 6" <- w204
      "flattened and interpolated transconductance 2" <- w203
      "adjusted transconductance 2" <- w202
    }
  }
  n80 = for {
    N: w46 -> [_]
    tunnel: w42 -> [w212]
    tunnel: w39 -> [w210]
    tunnel: [w209] -> w45 mode=indexing
    tunnel: w38 -> [w208] mode=indexing
    n81 = Multiply(x=w212, y=w208) -> (x*y=w211:dbl)
    n82 = Add(x=w211, y=w210) -> (x+y=w209:dbl)
  }
  n83 = Build Array(w50, w48) -> (→"first peak":cluster{dbl[], "Best Linear Fit":dbl[]}[])
  n84 = Bundle(w10, w17) -> (w30:cluster{dbl[], dbl[]})  [unwired: 1 in]
  n85 = Bundle(w10, w16) -> (w29:cluster{dbl[], dbl[]})  [unwired: 1 in]
  n86 = Bundle(w10, w15) -> (w23:cluster{dbl[], dbl[]})  [unwired: 1 in]
  n87 = Bundle(w10, w18) -> (w27:cluster{dbl[], dbl[]})  [unwired: 1 in]
  n88 = Bundle(w10, w28) -> (w26:cluster{dbl[], dbl[]})  [unwired: 1 in]
  n89 = Bundle(w10, w19) -> (w25:cluster{dbl[], dbl[]})  [unwired: 1 in]
  n90 = case shown="True" "display graphs?" {
    tunnel: w94 -> [_ w216]
    tunnel: w88 -> [_ w215]
    tunnel: w78 -> [_ w214]
    tunnel: w35 -> [_ w213]
    frame False {
    }
    frame True {
      "Transconductance" <- w213
      "Intensity Graph 12" <- w216
      "Y line cut 5" <- w215
      "Y line cut 7" <- w214
    }
  }
  n91 = Subtract(x="B min", y="B max") -> (x-y=w90:dbl)
  n92 = Array Size(array=w60) -> (size(s)=w58:i32)
  n93 = Greater?(x="B max", y="B min") -> (0:w84:bool)
  n94 = Absolute Value(x=w90) -> (abs(x)=w89:dbl)
  n95 = Build Array(w30, w29, w23) -> (→"peak diff":cluster{dbl[], dbl[]}[])
  n96 = Build Array(w27, w26, w25) -> (→"peak locations":cluster{dbl[], dbl[]}[])
  n97 = Decrement(x=w58) -> (x-1=w59:i32)
  n98 = Divide(x=w89, y=w87) -> (x/y=w81:dbl)
  n99 = Select(t=1.0, s=w84, f=-1.0) -> (s? t:f=w80:dbl)
  n100 = Subtract(x=w43, y=w45) -> (x-y=w37:dbl[])
  n101 = Build Array (concatenate)(w6) -> (w8:dbl[])
  n102 = Array Size(array=w8) -> (size(s)=w62:i32)
  n103 = Reverse 1D Array(array=w37) -> (reversed array=w36:dbl[])
  "Waveform Graph" <- w36
  n104 = Multiply(x=w80, y=w81) -> (x*y=w79:dbl)
  n105 = Bundle("B min"="B min", w79) -> (w76:cluster{"B min":dbl, dbl})  [unwired: 1 in]
  n106 = for {
    tunnel: w35 -> [w227] mode=indexing
    tunnel: [w220] -> w34 mode=indexing
    tunnel: w36 -> [w217] mode=indexing
    n107 = Unbundle(w227) -> ("Decimated Array"=w218:dbl[], "Decimated Array"=w226:dbl[])
    n108 = Subtract(x=w218, y=w217) -> (x-y=w219:dbl[])
    n109 = Bundle(w219, "Decimated Array"=w226) -> (w221:cluster{dbl[], "Decimated Array":dbl[]})  [unwired: 1 in]
    n110 = call <userlib>:"Decimate_VS_X_Value.vi"("XY Graph kind 1"=w221, "X Step"="X Step 3", "X High"="X High 3", "X Low"="X Low 3") -> ("Interpreted"=w222:cluster{dbl[], dbl[]})  [unwired: 6 in, 1 out]
    n111 = Unbundle(w222) -> (w220:dbl[])  [unwired: 1 out]
  }
  n112 = Decrement(x=w62) -> (x-1=w64:i32)
  n113 = Index Array(array=w8, index #1=0 ("index"), index #2=w64) -> (element #1=w75:dbl, element #2=w74:dbl)
  n114 = Index Array(array=w60, index #1=0 ("index"), index #2=w59) -> (element #1=w56:dbl, element #2=w55:dbl)
  n115 = Build Array (concatenate)(w2, w3) -> (w4:dbl[][])
  "appended array" <- w4
  n116 = Subtract(x=w75, y=w74) -> (x-y=w69:dbl)
  n117 = Subtract(x=w56, y=w55) -> (x-y=w63:dbl)
  n118 = Divide(x=w69, y=w62) -> (x/y=w68:dbl)
  n119 = case shown="True" "write SS file?" {
    tunnel: w4 -> [_ w231]
    frame False {
    }
    frame True {
      n120 = Build Array(string[] ["N1", "N2", "peak2-1", "peak3-2", "peak3-1", "peak1", "peak2", "peak3"] ("Header Lines[row][col]")) -> (w230:string[][])
      n121 = call <userlib>:"MGI Write Spreadsheet File.vi"("Existing File Behavior"=MGI_Write_Spreadsheet_Behavior_Enum."Append data", "Delimiter (Tab)"=",", "Data[row][col]"=w231, "Header Lines[row][col]"=w230, "Path"="Path") -> ()  [unwired: 3 in, 4 out]
    }
  }
  n122 = Divide(x=w63, y=w58) -> (x/y=w54:dbl)
  n123 = Absolute Value(x=w68) -> (abs(x)=w73:dbl)
  n124 = Bundle(w75, w73) -> (w72:cluster{dbl, dbl})  [unwired: 1 in]
  n125 = Bundle(w56, w54) -> (w61:cluster{dbl, dbl})  [unwired: 1 in]
  n126 = Transpose 2D Array(2D array=w34) -> (transposed array=w33:dbl[][])
  n127 = case shown="\"B field\", Default" "X axis" {
    tunnel: w76 -> [w234 _ _]
    tunnel: w72 -> [_ w237 _]
    tunnel: w61 -> [_ _ w239]
    frame "B field", Default {
      w235 = "B field"
      n128 = property on="Intensity Graph 15" class="IntGraph (strict)"("XScale.Ofst&Mult"=w234) -> ()  [unwired: 2 in, 2 out]
      n129 = property on="Intensity Graph 14" class="IntGraph (strict)"("XScale.NameLbl.Text"=w235) -> ()  [unwired: 2 in, 2 out]
      n130 = property on="Intensity Graph 12" class="IntGraph (strict)"("XScale.Ofst&Mult"=w234) -> ()  [unwired: 2 in, 2 out]
      n131 = property on="Intensity Graph 12" class="IntGraph (strict)"("XScale.NameLbl.Text"=w235) -> ()  [unwired: 2 in, 2 out]
      n132 = property on="Intensity Graph 14" class="IntGraph (strict)"("XScale.Ofst&Mult"=w234) -> ()  [unwired: 2 in, 2 out]
      n133 = property on="Intensity Graph 13" class="IntGraph (strict)"("XScale.NameLbl.Text"=w235) -> ()  [unwired: 2 in, 2 out]
      n134 = property on="Intensity Graph 13" class="IntGraph (strict)"("XScale.Ofst&Mult"=w234) -> ()  [unwired: 2 in, 2 out]
    }
    frame "theta" {
      w236 = "angle theta"
      n135 = property on="Intensity Graph 12" class="IntGraph (strict)"("XScale.NameLbl.Text"=w236) -> ()  [unwired: 2 in, 2 out]
      n136 = property on="Intensity Graph 12" class="IntGraph (strict)"("XScale.Ofst&Mult"=w237) -> ()  [unwired: 2 in, 2 out]
      n137 = property on="Intensity Graph 13" class="IntGraph (strict)"("XScale.Ofst&Mult"=w237) -> ()  [unwired: 2 in, 2 out]
      n138 = property on="Intensity Graph 14" class="IntGraph (strict)"("XScale.Ofst&Mult"=w237) -> ()  [unwired: 2 in, 2 out]
      n139 = property on="Intensity Graph 13" class="IntGraph (strict)"("XScale.NameLbl.Text"=w236) -> ()  [unwired: 2 in, 2 out]
      n140 = property on="Intensity Graph 14" class="IntGraph (strict)"("XScale.NameLbl.Text"=w236) -> ()  [unwired: 2 in, 2 out]
    }
    frame "phi" {
      w238 = "angle phi"
      n141 = property on="Intensity Graph 12" class="IntGraph (strict)"("XScale.NameLbl.Text"=w238) -> ()  [unwired: 2 in, 2 out]
      n142 = property on="Intensity Graph 13" class="IntGraph (strict)"("XScale.NameLbl.Text"=w238) -> ()  [unwired: 2 in, 2 out]
      n143 = property on="Intensity Graph 14" class="IntGraph (strict)"("XScale.NameLbl.Text"=w238) -> ()  [unwired: 2 in, 2 out]
      n144 = property on="Intensity Graph 12" class="IntGraph (strict)"("XScale.Ofst&Mult"=w239) -> ()  [unwired: 2 in, 2 out]
      n145 = property on="Intensity Graph 13" class="IntGraph (strict)"("XScale.Ofst&Mult"=w239) -> ()  [unwired: 2 in, 2 out]
      n146 = property on="Intensity Graph 14" class="IntGraph (strict)"("XScale.Ofst&Mult"=w239) -> ()  [unwired: 2 in, 2 out]
    }
  }
  n147 = case shown="False" "filter?" {
    tunnel: w33 -> [w240 w242]
    tunnel: [w240 w241] -> w32
    frame False {
    }
    frame True {
      n148 = for {
        tunnel: w242 -> [w246] mode=indexing
        tunnel: [w245] -> w241 mode=indexing
        n149 = call-poly <vilib>:"Chebyshev Filter.vi"("filter type"="filter type", "low cutoff freq: fl"="low cutoff freq: fl", "high cutoff freq: fh"="high cutoff freq: fh", "X"=w246) -> ("Filtered X"=w245:dbl[])  [unwired: 6 in, 1 out]
      }
    }
  }
  n150 = Transpose 2D Array(2D array=w32) -> (transposed array=→"Intensity Graph 15":dbl[][])
